vi "UNITEST MAIN v2.0.vi"() -> ()   [LabVIEW 2025]
uses:
  Traction Loop/Traction Receipe Enum.ctl
  controls/LAB-IQ UI Data.ctl
  <vilib>/Platform/TimedLoop/XDataNode/timing_clust.ctl
  <vilib>/Platform/TimedLoop/XDataNode/nitl_modes.ctl
  <vilib>/Platform/TimedLoop/XDataNode/wakeup.ctl
  Traction Loop/Traction Write enum.ctl
  Traction Loop/Traction Read enum.ctl
  HEAVE vi's/Heave Write enum.ctl
  SWAY vi's/Sway Write enum.ctl
  Acquostics Loops/Write Main Enum.ctl
  SWAY vi's/Sway Right enum.ctl
  HEAVE vi's/Heave Right enum.ctl
  Acquostics Loops/Read Main Enum.ctl
  0f9b3d6c-7caf-4790-9f98-5fac89a3677b.vi
  48f5795f-33f4-4366-aaa7-704d1097ecc1.vi
  d081153b-36ca-4bc4-8478-749476f82ba4.vi
  1202965f-721d-4349-8d61-5de826f379ef.vi
  785ec975-e53d-4ed4-be48-2cc128d7a91f.vi
  02c5850b-52e8-4ed5-91f8-6f0ad62f4994.vi
  1223eb78-e4c4-4b69-bf80-185c82055158.vi
  e5651a45-6a49-4a3f-b503-ff1eaf449b4a.vi
  <vilib>/Utility/error.llb/Trim Whitespace One-Sided.vi
  support/Message Queue/Enqueue Message (Single).vi
  <vilib>/Utility/error.llb/Error Cluster From Error Code.vi
  <vilib>/Utility/file.llb/Read Delimited Spreadsheet (string).vi
  <vilib>/Utility/file.llb/Write Delimited Spreadsheet (string).vi
  <vilib>/ErrorRing/Error Ring.xnode
  <vilib>/platform/TimedLoop/XDataNode/XDataNode.xnode
  support/Message Queue/LAB-IQ Message Queue.lvlib
  support/User Event - Stop/LAB-IQ User Event - Stop.lvlib
  <vilib>/Platform/TimedLoop/XDataNode/XDNodeRunTimeDep.lvlib
panel:
  out "AE Ring-Down Counts":u32(graph)
  out "Signal Energy":sgl(graph)
  out "Amplitude db_AE":sgl(graph)
  out "Peak Amplitude":sgl(graph)
  out "SET entrainment Velocity":dbl
  out "Test Array Size":i32
  in  "SRR INDEX [ STRIBECK]":i32
  out "Stribeck Size":i32
  out "SET SRR":dbl
  out "Enum - READ":T1
  out "ELAPSED TIMER":dbl
  out "BALL SET RPM":dbl
  out "DISC SET RPM":dbl
  out "SET LOAD":dbl
  in  "TEMPERATURE READ":dbl=40.0
  out "SET TEMPERATURE":dbl
  out "Traction Size":i32
  out "DISC SPEED (rpm)":dbl=100.0 min=0.1 max=3000.0 step=0.1 format="%.1f"
  out "BALL SPEED (rpm)":dbl=100.0 min=0.1 max=3000.0 step=0.1 format="%.1f"
  in  "BALL WEAR TRACK":dbl=7.9
  in  "DISC WEARTRACK":dbl=24.0
  in  "SRR INDEX [ TRACTION]":i32
  in  "Start Index Type":i32
  in  "Enum - Menu":T1
  out "Ball (mm/sec)":dbl
  out "Disc (mm/sec)":dbl
  in  "Traction Receipe Update Details":bool
  in  "HomeTraction":bool
  in  "Demo Mode Display":enum32{"Page 1", "Page 2"}(tab)
  in  "Traction Message":string="Recommended motion directions \nfor traction module.\n\nBall:  Counterclockwise\nDisc: Clockwise"
  in  "Traction Step Update Details":bool
  in  "Main Tab sequence for selection":T2(tab)
  out "ExceedDiscSpeed  Cinstant Speed":string
  out "ExceedBallSpeed Constant":string
  in  "TEST SELECTION (MTM) 2":enum32{"Ball Speed", "Disc Speed"}(radio)
  in  "SPEED SELECTION : MTM 2":enum32{"Speed in Rpm", "Speed in m/sec"}(radio)=enum."Speed in m/sec"
  in  "MTM Test Selection 2":enum32{"Time", "Cycle"}(radio)
  in  "Enter the Speed (m/sec):":dbl=0.5 min=3e-06 max=2500.0 step=0.001 format="%.6f"
  in  "Enter the Speed (m/sec):":dbl=0.5 min=3e-06 max=3000.0 step=0.001 format="%.6f"
  in  "Enter the Speed (RPM):":dbl=100.0 min=0.1 max=3000.0 step=0.1 format="%.1f"
  out "Lower Spped":string
  out "Upper":string
  in  "Enter the Speed (RPM):":dbl=1.0 min=0.1 max=2500.0 step=0.1 format="%.1f"
  out "ExceedBallSpeed step":string
  out "ExceedDiscSpeed":string
  out "Disc Speed Indicator":bool
  out "ExceedBallSpeed":string
  out "BallSpeed Exceed Indication":bool
  in  "Apply":bool
  in  "SPEED SELECTION : MTM":enum32{"Speed in Rpm", "Speed in m/sec"}(radio)=enum."Speed in m/sec"
  in  "TEST SELECTION (MTM)":enum32{"Ball Speed", "Disc Speed"}(radio)
  in  "MTM Test Selection":enum32{"Time", "Cycle"}(radio)
  in  "File Path Tab":enum32{"Page 1", "Page 2"}(tab)
  in  "File Path String":string="File Path Location : C:-->LAB-IQ 150 --> User Defined\n                                       Protocol-->File.txt"
  in  "Save":bool
  in  "Import":bool
  in  "File Path :":path
  in  "Step Sequence Indication Tab":enum32{"Page 1", "Page 2"}(tab)
  in  "Step Sequence Indication":string="Minimum 2 Steps required to perform the Speed Sequence"
  in  "Calculate Step":bool
  in  "StepTable":string[][](table)
  in  "Ramp Tab":enum32{"Page 1"}(tab)
  out "e.v/ssr":enum32{"E.V", "SSR"}(tab)
  in  "Enter Fixed SRR":dbl=1.0 min=-1.0 max=1.0 step=0.001 format="%.3f"
  in  "Enter the Final E.Velocity (m/s)":dbl=1.0 min=0.001 max=10.0 step=0.001 format="%.3f"
  in  "Enter initial E.Velocity (m/s)":dbl=2.0 min=0.001 max=10.0 step=0.001 format="%.3f"
  in  "Enter Fixed E.Velocity":dbl=1.0 min=0.001 max=2.0 step=0.001 format="%.3f"
  in  "Enter Final SRR":dbl=1.0 min=-1.0 max=1.0 step=0.001 format="%.2f"
  in  "Enter initial SRR":dbl=1.0 min=-1.0 max=1.0 step=0.001 format="%.2f"
  in  "Ball WTD":dbl=17.32 min=17.32 max=17.32 step=0.001 format="%.2f"
  in  "E.Velocity":bool caption="SRR"
  in  "Enter the Final Velocity (m/s)":dbl=1.0 min=0.001 max=2.0 step=0.001 format="%.3f"
  in  "Enter initial Velocity (m/s)":dbl=2.0 min=0.001 max=2.0 step=0.001 format="%.3f"
  out "Ramp Up   Disc":bool caption="Ramp Down"
  out "Initial DiscSpeed (RPM)":dbl=100.0 min=0.1 max=3000.0 step=0.1 format="%.1f"
  out "Final Speed (RPM)":dbl=1.0 min=0.1 max=3000.0 step=0.1 format="%.1f"
  out "Final Speed (RPM)":dbl=1.0 min=0.1 max=3000.0 step=0.1 format="%.1f"
  out "Initial Speed (RPM)":dbl=100.0 min=0.1 max=3000.0 step=0.1 format="%.1f"
  in  "Enter the Final Velocity (m/s)":dbl=1.0 min=0.001 max=2.0 step=0.001 format="%.3f"
  in  "Enter initial Velocity (m/s)":dbl=2.0 min=0.001 max=2.0 step=0.001 format="%.3f"
  out "Ramp Up":bool caption="Ramp Down"
  in  "Disc Motion Direction:":u16(ring) items=["Clockwise", "Counter Clockwise"]
  in  "Ball Motion Direction :":u16(ring) items=["Clockwise", "Counter Clockwise"]
  in  "Motion Mode:":u16(ring) items=["Uniform Rotation", "Speed Step", "Speed Ramp", "Speed Recipe"]
  in  "Wear Track Diameter (mm) 3":dbl=16.0 caption="Wear Track Diameter (mm):" min=1.0 max=20.0 step=0.01 format="%.2f"
  in  "Set WTD 2":bool
  in  "SRR Sweep Range (%)":string caption="Speed (mm/s)"
  out "Traction Receipe":i32(listbox)=-1
  in  "Total Execution Time":dbl
  in  "Total Steps":dbl
  in  "Duration / Step (s)":dbl=6.0
  in  "STRIBECK Fixed SRR List (%)":string="5,10,20,40,60,80,100"
  in  "Duration / Step (s)":dbl=6.0
  in  "SRR Sweep Range (%)":string
  in  "Speed (mm/s)":dbl=1000.0
  in  "Temperature Stages (°C)":string="40,100,140"
  in  "Load (N)":string="25"
  in  "Lubricant Name":string
  in  "Profile File Name":string
  out "error out":errorcluster
  in  "DEPTH TRIP   ENABLE":bool
  in  "DEPTH TRIP VALUE":dbl
  in  "LOAD TRIP  ENABLE":bool
  in  "LOAD TRIP VALUE":dbl
  in  "CYCLIC COF TRIP  ENABLE":bool
  in  "CYCLIC FF TRIP  ENABLE":bool
  in  "FF TRIP  ENABLE":bool
  in  "COF TRIP  ENABLE":bool
  in  "CYCLIC CoF TRIP VALUE":dbl
  in  "CYCLIC FF TRIP VALUE":dbl
  in  "FF TRIP VALUE":dbl
  in  "COF TRIP VALUE":dbl
  in  "Dummy Run":bool
  in  "AutoTune":bool
  in  "reinit 3":bool=TRUE
  in  "output range delay":cluster{"output high":dbl, "output low":dbl}={"output high"=100.0, "output low"=-100.0} {"output low" format="%.2f"; "output high" format="%.2f"}
  in  "PID gains out delay":T3={"proportional gain (Kc)"=30.0, "integral time (Ti, min)"=0.00101, "derivative time (Td, min)"=0.0} {"derivative time (Td, min)" format="%.3f"; "integral time (Ti, min)" min=1e-05 max=100.0 step=0.0001 format="%.4f"; "proportional gain (Kc)" format="%.3f"}
  in  "PID gains out delay (microForce)":T3={"proportional gain (Kc)"=300.0, "integral time (Ti, min)"=0.00011, "derivative time (Td, min)"=0.0} {"derivative time (Td, min)" format="%.3f"; "integral time (Ti, min)" min=1e-05 max=100.0 step=1e-06 format="%.6f"; "proportional gain (Kc)" format="%.3f"}
  in  "Gain 2":dbl=0.016
  in  "Offset  3":dbl=1.5
  in  "Ramp MulFac":dbl=2.0
  out "actpid":dbl
  in  "pulses LoadDiffRamp(2..10)":dbl=9.0
  in  "PulseControlRamp(diff<=3N)":dbl=5.0 min=1.0 max=1000.0 step=1.0 format="%#.1f"
  in  "SetLoadDeadband(%) Load(0-10N)":dbl=0.1 min=0.0001 max=100.0 step=0.0001 format="%#.6f"
  in  "pulses LoadDiff(2..10)":dbl=10.0
  in  "pulses LoadDiff(11..50)":dbl=40.0
  in  "PulseControl(diff<=3N)":dbl=1.0 min=1.0 max=1000.0 step=1.0 format="%#.1f"
  out "SetLoadDeadband(%)  2":dbl=1.0 min=0.001 max=100.0 step=0.001 format="%#.6f"
  in  "pulsesSent":dbl=200.0
  out "pulses":dbl
  in  "pulses LoadDiff(21..1000)":dbl=40.0
  in  "Delay":dbl=1.5 min=0.001 max=5.0 step=0.001 format="%#.6f"
  in  "deadband":dbl=0.2
  in  "Checkbox 2":bool
  in  "Checkbox":bool=TRUE
  out "Scratch Start Recording":bool
  in  "SwaySpeed Set":bool
  in  "Update":bool
  in  "Analysis Home":bool
  in  "Installation/Replacement completed":bool
  in  "Loahead":bool
  in  "Heave and Surge COM Port:":refnum<visa-resource-name>="COM9"
  in  "Sway COM Port:":refnum<visa-resource-name>="COM10"
  out "Test Trip":bool
  out "Hymidity":bool
  in  "Humidity Disable trip":bool=TRUE
  in  "CoF Trip  2":dbl=540.0 min=100.0 max=540.0 step=1.0
  in  "File Path :  2":path
  out "Wear Track Diameter":dbl
  in  "Stribeck table":bool
  in  "seq":bool=TRUE
  out "Drive Error":string
  out "mm/s  Surge":dbl=7.0 caption="Jog" min=0.001 max=50.0 step=0.0001 format="%.2f"
  in  "Update Surge Speed":bool
  out "mm/s  Sway":dbl=7.0 caption="Jog" min=0.001 max=50.0 step=0.0001 format="%.2f"
  in  "Update Sway Speed":bool
  in  "Update Heave Speed":bool
  out "mm/s Heave":dbl=7.0 caption="Jog" min=0.001 max=30.0 step=0.0001 format="%.2f"
  in  "mm/sec":dbl=1.0 caption="Jog" min=0.001 max=50.0 step=0.001 format="%.2f"
  out "Scratch Start Test":bool
  in  "HomeScratch":bool
  in  "TEST SELECTION":enum32{"Time", "Cycle"}(radio)
  out "Spare 15":u8
  out "Spare 14":u8
  out "Spare 13":u8
  out "Spare 12":u8
  out "Spare 11":u8
  out "Spare 10":u8
  out "Spare 9":u8
  out "Spare 8":u8
  out "Start Test Temp":bool
  in  "AppLoadSeq scratch":bool
  in  "PID Delay (sec)":dbl=1.0 format="%#_6p"
  out "Spare 15":u8
  out "Spare 14":u8
  out "Spare 13":u8
  out "Spare 12":u8
  out "Spare 11":u8
  out "Spare 10":u8
  out "Spare 9":u8
  out "Spare 8":u8
  out "Load Cell Temp":bool
  in  "Stop Scratch":bool
  in  "Enter Fixed SRR 2":dbl min=0.0 max=0.0 format="%.3f"
  in  "E.Velocity 2":bool=TRUE caption="SRR"
  in  "Tab Control 3":T4(tab)
  in  "Tab Control 5":enum32{""}(tab)
  in  "Tab Control 14":T5(tab)=enum."Motor Load"
  in  "Ramp":bool
  in  "apply load":bool
  in  "Enter ByPass Load":dbl
  in  "Bypass Load":bool
  out "gFF Rot 7":cluster{dbl, dbl, dbl}(graph)
  in  "Current Load":dbl
  in  "Set Load":dbl
  out "Current Position":dbl
  in  "Kp":dbl=1.0
  in  "Ki":dbl
  in  "Kd":dbl
  in  "Deadband":dbl=0.1
  in  "pct_scale":dbl=100.0
  in  "Init Step":dbl=10.0
  in  "Max Step Linit":dbl=10.0
  in  "i_limit":dbl=10.0
  in  "Min_pos_limit":dbl
  in  "Max_pos_limit":dbl=50000000.0
  in  "Fine Tune Zone":dbl=10.0
  out "Pulse delta":dbl
  out "Vertical load (N)":dbl format="%#.3f"
  in  "filter_alpha":dbl=0.05
  in  "dynamic_spindle_noise_scalar":dbl=100.0
  in  "min_finetune_floor":dbl=10.0
  in  "min_deadband_floor":dbl=50000000.0
  in  "Tab Control 26":enum32{"Page 1", "Page 2"}(tab)
  in  "ClearAll":bool
  out "Mz(Nm)":dbl[](array[numeric])
  out "My(Nm)":dbl[](array[numeric])
  out "Mx(Nm)":dbl[](array[numeric])
  in  "Save Dwell":dbl=0.015 caption="Save Dwell (sec)" min=0.0 max=5.0 step=0.001 format="%.3f"
  out "Mx":dbl[](graph)
  out "My":dbl[](graph)
  out "Mz":dbl[](graph)
  out "Fy(N)":dbl[](graph)
  out "Fz(N)":dbl[](graph)
  in  "ZeroAll":bool
  in  "Acq Delay (ms)":dbl=10.0
  in  "Burst Delay (ms)":dbl=10.0
  out "model":string
  out "SN":i32
  out "FFx(N)":dbl[](array[numeric])
  in  "Sensor IP":string="192.168.1.100"
  in  "Port":i32=8080
  out "FFy(N)":dbl[](array[numeric])
  out "Load(N)":dbl[](array[numeric])
  out "Fx(N)":dbl[](graph)
  out "AE":bool
  in  "delete Handle":bool
  in  "Create Handle":bool=TRUE
  out "ft_data":dbl[](array[numeric])=[1.0, 1.0, 1.0, 1.0, 1.0, 1.0]
  out "ft_range":dbl[](array[numeric])=[1.0, 1.0, 1.0, 1.0, 1.0, 1.0]
  in  "stop 6":bool
  out "running_flag":bool
  out "ft_udp_handle":i32
  out "get-data-return":i32
  out "get-range-return":i32
  out "zero-return":i32
  out "filter-return":i32
  out "initial-return":i32
  out "deleteHandle-result":i32
  in  "Tab Control 19":enum32{"Platform COM", "Config ", "DevInfo"}(tab)=enum."Config "
  in  "Manual Write Acquostic":bool
  out "data out":string
  out "Last Config Rejected":u32
  out "rx command count":u32
  out "Current Filter Id":u32
  out "Isolated Gain":u32
  out "DAQ Status":u32
  out "Heave and Surge Read":string
  out "error out Write":errorcluster
  out "error out Read":errorcluster
  out "Sequence ID":u16
  in  "Mode Command":u8=2
  in  "Distance":sgl=10000.0
  in  "SPEED":sgl=10000.0
  out "Ack ID":u16
  out "State":u8
  out "Homed":u8
  out "HEAVE POSE":sgl format="%#.6f"
  out "SURGE POSE":sgl format="%#.6f"
  out "faultCode":u16
  out "fwMajor":u8
  out "fwMinor":u8
  out "Read Heave Temp":bool
  out "Node Id":u8
  out "Spare 1":u8
  out "Spare 2":u8
  out "Spare 3":u8
  out "Spare 4":u8
  out "Spare 5":u8
  out "Spare 6":u8
  out "Spare 7":u8
  in  "SPARE 1":u8
  in  "SPARE 2":u8
  in  "SPARE 3":u8
  in  "SPARE 4":u8
  out "Heave and Surge Write":string
  in  "Manual Write Heave & Surge":bool
  out "HEAVE ENABLE":bool
  in  "Reserved":sgl
  in  "SPARE 5":u8
  in  "SPARE 6":u8
  in  "SPARE 7":u8
  in  "SPARE 8":u8
  in  "SPARE 9":u8
  in  "SPARE 10":u8
  in  "SPARE 11":u8
  in  "SPARE 12":u8
  in  "SPARE 13":u8
  in  "SPARE 14":u8
  in  "SPARE 15":u8
  in  "SPARE 16":u8
  in  "SPARE 17":u8
  out "System UPTIME":sgl
  out "Missed Packets":sgl format="%#.6f"
  out "faultCode Heave":u16
  out "faultCode Surge Left":u16
  out "faultCode Surge Right":u16
  out "SWAY READ":string
  out "error out Write  SWAY":errorcluster
  out "error out Read SWAY":errorcluster
  out "Sequence ID":u16
  in  "Mode Command":u8=2
  in  "Distance":sgl=10000.0
  in  "SPEED":sgl=10000.0
  out "Ack ID":u16
  out "State":u8
  out "Homed":u8
  out "SWAY POSE":sgl format="%#.6f"
  out "Rotary POSE":sgl format="%#.6f"
  out "faultCode":u16
  out "fwMajor":u8
  out "fwMinor":u8
  out "Read SWAY Temp":bool
  out "Node Id":u8
  out "Spare 1":u8
  out "Spare 2":u8
  out "Spare 3":u8
  out "Spare 4":u8
  out "Spare 5":u8
  out "Spare 6":u8
  out "Spare 7":u8
  in  "SPARE1":u8
  in  "SPARE 2":u8
  in  "SPARE  3":u8
  in  "SPARE  4":u8
  out "SWAY WRITE":string
  in  "Manual Write SWAY":bool
  in  "SPARE  5":u8
  in  "Reserved":sgl
  in  "SPARE 6":u8
  in  "SPARE 7":u8
  in  "SPARE 8":u8
  in  "SPARE 9":u8
  in  "SPARE 10":u8
  in  "SPARE 11":u8
  in  "SPARE 12":u8
  in  "SPARE 13":u8
  in  "SPARE 14":u8
  in  "SPARE 15":u8
  in  "SPARE 16":u8
  in  "SPARE 17":u8
  out "System UPTIME":sgl
  out "Missed Packets":sgl format="%#.6f"
  out "faultCode Sway":u16
  out "faultCode Rotary":u16
  out "TRACTION READ":string
  out "error out Write  TRACTION":errorcluster
  out "error out Read TRACTION":errorcluster
  out "Sequence ID":u16
  in  "Mode Command":u8=2
  in  "Distance":sgl=10000.0
  in  "SPEED":sgl=10000.0
  out "Ack ID":u16
  out "State":u8
  out "Homed":u8
  out "TRACTION POSE 1":sgl format="%#.6f"
  out "TRACTION POSE 2":sgl format="%#.6f"
  out "faultCode":u16
  out "fwMajor":u8
  out "fwMinor":u8
  out "Read TRACTION Temp":bool
  out "Node Id":u8
  out "Spare 1":u8
  out "Spare 2":u8
  out "Spare 3":u8
  out "Spare 4":u8
  out "Spare 5":u8
  out "Spare 6":u8
  out "Spare 7":u8
  in  "SPARE 1":u8
  in  "SPARE 2":u8
  in  "SPARE  3":u8
  in  "SPARE  4":u8
  out "TRACTION WRITE":string
  in  "Manual Write TRACTION":bool
  in  "SPARE  5":u8
  in  "Reserved":sgl
  in  "SPARE 6":u8
  in  "SPARE 7":u8
  in  "SPARE 8":u8
  in  "SPARE 9":u8
  in  "SPARE 10":u8
  in  "SPARE 11":u8
  in  "SPARE 12":u8
  in  "SPARE 13":u8
  in  "SPARE 14":u8
  in  "SPARE 15":u8
  in  "SPARE 16":u8
  in  "SPARE 17":u8
  out "System UPTIME":sgl
  out "Missed Packets":sgl format="%#.6f"
  out "faultCode Traction 1":u16
  out "faultCode Traction 2":u16
  in  "Uplink Packet":T6
  out "Downlink Packet":T7
  in  "error in (no error)":errorcluster
  out "error out":errorcluster
  in  "JOG TRIP LOAD VALUE (N)":dbl
  in  "SAMPLES":dbl=100.0
  in  "Re-initilaize":bool
  in  "Filter ON/OFF":bool=TRUE
  in  "TracHomeSurgeOffsetCounts 10MM":dbl=505100.0
  in  "TracHomeSwayOffsetCounts 10MM":dbl=1432.0
  in  "Acoustic Emission:":dbl=1.0 min=0.0001 max=200.0 step=0.0001 format="%.4f"
  in  "Apply Filter (FF)":bool
  in  "Filter% 2":dbl=50.0 min=50.0 max=100.0 step=0.1 format="%.1f"
  in  "Apply Filter (Load)":bool=TRUE
  in  "Filter%":dbl=80.0 min=50.0 max=100.0 step=0.1 format="%.1f"
  in  "Sway distance (mm)":dbl=245.0
  in  "Surge distance (mm)":dbl=370.0
  in  "DataSavingLoopDelay(ms)":dbl=15.0
  in  "SAVE  2":bool
  in  "Enter Distance":bool caption="Enter Counts"
  in  "Sway Counts:":dbl=100.0 min=0.0 max=100000000.0 step=1.0 format="%.2f"
  in  "Distance (mm): 3":dbl=100.0 caption="Distance (mm):" min=0.0 max=1500.0 step=0.001 format="%.5f"
  in  "Surge Counts:":dbl=100.0 min=0.0 max=100000000.0 step=1.0 format="%.1f"
  in  "Distance (mm): 2":dbl=100.0 caption="Distance (mm):" min=0.0 max=1500.0 step=0.0001 format="%.3f"
  in  "Distance (mm):":dbl=100.0 min=0.0 max=1500.0 step=0.001 format="%.5f"
  in  "Heave Counts:":dbl=100.0 min=0.0 max=100000000.0 step=1.0
  in  "LRMHomeSurgeOffsetCounts":dbl=307197.0
  in  "LRMHomeSwayOffsetCounts":dbl=26880.0
  in  "TracHomeSurgeOffsetCounts 20MM":dbl=505100.0
  in  "TracHomeSwayOffsetCounts 20MM":dbl=1432.0
  in  "RotHomeSwayOffsetCounts":dbl=14656.0
  in  "RotHomeSurgeOffsetCounts":dbl=311465.0
  in  "Heave distance":dbl=340.0
  out "Zmm":dbl=1600.0
  out "Heave Pulses/mm":dbl=1600.0
  out "Surge Pulses/mm":dbl=1600.0
  out "Sway Pulses/mm":dbl=320.0
  in  "Heave Pitch":dbl=4.0
  in  "Surge Pitch":dbl=3.0
  in  "Sway Pitch":dbl=2.0
  in  "Heave PPR":dbl=6400.0
  in  "Surge PPR":dbl=6400.0
  in  "Sway PPR":dbl=6400.0
  in  "Heave Jog Speed":dbl=15.0
  in  "Surge Jog Speed":dbl=1.0 format="%.4f"
  in  "Heave PID Speed":dbl=15.0
  in  "Heave Loop Delay":dbl
  in  "Sway Jog Speed":dbl=1.0 format="%.4f"
  in  "Sway PID Speed":dbl=1.0 format="%.4f"
  in  "Sway Loop Delay":dbl
  in  "GUI":T8(tab)
  in  "Platform Settings":bool caption="Password"
  in  "Configure":bool caption="Password"
  in  "Home":bool caption="Password"
  in  "EXIT":bool
  in  "Analysis":bool caption="Password"
  in  "service 2":bool caption="Password"
  in  "MainPage":T9(tab)=enum."HOME"
  in  "Select Load Head":bool
  in  "Notes :":string
  in  "FILE":string
  in  "Sample ID :":string
  in  "Operator ID :":string
  in  "Operator Name :":string
  in  "Auto":bool caption="Power Status"
  in  "Disable Axis Jog Soft Limits m":bool
  out "Sway and Surge COM Status":bool=TRUE caption="Load COM Status"
  out "Heave COM Status":bool=TRUE caption="Load COM Status"
  in  "Enable Platform":bool
  in  "Surge Forward Main":bool
  in  "Surge Backward Main":bool
  in  "Sway Right Main":bool
  in  "Sway Left Main":bool
  in  "Heave Down Main":bool
  in  "Heave Up main":bool
  in  "mm":dbl=0.001 caption="Jog" min=0.001 max=100.0 step=0.01 format="%#.3f"
  in  "Surface Analysis":bool
  in  "Imaging":bool
  in  "Image Analysis":bool
  in  "Post Analysis":bool
  in  "SSP 0.75":bool
  in  "SSP 0.5":bool
  in  "SSP 0.3":bool
  in  "Warning":enum32{"Page 2"}(tab)
  in  "gui GIF":enum32{"Check", "Deca", "kilo", "Micro"}(tab)
  out "Communication is established":bool=TRUE caption="Load COM Status"
  in  "Reference Sample":u16(ring) items=["None", "Brass", "Aluminium", "Mild Steel"]
  out "Load Cell Communication Slide":u8(slide)=1 min=1 max=10 step=1 scale=0.0..10.0
  in  "com 3":bool
  out "com":bool
  out "DecaForce COM Status":bool caption="Load COM Status"
  in  "Loading Mode":u16(ring) items=["Constant", "Ramp", "Steps", "Indentation"]
  in  "Enter the CoF Trip":dbl=1.0
  in  "Enter the Friction Force Trip":dbl=520.0 min=500.0 max=500.0 step=1.0 format="%#.1f"
  in  "Enter the Normal load Trip":dbl=520.0 min=500.0 max=500.0 step=0.001 format="%.3f"
  in  "KiloForce":bool
  in  "DecaForce":bool
  in  "MicroForce":bool
  in  "LHBack":bool
  in  "LHNext":bool
  in  "Load Selection":T10(tab)
  in  "Enter the Load  (N)":dbl=2.0 caption="Enter the Load (N)" min=2.0 max=50.0 step=0.1 format="%#.4f"
  in  "Enter the Final Load (N)":dbl=1.0 min=0.0 max=500.0 step=1.0 format="%#.0f"
  in  "Enter the Loading Rate (N/min)":dbl=60.0 min=1.0 max=1200.0 step=0.1 format="%.2f"
  out "Warning 2":bool
  in  "Stribeck Table  For loading":string[][](table)
  in  "Clear 3":bool
  out "Message":string="Load Entered is out of range!!!"
  in  "Indentation":string[][](table)=[["Detection", "5", "2"], ["Unload", "0", "5"], ["Load", "10", "2"], ["Unload", "0", "5"], ["Detection", "5", "2"], ["Unload", "0", "5"]]
  in  "Multipoint":bool caption="Singlepoint"
  in  "AppLoad 4":bool
  in  "zNL":bool
  out "NL disp":dbl caption="Normal Load ( N )" min=-2000.0 max=2000.0 step=0.0001 format="%.1f"
  in  "Traction":bool
  in  "Surge Forward MM":bool
  in  "Surge Backward MM":bool
  in  "M3 Image":enum32{"Page 1", "Page 2"}(tab)
  in  "String 39":string="Jog heave to bring the upper sample closer to the lower sample within 1mm."
  in  "Sway Left MM":bool
  in  "Sway Right MM":bool
  in  "Disable Axis Jog Soft Limits":bool
  in  "mm":dbl=0.001 caption="Jog" min=0.001 max=5.0 step=0.0001 format="%#.3f"
  in  "Heave Down MM":bool
  in  "Heave Up MM":bool
  in  "Wear Track Diameter (mm)":dbl=30.0 caption="Wear Track Diameter (mm):" min=1.0 max=30.0 step=1.0 format="%.2f"
  in  "Set WTD":bool
  in  "HomeScratch":bool
  in  "HomeRot":bool
  in  "PlaceModule":bool
  in  "Motion Mode:":u16(ring) items=["Uniform Rotation", "Angular Oscillation", "Stribeck ", "Steps"]
  in  "LR Sway":bool
  in  "Rot Hor":bool
  in  "Rot Ver":bool
  in  "Scratch":bool
  in  "LR Cam":bool
  in  "MMBack":bool
  in  "MMNext":bool
  in  "Rotary Module Selection":T11(tab)
  in  "SPEED SELECTION :":enum32{"Speed in RPM", "Speed in m/sec"}(radio)=enum."Speed in m/sec"
  in  "Enter the Speed(mm/sec)":dbl=0.1 min=0.1 max=10.0 step=0.1 format="%.3f"
  in  "Enter the Speed (RPM)":dbl=45.0 min=1.0 max=3000.0 step=1.0
  in  "Enter the Frequency (Hz)":dbl=1.0 min=0.1 max=10.0 step=0.1 format="%.1f"
  in  "Enter the Angle (Deg)":dbl=45.0 min=5.0 max=300.0 step=1.0
  in  "Angular Oscillation Set":bool
  in  "Rotary Tab":enum32{"Page 1", "Page 2"}(tab)
  out "e.v/ssr 2":enum32{"E.V", "SSR"}(tab)
  in  "Enter the Final E.Velocity (m/s) 2":dbl=1.0 min=0.001 max=4.0 step=0.001 format="%.3f"
  in  "Enter initial E.Velocity (m/s) 2":dbl=2.0 min=0.001 max=4.0 step=0.001 format="%.3f"
  in  "Enter Fixed E.Velocity 2":dbl=1.0 min=0.001 max=2.0 step=0.001 format="%.3f"
  in  "Enter Final SRR 2":dbl=1.0 min=0.001 max=1.0 step=0.001 format="%.2f"
  in  "Enter initial SRR 2":dbl=1.0 min=0.001 max=1.0 step=0.001 format="%.2f"
  out "Final Speed (RPM) 3":dbl=1.0 min=0.1 max=3000.0 step=0.1 format="%.1f"
  out "Initial Speed (RPM) 2":dbl=100.0 min=0.1 max=3000.0 step=0.1 format="%.1f"
  in  "Enter the Final Velocity (m/s) 3":dbl=1.0 min=0.001 max=2.0 step=0.001 format="%.3f"
  in  "Enter initial Velocity (m/s)  3":dbl=2.0 min=0.001 max=2.0 step=0.001 format="%.3f"
  out "Ramp Up 2":bool caption="Ramp Down"
  in  "Import 2":bool
  in  "Save 2":bool
  in  "SPEED SELECTION : rotary":enum32{"Speed in Rpm", "Speed in m/sec"}(radio)=enum."Speed in m/sec"
  in  "calculate rotary":bool
  in  "String 45":string="File Path Location : C:-->LAB-IQ 150 --> User Defined\n                                       Protocol-->File.txt"
  in  "Step Speed":enum32{"Step Speed", "Step (load-Speed)"}(tab)
  in  "StepTable For Speed":string[][](table)
  in  "StepTable For Load-Speed":string[][](table)=[["", "", ""], ["", "", ""], ["", "", ""], ["", "", ""]]
  in  "StepTable For Speed 3":string[][](table)=[["", "", ""], ["", "", ""], ["", "", ""], ["", "", ""]]
  in  "Motion Direction:  3":u16(ring) items=["Clockwise", "Counter Clockwise"]
  in  "Enter Scratch length (mm):":dbl=1.0 min=1.0 max=50.0 step=0.0001 format="%.4f"
  in  "Enter Scratch Speed (mm/s):":dbl=1.0 min=0.003 max=10.0 step=0.0031 format="%.5f"
  in  "Scartch Offset":dbl=1.0 caption="Scratch Offset: (mm)" min=0.1 max=5.0 step=0.1 format="%.1f"
  in  "Motion type:":u16(ring) items=["Unidirection", "Bidirection"]
  in  "Scratch Mode":u16(ring) items=["Scratch", "Pre-Post Scan", "Multi Scratch"]
  in  "Rotary Speed Exced":string="Motor Speed Out of Range"
  in  "No of Scratch":dbl=1.0 min=1.0 max=50.0 step=0.0001
  out "Humidity  Status  3":bool caption="Communication Status"
  out "Low Temp  Status  2":bool=TRUE caption="Communication Status"
  out "TK4 status 2":bool=TRUE caption="Communication Status"
  in  "Acuostic M":string="Before selecting Acoustic make sure the sensor output pin is connected to A4."
  in  "Stage Temperature":dbl[](array[numeric])=[150.0, 230.0, 300.0, 350.0, 400.0, 450.0, 500.0]
  in  "Sample Temperature":dbl[](array[numeric])=[100.0, 150.0, 200.0, 250.0, 300.0, 350.0, 400.0]
  in  "Humidity (Amb)":bool
  in  "Clear List":bool
  out "Sensors Picked":string
  in  "Add to list":bool
  in  "Wear":bool
  in  "Vibration":bool
  in  "Humidity (Chamber)":bool
  in  "Temperature (Chamber)":bool
  in  "ECR":bool
  in  "Temperature (Amb)":bool
  in  "Microphone":bool
  in  "Acoustic Emission 3":bool
  in  "SNext":bool
  in  "APBack":bool
  in  "Enter the Temperature (°C):":dbl
  in  "Enter the Stage \nTemperature (°C):":dbl=20.0 min=20.0 max=150.0 step=1.0 format="%#.0f"
  in  "Enter the Humidity (%Rh):":dbl=30.0 min=30.0 max=85.0 step=1.0
  in  "Low Temp":bool
  in  "High Temp":bool
  in  "Humidity":bool
  in  "Gains":enum32{"20dB", "40dB", "60dB"}(radio)=enum."60dB"
  in  "Main Screen Tab":T12(tab)
  in  "Depth Reset Graph":bool
  out "Weart Deapth":bool
  in  "Depth Trip 2":bool=TRUE
  out "Depth Trip":dbl=600.0
  out "NL Display 4":dbl caption="Normal Load ( N )" min=-2000.0 max=2000.0 step=0.0001 format="%.1f"
  in  "Load Reset Graph":bool
  in  "Load Disable Trip":bool=TRUE
  out "Load pid":bool
  out "NL Trip 2":dbl=600.0
  in  "ClrLog":bool
  out "Trip Log":string
  in  "Start Test":bool
  out "Test status":bool caption="Test Status"
  out "AR Led":bool caption="AR"
  out "Data":bool=TRUE
  out "Health":bool=TRUE
  out "Sway COM Status":bool=TRUE caption="Load COM Status"
  out "Heave COM Status":bool=TRUE caption="Load COM Status"
  in  "BACK":bool
  out "Ambient \nTemperature":dbl min=0.0 max=5000.0 step=0.1 format="%.1f"
  out "Ambient\n Humidity":dbl min=0.0 max=5000.0 step=0.1 format="%.2f"
  out "NL disp 2":dbl caption="Normal Load ( N )" min=-2000.0 max=2000.0 step=0.0001 format="%.1f"
  out "Set Humidity":dbl caption="Set Humidity  (% Rh)" min=-2000.0 max=2000.0 step=1.0 format="%.1f"
  out "humidity disp":dbl caption="Humidity (% Rh)" min=-2000.0 max=2000.0 step=1.0 format="%.1f"
  in  "Humidity On":bool
  in  "zNL 2":bool
  out "NLt":bool
  in  "Load En":bool
  out "Freq (Hz)":dbl min=0.0 max=5000.0 step=0.1 format="%.4f"
  out "HumCOMStatus":bool caption="Communication Status"
  out "Load Communication":bool
  in  "Temp Tabs":enum32{"Low Temp", "High Temp"}(tab)=enum."High Temp"
  out "Controller  Status":bool
  out "ChamberTemp":dbl format="%#.1f"
  in  "SetTmp":dbl=-190.0 caption="Set Temperature (Deg C)" min=-190.0 max=100.0 step=1.0 format="%.1f"
  in  "Cooling":bool
  in  "Heater":bool
  out "TK4 status":bool caption="Controller  Status"
  out "ChamberTemp":dbl format="%#.1f"
  in  "SetTmp":dbl caption="Set Temperature (Deg C)" min=0.0 max=1000.0 step=1.0 format="%.1f"
  in  "Set Load (N)":dbl=100.0 min=0.01 max=1500.0 step=0.01 format="%.1f"
  in  "Time Tab":enum32{"cycles", "duration"}(tab)=enum."duration"
  out "Test Duration 4":dbl=600.0 caption="Test Duration\n(HH:MM:SS)" min=0.0083 max=180000.0 step=0.0001 format="%<%H:%M:%S>t"
  out "TEST CYCLE":dbl min=0.0 max=5000.0 step=0.01 format="%.2f"
  in  "TOTAL CYCLES":dbl min=0.0 max=5000.0 step=0.1 format="%.4f"
  out "Time ( HH:MM:SS ) 2":dbl min=0.0 max=144000.0 step=1.0 format="%<%H:%M:%S>t"
  in  "Test Duration":dbl=600.0 caption="Test Duration\n(HH:MM:SS)" min=0.0083 max=180000.0 step=0.0001 format="%<%H:%M:%S>t"
  in  "Main Speed Tab":enum32{"ROTARY", "TRACTION"}(tab)
  in  "SPEED TAB":enum32{"RPM", "m/sec"}(tab)
  out "Speed (RPM)":dbl min=0.0 max=5000.0 step=0.1 format="%.1f"
  out "Set Speed":dbl caption="Set Speed (RPM)" min=0.0 max=1500.0 step=0.1 format="%.1f"
  out "Speed (m/sec)":dbl min=0.0 max=5000.0 step=0.001 format="%.4f"
  out "Set Speed (m/sec)":dbl min=0.0 max=1500.0 step=0.001 format="%.4f"
  in  "MTM MOTOR DISPLAY":enum32{"MTM RPM", "MTM m/sec"}(tab)
  out "Disc Speed (RPM)":dbl min=0.0 max=1500.0 step=0.1 format="%.1f"
  out "Ball Speed (RPM)":dbl min=0.0 max=1500.0 step=0.1 format="%.1f"
  out "Disc Speed (m/sec)":dbl min=0.0 max=1500.0 step=0.1 format="%.1f"
  out "Ball Speed (m/sec)":dbl min=0.0 max=1500.0 step=0.1 format="%.1f"
  in  "Angle and Frequency":enum32{"angular", "lrm"}(tab)
  out "Angle (Deg)":dbl min=0.0 max=5000.0 step=0.01 format="%.2f"
  out "Stroke (mm)":dbl min=0.0 max=5000.0 step=0.01 format="%.2f"
  in  "STOP":bool
  out "Multi Scratch Pass":dbl min=0.0 max=5000.0 step=0.1
  in  "FF Tab":T13(tab)
  in  "COF Reset Graph":bool
  in  "COF Disable Trip":bool=TRUE
  out "COF TRIP":dbl=600.0
  out "Coefficient of Friction":dbl(graph)=0.13298760003255525
  in  "zFF":bool
  out "Friction Force (N)":dbl min=-2000.0 max=2000.0 step=0.0001 format="%.3f"
  in  "FF Reset Graph":bool
  in  "FF Disable Trip":bool=TRUE
  out "FF TRIP":dbl=600.0
  out "Friction Force (N) Graph":dbl(graph)=0.13298760003255525
  in  "CZ FF":bool
  out "Cyclic Friction Force (N)":dbl min=-2000.0 max=2000.0 step=0.0001 format="%.3f"
  out "Cyclic FF TRIP":dbl=600.0
  in  "Cyclic FF Disable Trip":bool=TRUE
  in  "Cyclic FF Reset Graph":bool
  out "Cyclic Friction Force (N) Graph":dbl(graph)=0.13298760003255525
  out "cyclic COF TRIP":dbl=600.0
  in  "cyclic COF Disable Trip":bool=TRUE
  in  "cyclic COF Reset Graph":bool
  out "Cyclic Coefficient of Friction":dbl(graph)=0.13298760003255525
  out "Main Chart 3":cluster{dbl, "NL disp":dbl, dbl}(graph)
  out "WearGp":dbl(graph)=0.13298760003255525
  out "Depth (µm)":dbl min=-200.0 max=200.0 step=0.1 format="%.1f"
  in  "Depthz":bool
  out "Weart":bool
  in  "Sub Graph":T14(tab)
  in  "Speed Tab":enum32{" Rotary Disc", "MTM Ball", "MTM Disc"}(tab)
  in  "Speed Reset Graph":bool
  out "speed mm/sec":dbl(graph)=0.13298760003255525
  out "MTM BALL SPEED":dbl(graph)=0.13298760003255525
  out "MTM DISC  SPEED":dbl(graph)=0.13298760003255525
  in  "Temperature Reset":bool
  out "Temperature (deg c)":dbl(graph)=0.13298760003255525
  out "ECR 2":dbl(graph)=0.13298760003255525
  in  "ECR RESET":bool
  out "Acoustic Emission (mV)":dbl min=0.0 max=5000.0 step=0.1
  in  "Aqucostic Reset Graph":bool
  out "gACQUOS":dbl(graph)=0.13298760003255525
  in  "Humidity Reset Graph":bool
  out "HumrGp":dbl(graph)=0.13298760003255525
  out "SD (mm)":dbl caption="Sliding Distance ( mm )" min=-200.0 max=200.0 step=0.1 format="%.4f"
  in  "Siliding distance Reset Graph":bool
  out "SDGp":dbl(graph)=0.13298760003255525
  in  "X-AXIS":u16(ring) items=["None", "Time ( Sec )", "Normal Load ( N )", "Frictional Force ( N )", "Coefficient of Friction", "Depth ( Microns )", "Speed ( RPM )", "Frequency ( Hz )", "Angle ( Degree )", "Cyclic Friction Force ( N )", "Cyclic Co efficient Friction ", "Stage temperature ( Degree celcius )", "Sample temperature ( Degree celcius )", "Stroke Length ( mm )", "Scratch Speed ( mm/sec )", "Amb Humidity ( % Rh ) ", "Amb Temperature (Deg C)", "Acoustic (mV)", "Mx (Nm)", "My (Nm)", "Mz (Nm)", "Humidity ( % Rh )", "Sliding Distance (mm)", "Wear Track Diameter (mm)", "Fx(N)", "Fy(N)", "MTM BallSpeed (RPM)", "MTM DiscSpeed (RPM)", "Entrainment Speed", "Slide Role", "Slip(%)", "Rotary Speed (m/sec)", "MTM Ball Speed (m/sec)", "MTM Disc Speed (m/sec)", "ECR (ohms)"]
  in  "Y-AXIS":u16(ring) items=["None", "Time ( Sec )", "Normal Load ( N )", "Frictional Force ( N )", "Coefficient of Friction", "Depth ( Microns )", "Speed ( RPM )", "Frequency ( Hz )", "Angle ( Degree )", "Cyclic Friction Force ( N )", "Cyclic Co efficient Friction ", "Stage temperature ( Degree celcius )", "Sample temperature ( Degree celcius )", "Stroke Length ( mm )", "Scratch Speed ( mm/sec )", "Amb Humidity ( % Rh ) ", "Amb Temperature (Deg C)", "Acoustic (mV)", "Mx (Nm)", "My (Nm)", "Mz (Nm)", "Humidity ( % Rh )", "Sliding Distance (mm)", "Wear Track Diameter (mm)", "Fx(N)", "Fy(N)", "MTM BallSpeed (RPM)", "MTM DiscSpeed (RPM)", "Entrainment Speed", "Slide Role", "Slip(%)", "Rotary Speed (m/sec)", "MTM Ball Speed (m/sec)", "MTM Disc Speed (m/sec)", "ECR (ohms)"]
  out "XY Graph":cluster{"Array 2":dbl[], "Array 2":dbl[]}[](graph) caption="XY Graph 20"
  out "VARIANCE":dbl=-0.0 format="%0.2f"
  out "SD":dbl=-0.0 format="%.3f"
  out "MEAN":dbl format="%.3f"
  out "VARIANCE":dbl=-0.0 format="%0.2f"
  out "SD":dbl=-0.0 format="%.3f"
  out "MEAN":dbl format="%.3f"
  out "VARIANCE":dbl=-0.0 format="%0.2f"
  out "SD":dbl=-0.0 format="%.3f"
  out "MEAN":dbl format="%.3f"
  out "VARIANCE":dbl=-0.0 format="%0.2f"
  out "SD":dbl=-0.0 format="%.3f"
  out "MEAN":dbl format="%.3f"
  in  "Analysis Home new":bool
  out "File 2 Discription":string="\r"
  out "File 1 Discription":string="\r"
  in  "OPEN 1":bool
  in  "OPEN 2":bool
  out "File Name 1":string
  out "File Name 2":string
  in  "Refresh 2":bool
  in  "OPEN 3":bool
  out "File Name 3":string
  out "File Name 4":string
  in  "OPEN 4":bool
  out "File 4 Discription":string="\r"
  out "File 3 Discription":string="\r"
  in  "File Format":u16(ring) items=["csv", "txt", "duf"]
  in  "Export":bool
  in  "Report":bool
  in  "Password":string
  in  "Home Service":bool
  in  "Advanced Setting":bool
  in  "About Tab":enum32{"Primary"}(tab)
  in  "ECR Port:":refnum<visa-resource-name>="COM10"
  in  "Ramp Port:":refnum<visa-resource-name>="COM10"
  in  "Temp Modbus:":refnum<visa-resource-name>="COM14"
  in  "Humidity Port:":refnum<visa-resource-name>="COM10"
  in  "Edit Gain Constants":bool
  in  "Save Gain Constants":bool
  in  "Service About":bool
  # "1. Test Identification & Global Setup"
  # "2. Step Configurations & Timing"
  # "Step 1 Configuration: TRACTION Step"
  # "SET JOG SPEED"
  # "%"
  # "NOTE: This operation needs to be done only when the machine is ON."
  # "Steps 2+ Configuration: STRIBECK Steps"
  # "ohms"
  # "Upper Drive (Ball)"
  # "Lower Drive (Disc)"
  # "Variable"
  # "load Aquisition off"
  # "load Aquisition On"
  # "Configuration"
  # "Limits for Heave Surge and Sway"
  # "Modules Offset Parameters"
  # "Counts-Distance Calculator"
  # "File Name :"
  # "Ensure the traction module is aligned\n horizontally with the stage before ENABLE."
  # "JOG MODE"
  # "Module Selection"
  # "Positioning Control"
  # "Connect the controller\ncable to M3"
  # "Environment"
  # "Sensors"
  # "Data Points"
  # "Data Points"
  # "Data Points"
  # "Data Points"
  # "Data Points"
  # "Data Points"
  # "Data Points"
  # "LAB-IQ 150 / UNITEST / WO2456 / UT150  v05 / AUGUST 2025"
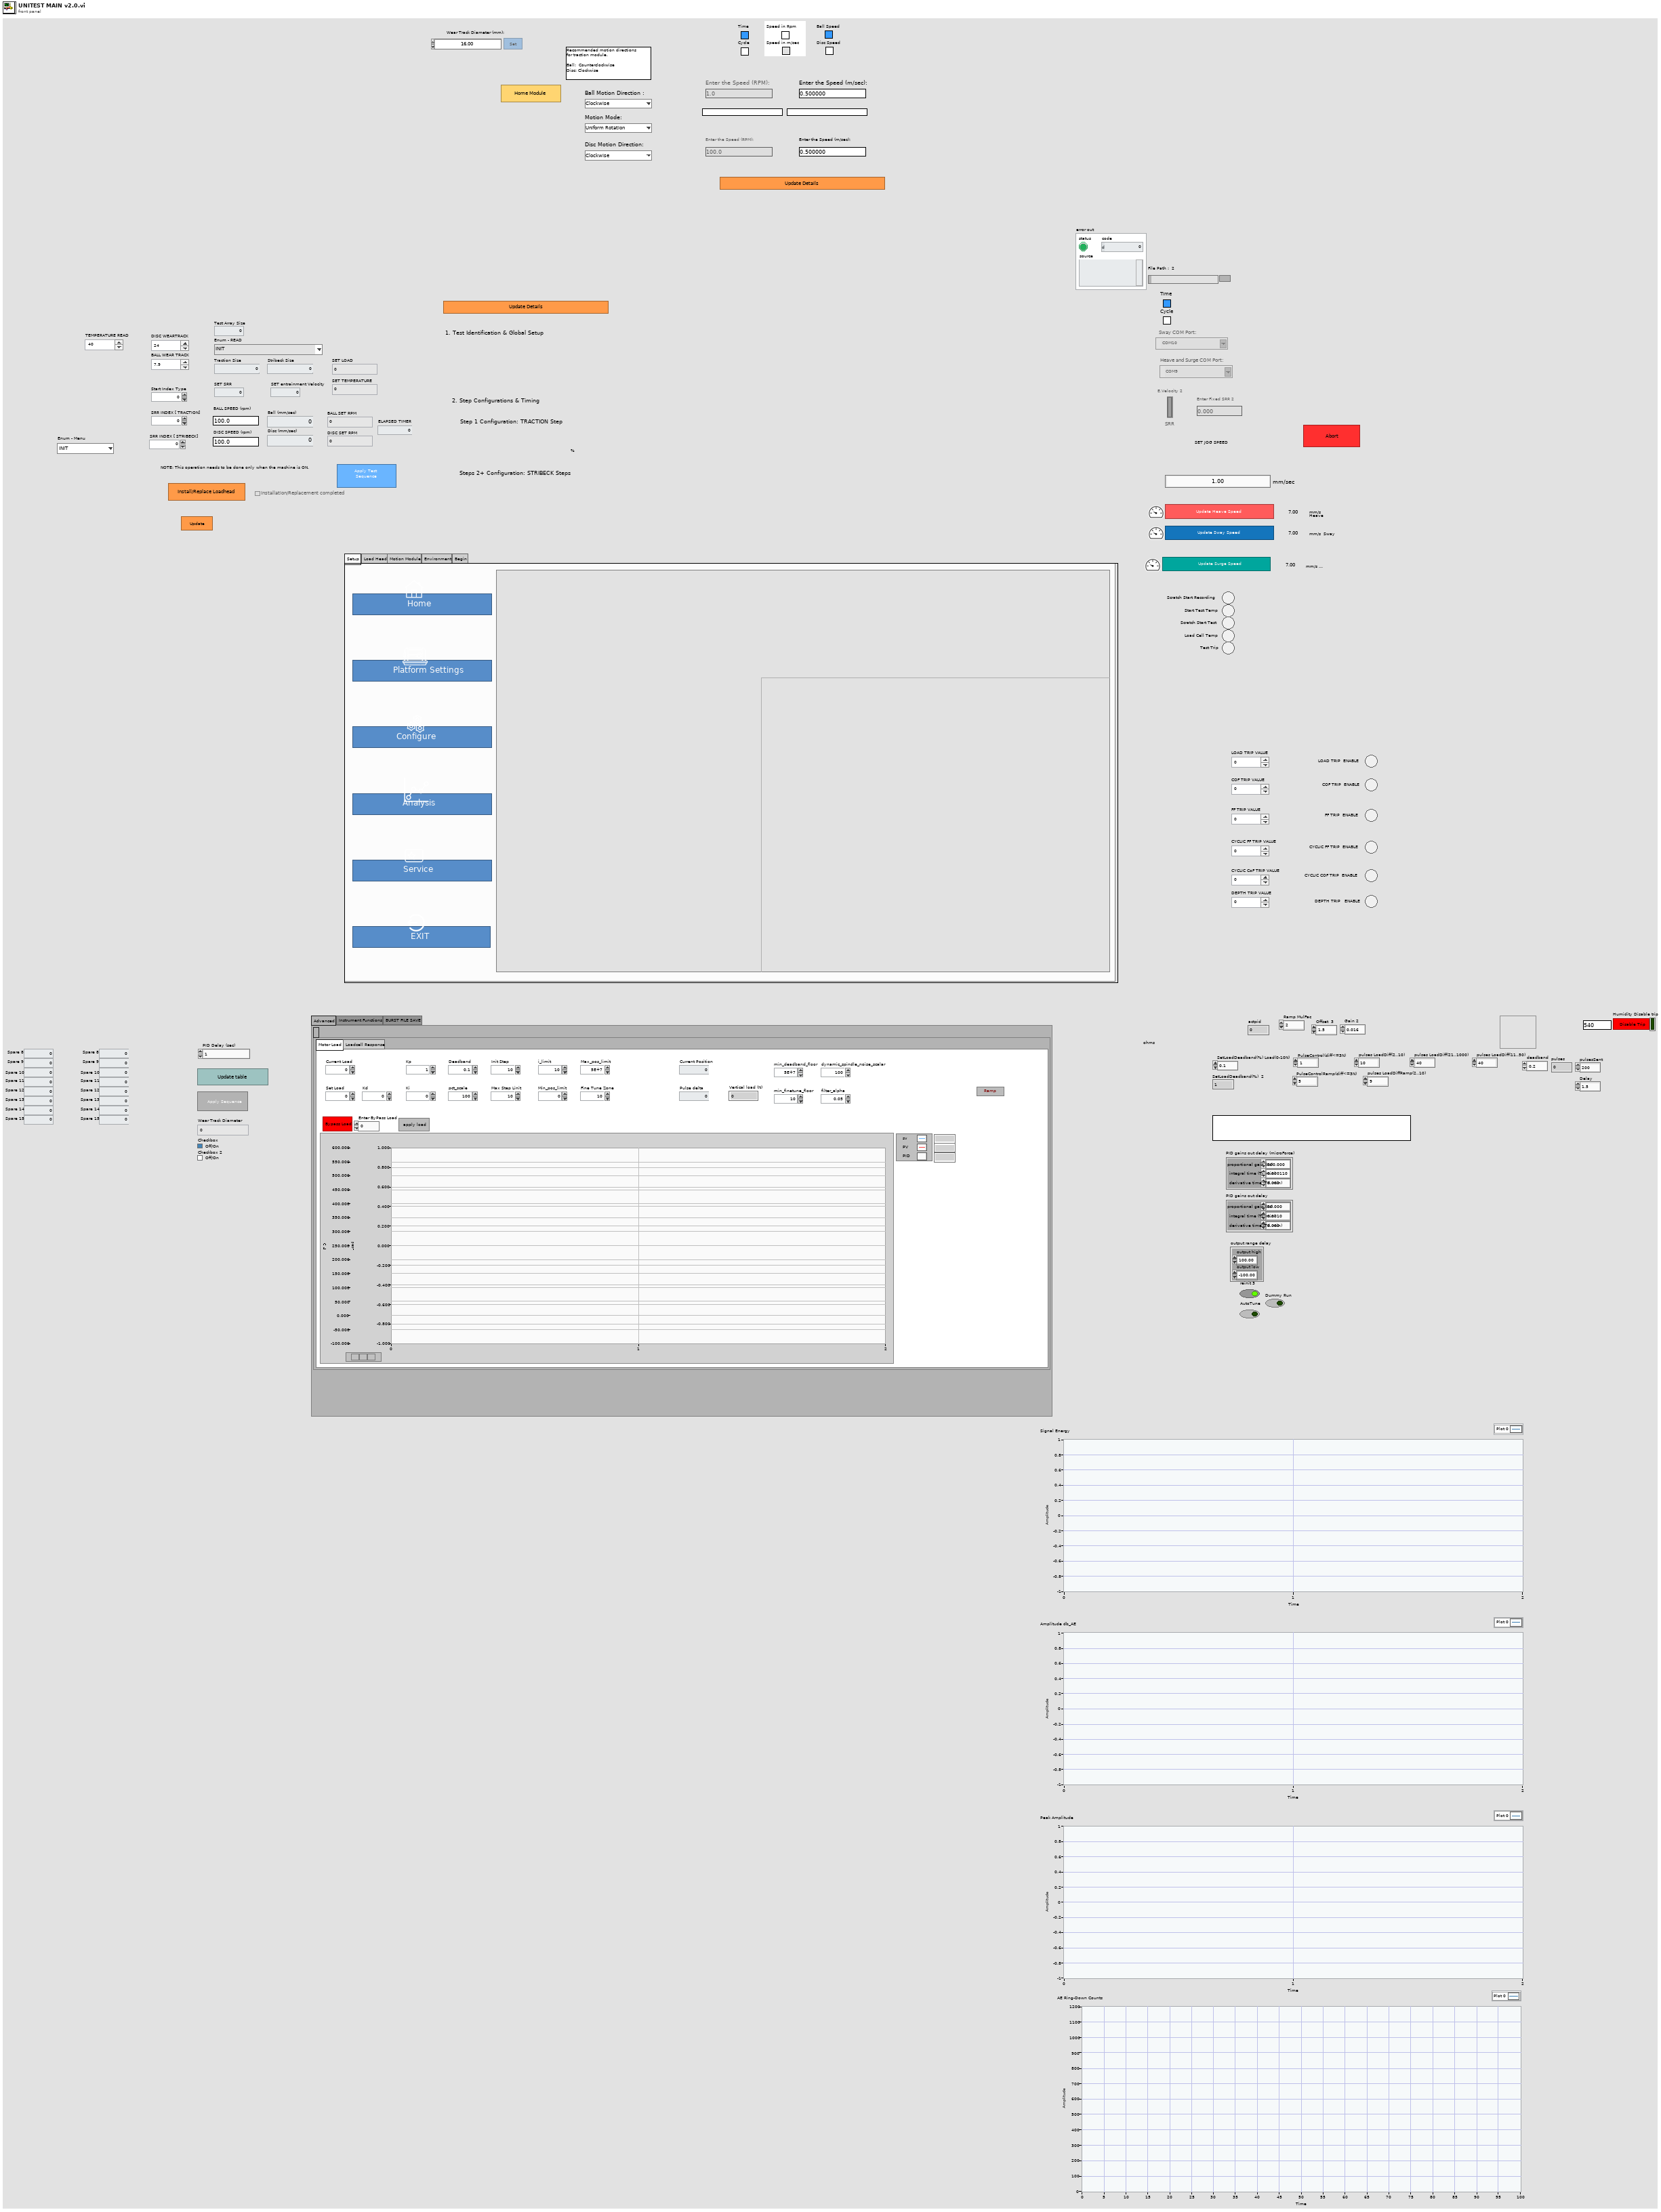
[diagram p1: front panel]
types:
  T1 = typedef "Traction Receipe Enum.ctl" = enum16{"INIT", "START", "TRACTION", "STRIBECK", "MAIN INDEX INCREMENT", "TEMPERATURE SET", "TEMPERATURE REACH", "CHURNING START", "CHURNING STOP", "LOAD", "LOAD REACHED", "SRR SET", "SRR WAIT", "SRR INCREMENT", "SPEED SET", "SPEED WAIT", "SPEED INCREMENT", "UNLOAD", "CLOSE"}
  T2 = enum32{"Uniform Rotary", "Speed Sequence", "SpeedRamp"}
  T3 = cluster{"proportional gain (Kc)":dbl, "integral time (Ti, min)":dbl, "derivative time (Td, min)":dbl}
  T4 = enum32{"Advanced", "Motor", "Depth_graph", "UIO Communicator", "Add to list parametrs", "Instrument Functions", "BURST FILE SAVE"}
  T5 = enum32{"LRM heating", "FBT_Heating", "Motor Load", "Loadcell Response", "Voice Load", "Step loading and speed ", "Depth"}
  T6 = cluster{"Sequence ID":u32, "Target Gain":u32, "Target Filter":u32, "Spare 1":u32, "Spare 2":u32, "Spare 3":u32, "Spare 4":u32, "Spare 5":u32}
  T7 = cluster{"Sequence ID":u32, "Timestamp":u32, "System Status":u32, "Peak Amplitude":sgl, "Amplitude dB_AE":sgl, "AE Ring-Down Counts":u32, "Signal Energy":sgl, "Spare 1":u32}
  T8 = enum32{"Setup", "Load Head", "Motion Module", "Environment", "Begin"}
  T9 = enum32{"Details", "PlatformSetting", "Analysis", "HOME"}
  T10 = enum32{"Constant", "Ramp", "Step", "Indentation"}
  T11 = enum32{"Uniform Rotation", "Angular Oscillation", "Speed Ramp", "Speed Step"}
  T12 = enum32{"  Acquire  ", "Compare Files Rot", "About", "Service"}
  T13 = enum32{"Coefficient of Friction ", "Friction Force (N)", "Cyclic Friction Force (N)", "Cyclic Coefficient of Friction "}
  T14 = enum32{"Speed", "Temperature", "ECR", "Acoustic Emission", "Humidity", "Sliding Distance"}
  T15 = typedef "LAB-IQ UI Data.ctl" = cluster{"Main Home Screen":cluster{"GUI":refnum<vi>, "Platform Settings":refnum<vi>, "Configure":refnum<vi>, "Home":refnum<vi>, "EXIT":refnum<vi>, "service 2":refnum<vi>, "MainPage":refnum<vi>, "Analysis":refnum<vi>}, "Platform Settings":cluster{"mm/s  Surge":refnum<vi>, "Update Surge Speed":refnum<vi>, "Drive Error":refnum<vi>, "Disable Axis Jog Soft Limits":refnum<vi>, "mm/s  Sway":refnum<vi>, "Sway and Surge COM Status":refnum<vi>, "Heave COM Status":refnum<vi>, "Enable Platform":refnum<vi>, "Surge Forward Main":refnum<vi>, "Sway Right Main":refnum<vi>, "Sway Left Main":refnum<vi>, "Heave Down Main":refnum<vi>, "Heave Up main":refnum<vi>, "Update Sway Speed":refnum<vi>, "Update Heave Speed":refnum<vi>, "mm/s Heave":refnum<vi>, "mm/sec":refnum<vi>, "mm":refnum<vi>, "Surge Backward Main":refnum<vi>}, "Analysis Screen":cluster{"Analysis Home":refnum<vi>, "Surface Analysis":refnum<vi>, "Imaging":refnum<vi>, "Image Analysis":refnum<vi>, "Post Analysis":refnum<vi>}, "Config Screen":cluster{"Select Load Head":refnum<vi>, "Notes :":refnum<vi>, "FILE":refnum<vi>, "Sample ID :":refnum<vi>, "Operator ID :":refnum<vi>, "Operator Name :":refnum<vi>, "Auto":refnum<vi>}, "Motion Module":cluster{"zNL":refnum<vi>, "NL disp":refnum<vi>, "Rotary Tab":refnum<vi>, "Motion Direction:  3":refnum<vi>, "E.Velocity 2":refnum<vi>, "e.v/ssr 2":refnum<vi>, "Enter Fixed E.Velocity 2":refnum<vi>, "Enter Final SRR 2":refnum<vi>, "Enter initial SRR 2":refnum<vi>, "Enter Fixed SRR 2":refnum<vi>, "Enter the Final E.Velocity (m/s) 2":refnum<vi>, "Enter initial E.Velocity (m/s) 2":refnum<vi>, "Final Speed (RPM) 3":refnum<vi>, "Initial Speed (RPM) 2":refnum<vi>, "Enter the Final Velocity (m/s) 3":refnum<vi>, "Enter initial Velocity (m/s)  3":refnum<vi>, "Ramp Up 2":refnum<vi>, "TEST SELECTION":refnum<vi>, "SPEED SELECTION : ":refnum<vi>, "Angular Oscillation Set":refnum<vi>, "Traction":refnum<vi>, "Step Speed":refnum<vi>, "StepTable For Load-Speed":refnum<vi>, "StepTable For Speed":refnum<vi>, "Surge Forward MM":refnum<vi>, "Surge Backward MM":refnum<vi>, "M3 Image":refnum<vi>, "String 39":refnum<vi>, "Sway Left MM":refnum<vi>, "Sway Right MM":refnum<vi>, "Disable Axis Jog Soft Limits":refnum<vi>, "mm":refnum<vi>, "Heave Down MM":refnum<vi>, "Heave Up MM":refnum<vi>, "Wear Track Diameter (mm)":refnum<vi>, "Set WTD":refnum<vi>, "HomeScratch":refnum<vi>, "HomeRot":refnum<vi>, "PlaceModule":refnum<vi>, "Enter the Angle (Deg)":refnum<vi>, "Enter the Frequency (Hz)":refnum<vi>, "Motion Mode:":refnum<vi>, "LR Sway":refnum<vi>, "Rot Hor":refnum<vi>, "Scratch":refnum<vi>, "LR Cam":refnum<vi>, "MMBack":refnum<vi>, "MMNext":refnum<vi>, "Rot Ver":refnum<vi>, "Rotary Module Selection":refnum<vi>, "calculate rotary":refnum<vi>, "SPEED SELECTION : rotary":refnum<vi>, "Import 2":refnum<vi>, "Save 2":refnum<vi>, "File Path :  2":refnum<vi>, "String 45":refnum<vi>, "StepTable For Speed 3":refnum<vi>, "Enter the Speed(mm/sec)":refnum<vi>, "Enter the Speed(RPM)":refnum<vi>, "Enter Scratch Speed (mm/s):":refnum<vi>, "SwaySpeed Set":refnum<vi>, "Scartch Offset":refnum<vi>, "Motion type:":refnum<vi>, "HomeScratch 2":refnum<vi>, "Enter Scratch length (mm):":refnum<vi>, "Wear Track Diameter":refnum<vi>, "Rotary Speed Exced":refnum<vi>, "Scratch Mode":refnum<vi>, "No of Scratch":refnum<vi>}, "Environmental control":cluster{"Humidity  Status  3":refnum<vi>, "Low Temp  Status  2":refnum<vi>, "TK4 status 2":refnum<vi>, "Stage Temperature":refnum<vi>, "Sample Temperature":refnum<vi>, "Humidity (Amb)":refnum<vi>, "Clear List":refnum<vi>, "Add to list":refnum<vi>, "Wear":refnum<vi>, "Vibration":refnum<vi>, "Humidity (Chamber)":refnum<vi>, "Temperature (Chamber)":refnum<vi>, "ECR ":refnum<vi>, "Temperature (Amb)":refnum<vi>, "Microphone":refnum<vi>, "Acoustic Emission 3":refnum<vi>, "SNext":refnum<vi>, "APBack":refnum<vi>, "Enter the Temperature (°C):":refnum<vi>, "Enter the Stage \nTemperature (°C):":refnum<vi>, "Enter the Humidity (%Rh):":refnum<vi>, "Low Temp":refnum<vi>, "High Temp":refnum<vi>, "Humidity":refnum<vi>, "Sensors Picked":refnum<vi>}, "About Screen":cluster{"Password":refnum<vi>, "Home Service":refnum<vi>, "Advanced Setting":refnum<vi>, "About Tab":refnum<vi>, "ECR Port:":refnum<vi>, "Ramp Port:":refnum<vi>, "Installation/Replacement completed":refnum<vi>, "Loahead":refnum<vi>, "Heave and Surge COM Port:":refnum<vi>, "Sway COM Port:":refnum<vi>, "Temp Modbus:":refnum<vi>, "Humidity Port:":refnum<vi>, "Edit Gain Constants":refnum<vi>, "Save Gain Constants":refnum<vi>}, "Main Screen":cluster{"Main Screen Tab":refnum<vi>, "Angle and Frequency":refnum<vi>, "Stroke (mm)":refnum<vi>, "Angle (Deg)":refnum<vi>, "Main Speed Tab":refnum<vi>, "MTM MOTOR DISPLAY":refnum<vi>, "Disc Speed (m/sec)":refnum<vi>, "Ball Speed (m/sec)":refnum<vi>, "Disc Speed (RPM)":refnum<vi>, "Ball Speed (RPM)":refnum<vi>, "SPEED TAB":refnum<vi>, "Speed (m/sec)":refnum<vi>, "Set Speed (m/sec)":refnum<vi>, "Speed (RPM)":refnum<vi>, "Set Speed":refnum<vi>, "Time Tab":refnum<vi>, "Time ( HH:MM:SS ) 2":refnum<vi>, "Test Duration":refnum<vi>, "Test Duration 4":refnum<vi>, "TEST CYCLE":refnum<vi>, "TOTAL CYCLES":refnum<vi>, "Set Load (N)":refnum<vi>, "Temp Tabs":refnum<vi>, "Heater":refnum<vi>, "TK4 status":refnum<vi>, "ChamberTemp":refnum<vi>, "SetTmp":refnum<vi>, "Controller  Status":refnum<vi>, "ChamberTemp 2":refnum<vi>, "SetTmp 2":refnum<vi>, "Controller  Status 2":refnum<vi>, "ChamberTemp 3":refnum<vi>, "SetTmp 3":refnum<vi>, "Cooling":refnum<vi>, "Load Communication":refnum<vi>, "Ambient \nTemperature":refnum<vi>, "HumCOMStatus":refnum<vi>, "Ambient\n Humidity":refnum<vi>, "Freq (Hz)":refnum<vi>, "Load En":refnum<vi>, "NLt":refnum<vi>, "zNL 2":refnum<vi>, "Humidity On":refnum<vi>, "humidity disp":refnum<vi>, "Set Humidity":refnum<vi>, "NL disp 2":refnum<vi>, "Humidity On 2":refnum<vi>, "humidity disp 2":refnum<vi>, "Set Humidity 2":refnum<vi>, "NL disp 3":refnum<vi>, "AppLoadSeq scratch":refnum<vi>, "Stop Scratch":refnum<vi>, "ClrLog":refnum<vi>, "Trip Log":refnum<vi>, "STOP":refnum<vi>, "Start Test":refnum<vi>, "Test status":refnum<vi>, "AR Led":refnum<vi>, "Data":refnum<vi>, "Health":refnum<vi>, "Sway COM Status":refnum<vi>, "Heave COM Status":refnum<vi>, "Grp Tab":refnum<vi>, "Sub Graph":refnum<vi>, "SD (mm)":refnum<vi>, "Siliding distance Reset Graph":refnum<vi>, "SDGp":refnum<vi>, "Humidity Reset Graph":refnum<vi>, "HumrGp":refnum<vi>, "Acoustic Emission (mV)":refnum<vi>, "Aqucostic Reset Graph":refnum<vi>, "gACQUOS":refnum<vi>, "ECR RESET":refnum<vi>, "ECR":refnum<vi>, "Temperature Reset":refnum<vi>, "Acoustic Emission (mV) 2":refnum<vi>, "Aqucostic Reset Graph 2":refnum<vi>, "gACQUOS 2":refnum<vi>, "ECR RESET 2":refnum<vi>, "ECR 2":refnum<vi>, "Temperature Reset 2":refnum<vi>, "Temperature (deg c)":refnum<vi>, "Speed Reset Graph":refnum<vi>, "Speed Tab":refnum<vi>, "MTM DISC  SPEED":refnum<vi>, "MTM BALL SPEED":refnum<vi>, "speed mm/sec":refnum<vi>, "Hymidity":refnum<vi>, "Humidity Disable trip":refnum<vi>, "CoF Trip  2":refnum<vi>, "Depth Trip":refnum<vi>, "Weart Deapth":refnum<vi>, "Depth Reset Graph":refnum<vi>, "Weart":refnum<vi>, "Depthz":refnum<vi>, "Depth (µm)":refnum<vi>, "WearGp":refnum<vi>, "NL Trip 2":refnum<vi>, "Load pid":refnum<vi>, "Load Disable Trip":refnum<vi>, "Load Reset Graph":refnum<vi>, "NL Display 4":refnum<vi>, "Main Chart 3":refnum<vi>, "BACK":refnum<vi>, "Depth Trip 2":refnum<vi>, "COF TRIP ":refnum<vi>, "Friction Force (N)":refnum<vi>, "FF Reset Graph":refnum<vi>, "FF Disable Trip":refnum<vi>, "FF TRIP":refnum<vi>, "COF Disable Trip":refnum<vi>, "COF Reset Graph":refnum<vi>, "Start Test Temp":refnum<vi>, "zFF":refnum<vi>, "Friction Force (N) Graph":refnum<vi>, "Coefficient of Friction":refnum<vi>, "Scratch Start Test":refnum<vi>, "FF Tab":refnum<vi>, "Cyclic Friction Force (N)":refnum<vi>, "CZ FF":refnum<vi>, "Cyclic Friction Force (N) Graph":refnum<vi>, "Cyclic Coefficient of Friction":refnum<vi>, "Cyclic FF TRIP":refnum<vi>, "Cyclic FF Disable Trip":refnum<vi>, "cyclic COF Disable Trip":refnum<vi>, "cyclic COF TRIP":refnum<vi>, "cyclic COF Reset Graph":refnum<vi>, "Cyclic FF Reset Graph":refnum<vi>, "Test Trip":refnum<vi>, "Multi Scratch Pass":refnum<vi>, "Scratch Start Recording":refnum<vi>}, "Loading":cluster{"Indentation":refnum<vi>, "Reference Sample":refnum<vi>, "Load Cell Communication Slide":refnum<vi>, "com 3":refnum<vi>, "com":refnum<vi>, "DecaForce COM Status":refnum<vi>, "Update":refnum<vi>, "Clear 3":refnum<vi>, "seq":refnum<vi>, "Stribeck table":refnum<vi>, "Stribeck Table  For loading":refnum<vi>, "Loading Mode":refnum<vi>, "Enter the Final Load (N)":refnum<vi>, "Enter the CoF Trip":refnum<vi>, "Enter the Friction Force Trip":refnum<vi>, "Enter the Normal load Trip":refnum<vi>, "Enter the Load  (N)":refnum<vi>, "KiloForce":refnum<vi>, "DecaForce ":refnum<vi>, "MicroForce":refnum<vi>, "LHBack":refnum<vi>, "LHNext":refnum<vi>, "Enter the Loading Rate (N/min)":refnum<vi>, "Message":refnum<vi>, "Warning 2":refnum<vi>, "SSP 0.75":refnum<vi>, "SSP 0.5":refnum<vi>, "SSP 0.3":refnum<vi>, "Warning":refnum<vi>, "gui GIF":refnum<vi>, "Communication is established":refnum<vi>, "AppLoad 4":refnum<vi>, "Multipoint":refnum<vi>, "Load Selection":refnum<vi>}, "PID":cluster{"Ramp MulFac":refnum<vi>, "pulses LoadDiffRamp(2..10)":refnum<vi>, "PulseControlRamp(diff<=3N)":refnum<vi>, "SetLoadDeadband(%) Load(0-10N)":refnum<vi>, "PID gains out delay (microForce)":refnum<vi>, "Ramp":refnum<vi>, "Gain 2":refnum<vi>, "pulses LoadDiff(2..10)":refnum<vi>, "pulses LoadDiff(11..50)":refnum<vi>, "PulseControl(diff<=3N)":refnum<vi>, "SetLoadDeadband(%)  2":refnum<vi>, "Dummy Run":refnum<vi>, "Vertical load (N)":refnum<vi>, "AutoTune":refnum<vi>, "Offset 3 ":refnum<vi>, "apply load":refnum<vi>, "Offset  3":refnum<vi>, "apply load 2":refnum<vi>, "Enter ByPass Load":refnum<vi>, "reinit 3":refnum<vi>, "output range delay":refnum<vi>, "PID gains out delay":refnum<vi>, "Bypass Load":refnum<vi>, "pulsesSent":refnum<vi>, "pulses ":refnum<vi>, "actpid":refnum<vi>, "gFF Rot":refnum<vi>, "pulses LoadDiff(21..1000)":refnum<vi>, "Delay":refnum<vi>, "deadband":refnum<vi>}, "Config Parameters":cluster{"Tab Control 3":refnum<vi>, "Tab Control 19":refnum<vi>, "SAMPLES":refnum<vi>, "Re-initilaize":refnum<vi>, "Filter ON/OFF":refnum<vi>, "TracHomeSurgeOffsetCounts 10MM":refnum<vi>, "TracHomeSwayOffsetCounts 10MM":refnum<vi>, "Acoustic Emission:":refnum<vi>, "Apply Filter (FF)":refnum<vi>, "Filter% 2":refnum<vi>, "Apply Filter (Load)":refnum<vi>, "Filter% ":refnum<vi>, "Sway distance (mm)":refnum<vi>, "Surge distance (mm)":refnum<vi>, "DataSavingLoopDelay(ms)":refnum<vi>, "SAVE 2":refnum<vi>, "Enter Distance":refnum<vi>, "Sway Counts:":refnum<vi>, "Distance (mm): 3":refnum<vi>, "Surge Counts:":refnum<vi>, "Distance (mm): 2":refnum<vi>, "Distance (mm):":refnum<vi>, "Heave Counts:":refnum<vi>, "LRMHomeSurgeOffsetCounts":refnum<vi>, "LRMHomeSwayOffsetCounts":refnum<vi>, "TracHomeSurgeOffsetCounts 20MM":refnum<vi>, "TracHomeSwayOffsetCounts 20MM":refnum<vi>, "RotHomeSwayOffsetCounts":refnum<vi>, "RotHomeSurgeOffsetCounts":refnum<vi>, "Heave distance":refnum<vi>, "Zmm":refnum<vi>, "Heave Pulses/mm":refnum<vi>, "Surge Pulses/mm":refnum<vi>, "Sway Pulses/mm":refnum<vi>, "Heave Pitch":refnum<vi>, "Surge Pitch":refnum<vi>, "Sway Pitch":refnum<vi>, "Heave PPR":refnum<vi>, "Surge PPR":refnum<vi>, "Sway PPR":refnum<vi>, "Tab Control 5":refnum<vi>, "Tab Control 14":refnum<vi>, "Tab Control 26":refnum<vi>, "AE":refnum<vi>, "Heave Loop Delay":refnum<vi>, "Heave PID Speed":refnum<vi>, "Surge Jog Speed":refnum<vi>, "Heave Jog Speed":refnum<vi>, "Sway Loop Delay":refnum<vi>, "Sway PID Speed":refnum<vi>, "Sway Jog Speed":refnum<vi>, "DEPTH TRIP VALUE":refnum<vi>, "LOAD TRIP VALUE":refnum<vi>, "DEPTH TRIP   ENABLE":refnum<vi>, "LOAD TRIP  ENABLE":refnum<vi>, "CYCLIC FF TRIP VALUE":refnum<vi>, "FF TRIP VALUE":refnum<vi>, "CYCLIC CoF TRIP VALUE":refnum<vi>, "COF TRIP VALUE":refnum<vi>, "CYCLIC COF TRIP  ENABLE":refnum<vi>, "CYCLIC FF TRIP  ENABLE":refnum<vi>, "FF TRIP  ENABLE":refnum<vi>, "COF TRIP  ENABLE":refnum<vi>, "JOG TRIP LOAD VALUE (N)":refnum<vi>}, "Loading Com Port":cluster{"ClearAll":refnum<vi>, "Mz(Nm)":refnum<vi>, "My(Nm)":refnum<vi>, "Mx(Nm)":refnum<vi>, "Save Dwell":refnum<vi>, "Mx ":refnum<vi>, "My ":refnum<vi>, "Mz":refnum<vi>, "Fx(N)":refnum<vi>, "Fy(N)":refnum<vi>, "Fz(N)":refnum<vi>, "ZeroAll":refnum<vi>, "Acq Delay (ms)":refnum<vi>, "Burst Delay (ms)":refnum<vi>, "model":refnum<vi>, "SN":refnum<vi>, "FFx(N)":refnum<vi>, "Sensor IP":refnum<vi>, "Port":refnum<vi>, "FFy(N)":refnum<vi>, "Load(N)":refnum<vi>, "delete Handle":refnum<vi>, "Create Handle":refnum<vi>, "ft_data":refnum<vi>, "ft_range":refnum<vi>, "ft_data 2":refnum<vi>, "stop 6":refnum<vi>, "running_flag":refnum<vi>, "ft_udp_handle":refnum<vi>, "get-data-return":refnum<vi>, "get-range-return":refnum<vi>, "zero-return":refnum<vi>, "filter-return":refnum<vi>, "initial-return":refnum<vi>, "deleteHandle-result":refnum<vi>, "Load Cell Temp":refnum<vi>}, "Heave AND Surge":cluster{"SURGE POSE":refnum<vi>, "error out Read":refnum<vi>, "HEAVE POSE":refnum<vi>, "State":refnum<vi>, "Homed":refnum<vi>, "Sequence ID":refnum<vi>, "error out Write":refnum<vi>, "faultCode":refnum<vi>, "Ack ID":refnum<vi>, "SPEED":refnum<vi>, "Distance":refnum<vi>, "Mode Command":refnum<vi>, "Heave and Surge Read":refnum<vi>, "Read Heave Temp":refnum<vi>, "Spare 15":refnum<vi>, "Spare 14":refnum<vi>, "Spare 13":refnum<vi>, "Spare 12":refnum<vi>, "Spare 11":refnum<vi>, "Spare 10":refnum<vi>, "Spare 9":refnum<vi>, "Spare 8":refnum<vi>, "Spare 7":refnum<vi>, "Spare 6":refnum<vi>, "Spare 5":refnum<vi>, "Spare 4":refnum<vi>, "Spare 2":refnum<vi>, "Spare 1":refnum<vi>, "Node Id":refnum<vi>, "Spare 3":refnum<vi>, "SPARE 4":refnum<vi>, "SPARE 3":refnum<vi>, "SPARE 2":refnum<vi>, "SPARE 1":refnum<vi>, "fwMajor":refnum<vi>, "fwMinor":refnum<vi>, "Manual Write":refnum<vi>, "Heave and Surge Write":refnum<vi>, "SPARE 5":refnum<vi>, "Reserved ":refnum<vi>, "SPARE 8":refnum<vi>, "SPARE 6":refnum<vi>, "SPARE 7":refnum<vi>, "SPARE 17":refnum<vi>, "SPARE 16":refnum<vi>, "SPARE 15":refnum<vi>, "SPARE 14":refnum<vi>, "SPARE 13":refnum<vi>, "SPARE 12":refnum<vi>, "SPARE 11":refnum<vi>, "SPARE 10":refnum<vi>, "SPARE 9":refnum<vi>, "System UPTIME":refnum<vi>, "Missed Packets":refnum<vi>, "faultCode Surge Right":refnum<vi>, "faultCode Surge Left":refnum<vi>, "faultCode Heave":refnum<vi>}, "New PID LOGIC":cluster{"Fine Tune Zone":refnum<vi>, "PID SDelay":refnum<vi>, "Max_pos_limit":refnum<vi>, "Min_pos_limit":refnum<vi>, "i_limit":refnum<vi>, "pct_scale":refnum<vi>, "Deadband":refnum<vi>, "Kd":refnum<vi>, "Ki":refnum<vi>, "Kp":refnum<vi>, "Current Position":refnum<vi>, "Set Load":refnum<vi>, "Current Load":refnum<vi>, "Pulse delta":refnum<vi>, "Init Step":refnum<vi>, "Max Step Linit":refnum<vi>, "min_deadband_floor":refnum<vi>, "dynamic_spindle_noise_scalar":refnum<vi>, "min_finetune_floor":refnum<vi>, "filter_alpha":refnum<vi>}, "SWAY ":cluster{"fwMajor":refnum<vi>, "Homed":refnum<vi>, "Rotary POSE":refnum<vi>, "State":refnum<vi>, "SWAY POSE":refnum<vi>, "Ack ID":refnum<vi>, "faultCode":refnum<vi>, "Node Id":refnum<vi>, "fwMinor":refnum<vi>, "Spare 6":refnum<vi>, "Spare 5":refnum<vi>, "Spare 4":refnum<vi>, "Spare 3":refnum<vi>, "Spare 2":refnum<vi>, "Spare 1":refnum<vi>, "Spare 7":refnum<vi>, "SPARE  5":refnum<vi>, "error out Write  SWAY ":refnum<vi>, "error out Read SWAY ":refnum<vi>, "Manual Write SWAY ":refnum<vi>, "SWAY WRITE":refnum<vi>, "SPARE  4":refnum<vi>, "SPARE  3":refnum<vi>, "SPARE 2":refnum<vi>, "SPARE 1":refnum<vi>, "Spare 15":refnum<vi>, "Spare 14":refnum<vi>, "Spare 13":refnum<vi>, "Spare 12":refnum<vi>, "Spare 11":refnum<vi>, "Spare 9":refnum<vi>, "Spare 8":refnum<vi>, "SPEED":refnum<vi>, "Distance":refnum<vi>, "Mode Command":refnum<vi>, "Sequence ID":refnum<vi>, "SWAY READ":refnum<vi>, "Spare 10":refnum<vi>, "Read SWAY Temp":refnum<vi>, "faultCode Sway ":refnum<vi>, "Missed Packets":refnum<vi>, "System UPTIME sway":refnum<vi>, "SPARE 6":refnum<vi>, "SPARE 7":refnum<vi>, "SPARE 9":refnum<vi>, "SPARE 11":refnum<vi>, "SPARE 10":refnum<vi>, "SPARE 8":refnum<vi>, "SPARE 13":refnum<vi>, "SPARE 12":refnum<vi>, "SPARE 17":refnum<vi>, "SPARE 16":refnum<vi>, "SPARE 15":refnum<vi>, "SPARE 14":refnum<vi>, "Reserved":refnum<vi>, "faultCode Rotary":refnum<vi>}, "Analysis Screen":cluster{"Analysis Home":refnum<vi>, "Refresh 2":refnum<vi>, "MEAN 4":refnum<vi>, "SD 4":refnum<vi>, "VARIANCE 4":refnum<vi>, "MEAN  3":refnum<vi>, "SD  3":refnum<vi>, "VARIANCE  3":refnum<vi>, "MEAN 2":refnum<vi>, "SD  2":refnum<vi>, "VARIANCE 2":refnum<vi>, "MEAN":refnum<vi>, "SD":refnum<vi>, "VARIANCE":refnum<vi>, "File 4 Discription":refnum<vi>, "OPEN 4":refnum<vi>, "File Name 4":refnum<vi>, "OPEN 3":refnum<vi>, "File 3 Discription":refnum<vi>, "File Name 3":refnum<vi>, "Y-AXIS":refnum<vi>, "X-AXIS":refnum<vi>, "XY Graph":refnum<vi>, "File Name 2":refnum<vi>, "File Name 1":refnum<vi>, "OPEN 2":refnum<vi>, "OPEN 1":refnum<vi>, "File 1 Discription ":refnum<vi>, "File 2 Discription":refnum<vi>, "Export":refnum<vi>, "File Format":refnum<vi>}, "Traction":cluster{"faultCode Traction 2":refnum<vi>, "faultCode Traction 1":refnum<vi>, "Missed Packets":refnum<vi>, "System UPTIME Traction":refnum<vi>, "SPARE 17":refnum<vi>, "SPARE 16":refnum<vi>, "SPARE 15":refnum<vi>, "SPARE 14":refnum<vi>, "SPARE 13":refnum<vi>, "SPARE 12":refnum<vi>, "SPARE 11":refnum<vi>, "SPARE 10":refnum<vi>, "SPARE 9":refnum<vi>, "SPARE 8":refnum<vi>, "SPARE 7":refnum<vi>, "SPARE 6":refnum<vi>, "Reserved":refnum<vi>, "SPARE  5":refnum<vi>, "Manual Write TRACTION":refnum<vi>, "TRACTION WRITE":refnum<vi>, "SPARE  4":refnum<vi>, "SPARE  3":refnum<vi>, "SPARE 2":refnum<vi>, "SPARE 1":refnum<vi>, "Spare 7":refnum<vi>, "Spare 6":refnum<vi>, "Spare 5":refnum<vi>, "Spare 4":refnum<vi>, "Spare 2":refnum<vi>, "Spare 1":refnum<vi>, "Node Id":refnum<vi>, "Read TRACTION Temp":refnum<vi>, "fwMinor":refnum<vi>, "fwMajor":refnum<vi>, "faultCode":refnum<vi>, "TRACTION POSE":refnum<vi>, "TRACTION POSE 2":refnum<vi>, "Homed":refnum<vi>, "State":refnum<vi>, "Ack ID":refnum<vi>, "SPEED":refnum<vi>, "Distance":refnum<vi>, "Mode Command":refnum<vi>, "Sequence ID":refnum<vi>, "error out Read TRACTION":refnum<vi>, "error out Write  TRACTION":refnum<vi>, "TRACTION READ":refnum<vi>, "Spare 3":refnum<vi>}, "Traction reciepe":cluster{"SRR Sweep Range (%) Stribeck":refnum<vi>, "Traction Receipe":refnum<vi>, "Total Execution Time":refnum<vi>, "Total Steps":refnum<vi>, "Duration / Step (s)  Stribeck":refnum<vi>, "STRIBECK Fixed SRR List (%)":refnum<vi>, "Duration / Step (s) Traction":refnum<vi>, "SRR Sweep Range (%) traction":refnum<vi>, "Rolling Speed (mm/s)":refnum<vi>, "Temperature Stages (°C)":refnum<vi>, "Ball Load (N)":refnum<vi>, "Lubricant Name":refnum<vi>, "Profile File Name":refnum<vi>, "SET entrainment Velocity":refnum<vi>, "Test Array Size":refnum<vi>, "SRR INDEX [ STRIBECK]":refnum<vi>, "Stribeck Size":refnum<vi>, "SET SRR":refnum<vi>, "ELAPSED TIMER ":refnum<vi>, "BALL SET RPM":refnum<vi>, "DISC SET RPM":refnum<vi>, "SET LOAD":refnum<vi>, "TEMPERATURE READ":refnum<vi>, "SET TEMPERATURE":refnum<vi>, "Traction Size":refnum<vi>, "DISC SPEED (rpm)":refnum<vi>, "BALL SPEED (rpm)":refnum<vi>, "BALL WEAR TRACK":refnum<vi>, "DISC WEARTRACK":refnum<vi>, "SRR INDEX [ TRACTION]":refnum<vi>, "Start Index Type":refnum<vi>, "Enum - Menu":refnum<vi>, "Ball (mm/sec)":refnum<vi>, "Disc (mm/sec)":refnum<vi>}, "Traction Control":cluster{"HomeTraction":refnum<vi>, "Demo Mode Display":refnum<vi>, "Traction Message":refnum<vi>, "Traction Step Update Details":refnum<vi>, "Main Tab sequence for selection":refnum<vi>, "Ramp Tab":refnum<vi>, "e.v/ssr":refnum<vi>, "Enter Fixed E.Velocity":refnum<vi>, "Enter Final SRR":refnum<vi>, "Enter initial SRR":refnum<vi>, "Enter Fixed SRR":refnum<vi>, "Enter the Final E.Velocity (m/s)":refnum<vi>, "Enter initial E.Velocity (m/s)":refnum<vi>, "Ball WTD":refnum<vi>, "E.Velocity":refnum<vi>, "Enter the Final Velocity (m/s)":refnum<vi>, "Enter initial Velocity (m/s)":refnum<vi>, "Ramp Up   Disc":refnum<vi>, "Initial DiscSpeed (RPM)":refnum<vi>, "Final Speed (RPM) Ball":refnum<vi>, "Final Speed (RPM)":refnum<vi>, "Initial Speed (RPM) Ball":refnum<vi>, "Enter the Final Velocity (m/s) Ball":refnum<vi>, "Enter initial Velocity (m/s) Ball":refnum<vi>, "Ramp Up":refnum<vi>, "ExceedBallSpeed step":refnum<vi>, "ExceedDiscSpeed":refnum<vi>, "BallSpeed Exceed Indication":refnum<vi>, "Apply":refnum<vi>, "SPEED SELECTION : MTM":refnum<vi>, "SPEED SELECTION : MTM 2":refnum<vi>, "TEST SELECTION (MTM)":refnum<vi>, "MTM Test Selection":refnum<vi>, "File Path Tab":refnum<vi>, "File Path String":refnum<vi>, "Save":refnum<vi>, "Save  2":refnum<vi>, "Import ":refnum<vi>, "File Path :":refnum<vi>, "Step Sequence Indication Tab":refnum<vi>, "Step Sequence Indication":refnum<vi>, "Calculate Step":refnum<vi>, "StepTable":refnum<vi>, "ExceedDiscSpeed  Cinstant Speed":refnum<vi>, "ExceedBallSpeed Constant":refnum<vi>, "TEST SELECTION (MTM) 2":refnum<vi>, "SPEED SELECTION : MTM 3":refnum<vi>, "MTM Test Selection 2":refnum<vi>, "Enter the Speed (m/sec): ":refnum<vi>, "Enter the Speed (m/sec):  2":refnum<vi>, "Enter the Speed (RPM):":refnum<vi>, "Lower Spped ":refnum<vi>, "Upper":refnum<vi>, "Enter the Speed (RPM):Ball":refnum<vi>, "Disc Motion Direction: ":refnum<vi>, "Ball Motion Direction :":refnum<vi>, "Motion Mode: ":refnum<vi>, "Wear Track Diameter (mm) ":refnum<vi>, "Disc Speed Indicator":refnum<vi>, "ExceedBallSpeed":refnum<vi>}, "Acquostic":cluster{"Last Config Rejected ":refnum<vi>, "rx command count":refnum<vi>, "Current Filter Id":refnum<vi>, "Isolated Gain":refnum<vi>, "DAQ Status":refnum<vi>, "error out":refnum<vi>, "error in (no error)":refnum<vi>, "Uplink Packet":refnum<vi>, "data out":refnum<vi>, "Downlink Packet":refnum<vi>, "Signal Energy":refnum<vi>, "Amplitude db_AE":refnum<vi>, "Peak Amplitude":refnum<vi>, "AE Ring-Down Counts":refnum<vi>, "Gains":refnum<vi>, "Manual Write Acquostic":refnum<vi>}}
  T16 = typedef "init queue out loop.ctl" = cluster{"UI Loop":refnum<queue>, "LOAD COM LOOP ":refnum<queue>, "SWAY MOTOR COM LOOP":refnum<queue>, "HEAVE MOTOR COM LOOP":refnum<queue>, "TEMPERATURE COM LOOP":refnum<queue>, "RAMP MOTOR COM LOOP":refnum<queue>, "ECR PORT":refnum<queue>, "HUMIDITY COM PORT":refnum<queue>, "PROGRAM LOOP":refnum<queue>, "MONITOR LOOP":refnum<queue>, "REPORT":refnum<queue>, "LOAD PID":refnum<queue>, "ACOUSTIC":refnum<queue>}
  T17 = typedef "XDNodeRunTimeDep.lvlib/timing_clust.ctl" = cluster{"Expected End [f-1]":u64, "Actual End [f-1]":u64, "Finished Late? [f-1]":bool, "Expected End [i-1]":u64, "Actual End [i-1]":u64, "Finished Late? [i-1]":bool, "Expected Start [i]":u64, "Actual Start [i]":u64, "Expected Start [f]":u64, "Actual Start [f]":u64, "Source Name":string, "Structure Name":string, "Period":i64, "Deadline":i64, "Offset":i64, "Start":i64, "Priority":i32, "Timeout":i32, "Mode":T18, "Wakeup Reason":T19, "Error":errorcluster, "Source Type":string, "Secondary Source Type":string, "Global End Time":u64, "Global Start Time":u64, "Frame Duration":u64, "Iteration Duration":u64, "Assigned CPU":i32, "I/O Scan Engine Mode":u32}
  T18 = typedef "XDNodeRunTimeDep.lvlib/nitl_modes.ctl" = enum32{"No Change", "Process missed periods, maintain original phase", "Discard missed periods, maintain original phase", "Process missed periods, ignore original phase", "Discard missed periods, ignore original phase"}
  T19 = typedef "XDNodeRunTimeDep.lvlib/wakeup.ctl" = enum32{"Normal", "Aborted", "Asynchronous wakeup", "Timing source error", "Timed loop error", "Timeout"}
  T20 = typedef "Read Main Enum.ctl" = enum16{"INIT", "READ", "RE-INIT", "CLOSE"}
  T21 = typedef "Write Main Enum.ctl" = enum16{"INIT", "WRITE", "RE-INIT", "CLOSE"}
  T22 = typedef "Heave Right enum.ctl" = enum16{"INIT", "READ", "CLOSE", "REINIT", ""}
  T23 = typedef "Heave Write enum.ctl" = enum16{"INIT", "WRITE", "CLOSE", "REINIT"}
  T24 = enum8{"Enabled", "Disabled", "Disabled and Grayed Out"}
  T25 = enum16{"INIT", "SETLOWPASSFILTER", "SETZERO", "GETSENSORINFO", "GETRANGE", "ZEROALL", "READDATA", "UNINITIAL", "DELETEHANDLE"}
  T26 = typedef "Sway Write enum.ctl" = enum16{"INIT", "WRITE", "CLOSE", "REINIT"}
  T27 = typedef "Traction Write enum.ctl" = enum16{"INIT", "WRITE", "CLOSE", "REINIT"}
  T28 = typedef "Sway Right enum.ctl" = enum16{"INIT", "READ", "CLOSE", "REINIT", ""}
  T29 = typedef "Traction Read enum.ctl" = enum16{"INIT", "READ", "CLOSE", "REINIT", ""}
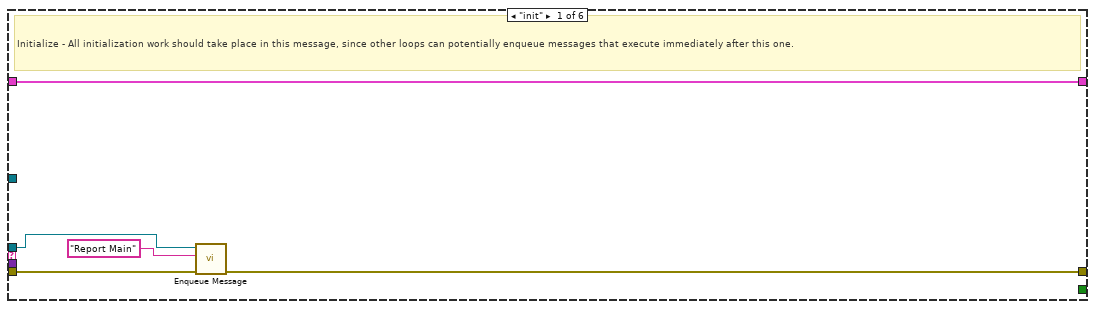
[diagram p2: hidden frame]
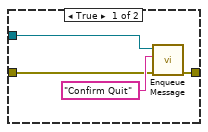
[diagram p3: hidden frame]
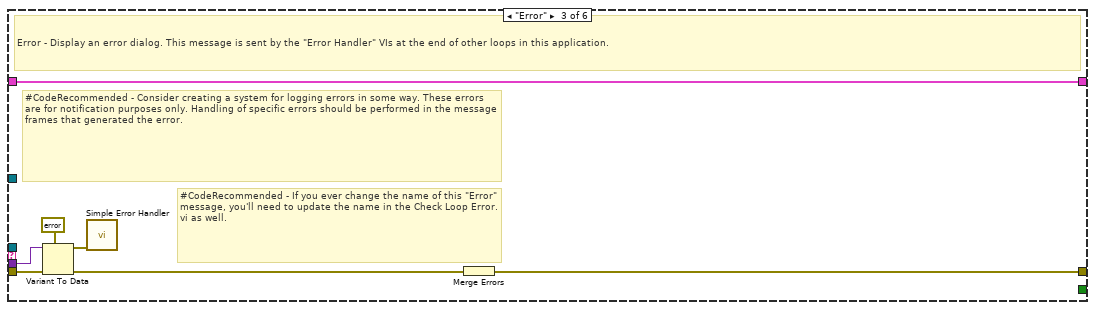
[diagram p4: hidden frame]
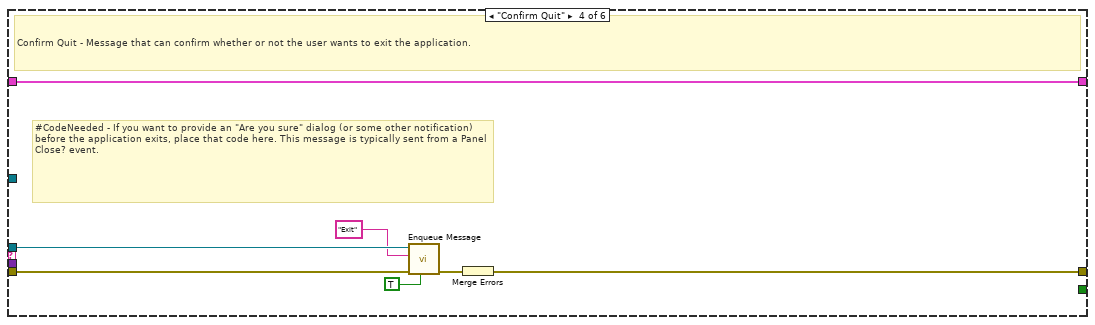
[diagram p5: hidden frame]
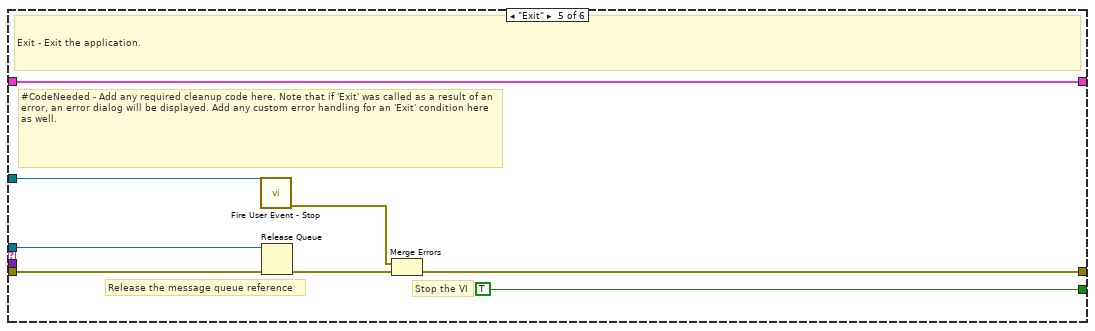
[diagram p6: hidden frame]
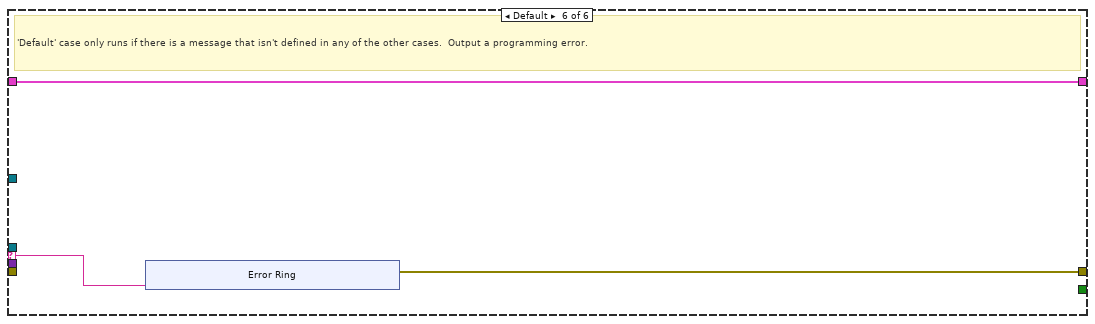
[diagram p7: hidden frame]
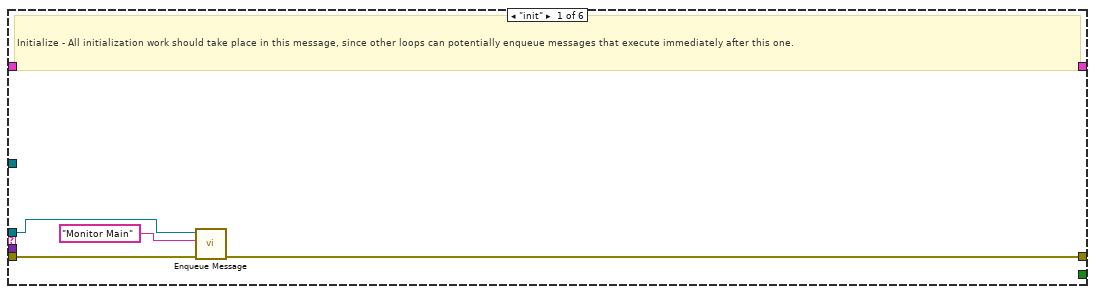
[diagram p8: hidden frame]
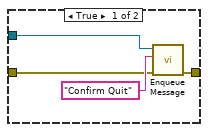
[diagram p9: hidden frame]
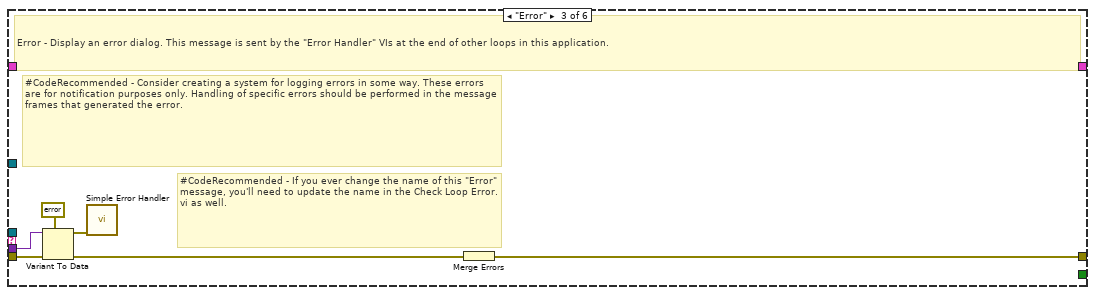
[diagram p10: hidden frame]
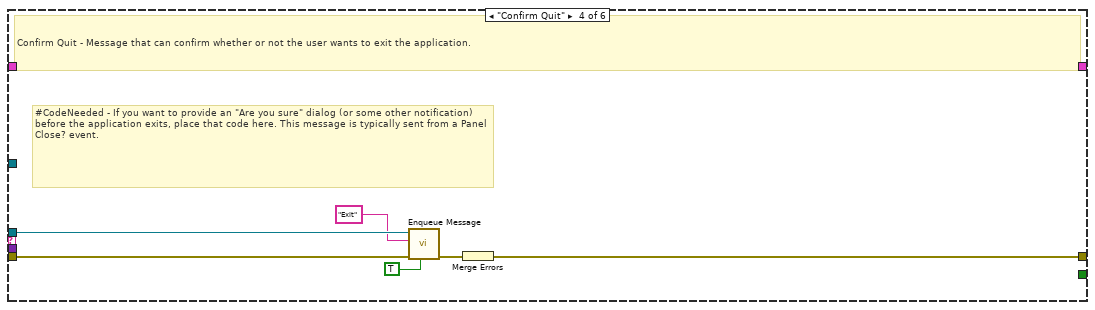
[diagram p11: hidden frame]
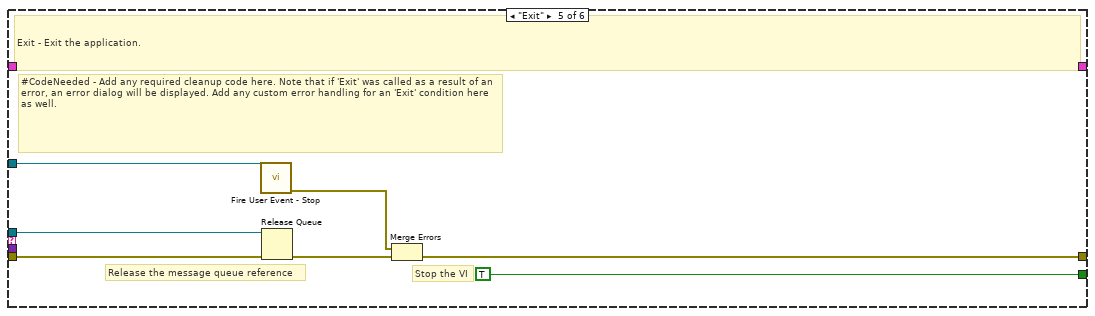
[diagram p12: hidden frame]
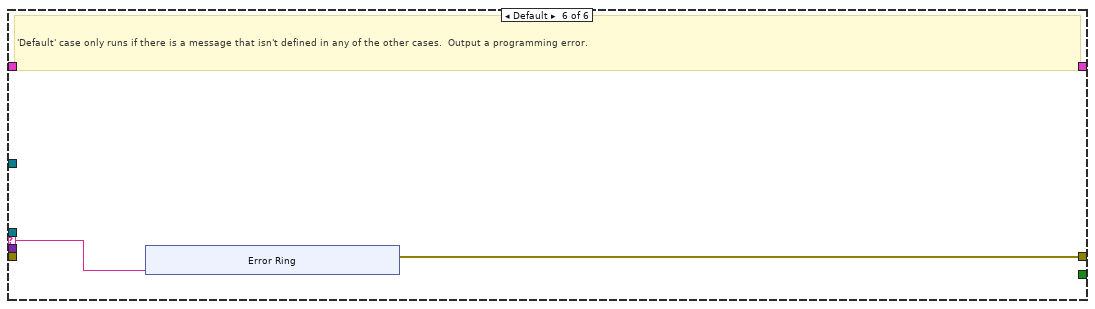
[diagram p13: hidden frame]
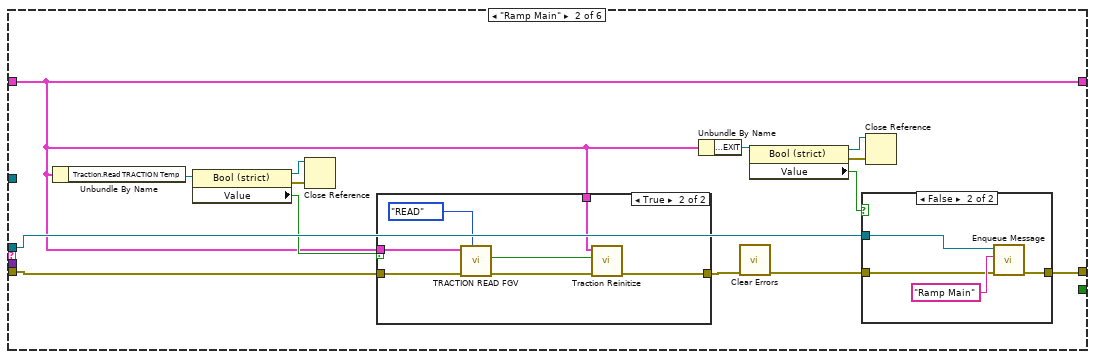
[diagram p14: hidden frame]
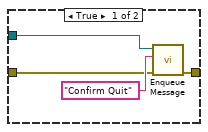
[diagram p16: hidden frame]
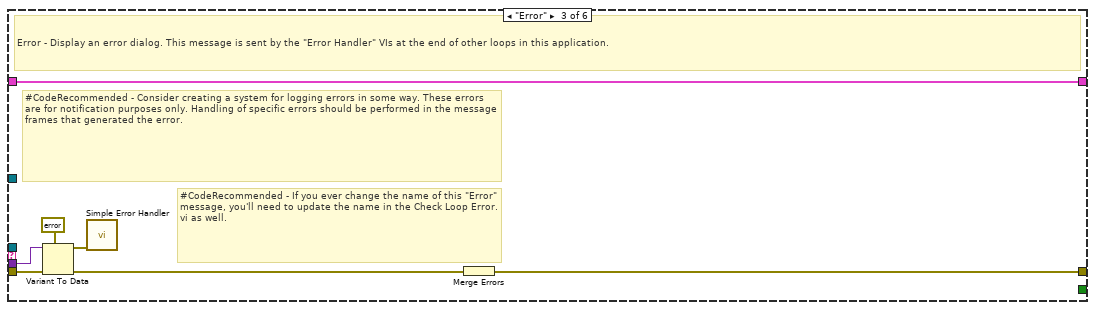
[diagram p17: hidden frame]
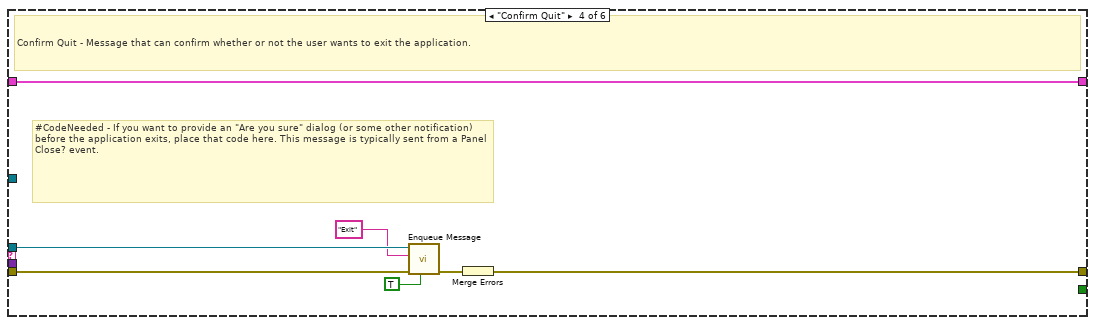
[diagram p18: hidden frame]
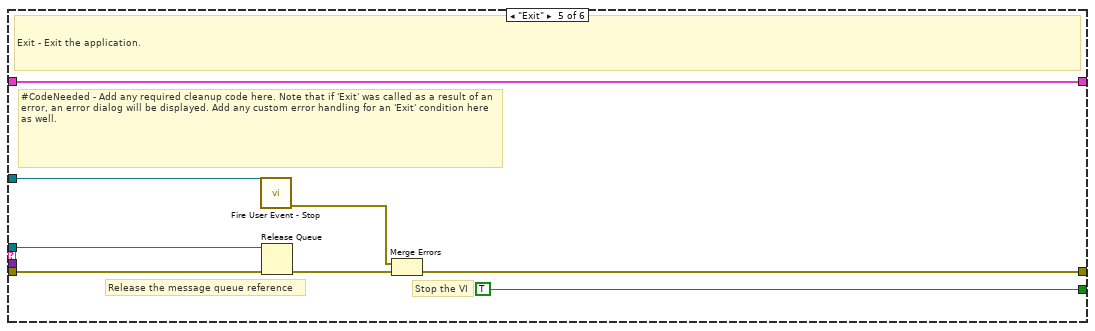
[diagram p19: hidden frame]
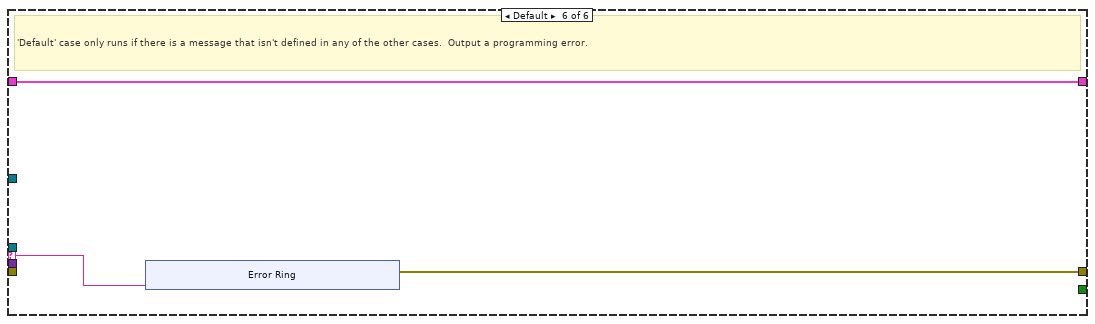
[diagram p20: hidden frame]
diagram:
  w24 = 0.0 ("prev_error_out")
  n1 = flat-sequence {
    tunnel: [w82] -> w69
    tunnel: T15 {"Main Home Screen"={"GUI"=refnum, "Platform Settings"=refnum, "Configure"=refnum, "Home"=refnum, "EXIT"=refnum, "service 2"=refnum, "MainPage"=refnum, "Analysis"=refnum}, "Platform Settings"={"mm/s  Surge"=refnum, "Update Surge Speed"=refnum, "Drive Error"=refnum, "Disable Axis Jog Soft Limits"=refnum, "mm/s  Sway"=refnum, "Sway and Surge COM Status"=refnum, "Heave COM Status"=refnum, "Enable Platform"=refnum, "Surge Forward Main"=refnum, "Sway Right Main"=refnum, "Sway Left Main"=refnum, "Heave Down Main"=refnum, "Heave Up main"=refnum, "Update Sway Speed"=refnum, "Update Heave Speed"=refnum, "mm/s Heave"=refnum, "mm/sec"=refnum, "mm"=refnum, "Surge Backward Main"=refnum}, "Analysis Screen"={"Analysis Home"=refnum, "Surface Analysis"=refnum, "Imaging"=refnum, "Image Analysis"=refnum, "Post Analysis"=refnum}, "Config Screen"={"Select Load Head"=refnum, "Notes :"=refnum, "FILE"=refnum, "Sample ID :"=refnum, "Operator ID :"=refnum, "Operator Name :"=refnum, "Auto"=refnum}, "Motion Module"={"zNL"=refnum, "NL disp"=refnum, "Rotary Tab"=refnum, "Motion Direction:  3"=refnum, "E.Velocity 2"=refnum, "e.v/ssr 2"=refnum, "Enter Fixed E.Velocity 2"=refnum, "Enter Final SRR 2"=refnum, "Enter initial SRR 2"=refnum, "Enter Fixed SRR 2"=refnum, "Enter the Final E.Velocity (m/s) 2"=refnum, "Enter initial E.Velocity (m/s) 2"=refnum, "Final Speed (RPM) 3"=refnum, "Initial Speed (RPM) 2"=refnum, "Enter the Final Velocity (m/s) 3"=refnum, "Enter initial Velocity (m/s)  3"=refnum, "Ramp Up 2"=refnum, "TEST SELECTION"=refnum, "SPEED SELECTION : "=refnum, "Angular Oscillation Set"=refnum, "Traction"=refnum, "Step Speed"=refnum, "StepTable For Load-Speed"=refnum, "StepTable For Speed"=refnum, "Surge Forward MM"=refnum, "Surge Backward MM"=refnum, "M3 Image"=refnum, "String 39"=refnum, "Sway Left MM"=refnum, "Sway Right MM"=refnum, "Disable Axis Jog Soft Limits"=refnum, "mm"=refnum, "Heave Down MM"=refnum, "Heave Up MM"=refnum, "Wear Track Diameter (mm)"=refnum, "Set WTD"=refnum, "HomeScratch"=refnum, "HomeRot"=refnum, "PlaceModule"=refnum, "Enter the Angle (Deg)"=refnum, "Enter the Frequency (Hz)"=refnum, "Motion Mode:"=refnum, "LR Sway"=refnum, "Rot Hor"=refnum, "Scratch"=refnum, "LR Cam"=refnum, "MMBack"=refnum, "MMNext"=refnum, "Rot Ver"=refnum, "Rotary Module Selection"=refnum, "calculate rotary"=refnum, "SPEED SELECTION : rotary"=refnum, "Import 2"=refnum, "Save 2"=refnum, "File Path :  2"=refnum, "String 45"=refnum, "StepTable For Speed 3"=refnum, "Enter the Speed(mm/sec)"=refnum, "Enter the Speed(RPM)"=refnum, "Enter Scratch Speed (mm/s):"=refnum, "SwaySpeed Set"=refnum, "Scartch Offset"=refnum, "Motion type:"=refnum, "HomeScratch 2"=refnum, "Enter Scratch length (mm):"=refnum, "Wear Track Diameter"=refnum, "Rotary Speed Exced"=refnum, "Scratch Mode"=refnum, "No of Scratch"=refnum}, "Environmental control"={"Humidity  Status  3"=refnum, "Low Temp  Status  2"=refnum, "TK4 status 2"=refnum, "Stage Temperature"=refnum, "Sample Temperature"=refnum, "Humidity (Amb)"=refnum, "Clear List"=refnum, "Add to list"=refnum, "Wear"=refnum, "Vibration"=refnum, "Humidity (Chamber)"=refnum, "Temperature (Chamber)"=refnum, "ECR "=refnum, "Temperature (Amb)"=refnum, "Microphone"=refnum, "Acoustic Emission 3"=refnum, "SNext"=refnum, "APBack"=refnum, "Enter the Temperature (°C):"=refnum, "Enter the Stage \nTemperature (°C):"=refnum, "Enter the Humidity (%Rh):"=refnum, "Low Temp"=refnum, "High Temp"=refnum, "Humidity"=refnum, "Sensors Picked"=refnum}, "About Screen"={"Password"=refnum, "Home Service"=refnum, "Advanced Setting"=refnum, "About Tab"=refnum, "ECR Port:"=refnum, "Ramp Port:"=refnum, "Installation/Replacement completed"=refnum, "Loahead"=refnum, "Heave and Surge COM Port:"=refnum, "Sway COM Port:"=refnum, "Temp Modbus:"=refnum, "Humidity Port:"=refnum, "Edit Gain Constants"=refnum, "Save Gain Constants"=refnum}, "Main Screen"={"Main Screen Tab"=refnum, "Angle and Frequency"=refnum, "Stroke (mm)"=refnum, "Angle (Deg)"=refnum, "Main Speed Tab"=refnum, "MTM MOTOR DISPLAY"=refnum, "Disc Speed (m/sec)"=refnum, "Ball Speed (m/sec)"=refnum, "Disc Speed (RPM)"=refnum, "Ball Speed (RPM)"=refnum, "SPEED TAB"=refnum, "Speed (m/sec)"=refnum, "Set Speed (m/sec)"=refnum, "Speed (RPM)"=refnum, "Set Speed"=refnum, "Time Tab"=refnum, "Time ( HH:MM:SS ) 2"=refnum, "Test Duration"=refnum, "Test Duration 4"=refnum, "TEST CYCLE"=refnum, "TOTAL CYCLES"=refnum, "Set Load (N)"=refnum, "Temp Tabs"=refnum, "Heater"=refnum, "TK4 status"=refnum, "ChamberTemp"=refnum, "SetTmp"=refnum, "Controller  Status"=refnum, "ChamberTemp 2"=refnum, "SetTmp 2"=refnum, "Controller  Status 2"=refnum, "ChamberTemp 3"=refnum, "SetTmp 3"=refnum, "Cooling"=refnum, "Load Communication"=refnum, "Ambient \nTemperature"=refnum, "HumCOMStatus"=refnum, "Ambient\n Humidity"=refnum, "Freq (Hz)"=refnum, "Load En"=refnum, "NLt"=refnum, "zNL 2"=refnum, "Humidity On"=refnum, "humidity disp"=refnum, "Set Humidity"=refnum, "NL disp 2"=refnum, "Humidity On 2"=refnum, "humidity disp 2"=refnum, "Set Humidity 2"=refnum, "NL disp 3"=refnum, "AppLoadSeq scratch"=refnum, "Stop Scratch"=refnum, "ClrLog"=refnum, "Trip Log"=refnum, "STOP"=refnum, "Start Test"=refnum, "Test status"=refnum, "AR Led"=refnum, "Data"=refnum, "Health"=refnum, "Sway COM Status"=refnum, "Heave COM Status"=refnum, "Grp Tab"=refnum, "Sub Graph"=refnum, "SD (mm)"=refnum, "Siliding distance Reset Graph"=refnum, "SDGp"=refnum, "Humidity Reset Graph"=refnum, "HumrGp"=refnum, "Acoustic Emission (mV)"=refnum, "Aqucostic Reset Graph"=refnum, "gACQUOS"=refnum, "ECR RESET"=refnum, "ECR"=refnum, "Temperature Reset"=refnum, "Acoustic Emission (mV) 2"=refnum, "Aqucostic Reset Graph 2"=refnum, "gACQUOS 2"=refnum, "ECR RESET 2"=refnum, "ECR 2"=refnum, "Temperature Reset 2"=refnum, "Temperature (deg c)"=refnum, "Speed Reset Graph"=refnum, "Speed Tab"=refnum, "MTM DISC  SPEED"=refnum, "MTM BALL SPEED"=refnum, "speed mm/sec"=refnum, "Hymidity"=refnum, "Humidity Disable trip"=refnum, "CoF Trip  2"=refnum, "Depth Trip"=refnum, "Weart Deapth"=refnum, "Depth Reset Graph"=refnum, "Weart"=refnum, "Depthz"=refnum, "Depth (µm)"=refnum, "WearGp"=refnum, "NL Trip 2"=refnum, "Load pid"=refnum, "Load Disable Trip"=refnum, "Load Reset Graph"=refnum, "NL Display 4"=refnum, "Main Chart 3"=refnum, "BACK"=refnum, "Depth Trip 2"=refnum, "COF TRIP "=refnum, "Friction Force (N)"=refnum, "FF Reset Graph"=refnum, "FF Disable Trip"=refnum, "FF TRIP"=refnum, "COF Disable Trip"=refnum, "COF Reset Graph"=refnum, "Start Test Temp"=refnum, "zFF"=refnum, "Friction Force (N) Graph"=refnum, "Coefficient of Friction"=refnum, "Scratch Start Test"=refnum, "FF Tab"=refnum, "Cyclic Friction Force (N)"=refnum, "CZ FF"=refnum, "Cyclic Friction Force (N) Graph"=refnum, "Cyclic Coefficient of Friction"=refnum, "Cyclic FF TRIP"=refnum, "Cyclic FF Disable Trip"=refnum, "cyclic COF Disable Trip"=refnum, "cyclic COF TRIP"=refnum, "cyclic COF Reset Graph"=refnum, "Cyclic FF Reset Graph"=refnum, "Test Trip"=refnum, "Multi Scratch Pass"=refnum, "Scratch Start Recording"=refnum}, "Loading"={"Indentation"=refnum, "Reference Sample"=refnum, "Load Cell Communication Slide"=refnum, "com 3"=refnum, "com"=refnum, "DecaForce COM Status"=refnum, "Update"=refnum, "Clear 3"=refnum, "seq"=refnum, "Stribeck table"=refnum, "Stribeck Table  For loading"=refnum, "Loading Mode"=refnum, "Enter the Final Load (N)"=refnum, "Enter the CoF Trip"=refnum, "Enter the Friction Force Trip"=refnum, "Enter the Normal load Trip"=refnum, "Enter the Load  (N)"=refnum, "KiloForce"=refnum, "DecaForce "=refnum, "MicroForce"=refnum, "LHBack"=refnum, "LHNext"=refnum, "Enter the Loading Rate (N/min)"=refnum, "Message"=refnum, "Warning 2"=refnum, "SSP 0.75"=refnum, "SSP 0.5"=refnum, "SSP 0.3"=refnum, "Warning"=refnum, "gui GIF"=refnum, "Communication is established"=refnum, "AppLoad 4"=refnum, "Multipoint"=refnum, "Load Selection"=refnum}, "PID"={"Ramp MulFac"=refnum, "pulses LoadDiffRamp(2..10)"=refnum, "PulseControlRamp(diff<=3N)"=refnum, "SetLoadDeadband(%) Load(0-10N)"=refnum, "PID gains out delay (microForce)"=refnum, "Ramp"=refnum, "Gain 2"=refnum, "pulses LoadDiff(2..10)"=refnum, "pulses LoadDiff(11..50)"=refnum, "PulseControl(diff<=3N)"=refnum, "SetLoadDeadband(%)  2"=refnum, "Dummy Run"=refnum, "Vertical load (N)"=refnum, "AutoTune"=refnum, "Offset 3 "=refnum, "apply load"=refnum, "Offset  3"=refnum, "apply load 2"=refnum, "Enter ByPass Load"=refnum, "reinit 3"=refnum, "output range delay"=refnum, "PID gains out delay"=refnum, "Bypass Load"=refnum, "pulsesSent"=refnum, "pulses "=refnum, "actpid"=refnum, "gFF Rot"=refnum, "pulses LoadDiff(21..1000)"=refnum, "Delay"=refnum, "deadband"=refnum}, "Config Parameters"={"Tab Control 3"=refnum, "Tab Control 19"=refnum, "SAMPLES"=refnum, "Re-initilaize"=refnum, "Filter ON/OFF"=refnum, "TracHomeSurgeOffsetCounts 10MM"=refnum, "TracHomeSwayOffsetCounts 10MM"=refnum, "Acoustic Emission:"=refnum, "Apply Filter (FF)"=refnum, "Filter% 2"=refnum, "Apply Filter (Load)"=refnum, "Filter% "=refnum, "Sway distance (mm)"=refnum, "Surge distance (mm)"=refnum, "DataSavingLoopDelay(ms)"=refnum, "SAVE 2"=refnum, "Enter Distance"=refnum, "Sway Counts:"=refnum, "Distance (mm): 3"=refnum, "Surge Counts:"=refnum, "Distance (mm): 2"=refnum, "Distance (mm):"=refnum, "Heave Counts:"=refnum, "LRMHomeSurgeOffsetCounts"=refnum, "LRMHomeSwayOffsetCounts"=refnum, "TracHomeSurgeOffsetCounts 20MM"=refnum, "TracHomeSwayOffsetCounts 20MM"=refnum, "RotHomeSwayOffsetCounts"=refnum, "RotHomeSurgeOffsetCounts"=refnum, "Heave distance"=refnum, "Zmm"=refnum, "Heave Pulses/mm"=refnum, "Surge Pulses/mm"=refnum, "Sway Pulses/mm"=refnum, "Heave Pitch"=refnum, "Surge Pitch"=refnum, "Sway Pitch"=refnum, "Heave PPR"=refnum, "Surge PPR"=refnum, "Sway PPR"=refnum, "Tab Control 5"=refnum, "Tab Control 14"=refnum, "Tab Control 26"=refnum, "AE"=refnum, "Heave Loop Delay"=refnum, "Heave PID Speed"=refnum, "Surge Jog Speed"=refnum, "Heave Jog Speed"=refnum, "Sway Loop Delay"=refnum, "Sway PID Speed"=refnum, "Sway Jog Speed"=refnum, "DEPTH TRIP VALUE"=refnum, "LOAD TRIP VALUE"=refnum, "DEPTH TRIP   ENABLE"=refnum, "LOAD TRIP  ENABLE"=refnum, "CYCLIC FF TRIP VALUE"=refnum, "FF TRIP VALUE"=refnum, "CYCLIC CoF TRIP VALUE"=refnum, "COF TRIP VALUE"=refnum, "CYCLIC COF TRIP  ENABLE"=refnum, "CYCLIC FF TRIP  ENABLE"=refnum, "FF TRIP  ENABLE"=refnum, "COF TRIP  ENABLE"=refnum, "JOG TRIP LOAD VALUE (N)"=refnum}, "Loading Com Port"={"ClearAll"=refnum, "Mz(Nm)"=refnum, "My(Nm)"=refnum, "Mx(Nm)"=refnum, "Save Dwell"=refnum, "Mx "=refnum, "My "=refnum, "Mz"=refnum, "Fx(N)"=refnum, "Fy(N)"=refnum, "Fz(N)"=refnum, "ZeroAll"=refnum, "Acq Delay (ms)"=refnum, "Burst Delay (ms)"=refnum, "model"=refnum, "SN"=refnum, "FFx(N)"=refnum, "Sensor IP"=refnum, "Port"=refnum, "FFy(N)"=refnum, "Load(N)"=refnum, "delete Handle"=refnum, "Create Handle"=refnum, "ft_data"=refnum, "ft_range"=refnum, "ft_data 2"=refnum, "stop 6"=refnum, "running_flag"=refnum, "ft_udp_handle"=refnum, "get-data-return"=refnum, "get-range-return"=refnum, "zero-return"=refnum, "filter-return"=refnum, "initial-return"=refnum, "deleteHandle-result"=refnum, "Load Cell Temp"=refnum}, "Heave AND Surge"={"SURGE POSE"=refnum, "error out Read"=refnum, "HEAVE POSE"=refnum, "State"=refnum, "Homed"=refnum, "Sequence ID"=refnum, "error out Write"=refnum, "faultCode"=refnum, "Ack ID"=refnum, "SPEED"=refnum, "Distance"=refnum, "Mode Command"=refnum, "Heave and Surge Read"=refnum, "Read Heave Temp"=refnum, "Spare 15"=refnum, "Spare 14"=refnum, "Spare 13"=refnum, "Spare 12"=refnum, "Spare 11"=refnum, "Spare 10"=refnum, "Spare 9"=refnum, "Spare 8"=refnum, "Spare 7"=refnum, "Spare 6"=refnum, "Spare 5"=refnum, "Spare 4"=refnum, "Spare 2"=refnum, "Spare 1"=refnum, "Node Id"=refnum, "Spare 3"=refnum, "SPARE 4"=refnum, "SPARE 3"=refnum, "SPARE 2"=refnum, "SPARE 1"=refnum, "fwMajor"=refnum, "fwMinor"=refnum, "Manual Write"=refnum, "Heave and Surge Write"=refnum, "SPARE 5"=refnum, "Reserved "=refnum, "SPARE 8"=refnum, "SPARE 6"=refnum, "SPARE 7"=refnum, "SPARE 17"=refnum, "SPARE 16"=refnum, "SPARE 15"=refnum, "SPARE 14"=refnum, "SPARE 13"=refnum, "SPARE 12"=refnum, "SPARE 11"=refnum, "SPARE 10"=refnum, "SPARE 9"=refnum, "System UPTIME"=refnum, "Missed Packets"=refnum, "faultCode Surge Right"=refnum, "faultCode Surge Left"=refnum, "faultCode Heave"=refnum}, "New PID LOGIC"={"Fine Tune Zone"=refnum, "PID SDelay"=refnum, "Max_pos_limit"=refnum, "Min_pos_limit"=refnum, "i_limit"=refnum, "pct_scale"=refnum, "Deadband"=refnum, "Kd"=refnum, "Ki"=refnum, "Kp"=refnum, "Current Position"=refnum, "Set Load"=refnum, "Current Load"=refnum, "Pulse delta"=refnum, "Init Step"=refnum, "Max Step Linit"=refnum, "min_deadband_floor"=refnum, "dynamic_spindle_noise_scalar"=refnum, "min_finetune_floor"=refnum, "filter_alpha"=refnum}, "SWAY "={"fwMajor"=refnum, "Homed"=refnum, "Rotary POSE"=refnum, "State"=refnum, "SWAY POSE"=refnum, "Ack ID"=refnum, "faultCode"=refnum, "Node Id"=refnum, "fwMinor"=refnum, "Spare 6"=refnum, "Spare 5"=refnum, "Spare 4"=refnum, "Spare 3"=refnum, "Spare 2"=refnum, "Spare 1"=refnum, "Spare 7"=refnum, "SPARE  5"=refnum, "error out Write  SWAY "=refnum, "error out Read SWAY "=refnum, "Manual Write SWAY "=refnum, "SWAY WRITE"=refnum, "SPARE  4"=refnum, "SPARE  3"=refnum, "SPARE 2"=refnum, "SPARE 1"=refnum, "Spare 15"=refnum, "Spare 14"=refnum, "Spare 13"=refnum, "Spare 12"=refnum, "Spare 11"=refnum, "Spare 9"=refnum, "Spare 8"=refnum, "SPEED"=refnum, "Distance"=refnum, "Mode Command"=refnum, "Sequence ID"=refnum, "SWAY READ"=refnum, "Spare 10"=refnum, "Read SWAY Temp"=refnum, "faultCode Sway "=refnum, "Missed Packets"=refnum, "System UPTIME sway"=refnum, "SPARE 6"=refnum, "SPARE 7"=refnum, "SPARE 9"=refnum, "SPARE 11"=refnum, "SPARE 10"=refnum, "SPARE 8"=refnum, "SPARE 13"=refnum, "SPARE 12"=refnum, "SPARE 17"=refnum, "SPARE 16"=refnum, "SPARE 15"=refnum, "SPARE 14"=refnum, "Reserved"=refnum, "faultCode Rotary"=refnum}, "Analysis Screen"={"Analysis Home"=refnum, "Refresh 2"=refnum, "MEAN 4"=refnum, "SD 4"=refnum, "VARIANCE 4"=refnum, "MEAN  3"=refnum, "SD  3"=refnum, "VARIANCE  3"=refnum, "MEAN 2"=refnum, "SD  2"=refnum, "VARIANCE 2"=refnum, "MEAN"=refnum, "SD"=refnum, "VARIANCE"=refnum, "File 4 Discription"=refnum, "OPEN 4"=refnum, "File Name 4"=refnum, "OPEN 3"=refnum, "File 3 Discription"=refnum, "File Name 3"=refnum, "Y-AXIS"=refnum, "X-AXIS"=refnum, "XY Graph"=refnum, "File Name 2"=refnum, "File Name 1"=refnum, "OPEN 2"=refnum, "OPEN 1"=refnum, "File 1 Discription "=refnum, "File 2 Discription"=refnum, "Export"=refnum, "File Format"=refnum}, "Traction"={"faultCode Traction 2"=refnum, "faultCode Traction 1"=refnum, "Missed Packets"=refnum, "System UPTIME Traction"=refnum, "SPARE 17"=refnum, "SPARE 16"=refnum, "SPARE 15"=refnum, "SPARE 14"=refnum, "SPARE 13"=refnum, "SPARE 12"=refnum, "SPARE 11"=refnum, "SPARE 10"=refnum, "SPARE 9"=refnum, "SPARE 8"=refnum, "SPARE 7"=refnum, "SPARE 6"=refnum, "Reserved"=refnum, "SPARE  5"=refnum, "Manual Write TRACTION"=refnum, "TRACTION WRITE"=refnum, "SPARE  4"=refnum, "SPARE  3"=refnum, "SPARE 2"=refnum, "SPARE 1"=refnum, "Spare 7"=refnum, "Spare 6"=refnum, "Spare 5"=refnum, "Spare 4"=refnum, "Spare 2"=refnum, "Spare 1"=refnum, "Node Id"=refnum, "Read TRACTION Temp"=refnum, "fwMinor"=refnum, "fwMajor"=refnum, "faultCode"=refnum, "TRACTION POSE"=refnum, "TRACTION POSE 2"=refnum, "Homed"=refnum, "State"=refnum, "Ack ID"=refnum, "SPEED"=refnum, "Distance"=refnum, "Mode Command"=refnum, "Sequence ID"=refnum, "error out Read TRACTION"=refnum, "error out Write  TRACTION"=refnum, "TRACTION READ"=refnum, "Spare 3"=refnum}, "Traction reciepe"={"SRR Sweep Range (%) Stribeck"=refnum, "Traction Receipe"=refnum, "Total Execution Time"=refnum, "Total Steps"=refnum, "Duration / Step (s)  Stribeck"=refnum, "STRIBECK Fixed SRR List (%)"=refnum, "Duration / Step (s) Traction"=refnum, "SRR Sweep Range (%) traction"=refnum, "Rolling Speed (mm/s)"=refnum, "Temperature Stages (°C)"=refnum, "Ball Load (N)"=refnum, "Lubricant Name"=refnum, "Profile File Name"=refnum, "SET entrainment Velocity"=refnum, "Test Array Size"=refnum, "SRR INDEX [ STRIBECK]"=refnum, "Stribeck Size"=refnum, "SET SRR"=refnum, "ELAPSED TIMER "=refnum, "BALL SET RPM"=refnum, "DISC SET RPM"=refnum, "SET LOAD"=refnum, "TEMPERATURE READ"=refnum, "SET TEMPERATURE"=refnum, "Traction Size"=refnum, "DISC SPEED (rpm)"=refnum, "BALL SPEED (rpm)"=refnum, "BALL WEAR TRACK"=refnum, "DISC WEARTRACK"=refnum, "SRR INDEX [ TRACTION]"=refnum, "Start Index Type"=refnum, "Enum - Menu"=refnum, "Ball (mm/sec)"=refnum, "Disc (mm/sec)"=refnum}, "Traction Control"={"HomeTraction"=refnum, "Demo Mode Display"=refnum, "Traction Message"=refnum, "Traction Step Update Details"=refnum, "Main Tab sequence for selection"=refnum, "Ramp Tab"=refnum, "e.v/ssr"=refnum, "Enter Fixed E.Velocity"=refnum, "Enter Final SRR"=refnum, "Enter initial SRR"=refnum, "Enter Fixed SRR"=refnum, "Enter the Final E.Velocity (m/s)"=refnum, "Enter initial E.Velocity (m/s)"=refnum, "Ball WTD"=refnum, "E.Velocity"=refnum, "Enter the Final Velocity (m/s)"=refnum, "Enter initial Velocity (m/s)"=refnum, "Ramp Up   Disc"=refnum, "Initial DiscSpeed (RPM)"=refnum, "Final Speed (RPM) Ball"=refnum, "Final Speed (RPM)"=refnum, "Initial Speed (RPM) Ball"=refnum, "Enter the Final Velocity (m/s) Ball"=refnum, "Enter initial Velocity (m/s) Ball"=refnum, "Ramp Up"=refnum, "ExceedBallSpeed step"=refnum, "ExceedDiscSpeed"=refnum, "BallSpeed Exceed Indication"=refnum, "Apply"=refnum, "SPEED SELECTION : MTM"=refnum, "SPEED SELECTION : MTM 2"=refnum, "TEST SELECTION (MTM)"=refnum, "MTM Test Selection"=refnum, "File Path Tab"=refnum, "File Path String"=refnum, "Save"=refnum, "Save  2"=refnum, "Import "=refnum, "File Path :"=refnum, "Step Sequence Indication Tab"=refnum, "Step Sequence Indication"=refnum, "Calculate Step"=refnum, "StepTable"=refnum, "ExceedDiscSpeed  Cinstant Speed"=refnum, "ExceedBallSpeed Constant"=refnum, "TEST SELECTION (MTM) 2"=refnum, "SPEED SELECTION : MTM 3"=refnum, "MTM Test Selection 2"=refnum, "Enter the Speed (m/sec): "=refnum, "Enter the Speed (m/sec):  2"=refnum, "Enter the Speed (RPM):"=refnum, "Lower Spped "=refnum, "Upper"=refnum, "Enter the Speed (RPM):Ball"=refnum, "Disc Motion Direction: "=refnum, "Ball Motion Direction :"=refnum, "Motion Mode: "=refnum, "Wear Track Diameter (mm) "=refnum, "Disc Speed Indicator"=refnum, "ExceedBallSpeed"=refnum}, "Acquostic"={"Last Config Rejected "=refnum, "rx command count"=refnum, "Current Filter Id"=refnum, "Isolated Gain"=refnum, "DAQ Status"=refnum, "error out"=refnum, "error in (no error)"=refnum, "Uplink Packet"=refnum, "data out"=refnum, "Downlink Packet"=refnum, "Signal Energy"=refnum, "Amplitude db_AE"=refnum, "Peak Amplitude"=refnum, "AE Ring-Down Counts"=refnum, "Gains"=refnum, "Manual Write Acquostic"=refnum}} ("Data Cluster") -> [w81]
    tunnel: w69 -> [w111]
    tunnel: [w91] -> w68
    tunnel: w68 -> [w118]
    tunnel: [w112] -> w67
    tunnel: w67 -> [w127]
    tunnel: [w126] -> w66
    tunnel: w66 -> [w163]
    tunnel: [w162] -> w64
    tunnel: w64 -> [w234]
    tunnel: [w233] -> w63
    tunnel: w63 -> [w261]
    tunnel: [w260] -> w62
    tunnel: w62 -> [w277]
    tunnel: [w276] -> w61
    tunnel: w61 -> [w396]
    tunnel: [w395] -> w39
    tunnel: w39 -> [w426]
    tunnel: [w425] -> w38
    tunnel: w38 -> [w492]
    tunnel: [w491] -> w37
    tunnel: w37 -> [w529]
    tunnel: [w528] -> w36
    tunnel: w36 -> [w588]
    tunnel: [w587] -> w34
    tunnel: w34 -> [w610]
    tunnel: [w609] -> w33
    tunnel: w33 -> [w668]
    tunnel: [w667] -> w31
    tunnel: w31 -> [w701]
    tunnel: [w700] -> w22
    tunnel: w22 -> [w751]
    tunnel: [w750] -> w21
    tunnel: w21 -> [w787]
    tunnel: [w786] -> w18
    tunnel: w18 -> [w847]
    tunnel: [w846] -> w11
    tunnel: [w864] -> w9
    tunnel: w11 -> [w865]
    frame #0 {
      n2 = control-ref of="GUI"() -> (w90:refnum<vi>)
      n3 = control-ref of="MainPage"() -> (w84:refnum<vi>)
      n4 = control-ref of="Platform Settings"() -> (w89:refnum<vi>)
      n5 = control-ref of="Configure"() -> (w88:refnum<vi>)
      n6 = control-ref of="Home"() -> (w87:refnum<vi>)
      n7 = control-ref of="EXIT"() -> (w86:refnum<vi>)
      n8 = control-ref of="service 2"() -> (w85:refnum<vi>)
      n9 = control-ref of="Analysis"() -> (w83:refnum<vi>)
      n10 = Bundle By Name(cluster=w81, "Main Home Screen.GUI"=w90, "Main Home Screen.Platform Settings"=w89, "Main Home Screen.Configure"=w88, "Main Home Screen.Home"=w87, "Main Home Screen.EXIT"=w86, "Main Home Screen.service 2"=w85, "Main Home Screen.MainPage"=w84, "Main Home Screen.Analysis"=w83) -> (w82:T15)
    }
    frame #1 {
      n11 = control-ref of="Sway Right Main"() -> (w101:refnum<vi>)
      n12 = control-ref of="Sway Left Main"() -> (w100:refnum<vi>)
      n13 = control-ref of="Heave Down Main"() -> (w99:refnum<vi>)
      n14 = control-ref of="Heave Up main"() -> (w98:refnum<vi>)
      n15 = control-ref of="Update Sway Speed"() -> (w97:refnum<vi>)
      n16 = control-ref of="Update Heave Speed"() -> (w96:refnum<vi>)
      n17 = control-ref of="Surge Backward Main"() -> (w92:refnum<vi>)
      n18 = control-ref of="Update Surge Speed"() -> (w109:refnum<vi>)
      n19 = control-ref of="Disable Axis Jog Soft Limits m"() -> (w107:refnum<vi>)
      n20 = control-ref of="Sway and Surge COM Status"() -> (w105:refnum<vi>)
      n21 = control-ref of="Heave COM Status"() -> (w104:refnum<vi>)
      n22 = control-ref of="Enable Platform"() -> (w103:refnum<vi>)
      n23 = control-ref of="Surge Forward Main"() -> (w102:refnum<vi>)
      n24 = control-ref of="mm/s Heave"() -> (w95:refnum<vi>)
      n25 = control-ref of="mm/sec"() -> (w94:refnum<vi>)
      n26 = control-ref of="mm"() -> (w93:refnum<vi>)
      n27 = control-ref of="mm/s  Surge"() -> (w110:refnum<vi>)
      n28 = control-ref of="mm/s  Sway"() -> (w106:refnum<vi>)
      n29 = control-ref of="Drive Error"() -> (w108:refnum<vi>)
      n30 = Bundle By Name(cluster=w111, "Platform Settings.mm/s  Surge"=w110, "Platform Settings.Update Surge Speed"=w109, "Platform Settings.Drive Error"=w108, "Platform Settings.Disable Axis Jog Soft Limits"=w107, "Platform Settings.mm/s  Sway"=w106, "Platform Settings.Sway and Surge COM Status"=w105, "Platform Settings.Heave COM Status"=w104, "Platform Settings.Enable Platform"=w103, "Platform Settings.Surge Forward Main"=w102, "Platform Settings.Sway Right Main"=w101, "Platform Settings.Sway Left Main"=w100, "Platform Settings.Heave Down Main"=w99, "Platform Settings.Heave Up main"=w98, "Platform Settings.Update Sway Speed"=w97, "Platform Settings.Update Heave Speed"=w96, "Platform Settings.mm/s Heave"=w95, "Platform Settings.mm/sec"=w94, "Platform Settings.mm"=w93, "Platform Settings.Surge Backward Main"=w92) -> (w91:T15)
    }
    frame #2 {
      n31 = control-ref of="Analysis Home"() -> (w117:refnum<vi>)
      n32 = control-ref of="Surface Analysis"() -> (w116:refnum<vi>)
      n33 = control-ref of="Imaging"() -> (w115:refnum<vi>)
      n34 = control-ref of="Image Analysis"() -> (w114:refnum<vi>)
      n35 = control-ref of="Post Analysis"() -> (w113:refnum<vi>)
      n36 = Bundle By Name(cluster=w118, "Analysis Screen.Analysis Home"=w117, "Analysis Screen.Surface Analysis"=w116, "Analysis Screen.Imaging"=w115, "Analysis Screen.Image Analysis"=w114, "Analysis Screen.Post Analysis"=w113) -> (w112:T15)
    }
    frame #3 {
      n37 = control-ref of="Select Load Head"() -> (w125:refnum<vi>)
      n38 = control-ref of="Auto"() -> (w119:refnum<vi>)
      n39 = control-ref of="Notes :"() -> (w124:refnum<vi>)
      n40 = control-ref of="FILE"() -> (w123:refnum<vi>)
      n41 = control-ref of="Sample ID :"() -> (w122:refnum<vi>)
      n42 = control-ref of="Operator ID :"() -> (w121:refnum<vi>)
      n43 = control-ref of="Operator Name :"() -> (w120:refnum<vi>)
      n44 = Bundle By Name(cluster=w127, "Config Screen.Select Load Head"=w125, "Config Screen.Notes :"=w124, "Config Screen.FILE"=w123, "Config Screen.Sample ID :"=w122, "Config Screen.Operator ID :"=w121, "Config Screen.Operator Name :"=w120, "Config Screen.Auto"=w119) -> (w126:T15)
    }
    frame #4 {
      n45 = control-ref of="Warning"() -> (w155:refnum<vi>)
      n46 = control-ref of="gui GIF"() -> (w154:refnum<vi>)
      n47 = control-ref of="Load Selection"() -> (w128:refnum<vi>)
      n48 = control-ref of="Warning 2"() -> (w159:refnum<vi>)
      n49 = control-ref of="SSP 0.75"() -> (w158:refnum<vi>)
      n50 = control-ref of="SSP 0.5"() -> (w157:refnum<vi>)
      n51 = control-ref of="SSP 0.3"() -> (w156:refnum<vi>)
      n52 = control-ref of="Communication is established"() -> (w153:refnum<vi>)
      n53 = control-ref of="AppLoad 4"() -> (w152:refnum<vi>)
      n54 = control-ref of="Multipoint"() -> (w151:refnum<vi>)
      n55 = control-ref of="com 3"() -> (w147:refnum<vi>)
      n56 = control-ref of="com"() -> (w146:refnum<vi>)
      n57 = control-ref of="DecaForce COM Status"() -> (w145:refnum<vi>)
      n58 = control-ref of="Update"() -> (w144:refnum<vi>)
      n59 = control-ref of="Clear 3"() -> (w143:refnum<vi>)
      n60 = control-ref of="seq"() -> (w142:refnum<vi>)
      n61 = control-ref of="Stribeck table"() -> (w141:refnum<vi>)
      n62 = control-ref of="KiloForce"() -> (w133:refnum<vi>)
      n63 = control-ref of="DecaForce"() -> (w132:refnum<vi>)
      n64 = control-ref of="MicroForce"() -> (w131:refnum<vi>)
      n65 = control-ref of="LHBack"() -> (w130:refnum<vi>)
      n66 = control-ref of="LHNext"() -> (w129:refnum<vi>)
      n67 = control-ref of="Enter the Loading Rate (N/min)"() -> (w161:refnum<vi>)
      n68 = control-ref of="Enter the Final Load (N)"() -> (w138:refnum<vi>)
      n69 = control-ref of="Enter the CoF Trip"() -> (w137:refnum<vi>)
      n70 = control-ref of="Enter the Friction Force Trip"() -> (w136:refnum<vi>)
      n71 = control-ref of="Enter the Normal load Trip"() -> (w135:refnum<vi>)
      n72 = control-ref of="Enter the Load  (N)"() -> (w134:refnum<vi>)
      n73 = control-ref of="Message"() -> (w160:refnum<vi>)
      n74 = control-ref of="Indentation"() -> (w150:refnum<vi>)
      n75 = control-ref of="Stribeck Table  For loading"() -> (w140:refnum<vi>)
      n76 = control-ref of="Reference Sample"() -> (w149:refnum<vi>)
      n77 = control-ref of="Load Cell Communication Slide"() -> (w148:refnum<vi>)
      n78 = control-ref of="Loading Mode"() -> (w139:refnum<vi>)
      n79 = Bundle By Name(cluster=w163, "Loading.Enter the Loading Rate (N/min)"=w161, "Loading.Message"=w160, "Loading.Warning 2"=w159, "Loading.SSP 0.75"=w158, "Loading.SSP 0.5"=w157, "Loading.SSP 0.3"=w156, "Loading.Warning"=w155, "Loading.gui GIF"=w154, "Loading.Communication is established"=w153, "Loading.AppLoad 4"=w152, "Loading.Multipoint"=w151, "Loading.Indentation"=w150, "Loading.Reference Sample"=w149, "Loading.Load Cell Communication Slide"=w148, "Loading.com 3"=w147, "Loading.com"=w146, "Loading.DecaForce COM Status"=w145, "Loading.Update"=w144, "Loading.Clear 3"=w143, "Loading.seq"=w142, "Loading.Stribeck table"=w141, "Loading.Stribeck Table  For loading"=w140, "Loading.Loading Mode"=w139, "Loading.Enter the Final Load (N)"=w138, "Loading.Enter the CoF Trip"=w137, "Loading.Enter the Friction Force Trip"=w136, "Loading.Enter the Normal load Trip"=w135, "Loading.Enter the Load  (N)"=w134, "Loading.KiloForce"=w133, "Loading.DecaForce"=w132, "Loading.MicroForce"=w131, "Loading.LHBack"=w130, "Loading.LHNext"=w129, "Loading.Load Selection"=w128) -> (w162:T15)
    }
    frame #5 {
      n80 = control-ref of="TEST SELECTION"() -> (w215:refnum<vi>)
      n81 = control-ref of="SPEED SELECTION :"() -> (w214:refnum<vi>)
      n82 = control-ref of="SPEED SELECTION : rotary"() -> (w181:refnum<vi>)
      n83 = control-ref of="Rotary Tab"() -> (w230:refnum<vi>)
      n84 = control-ref of="e.v/ssr 2"() -> (w227:refnum<vi>)
      n85 = control-ref of="Step Speed"() -> (w211:refnum<vi>)
      n86 = control-ref of="M3 Image"() -> (w206:refnum<vi>)
      n87 = control-ref of="Rotary Module Selection"() -> (w183:refnum<vi>)
      n88 = control-ref of="zNL"() -> (w232:refnum<vi>)
      n89 = control-ref of="E.Velocity 2"() -> (w228:refnum<vi>)
      n90 = control-ref of="Ramp Up 2"() -> (w216:refnum<vi>)
      n91 = control-ref of="Angular Oscillation Set"() -> (w213:refnum<vi>)
      n92 = control-ref of="Traction"() -> (w212:refnum<vi>)
      n93 = control-ref of="Surge Forward MM"() -> (w208:refnum<vi>)
      n94 = control-ref of="Surge Backward MM"() -> (w207:refnum<vi>)
      n95 = control-ref of="Sway Left MM"() -> (w204:refnum<vi>)
      n96 = control-ref of="Sway Right MM"() -> (w203:refnum<vi>)
      n97 = control-ref of="Disable Axis Jog Soft Limits"() -> (w202:refnum<vi>)
      n98 = control-ref of="Heave Down MM"() -> (w200:refnum<vi>)
      n99 = control-ref of="Heave Up MM"() -> (w199:refnum<vi>)
      n100 = control-ref of="Set WTD"() -> (w197:refnum<vi>)
      n101 = control-ref of="HomeScratch"() -> (w196:refnum<vi>)
      n102 = control-ref of="HomeRot"() -> (w195:refnum<vi>)
      n103 = control-ref of="PlaceModule"() -> (w194:refnum<vi>)
      n104 = control-ref of="LR Sway"() -> (w190:refnum<vi>)
      n105 = control-ref of="Rot Hor"() -> (w189:refnum<vi>)
      n106 = control-ref of="Scratch"() -> (w188:refnum<vi>)
      n107 = control-ref of="LR Cam"() -> (w187:refnum<vi>)
      n108 = control-ref of="MMBack"() -> (w186:refnum<vi>)
      n109 = control-ref of="MMNext"() -> (w185:refnum<vi>)
      n110 = control-ref of="Rot Ver"() -> (w184:refnum<vi>)
      n111 = control-ref of="calculate rotary"() -> (w182:refnum<vi>)
      n112 = control-ref of="Import 2"() -> (w180:refnum<vi>)
      n113 = control-ref of="Save 2"() -> (w179:refnum<vi>)
      n114 = control-ref of="SwaySpeed Set"() -> (w172:refnum<vi>)
      n115 = control-ref of="HomeScratch"() -> (w168:refnum<vi>)
      n116 = control-ref of="NL disp"() -> (w231:refnum<vi>)
      n117 = control-ref of="Enter Fixed E.Velocity 2"() -> (w226:refnum<vi>)
      n118 = control-ref of="Enter Final SRR 2"() -> (w225:refnum<vi>)
      n119 = control-ref of="Enter initial SRR 2"() -> (w224:refnum<vi>)
      n120 = control-ref of="Enter Fixed SRR 2"() -> (w223:refnum<vi>)
      n121 = control-ref of="Enter the Final E.Velocity (m/s) 2"() -> (w222:refnum<vi>)
      n122 = control-ref of="Enter initial E.Velocity (m/s) 2"() -> (w221:refnum<vi>)
      n123 = control-ref of="Final Speed (RPM) 3"() -> (w220:refnum<vi>)
      n124 = control-ref of="Initial Speed (RPM) 2"() -> (w219:refnum<vi>)
      n125 = control-ref of="Enter the Final Velocity (m/s) 3"() -> (w218:refnum<vi>)
      n126 = control-ref of="Enter initial Velocity (m/s)  3"() -> (w217:refnum<vi>)
      n127 = control-ref of="mm"() -> (w201:refnum<vi>)
      n128 = control-ref of="Wear Track Diameter (mm)"() -> (w198:refnum<vi>)
      n129 = control-ref of="Enter the Angle (Deg)"() -> (w193:refnum<vi>)
      n130 = control-ref of="Enter the Frequency (Hz)"() -> (w192:refnum<vi>)
      n131 = control-ref of="Enter the Speed(mm/sec)"() -> (w175:refnum<vi>)
      n132 = control-ref of="Enter the Speed (RPM)"() -> (w174:refnum<vi>)
      n133 = control-ref of="Enter Scratch Speed (mm/s):"() -> (w173:refnum<vi>)
      n134 = control-ref of="Scartch Offset"() -> (w171:refnum<vi>)
      n135 = control-ref of="Enter Scratch length (mm):"() -> (w167:refnum<vi>)
      n136 = control-ref of="Wear Track Diameter"() -> (w166:refnum<vi>)
      n137 = control-ref of="No of Scratch"() -> (w164:refnum<vi>)
      n138 = control-ref of="String 39"() -> (w205:refnum<vi>)
      n139 = control-ref of="String 45"() -> (w177:refnum<vi>)
      n140 = control-ref of="Rotary Speed Exced"() -> (w165:refnum<vi>)
      n141 = control-ref of="StepTable For Load-Speed"() -> (w210:refnum<vi>)
      n142 = control-ref of="StepTable For Speed"() -> (w209:refnum<vi>)
      n143 = control-ref of="StepTable For Speed 3"() -> (w176:refnum<vi>)
      n144 = control-ref of="Motion Direction:  3"() -> (w229:refnum<vi>)
      n145 = control-ref of="Motion Mode:"() -> (w191:refnum<vi>)
      n146 = control-ref of="Scratch Mode"() -> (w170:refnum<vi>)
      n147 = control-ref of="Motion type:"() -> (w169:refnum<vi>)
      n148 = control-ref of="File Path :  2"() -> (w178:refnum<vi>)
      n149 = Bundle By Name(cluster=w234, "Motion Module.zNL"=w232, "Motion Module.NL disp"=w231, "Motion Module.Rotary Tab"=w230, "Motion Module.Motion Direction:  3"=w229, "Motion Module.E.Velocity 2"=w228, "Motion Module.e.v/ssr 2"=w227, "Motion Module.Enter Fixed E.Velocity 2"=w226, "Motion Module.Enter Final SRR 2"=w225, "Motion Module.Enter initial SRR 2"=w224, "Motion Module.Enter Fixed SRR 2"=w223, "Motion Module.Enter the Final E.Velocity (m/s) 2"=w222, "Motion Module.Enter initial E.Velocity (m/s) 2"=w221, "Motion Module.Final Speed (RPM) 3"=w220, "Motion Module.Initial Speed (RPM) 2"=w219, "Motion Module.Enter the Final Velocity (m/s) 3"=w218, "Motion Module.Enter initial Velocity (m/s)  3"=w217, "Motion Module.Ramp Up 2"=w216, "Motion Module.TEST SELECTION"=w215, "Motion Module.SPEED SELECTION :"=w214, "Motion Module.Angular Oscillation Set"=w213, "Motion Module.Traction"=w212, "Motion Module.Step Speed"=w211, "Motion Module.StepTable For Load-Speed"=w210, "Motion Module.StepTable For Speed"=w209, "Motion Module.Surge Forward MM"=w208, "Motion Module.Surge Backward MM"=w207, "Motion Module.M3 Image"=w206, "Motion Module.String 39"=w205, "Motion Module.Sway Left MM"=w204, "Motion Module.Sway Right MM"=w203, "Motion Module.Disable Axis Jog Soft Limits"=w202, "Motion Module.mm"=w201, "Motion Module.Heave Down MM"=w200, "Motion Module.Heave Up MM"=w199, "Motion Module.Wear Track Diameter (mm)"=w198, "Motion Module.Set WTD"=w197, "Motion Module.HomeScratch"=w196, "Motion Module.HomeRot"=w195, "Motion Module.PlaceModule"=w194, "Motion Module.Enter the Angle (Deg)"=w193, "Motion Module.Enter the Frequency (Hz)"=w192, "Motion Module.Motion Mode:"=w191, "Motion Module.LR Sway"=w190, "Motion Module.Rot Hor"=w189, "Motion Module.Scratch"=w188, "Motion Module.LR Cam"=w187, "Motion Module.MMBack"=w186, "Motion Module.MMNext"=w185, "Motion Module.Rot Ver"=w184, "Motion Module.Rotary Module Selection"=w183, "Motion Module.calculate rotary"=w182, "Motion Module.SPEED SELECTION : rotary"=w181, "Motion Module.Import 2"=w180, "Motion Module.Save 2"=w179, "Motion Module.File Path :  2"=w178, "Motion Module.String 45"=w177, "Motion Module.StepTable For Speed 3"=w176, "Motion Module.Enter the Speed(mm/sec)"=w175, "Motion Module.Enter the Speed(RPM)"=w174, "Motion Module.Enter Scratch Speed (mm/s):"=w173, "Motion Module.SwaySpeed Set"=w172, "Motion Module.Scartch Offset"=w171, "Motion Module.Scratch Mode"=w170, "Motion Module.Motion type:"=w169, "Motion Module.HomeScratch 2"=w168, "Motion Module.Enter Scratch length (mm):"=w167, "Motion Module.Wear Track Diameter"=w166, "Motion Module.Rotary Speed Exced"=w165, "Motion Module.No of Scratch"=w164) -> (w233:T15)
    }
    frame #6 {
      n150 = control-ref of="Add to list"() -> (w252:refnum<vi>)
      n151 = control-ref of="Wear"() -> (w251:refnum<vi>)
      n152 = control-ref of="Vibration"() -> (w250:refnum<vi>)
      n153 = control-ref of="Humidity (Chamber)"() -> (w249:refnum<vi>)
      n154 = control-ref of="Temperature (Chamber)"() -> (w248:refnum<vi>)
      n155 = control-ref of="ECR"() -> (w247:refnum<vi>)
      n156 = control-ref of="Temperature (Amb)"() -> (w246:refnum<vi>)
      n157 = control-ref of="Microphone"() -> (w245:refnum<vi>)
      n158 = control-ref of="Acoustic Emission 3"() -> (w244:refnum<vi>)
      n159 = control-ref of="SNext"() -> (w243:refnum<vi>)
      n160 = control-ref of="APBack"() -> (w242:refnum<vi>)
      n161 = control-ref of="Low Temp"() -> (w238:refnum<vi>)
      n162 = control-ref of="High Temp"() -> (w237:refnum<vi>)
      n163 = control-ref of="Humidity"() -> (w236:refnum<vi>)
      n164 = control-ref of="Humidity  Status  3"() -> (w259:refnum<vi>)
      n165 = control-ref of="Low Temp  Status  2"() -> (w258:refnum<vi>)
      n166 = control-ref of="TK4 status 2"() -> (w257:refnum<vi>)
      n167 = control-ref of="Humidity (Amb)"() -> (w254:refnum<vi>)
      n168 = control-ref of="Clear List"() -> (w253:refnum<vi>)
      n169 = control-ref of="Enter the Temperature (°C):"() -> (w241:refnum<vi>)
      n170 = control-ref of="Enter the Stage \nTemperature (°C):"() -> (w240:refnum<vi>)
      n171 = control-ref of="Enter the Humidity (%Rh):"() -> (w239:refnum<vi>)
      n172 = control-ref of="Sensors Picked"() -> (w235:refnum<vi>)
      n173 = control-ref of="Stage Temperature"() -> (w256:refnum<vi>)
      n174 = control-ref of="Sample Temperature"() -> (w255:refnum<vi>)
      n175 = Bundle By Name(cluster=w261, "Environmental control.Humidity  Status  3"=w259, "Environmental control.Low Temp  Status  2"=w258, "Environmental control.TK4 status 2"=w257, "Environmental control.Stage Temperature"=w256, "Environmental control.Sample Temperature"=w255, "Environmental control.Humidity (Amb)"=w254, "Environmental control.Clear List"=w253, "Environmental control.Add to list"=w252, "Environmental control.Wear"=w251, "Environmental control.Vibration"=w250, "Environmental control.Humidity (Chamber)"=w249, "Environmental control.Temperature (Chamber)"=w248, "Environmental control.ECR"=w247, "Environmental control.Temperature (Amb)"=w246, "Environmental control.Microphone"=w245, "Environmental control.Acoustic Emission 3"=w244, "Environmental control.SNext"=w243, "Environmental control.APBack"=w242, "Environmental control.Enter the Temperature (°C):"=w241, "Environmental control.Enter the Stage \nTemperature (°C):"=w240, "Environmental control.Enter the Humidity (%Rh):"=w239, "Environmental control.Low Temp"=w238, "Environmental control.High Temp"=w237, "Environmental control.Humidity"=w236, "Environmental control.Sensors Picked"=w235) -> (w260:T15)
    }
    frame #7 {
      n176 = control-ref of="ECR Port:"() -> (w271:refnum<vi>)
      n177 = control-ref of="Ramp Port:"() -> (w270:refnum<vi>)
      n178 = control-ref of="Heave and Surge COM Port:"() -> (w267:refnum<vi>)
      n179 = control-ref of="Sway COM Port:"() -> (w266:refnum<vi>)
      n180 = control-ref of="Temp Modbus:"() -> (w265:refnum<vi>)
      n181 = control-ref of="Humidity Port:"() -> (w264:refnum<vi>)
      n182 = control-ref of="About Tab"() -> (w272:refnum<vi>)
      n183 = control-ref of="Home Service"() -> (w274:refnum<vi>)
      n184 = control-ref of="Advanced Setting"() -> (w273:refnum<vi>)
      n185 = control-ref of="Installation/Replacement completed"() -> (w269:refnum<vi>)
      n186 = control-ref of="Loahead"() -> (w268:refnum<vi>)
      n187 = control-ref of="Edit Gain Constants"() -> (w263:refnum<vi>)
      n188 = control-ref of="Save Gain Constants"() -> (w262:refnum<vi>)
      n189 = control-ref of="Password"() -> (w275:refnum<vi>)
      n190 = Bundle By Name(cluster=w277, "About Screen.Password"=w275, "About Screen.Home Service"=w274, "About Screen.Advanced Setting"=w273, "About Screen.About Tab"=w272, "About Screen.ECR Port:"=w271, "About Screen.Ramp Port:"=w270, "About Screen.Installation/Replacement completed"=w269, "About Screen.Loahead"=w268, "About Screen.Heave and Surge COM Port:"=w267, "About Screen.Sway COM Port:"=w266, "About Screen.Temp Modbus:"=w265, "About Screen.Humidity Port:"=w264, "About Screen.Edit Gain Constants"=w263, "About Screen.Save Gain Constants"=w262) -> (w276:T15)
    }
    frame #8 {
      n191 = control-ref of="Cyclic Friction Force (N) Graph"() -> (w288:refnum<vi>)
      n192 = control-ref of="Cyclic Coefficient of Friction"() -> (w287:refnum<vi>)
      n193 = control-ref of="SDGp"() -> (w336:refnum<vi>)
      n194 = control-ref of="HumrGp"() -> (w334:refnum<vi>)
      n195 = control-ref of="gACQUOS"() -> (w331:refnum<vi>)
      n196 = control-ref of="ECR 2"() -> (w329:refnum<vi>)
      n197 = control-ref of="Temperature (deg c)"() -> (w327:refnum<vi>)
      n198 = control-ref of="MTM DISC  SPEED"() -> (w324:refnum<vi>)
      n199 = control-ref of="MTM BALL SPEED"() -> (w323:refnum<vi>)
      n200 = control-ref of="speed mm/sec"() -> (w322:refnum<vi>)
      n201 = control-ref of="WearGp"() -> (w312:refnum<vi>)
      n202 = control-ref of="Main Chart 3"() -> (w306:refnum<vi>)
      n203 = control-ref of="Friction Force (N) Graph"() -> (w294:refnum<vi>)
      n204 = control-ref of="Coefficient of Friction"() -> (w293:refnum<vi>)
      n205 = control-ref of="Main Screen Tab"() -> (w394:refnum<vi>)
      n206 = control-ref of="Angle and Frequency"() -> (w393:refnum<vi>)
      n207 = control-ref of="Main Speed Tab"() -> (w390:refnum<vi>)
      n208 = control-ref of="MTM MOTOR DISPLAY"() -> (w389:refnum<vi>)
      n209 = control-ref of="SPEED TAB"() -> (w384:refnum<vi>)
      n210 = control-ref of="Time Tab"() -> (w379:refnum<vi>)
      n211 = control-ref of="Temp Tabs"() -> (w372:refnum<vi>)
      n212 = control-ref of="Sub Graph"() -> (w339:refnum<vi>)
      n213 = control-ref of="Speed Tab"() -> (w325:refnum<vi>)
      n214 = control-ref of="FF Tab"() -> (w291:refnum<vi>)
      n215 = control-ref of="CZ FF"() -> (w289:refnum<vi>)
      n216 = control-ref of="Cyclic FF Disable Trip"() -> (w285:refnum<vi>)
      n217 = control-ref of="cyclic COF Disable Trip"() -> (w284:refnum<vi>)
      n218 = control-ref of="cyclic COF Reset Graph"() -> (w282:refnum<vi>)
      n219 = control-ref of="Cyclic FF Reset Graph"() -> (w281:refnum<vi>)
      n220 = control-ref of="Test Trip"() -> (w280:refnum<vi>)
      n221 = control-ref of="Scratch Start Test"() -> (w292:refnum<vi>)
      n222 = control-ref of="Scratch Start Recording"() -> (w278:refnum<vi>)
      n223 = control-ref of="Heater"() -> (w371:refnum<vi>)
      n224 = control-ref of="TK4 status"() -> (w370:refnum<vi>)
      n225 = control-ref of="Controller  Status"() -> (w367:refnum<vi>)
      n226 = control-ref of="Cooling"() -> (w364:refnum<vi>)
      n227 = control-ref of="Load Communication"() -> (w363:refnum<vi>)
      n228 = control-ref of="HumCOMStatus"() -> (w361:refnum<vi>)
      n229 = control-ref of="Load En"() -> (w358:refnum<vi>)
      n230 = control-ref of="NLt"() -> (w357:refnum<vi>)
      n231 = control-ref of="zNL 2"() -> (w356:refnum<vi>)
      n232 = control-ref of="Humidity On"() -> (w355:refnum<vi>)
      n233 = control-ref of="AppLoadSeq scratch"() -> (w351:refnum<vi>)
      n234 = control-ref of="Stop Scratch"() -> (w350:refnum<vi>)
      n235 = control-ref of="ClrLog"() -> (w349:refnum<vi>)
      n236 = control-ref of="STOP"() -> (w347:refnum<vi>)
      n237 = control-ref of="Start Test"() -> (w346:refnum<vi>)
      n238 = control-ref of="Test status"() -> (w345:refnum<vi>)
      n239 = control-ref of="AR Led"() -> (w344:refnum<vi>)
      n240 = control-ref of="Data"() -> (w343:refnum<vi>)
      n241 = control-ref of="Health"() -> (w342:refnum<vi>)
      n242 = control-ref of="Sway COM Status"() -> (w341:refnum<vi>)
      n243 = control-ref of="Heave COM Status"() -> (w340:refnum<vi>)
      n244 = control-ref of="Siliding distance Reset Graph"() -> (w337:refnum<vi>)
      n245 = control-ref of="Humidity Reset Graph"() -> (w335:refnum<vi>)
      n246 = control-ref of="Aqucostic Reset Graph"() -> (w332:refnum<vi>)
      n247 = control-ref of="ECR RESET"() -> (w330:refnum<vi>)
      n248 = control-ref of="Temperature Reset"() -> (w328:refnum<vi>)
      n249 = control-ref of="Speed Reset Graph"() -> (w326:refnum<vi>)
      n250 = control-ref of="Hymidity"() -> (w321:refnum<vi>)
      n251 = control-ref of="Humidity Disable trip"() -> (w320:refnum<vi>)
      n252 = control-ref of="Weart Deapth"() -> (w317:refnum<vi>)
      n253 = control-ref of="Depth Reset Graph"() -> (w316:refnum<vi>)
      n254 = control-ref of="Weart"() -> (w315:refnum<vi>)
      n255 = control-ref of="Depthz"() -> (w314:refnum<vi>)
      n256 = control-ref of="Load pid"() -> (w310:refnum<vi>)
      n257 = control-ref of="Load Disable Trip"() -> (w309:refnum<vi>)
      n258 = control-ref of="Load Reset Graph"() -> (w308:refnum<vi>)
      n259 = control-ref of="BACK"() -> (w305:refnum<vi>)
      n260 = control-ref of="zFF"() -> (w295:refnum<vi>)
      n261 = control-ref of="FF Reset Graph"() -> (w301:refnum<vi>)
      n262 = control-ref of="FF Disable Trip"() -> (w300:refnum<vi>)
      n263 = control-ref of="COF Disable Trip"() -> (w298:refnum<vi>)
      n264 = control-ref of="COF Reset Graph"() -> (w297:refnum<vi>)
      n265 = control-ref of="Start Test Temp"() -> (w296:refnum<vi>)
      n266 = control-ref of="Depth Trip 2"() -> (w304:refnum<vi>)
      n267 = control-ref of="Multi Scratch Pass"() -> (w279:refnum<vi>)
      n268 = control-ref of="Cyclic Friction Force (N)"() -> (w290:refnum<vi>)
      n269 = control-ref of="Cyclic FF TRIP"() -> (w286:refnum<vi>)
      n270 = control-ref of="cyclic COF TRIP"() -> (w283:refnum<vi>)
      n271 = control-ref of="Stroke (mm)"() -> (w392:refnum<vi>)
      n272 = control-ref of="Angle (Deg)"() -> (w391:refnum<vi>)
      n273 = control-ref of="Disc Speed (m/sec)"() -> (w388:refnum<vi>)
      n274 = control-ref of="Ball Speed (m/sec)"() -> (w387:refnum<vi>)
      n275 = control-ref of="Disc Speed (RPM)"() -> (w386:refnum<vi>)
      n276 = control-ref of="Ball Speed (RPM)"() -> (w385:refnum<vi>)
      n277 = control-ref of="Speed (m/sec)"() -> (w383:refnum<vi>)
      n278 = control-ref of="Set Speed (m/sec)"() -> (w382:refnum<vi>)
      n279 = control-ref of="Speed (RPM)"() -> (w381:refnum<vi>)
      n280 = control-ref of="Set Speed"() -> (w380:refnum<vi>)
      n281 = control-ref of="Time ( HH:MM:SS ) 2"() -> (w378:refnum<vi>)
      n282 = control-ref of="Test Duration"() -> (w377:refnum<vi>)
      n283 = control-ref of="Test Duration 4"() -> (w376:refnum<vi>)
      n284 = control-ref of="TEST CYCLE"() -> (w375:refnum<vi>)
      n285 = control-ref of="TOTAL CYCLES"() -> (w374:refnum<vi>)
      n286 = control-ref of="Set Load (N)"() -> (w373:refnum<vi>)
      n287 = control-ref of="ChamberTemp"() -> (w369:refnum<vi>)
      n288 = control-ref of="SetTmp"() -> (w368:refnum<vi>)
      n289 = control-ref of="ChamberTemp"() -> (w366:refnum<vi>)
      n290 = control-ref of="SetTmp"() -> (w365:refnum<vi>)
      n291 = control-ref of="Ambient \nTemperature"() -> (w362:refnum<vi>)
      n292 = control-ref of="Ambient\n Humidity"() -> (w360:refnum<vi>)
      n293 = control-ref of="Freq (Hz)"() -> (w359:refnum<vi>)
      n294 = control-ref of="humidity disp"() -> (w354:refnum<vi>)
      n295 = control-ref of="Set Humidity"() -> (w353:refnum<vi>)
      n296 = control-ref of="NL disp 2"() -> (w352:refnum<vi>)
      n297 = control-ref of="SD (mm)"() -> (w338:refnum<vi>)
      n298 = control-ref of="Acoustic Emission (mV)"() -> (w333:refnum<vi>)
      n299 = control-ref of="CoF Trip  2"() -> (w319:refnum<vi>)
      n300 = control-ref of="Depth Trip"() -> (w318:refnum<vi>)
      n301 = control-ref of="Depth (µm)"() -> (w313:refnum<vi>)
      n302 = control-ref of="NL Trip 2"() -> (w311:refnum<vi>)
      n303 = control-ref of="NL Display 4"() -> (w307:refnum<vi>)
      n304 = control-ref of="COF TRIP"() -> (w303:refnum<vi>)
      n305 = control-ref of="Friction Force (N)"() -> (w302:refnum<vi>)
      n306 = control-ref of="FF TRIP"() -> (w299:refnum<vi>)
      n307 = control-ref of="Trip Log"() -> (w348:refnum<vi>)
      n308 = Bundle By Name(cluster=w396, "Main Screen.Test Trip"=w280, "Main Screen.Main Screen Tab"=w394, "Main Screen.Angle and Frequency"=w393, "Main Screen.Stroke (mm)"=w392, "Main Screen.Angle (Deg)"=w391, "Main Screen.Main Speed Tab"=w390, "Main Screen.MTM MOTOR DISPLAY"=w389, "Main Screen.Disc Speed (m/sec)"=w388, "Main Screen.Ball Speed (m/sec)"=w387, "Main Screen.Disc Speed (RPM)"=w386, "Main Screen.Ball Speed (RPM)"=w385, "Main Screen.SPEED TAB"=w384, "Main Screen.Speed (m/sec)"=w383, "Main Screen.Set Speed (m/sec)"=w382, "Main Screen.Speed (RPM)"=w381, "Main Screen.Set Speed"=w380, "Main Screen.Time Tab"=w379, "Main Screen.Time ( HH:MM:SS ) 2"=w378, "Main Screen.Test Duration"=w377, "Main Screen.Test Duration 4"=w376, "Main Screen.TEST CYCLE"=w375, "Main Screen.TOTAL CYCLES"=w374, "Main Screen.Set Load (N)"=w373, "Main Screen.Temp Tabs"=w372, "Main Screen.Heater"=w371, "Main Screen.TK4 status"=w370, "Main Screen.ChamberTemp"=w369, "Main Screen.SetTmp"=w368, "Main Screen.Controller  Status"=w367, "Main Screen.ChamberTemp 2"=w366, "Main Screen.SetTmp 2"=w365, "Main Screen.Cooling"=w364, "Main Screen.Load Communication"=w363, "Main Screen.Ambient \nTemperature"=w362, "Main Screen.HumCOMStatus"=w361, "Main Screen.Ambient\n Humidity"=w360, "Main Screen.Freq (Hz)"=w359, "Main Screen.Load En"=w358, "Main Screen.NLt"=w357, "Main Screen.zNL 2"=w356, "Main Screen.Humidity On"=w355, "Main Screen.humidity disp"=w354, "Main Screen.Set Humidity"=w353, "Main Screen.NL disp 2"=w352, "Main Screen.AppLoadSeq scratch"=w351, "Main Screen.Stop Scratch"=w350, "Main Screen.ClrLog"=w349, "Main Screen.Trip Log"=w348, "Main Screen.STOP"=w347, "Main Screen.Start Test"=w346, "Main Screen.Test status"=w345, "Main Screen.AR Led"=w344, "Main Screen.Data"=w343, "Main Screen.Health"=w342, "Main Screen.Sway COM Status"=w341, "Main Screen.Heave COM Status"=w340, "Main Screen.Sub Graph"=w339, "Main Screen.SD (mm)"=w338, "Main Screen.Siliding distance Reset Graph"=w337, "Main Screen.SDGp"=w336, "Main Screen.Humidity Reset Graph"=w335, "Main Screen.HumrGp"=w334, "Main Screen.Acoustic Emission (mV)"=w333, "Main Screen.Aqucostic Reset Graph"=w332, "Main Screen.gACQUOS"=w331, "Main Screen.ECR RESET"=w330, "Main Screen.ECR"=w329, "Main Screen.Temperature Reset"=w328, "Main Screen.Temperature (deg c)"=w327, "Main Screen.Speed Reset Graph"=w326, "Main Screen.Speed Tab"=w325, "Main Screen.MTM DISC  SPEED"=w324, "Main Screen.MTM BALL SPEED"=w323, "Main Screen.speed mm/sec"=w322, "Main Screen.Hymidity"=w321, "Main Screen.Humidity Disable trip"=w320, "Main Screen.CoF Trip  2"=w319, "Main Screen.Depth Trip"=w318, "Main Screen.Weart Deapth"=w317, "Main Screen.Depth Reset Graph"=w316, "Main Screen.Weart"=w315, "Main Screen.Depthz"=w314, "Main Screen.Depth (µm)"=w313, "Main Screen.WearGp"=w312, "Main Screen.NL Trip 2"=w311, "Main Screen.Load pid"=w310, "Main Screen.Load Disable Trip"=w309, "Main Screen.Load Reset Graph"=w308, "Main Screen.NL Display 4"=w307, "Main Screen.Main Chart 3"=w306, "Main Screen.BACK"=w305, "Main Screen.Depth Trip 2"=w304, "Main Screen.COF TRIP"=w303, "Main Screen.Friction Force (N)"=w302, "Main Screen.FF Reset Graph"=w301, "Main Screen.FF Disable Trip"=w300, "Main Screen.FF TRIP"=w299, "Main Screen.COF Disable Trip"=w298, "Main Screen.COF Reset Graph"=w297, "Main Screen.FF Tab"=w291, "Main Screen.Start Test Temp"=w296, "Main Screen.zFF"=w295, "Main Screen.Friction Force (N) Graph"=w294, "Main Screen.Coefficient of Friction"=w293, "Main Screen.Scratch Start Test"=w292, "Main Screen.Cyclic Friction Force (N)"=w290, "Main Screen.CZ FF"=w289, "Main Screen.Cyclic Friction Force (N) Graph"=w288, "Main Screen.Cyclic Coefficient of Friction"=w287, "Main Screen.Cyclic FF TRIP"=w286, "Main Screen.Cyclic FF Disable Trip"=w285, "Main Screen.cyclic COF Disable Trip"=w284, "Main Screen.cyclic COF TRIP"=w283, "Main Screen.cyclic COF Reset Graph"=w282, "Main Screen.Cyclic FF Reset Graph"=w281, "Main Screen.Multi Scratch Pass"=w279, "Main Screen.Scratch Start Recording"=w278) -> (w395:T15)
    }
    frame #9 {
      n309 = control-ref of="gFF Rot 7"() -> (w400:refnum<vi>)
      n310 = control-ref of="Ramp"() -> (w419:refnum<vi>)
      n311 = control-ref of="Dummy Run"() -> (w413:refnum<vi>)
      n312 = control-ref of="AutoTune"() -> (w411:refnum<vi>)
      n313 = control-ref of="apply load"() -> (w409:refnum<vi>)
      n314 = control-ref of="reinit 3"() -> (w407:refnum<vi>)
      n315 = control-ref of="Bypass Load"() -> (w404:refnum<vi>)
      n316 = control-ref of="PID gains out delay (microForce)"() -> (w420:refnum<vi>)
      n317 = control-ref of="output range delay"() -> (w406:refnum<vi>)
      n318 = control-ref of="PID gains out delay"() -> (w405:refnum<vi>)
      n319 = control-ref of="Ramp MulFac"() -> (w424:refnum<vi>)
      n320 = control-ref of="pulses LoadDiffRamp(2..10)"() -> (w423:refnum<vi>)
      n321 = control-ref of="PulseControlRamp(diff<=3N)"() -> (w422:refnum<vi>)
      n322 = control-ref of="SetLoadDeadband(%) Load(0-10N)"() -> (w421:refnum<vi>)
      n323 = control-ref of="Gain 2"() -> (w418:refnum<vi>)
      n324 = control-ref of="pulses LoadDiff(2..10)"() -> (w417:refnum<vi>)
      n325 = control-ref of="pulses LoadDiff(11..50)"() -> (w416:refnum<vi>)
      n326 = control-ref of="PulseControl(diff<=3N)"() -> (w415:refnum<vi>)
      n327 = control-ref of="SetLoadDeadband(%)  2"() -> (w414:refnum<vi>)
      n328 = control-ref of="Vertical load (N)"() -> (w412:refnum<vi>)
      n329 = control-ref of="Offset  3"() -> (w410:refnum<vi>)
      n330 = control-ref of="Enter ByPass Load"() -> (w408:refnum<vi>)
      n331 = control-ref of="pulsesSent"() -> (w403:refnum<vi>)
      n332 = control-ref of="pulses"() -> (w402:refnum<vi>)
      n333 = control-ref of="actpid"() -> (w401:refnum<vi>)
      n334 = control-ref of="pulses LoadDiff(21..1000)"() -> (w399:refnum<vi>)
      n335 = control-ref of="Delay"() -> (w398:refnum<vi>)
      n336 = control-ref of="deadband"() -> (w397:refnum<vi>)
      n337 = Bundle By Name(cluster=w426, "PID.Ramp MulFac"=w424, "PID.pulses LoadDiffRamp(2..10)"=w423, "PID.PulseControlRamp(diff<=3N)"=w422, "PID.SetLoadDeadband(%) Load(0-10N)"=w421, "PID.PID gains out delay (microForce)"=w420, "PID.Ramp"=w419, "PID.Gain 2"=w418, "PID.pulses LoadDiff(2..10)"=w417, "PID.pulses LoadDiff(11..50)"=w416, "PID.PulseControl(diff<=3N)"=w415, "PID.SetLoadDeadband(%)  2"=w414, "PID.Dummy Run"=w413, "PID.Vertical load (N)"=w412, "PID.AutoTune"=w411, "PID.Offset 3"=w410, "PID.apply load"=w409, "PID.Enter ByPass Load"=w408, "PID.reinit 3"=w407, "PID.output range delay"=w406, "PID.PID gains out delay"=w405, "PID.Bypass Load"=w404, "PID.pulsesSent"=w403, "PID.pulses"=w402, "PID.actpid"=w401, "PID.gFF Rot"=w400, "PID.pulses LoadDiff(21..1000)"=w399, "PID.Delay"=w398, "PID.deadband"=w397) -> (w425:T15)
    }
    frame #10 {
      n338 = control-ref of="Tab Control 3"() -> (w490:refnum<vi>)
      n339 = control-ref of="Tab Control 19"() -> (w489:refnum<vi>)
      n340 = control-ref of="Tab Control 5"() -> (w450:refnum<vi>)
      n341 = control-ref of="Tab Control 14"() -> (w449:refnum<vi>)
      n342 = control-ref of="Tab Control 26"() -> (w448:refnum<vi>)
      n343 = control-ref of="DEPTH TRIP   ENABLE"() -> (w437:refnum<vi>)
      n344 = control-ref of="LOAD TRIP  ENABLE"() -> (w436:refnum<vi>)
      n345 = control-ref of="CYCLIC COF TRIP  ENABLE"() -> (w431:refnum<vi>)
      n346 = control-ref of="CYCLIC FF TRIP  ENABLE"() -> (w430:refnum<vi>)
      n347 = control-ref of="FF TRIP  ENABLE"() -> (w429:refnum<vi>)
      n348 = control-ref of="COF TRIP  ENABLE"() -> (w428:refnum<vi>)
      n349 = control-ref of="Re-initilaize"() -> (w487:refnum<vi>)
      n350 = control-ref of="Filter ON/OFF"() -> (w486:refnum<vi>)
      n351 = control-ref of="Apply Filter (FF)"() -> (w482:refnum<vi>)
      n352 = control-ref of="Apply Filter (Load)"() -> (w480:refnum<vi>)
      n353 = control-ref of="SAVE  2"() -> (w475:refnum<vi>)
      n354 = control-ref of="Enter Distance"() -> (w474:refnum<vi>)
      n355 = control-ref of="AE"() -> (w447:refnum<vi>)
      n356 = control-ref of="Heave Loop Delay"() -> (w446:refnum<vi>)
      n357 = control-ref of="Heave PID Speed"() -> (w445:refnum<vi>)
      n358 = control-ref of="Surge Jog Speed"() -> (w444:refnum<vi>)
      n359 = control-ref of="Heave Jog Speed"() -> (w443:refnum<vi>)
      n360 = control-ref of="Sway Loop Delay"() -> (w442:refnum<vi>)
      n361 = control-ref of="Sway PID Speed"() -> (w441:refnum<vi>)
      n362 = control-ref of="Sway Jog Speed"() -> (w440:refnum<vi>)
      n363 = control-ref of="DEPTH TRIP VALUE"() -> (w439:refnum<vi>)
      n364 = control-ref of="LOAD TRIP VALUE"() -> (w438:refnum<vi>)
      n365 = control-ref of="CYCLIC FF TRIP VALUE"() -> (w435:refnum<vi>)
      n366 = control-ref of="FF TRIP VALUE"() -> (w434:refnum<vi>)
      n367 = control-ref of="CYCLIC CoF TRIP VALUE"() -> (w433:refnum<vi>)
      n368 = control-ref of="COF TRIP VALUE"() -> (w432:refnum<vi>)
      n369 = control-ref of="JOG TRIP LOAD VALUE (N)"() -> (w427:refnum<vi>)
      n370 = control-ref of="SAMPLES"() -> (w488:refnum<vi>)
      n371 = control-ref of="TracHomeSurgeOffsetCounts 10MM"() -> (w485:refnum<vi>)
      n372 = control-ref of="TracHomeSwayOffsetCounts 10MM"() -> (w484:refnum<vi>)
      n373 = control-ref of="Acoustic Emission:"() -> (w483:refnum<vi>)
      n374 = control-ref of="Filter% 2"() -> (w481:refnum<vi>)
      n375 = control-ref of="Filter%"() -> (w479:refnum<vi>)
      n376 = control-ref of="Sway distance (mm)"() -> (w478:refnum<vi>)
      n377 = control-ref of="Surge distance (mm)"() -> (w477:refnum<vi>)
      n378 = control-ref of="DataSavingLoopDelay(ms)"() -> (w476:refnum<vi>)
      n379 = control-ref of="Sway Counts:"() -> (w473:refnum<vi>)
      n380 = control-ref of="Distance (mm): 3"() -> (w472:refnum<vi>)
      n381 = control-ref of="Surge Counts:"() -> (w471:refnum<vi>)
      n382 = control-ref of="Distance (mm): 2"() -> (w470:refnum<vi>)
      n383 = control-ref of="Distance (mm):"() -> (w469:refnum<vi>)
      n384 = control-ref of="Heave Counts:"() -> (w468:refnum<vi>)
      n385 = control-ref of="LRMHomeSurgeOffsetCounts"() -> (w467:refnum<vi>)
      n386 = control-ref of="LRMHomeSwayOffsetCounts"() -> (w466:refnum<vi>)
      n387 = control-ref of="TracHomeSurgeOffsetCounts 20MM"() -> (w465:refnum<vi>)
      n388 = control-ref of="TracHomeSwayOffsetCounts 20MM"() -> (w464:refnum<vi>)
      n389 = control-ref of="RotHomeSwayOffsetCounts"() -> (w463:refnum<vi>)
      n390 = control-ref of="RotHomeSurgeOffsetCounts"() -> (w462:refnum<vi>)
      n391 = control-ref of="Heave distance"() -> (w461:refnum<vi>)
      n392 = control-ref of="Zmm"() -> (w460:refnum<vi>)
      n393 = control-ref of="Heave Pulses/mm"() -> (w459:refnum<vi>)
      n394 = control-ref of="Surge Pulses/mm"() -> (w458:refnum<vi>)
      n395 = control-ref of="Sway Pulses/mm"() -> (w457:refnum<vi>)
      n396 = control-ref of="Heave Pitch"() -> (w456:refnum<vi>)
      n397 = control-ref of="Surge Pitch"() -> (w455:refnum<vi>)
      n398 = control-ref of="Sway Pitch"() -> (w454:refnum<vi>)
      n399 = control-ref of="Heave PPR"() -> (w453:refnum<vi>)
      n400 = control-ref of="Surge PPR"() -> (w452:refnum<vi>)
      n401 = control-ref of="Sway PPR"() -> (w451:refnum<vi>)
      n402 = Bundle By Name(cluster=w492, "Config Parameters.Tab Control 3"=w490, "Config Parameters.Tab Control 19"=w489, "Config Parameters.SAMPLES"=w488, "Config Parameters.Re-initilaize"=w487, "Config Parameters.Filter ON/OFF"=w486, "Config Parameters.TracHomeSurgeOffsetCounts 10MM"=w485, "Config Parameters.TracHomeSwayOffsetCounts 10MM"=w484, "Config Parameters.Acoustic Emission:"=w483, "Config Parameters.Apply Filter (FF)"=w482, "Config Parameters.Filter% 2"=w481, "Config Parameters.Apply Filter (Load)"=w480, "Config Parameters.Filter%"=w479, "Config Parameters.Sway distance (mm)"=w478, "Config Parameters.Surge distance (mm)"=w477, "Config Parameters.DataSavingLoopDelay(ms)"=w476, "Config Parameters.SAVE 2"=w475, "Config Parameters.Enter Distance"=w474, "Config Parameters.Sway Counts:"=w473, "Config Parameters.Distance (mm): 3"=w472, "Config Parameters.Surge Counts:"=w471, "Config Parameters.Distance (mm): 2"=w470, "Config Parameters.Distance (mm):"=w469, "Config Parameters.Heave Counts:"=w468, "Config Parameters.LRMHomeSurgeOffsetCounts"=w467, "Config Parameters.LRMHomeSwayOffsetCounts"=w466, "Config Parameters.TracHomeSurgeOffsetCounts 20MM"=w465, "Config Parameters.TracHomeSwayOffsetCounts 20MM"=w464, "Config Parameters.RotHomeSwayOffsetCounts"=w463, "Config Parameters.RotHomeSurgeOffsetCounts"=w462, "Config Parameters.Heave distance"=w461, "Config Parameters.Zmm"=w460, "Config Parameters.Heave Pulses/mm"=w459, "Config Parameters.Surge Pulses/mm"=w458, "Config Parameters.Sway Pulses/mm"=w457, "Config Parameters.Heave Pitch"=w456, "Config Parameters.Surge Pitch"=w455, "Config Parameters.Sway Pitch"=w454, "Config Parameters.Heave PPR"=w453, "Config Parameters.Surge PPR"=w452, "Config Parameters.Sway PPR"=w451, "Config Parameters.Tab Control 5"=w450, "Config Parameters.Tab Control 14"=w449, "Config Parameters.Tab Control 26"=w448, "Config Parameters.AE"=w447, "Config Parameters.Heave Loop Delay"=w446, "Config Parameters.Heave PID Speed"=w445, "Config Parameters.Surge Jog Speed"=w444, "Config Parameters.Heave Jog Speed"=w443, "Config Parameters.Sway Loop Delay"=w442, "Config Parameters.Sway PID Speed"=w441, "Config Parameters.Sway Jog Speed"=w440, "Config Parameters.DEPTH TRIP VALUE"=w439, "Config Parameters.LOAD TRIP VALUE"=w438, "Config Parameters.DEPTH TRIP   ENABLE"=w437, "Config Parameters.LOAD TRIP  ENABLE"=w436, "Config Parameters.CYCLIC FF TRIP VALUE"=w435, "Config Parameters.FF TRIP VALUE"=w434, "Config Parameters.CYCLIC CoF TRIP VALUE"=w433, "Config Parameters.COF TRIP VALUE"=w432, "Config Parameters.CYCLIC COF TRIP  ENABLE"=w431, "Config Parameters.CYCLIC FF TRIP  ENABLE"=w430, "Config Parameters.FF TRIP  ENABLE"=w429, "Config Parameters.COF TRIP  ENABLE"=w428, "Config Parameters.JOG TRIP LOAD VALUE (N)"=w427) -> (w491:T15)
    }
    frame #11 {
      n403 = control-ref of="Mx"() -> (w522:refnum<vi>)
      n404 = control-ref of="My"() -> (w521:refnum<vi>)
      n405 = control-ref of="Mz"() -> (w520:refnum<vi>)
      n406 = control-ref of="Fx(N)"() -> (w519:refnum<vi>)
      n407 = control-ref of="Fy(N)"() -> (w518:refnum<vi>)
      n408 = control-ref of="Fz(N)"() -> (w517:refnum<vi>)
      n409 = control-ref of="Load Cell Temp"() -> (w493:refnum<vi>)
      n410 = control-ref of="ClearAll"() -> (w527:refnum<vi>)
      n411 = control-ref of="ZeroAll"() -> (w516:refnum<vi>)
      n412 = control-ref of="delete Handle"() -> (w506:refnum<vi>)
      n413 = control-ref of="Create Handle"() -> (w505:refnum<vi>)
      n414 = control-ref of="stop 6"() -> (w502:refnum<vi>)
      n415 = control-ref of="running_flag"() -> (w501:refnum<vi>)
      n416 = control-ref of="Save Dwell"() -> (w523:refnum<vi>)
      n417 = control-ref of="Acq Delay (ms)"() -> (w515:refnum<vi>)
      n418 = control-ref of="Burst Delay (ms)"() -> (w514:refnum<vi>)
      n419 = control-ref of="SN"() -> (w512:refnum<vi>)
      n420 = control-ref of="Port"() -> (w509:refnum<vi>)
      n421 = control-ref of="ft_udp_handle"() -> (w500:refnum<vi>)
      n422 = control-ref of="get-data-return"() -> (w499:refnum<vi>)
      n423 = control-ref of="get-range-return"() -> (w498:refnum<vi>)
      n424 = control-ref of="zero-return"() -> (w497:refnum<vi>)
      n425 = control-ref of="filter-return"() -> (w496:refnum<vi>)
      n426 = control-ref of="initial-return"() -> (w495:refnum<vi>)
      n427 = control-ref of="deleteHandle-result"() -> (w494:refnum<vi>)
      n428 = control-ref of="model"() -> (w513:refnum<vi>)
      n429 = control-ref of="Sensor IP"() -> (w510:refnum<vi>)
      n430 = control-ref of="Mz(Nm)"() -> (w526:refnum<vi>)
      n431 = control-ref of="My(Nm)"() -> (w525:refnum<vi>)
      n432 = control-ref of="Mx(Nm)"() -> (w524:refnum<vi>)
      n433 = control-ref of="FFx(N)"() -> (w511:refnum<vi>)
      n434 = control-ref of="FFy(N)"() -> (w508:refnum<vi>)
      n435 = control-ref of="Load(N)"() -> (w507:refnum<vi>)
      n436 = control-ref of="ft_data"() -> (w504:refnum<vi>)
      n437 = control-ref of="ft_range"() -> (w503:refnum<vi>)
      n438 = Bundle By Name(cluster=w529, "Loading Com Port.ClearAll"=w527, "Loading Com Port.Mz(Nm)"=w526, "Loading Com Port.My(Nm)"=w525, "Loading Com Port.Mx(Nm)"=w524, "Loading Com Port.Save Dwell"=w523, "Loading Com Port.Mx"=w522, "Loading Com Port.My"=w521, "Loading Com Port.Mz"=w520, "Loading Com Port.Fx(N)"=w519, "Loading Com Port.Fy(N)"=w518, "Loading Com Port.Fz(N)"=w517, "Loading Com Port.ZeroAll"=w516, "Loading Com Port.Acq Delay (ms)"=w515, "Loading Com Port.Burst Delay (ms)"=w514, "Loading Com Port.model"=w513, "Loading Com Port.SN"=w512, "Loading Com Port.FFx(N)"=w511, "Loading Com Port.Sensor IP"=w510, "Loading Com Port.Port"=w509, "Loading Com Port.FFy(N)"=w508, "Loading Com Port.Load(N)"=w507, "Loading Com Port.delete Handle"=w506, "Loading Com Port.Create Handle"=w505, "Loading Com Port.ft_data"=w504, "Loading Com Port.ft_range"=w503, "Loading Com Port.stop 6"=w502, "Loading Com Port.running_flag"=w501, "Loading Com Port.ft_udp_handle"=w500, "Loading Com Port.get-data-return"=w499, "Loading Com Port.get-range-return"=w498, "Loading Com Port.zero-return"=w497, "Loading Com Port.filter-return"=w496, "Loading Com Port.initial-return"=w495, "Loading Com Port.deleteHandle-result"=w494, "Loading Com Port.Load Cell Temp"=w493) -> (w528:T15)
    }
    frame #12 {
      n439 = control-ref of="Read Heave Temp"() -> (w573:refnum<vi>)
      n440 = control-ref of="Manual Write Heave & Surge"() -> (w550:refnum<vi>)
      n441 = control-ref of="error out Read"() -> (w585:refnum<vi>)
      n442 = control-ref of="error out Write"() -> (w580:refnum<vi>)
      n443 = control-ref of="SURGE POSE"() -> (w586:refnum<vi>)
      n444 = control-ref of="HEAVE POSE"() -> (w584:refnum<vi>)
      n445 = control-ref of="State"() -> (w583:refnum<vi>)
      n446 = control-ref of="Homed"() -> (w582:refnum<vi>)
      n447 = control-ref of="Sequence ID"() -> (w581:refnum<vi>)
      n448 = control-ref of="faultCode"() -> (w579:refnum<vi>)
      n449 = control-ref of="Ack ID"() -> (w578:refnum<vi>)
      n450 = control-ref of="SPEED"() -> (w577:refnum<vi>)
      n451 = control-ref of="Distance"() -> (w576:refnum<vi>)
      n452 = control-ref of="Mode Command"() -> (w575:refnum<vi>)
      n453 = control-ref of="SPARE 2"() -> (w572:refnum<vi>)
      n454 = control-ref of="SPARE 1"() -> (w571:refnum<vi>)
      n455 = control-ref of="Spare 15"() -> (w570:refnum<vi>)
      n456 = control-ref of="Spare 14"() -> (w569:refnum<vi>)
      n457 = control-ref of="Spare 13"() -> (w568:refnum<vi>)
      n458 = control-ref of="Spare 12"() -> (w567:refnum<vi>)
      n459 = control-ref of="Spare 11"() -> (w566:refnum<vi>)
      n460 = control-ref of="Spare 10"() -> (w565:refnum<vi>)
      n461 = control-ref of="Spare 9"() -> (w564:refnum<vi>)
      n462 = control-ref of="Spare 8"() -> (w563:refnum<vi>)
      n463 = control-ref of="Spare 7"() -> (w562:refnum<vi>)
      n464 = control-ref of="Spare 6"() -> (w561:refnum<vi>)
      n465 = control-ref of="Spare 5"() -> (w560:refnum<vi>)
      n466 = control-ref of="Spare 4"() -> (w559:refnum<vi>)
      n467 = control-ref of="Spare 3"() -> (w558:refnum<vi>)
      n468 = control-ref of="Spare 2"() -> (w557:refnum<vi>)
      n469 = control-ref of="Spare 1"() -> (w556:refnum<vi>)
      n470 = control-ref of="Node Id"() -> (w555:refnum<vi>)
      n471 = control-ref of="SPARE 3"() -> (w554:refnum<vi>)
      n472 = control-ref of="SPARE 4"() -> (w553:refnum<vi>)
      n473 = control-ref of="fwMajor"() -> (w552:refnum<vi>)
      n474 = control-ref of="fwMinor"() -> (w551:refnum<vi>)
      n475 = control-ref of="SPARE 5"() -> (w548:refnum<vi>)
      n476 = control-ref of="Reserved"() -> (w547:refnum<vi>)
      n477 = control-ref of="SPARE 8"() -> (w546:refnum<vi>)
      n478 = control-ref of="SPARE 6"() -> (w545:refnum<vi>)
      n479 = control-ref of="SPARE 7"() -> (w544:refnum<vi>)
      n480 = control-ref of="SPARE 17"() -> (w543:refnum<vi>)
      n481 = control-ref of="SPARE 16"() -> (w542:refnum<vi>)
      n482 = control-ref of="SPARE 15"() -> (w541:refnum<vi>)
      n483 = control-ref of="SPARE 14"() -> (w540:refnum<vi>)
      n484 = control-ref of="SPARE 13"() -> (w539:refnum<vi>)
      n485 = control-ref of="SPARE 12"() -> (w538:refnum<vi>)
      n486 = control-ref of="SPARE 11"() -> (w537:refnum<vi>)
      n487 = control-ref of="SPARE 10"() -> (w536:refnum<vi>)
      n488 = control-ref of="SPARE 9"() -> (w535:refnum<vi>)
      n489 = control-ref of="System UPTIME"() -> (w534:refnum<vi>)
      n490 = control-ref of="Missed Packets"() -> (w533:refnum<vi>)
      n491 = control-ref of="faultCode Surge Right"() -> (w532:refnum<vi>)
      n492 = control-ref of="faultCode Surge Left"() -> (w531:refnum<vi>)
      n493 = control-ref of="faultCode Heave"() -> (w530:refnum<vi>)
      n494 = control-ref of="Heave and Surge Read"() -> (w574:refnum<vi>)
      n495 = control-ref of="Heave and Surge Write"() -> (w549:refnum<vi>)
      n496 = Bundle By Name(cluster=w588, "Heave AND Surge.SURGE POSE"=w586, "Heave AND Surge.error out Read"=w585, "Heave AND Surge.HEAVE POSE"=w584, "Heave AND Surge.State"=w583, "Heave AND Surge.Homed"=w582, "Heave AND Surge.Sequence ID"=w581, "Heave AND Surge.error out Write"=w580, "Heave AND Surge.faultCode"=w579, "Heave AND Surge.Ack ID"=w578, "Heave AND Surge.SPEED"=w577, "Heave AND Surge.Distance"=w576, "Heave AND Surge.Mode Command"=w575, "Heave AND Surge.Heave and Surge Read"=w574, "Heave AND Surge.Read Heave Temp"=w573, "Heave AND Surge.SPARE 2"=w572, "Heave AND Surge.SPARE 1"=w571, "Heave AND Surge.Spare 15"=w570, "Heave AND Surge.Spare 14"=w569, "Heave AND Surge.Spare 13"=w568, "Heave AND Surge.Spare 12"=w567, "Heave AND Surge.Spare 11"=w566, "Heave AND Surge.Spare 10"=w565, "Heave AND Surge.Spare 9"=w564, "Heave AND Surge.Spare 8"=w563, "Heave AND Surge.Spare 7"=w562, "Heave AND Surge.Spare 6"=w561, "Heave AND Surge.Spare 5"=w560, "Heave AND Surge.Spare 4"=w559, "Heave AND Surge.Spare 3"=w558, "Heave AND Surge.Spare 2"=w557, "Heave AND Surge.Spare 1"=w556, "Heave AND Surge.Node Id"=w555, "Heave AND Surge.SPARE 3"=w554, "Heave AND Surge.SPARE 4"=w553, "Heave AND Surge.fwMajor"=w552, "Heave AND Surge.fwMinor"=w551, "Heave AND Surge.Manual Write"=w550, "Heave AND Surge.Heave and Surge Write"=w549, "Heave AND Surge.SPARE 5"=w548, "Heave AND Surge.Reserved"=w547, "Heave AND Surge.SPARE 8"=w546, "Heave AND Surge.SPARE 6"=w545, "Heave AND Surge.SPARE 7"=w544, "Heave AND Surge.SPARE 17"=w543, "Heave AND Surge.SPARE 16"=w542, "Heave AND Surge.SPARE 15"=w541, "Heave AND Surge.SPARE 14"=w540, "Heave AND Surge.SPARE 13"=w539, "Heave AND Surge.SPARE 12"=w538, "Heave AND Surge.SPARE 11"=w537, "Heave AND Surge.SPARE 10"=w536, "Heave AND Surge.SPARE 9"=w535, "Heave AND Surge.System UPTIME"=w534, "Heave AND Surge.Missed Packets"=w533, "Heave AND Surge.faultCode Surge Right"=w532, "Heave AND Surge.faultCode Surge Left"=w531, "Heave AND Surge.faultCode Heave"=w530) -> (w587:T15)
    }
    frame #13 {
      n497 = control-ref of="Fine Tune Zone"() -> (w608:refnum<vi>)
      n498 = control-ref of="PID Delay (sec)"() -> (w607:refnum<vi>)
      n499 = control-ref of="Max_pos_limit"() -> (w606:refnum<vi>)
      n500 = control-ref of="Min_pos_limit"() -> (w605:refnum<vi>)
      n501 = control-ref of="i_limit"() -> (w604:refnum<vi>)
      n502 = control-ref of="pct_scale"() -> (w595:refnum<vi>)
      n503 = control-ref of="Deadband"() -> (w603:refnum<vi>)
      n504 = control-ref of="Kd"() -> (w602:refnum<vi>)
      n505 = control-ref of="Ki"() -> (w601:refnum<vi>)
      n506 = control-ref of="Kp"() -> (w600:refnum<vi>)
      n507 = control-ref of="Current Position"() -> (w599:refnum<vi>)
      n508 = control-ref of="Set Load"() -> (w598:refnum<vi>)
      n509 = control-ref of="Current Load"() -> (w597:refnum<vi>)
      n510 = control-ref of="Pulse delta"() -> (w596:refnum<vi>)
      n511 = control-ref of="Init Step"() -> (w594:refnum<vi>)
      n512 = control-ref of="Max Step Linit"() -> (w593:refnum<vi>)
      n513 = control-ref of="min_deadband_floor"() -> (w592:refnum<vi>)
      n514 = control-ref of="dynamic_spindle_noise_scalar"() -> (w591:refnum<vi>)
      n515 = control-ref of="min_finetune_floor"() -> (w590:refnum<vi>)
      n516 = control-ref of="filter_alpha"() -> (w589:refnum<vi>)
      n517 = Bundle By Name(cluster=w610, "New PID LOGIC.Fine Tune Zone"=w608, "New PID LOGIC.PID SDelay"=w607, "New PID LOGIC.Max_pos_limit"=w606, "New PID LOGIC.Min_pos_limit"=w605, "New PID LOGIC.i_limit"=w604, "New PID LOGIC.pct_scale"=w595, "New PID LOGIC.Deadband"=w603, "New PID LOGIC.Kd"=w602, "New PID LOGIC.Ki"=w601, "New PID LOGIC.Kp"=w600, "New PID LOGIC.Current Position"=w599, "New PID LOGIC.Set Load"=w598, "New PID LOGIC.Current Load"=w597, "New PID LOGIC.Pulse delta"=w596, "New PID LOGIC.Init Step"=w594, "New PID LOGIC.Max Step Linit"=w593, "New PID LOGIC.min_deadband_floor"=w592, "New PID LOGIC.dynamic_spindle_noise_scalar"=w591, "New PID LOGIC.min_finetune_floor"=w590, "New PID LOGIC.filter_alpha"=w589) -> (w609:T15)
    }
    frame #14 {
      n518 = control-ref of="Manual Write SWAY"() -> (w647:refnum<vi>)
      n519 = control-ref of="Read SWAY Temp"() -> (w628:refnum<vi>)
      n520 = control-ref of="error out Write  SWAY"() -> (w649:refnum<vi>)
      n521 = control-ref of="error out Read SWAY"() -> (w648:refnum<vi>)
      n522 = control-ref of="faultCode Rotary"() -> (w611:refnum<vi>)
      n523 = control-ref of="fwMajor"() -> (w666:refnum<vi>)
      n524 = control-ref of="Homed"() -> (w665:refnum<vi>)
      n525 = control-ref of="Rotary POSE"() -> (w664:refnum<vi>)
      n526 = control-ref of="State"() -> (w663:refnum<vi>)
      n527 = control-ref of="SWAY POSE"() -> (w662:refnum<vi>)
      n528 = control-ref of="Ack ID"() -> (w661:refnum<vi>)
      n529 = control-ref of="faultCode"() -> (w660:refnum<vi>)
      n530 = control-ref of="Node Id"() -> (w659:refnum<vi>)
      n531 = control-ref of="fwMinor"() -> (w658:refnum<vi>)
      n532 = control-ref of="Spare 6"() -> (w657:refnum<vi>)
      n533 = control-ref of="Spare 5"() -> (w656:refnum<vi>)
      n534 = control-ref of="Spare 4"() -> (w655:refnum<vi>)
      n535 = control-ref of="Spare 3"() -> (w654:refnum<vi>)
      n536 = control-ref of="Spare 2"() -> (w653:refnum<vi>)
      n537 = control-ref of="Spare 1"() -> (w652:refnum<vi>)
      n538 = control-ref of="Spare 7"() -> (w651:refnum<vi>)
      n539 = control-ref of="SPARE  5"() -> (w650:refnum<vi>)
      n540 = control-ref of="SPARE  4"() -> (w645:refnum<vi>)
      n541 = control-ref of="SPARE  3"() -> (w644:refnum<vi>)
      n542 = control-ref of="SPARE 2"() -> (w643:refnum<vi>)
      n543 = control-ref of="SPARE1"() -> (w642:refnum<vi>)
      n544 = control-ref of="Spare 15"() -> (w641:refnum<vi>)
      n545 = control-ref of="Spare 14"() -> (w640:refnum<vi>)
      n546 = control-ref of="Spare 13"() -> (w639:refnum<vi>)
      n547 = control-ref of="Spare 12"() -> (w638:refnum<vi>)
      n548 = control-ref of="Spare 11"() -> (w637:refnum<vi>)
      n549 = control-ref of="Spare 9"() -> (w636:refnum<vi>)
      n550 = control-ref of="Spare 8"() -> (w635:refnum<vi>)
      n551 = control-ref of="SPEED"() -> (w634:refnum<vi>)
      n552 = control-ref of="Distance"() -> (w633:refnum<vi>)
      n553 = control-ref of="Mode Command"() -> (w632:refnum<vi>)
      n554 = control-ref of="Sequence ID"() -> (w631:refnum<vi>)
      n555 = control-ref of="Spare 10"() -> (w629:refnum<vi>)
      n556 = control-ref of="faultCode Sway"() -> (w627:refnum<vi>)
      n557 = control-ref of="Missed Packets"() -> (w626:refnum<vi>)
      n558 = control-ref of="System UPTIME"() -> (w625:refnum<vi>)
      n559 = control-ref of="SPARE 6"() -> (w624:refnum<vi>)
      n560 = control-ref of="SPARE 7"() -> (w623:refnum<vi>)
      n561 = control-ref of="SPARE 9"() -> (w622:refnum<vi>)
      n562 = control-ref of="SPARE 11"() -> (w621:refnum<vi>)
      n563 = control-ref of="SPARE 10"() -> (w620:refnum<vi>)
      n564 = control-ref of="SPARE 8"() -> (w619:refnum<vi>)
      n565 = control-ref of="SPARE 13"() -> (w618:refnum<vi>)
      n566 = control-ref of="SPARE 12"() -> (w617:refnum<vi>)
      n567 = control-ref of="SPARE 17"() -> (w616:refnum<vi>)
      n568 = control-ref of="SPARE 16"() -> (w615:refnum<vi>)
      n569 = control-ref of="SPARE 15"() -> (w614:refnum<vi>)
      n570 = control-ref of="SPARE 14"() -> (w613:refnum<vi>)
      n571 = control-ref of="Reserved"() -> (w612:refnum<vi>)
      n572 = control-ref of="SWAY WRITE"() -> (w646:refnum<vi>)
      n573 = control-ref of="SWAY READ"() -> (w630:refnum<vi>)
      n574 = Bundle By Name(cluster=w668, "SWAY.fwMajor"=w666, "SWAY.Homed"=w665, "SWAY.Rotary POSE"=w664, "SWAY.State"=w663, "SWAY.SWAY POSE"=w662, "SWAY.Ack ID"=w661, "SWAY.faultCode"=w660, "SWAY.Node Id"=w659, "SWAY.fwMinor"=w658, "SWAY.Spare 6"=w657, "SWAY.Spare 5"=w656, "SWAY.Spare 4"=w655, "SWAY.Spare 3"=w654, "SWAY.Spare 2"=w653, "SWAY.Spare 1"=w652, "SWAY.Spare 7"=w651, "SWAY.SPARE  5"=w650, "SWAY.error out Write  SWAY"=w649, "SWAY.error out Read SWAY"=w648, "SWAY.Manual Write SWAY"=w647, "SWAY.SWAY WRITE"=w646, "SWAY.SPARE  4"=w645, "SWAY.SPARE  3"=w644, "SWAY.SPARE 2"=w643, "SWAY.SPARE 1"=w642, "SWAY.Spare 15"=w641, "SWAY.Spare 14"=w640, "SWAY.Spare 13"=w639, "SWAY.Spare 12"=w638, "SWAY.Spare 11"=w637, "SWAY.Spare 9"=w636, "SWAY.Spare 8"=w635, "SWAY.SPEED"=w634, "SWAY.Distance"=w633, "SWAY.Mode Command"=w632, "SWAY.Sequence ID"=w631, "SWAY.SWAY READ"=w630, "SWAY.Spare 10"=w629, "SWAY.Read SWAY Temp"=w628, "SWAY.faultCode Sway"=w627, "SWAY.Missed Packets"=w626, "SWAY.System UPTIME sway"=w625, "SWAY.SPARE 6"=w624, "SWAY.SPARE 7"=w623, "SWAY.SPARE 9"=w622, "SWAY.SPARE 11"=w621, "SWAY.SPARE 10"=w620, "SWAY.SPARE 8"=w619, "SWAY.SPARE 13"=w618, "SWAY.SPARE 12"=w617, "SWAY.SPARE 17"=w616, "SWAY.SPARE 16"=w615, "SWAY.SPARE 15"=w614, "SWAY.SPARE 14"=w613, "SWAY.Reserved"=w612, "SWAY.faultCode Rotary"=w611) -> (w667:T15)
    }
    frame #15 {
      n575 = control-ref of="Analysis Home new"() -> (w699:refnum<vi>)
      n576 = control-ref of="Refresh 2"() -> (w698:refnum<vi>)
      n577 = control-ref of="OPEN 4"() -> (w684:refnum<vi>)
      n578 = control-ref of="OPEN 3"() -> (w682:refnum<vi>)
      n579 = control-ref of="XY Graph"() -> (w677:refnum<vi>)
      n580 = control-ref of="OPEN 2"() -> (w674:refnum<vi>)
      n581 = control-ref of="OPEN 1"() -> (w673:refnum<vi>)
      n582 = control-ref of="Export"() -> (w670:refnum<vi>)
      n583 = control-ref of="MEAN"() -> (w697:refnum<vi>)
      n584 = control-ref of="SD"() -> (w696:refnum<vi>)
      n585 = control-ref of="VARIANCE"() -> (w695:refnum<vi>)
      n586 = control-ref of="MEAN"() -> (w694:refnum<vi>)
      n587 = control-ref of="SD"() -> (w693:refnum<vi>)
      n588 = control-ref of="VARIANCE"() -> (w692:refnum<vi>)
      n589 = control-ref of="MEAN"() -> (w691:refnum<vi>)
      n590 = control-ref of="SD"() -> (w690:refnum<vi>)
      n591 = control-ref of="VARIANCE"() -> (w689:refnum<vi>)
      n592 = control-ref of="MEAN"() -> (w688:refnum<vi>)
      n593 = control-ref of="SD"() -> (w687:refnum<vi>)
      n594 = control-ref of="VARIANCE"() -> (w686:refnum<vi>)
      n595 = control-ref of="File 4 Discription"() -> (w685:refnum<vi>)
      n596 = control-ref of="File Name 4"() -> (w683:refnum<vi>)
      n597 = control-ref of="File 3 Discription"() -> (w681:refnum<vi>)
      n598 = control-ref of="File Name 3"() -> (w680:refnum<vi>)
      n599 = control-ref of="File Name 2"() -> (w676:refnum<vi>)
      n600 = control-ref of="File Name 1"() -> (w675:refnum<vi>)
      n601 = control-ref of="File 1 Discription"() -> (w672:refnum<vi>)
      n602 = control-ref of="File 2 Discription"() -> (w671:refnum<vi>)
      n603 = control-ref of="Y-AXIS"() -> (w679:refnum<vi>)
      n604 = control-ref of="X-AXIS"() -> (w678:refnum<vi>)
      n605 = control-ref of="File Format"() -> (w669:refnum<vi>)
      n606 = Bundle By Name(cluster=w701, "Analysis Screen.Analysis Home"=w699, "Analysis Screen.Refresh 2"=w698, "Analysis Screen.MEAN 4"=w697, "Analysis Screen.SD 4"=w696, "Analysis Screen.VARIANCE 4"=w695, "Analysis Screen.MEAN  3"=w694, "Analysis Screen.SD  3"=w693, "Analysis Screen.VARIANCE  3"=w692, "Analysis Screen.MEAN 2"=w691, "Analysis Screen.SD  2"=w690, "Analysis Screen.VARIANCE 2"=w689, "Analysis Screen.MEAN"=w688, "Analysis Screen.SD"=w687, "Analysis Screen.VARIANCE"=w686, "Analysis Screen.File 4 Discription"=w685, "Analysis Screen.OPEN 4"=w684, "Analysis Screen.File Name 4"=w683, "Analysis Screen.OPEN 3"=w682, "Analysis Screen.File 3 Discription"=w681, "Analysis Screen.File Name 3"=w680, "Analysis Screen.Y-AXIS"=w679, "Analysis Screen.X-AXIS"=w678, "Analysis Screen.XY Graph"=w677, "Analysis Screen.File Name 2"=w676, "Analysis Screen.File Name 1"=w675, "Analysis Screen.OPEN 2"=w674, "Analysis Screen.OPEN 1"=w673, "Analysis Screen.File 1 Discription"=w672, "Analysis Screen.File 2 Discription"=w671, "Analysis Screen.Export"=w670, "Analysis Screen.File Format"=w669) -> (w700:T15)
    }
    frame #16 {
      n607 = control-ref of="Manual Write TRACTION"() -> (w731:refnum<vi>)
      n608 = control-ref of="Read TRACTION Temp"() -> (w718:refnum<vi>)
      n609 = control-ref of="error out Read TRACTION"() -> (w705:refnum<vi>)
      n610 = control-ref of="error out Write  TRACTION"() -> (w704:refnum<vi>)
      n611 = control-ref of="Spare 3"() -> (w702:refnum<vi>)
      n612 = control-ref of="faultCode Traction 2"() -> (w749:refnum<vi>)
      n613 = control-ref of="faultCode Traction 1"() -> (w748:refnum<vi>)
      n614 = control-ref of="Missed Packets"() -> (w747:refnum<vi>)
      n615 = control-ref of="System UPTIME"() -> (w746:refnum<vi>)
      n616 = control-ref of="SPARE 17"() -> (w745:refnum<vi>)
      n617 = control-ref of="SPARE 16"() -> (w744:refnum<vi>)
      n618 = control-ref of="SPARE 15"() -> (w743:refnum<vi>)
      n619 = control-ref of="SPARE 14"() -> (w742:refnum<vi>)
      n620 = control-ref of="SPARE 13"() -> (w741:refnum<vi>)
      n621 = control-ref of="SPARE 12"() -> (w740:refnum<vi>)
      n622 = control-ref of="SPARE 11"() -> (w739:refnum<vi>)
      n623 = control-ref of="SPARE 10"() -> (w738:refnum<vi>)
      n624 = control-ref of="SPARE 9"() -> (w737:refnum<vi>)
      n625 = control-ref of="SPARE 8"() -> (w736:refnum<vi>)
      n626 = control-ref of="SPARE 7"() -> (w735:refnum<vi>)
      n627 = control-ref of="SPARE 6"() -> (w734:refnum<vi>)
      n628 = control-ref of="Reserved"() -> (w733:refnum<vi>)
      n629 = control-ref of="SPARE  5"() -> (w732:refnum<vi>)
      n630 = control-ref of="SPARE  4"() -> (w729:refnum<vi>)
      n631 = control-ref of="SPARE  3"() -> (w728:refnum<vi>)
      n632 = control-ref of="SPARE 2"() -> (w727:refnum<vi>)
      n633 = control-ref of="SPARE 1"() -> (w726:refnum<vi>)
      n634 = control-ref of="Spare 7"() -> (w725:refnum<vi>)
      n635 = control-ref of="Spare 6"() -> (w724:refnum<vi>)
      n636 = control-ref of="Spare 5"() -> (w723:refnum<vi>)
      n637 = control-ref of="Spare 4"() -> (w722:refnum<vi>)
      n638 = control-ref of="Spare 2"() -> (w721:refnum<vi>)
      n639 = control-ref of="Spare 1"() -> (w720:refnum<vi>)
      n640 = control-ref of="Node Id"() -> (w719:refnum<vi>)
      n641 = control-ref of="fwMinor"() -> (w717:refnum<vi>)
      n642 = control-ref of="fwMajor"() -> (w716:refnum<vi>)
      n643 = control-ref of="faultCode"() -> (w715:refnum<vi>)
      n644 = control-ref of="TRACTION POSE 2"() -> (w714:refnum<vi>)
      n645 = control-ref of="TRACTION POSE 1"() -> (w713:refnum<vi>)
      n646 = control-ref of="Homed"() -> (w712:refnum<vi>)
      n647 = control-ref of="State"() -> (w711:refnum<vi>)
      n648 = control-ref of="Ack ID"() -> (w710:refnum<vi>)
      n649 = control-ref of="SPEED"() -> (w709:refnum<vi>)
      n650 = control-ref of="Distance"() -> (w708:refnum<vi>)
      n651 = control-ref of="Mode Command"() -> (w707:refnum<vi>)
      n652 = control-ref of="Sequence ID"() -> (w706:refnum<vi>)
      n653 = control-ref of="TRACTION WRITE"() -> (w730:refnum<vi>)
      n654 = control-ref of="TRACTION READ"() -> (w703:refnum<vi>)
      n655 = Bundle By Name(cluster=w751, "Traction.faultCode Traction 2"=w749, "Traction.faultCode Traction 1"=w748, "Traction.Missed Packets"=w747, "Traction.System UPTIME Traction"=w746, "Traction.SPARE 17"=w745, "Traction.SPARE 16"=w744, "Traction.SPARE 15"=w743, "Traction.SPARE 14"=w742, "Traction.SPARE 13"=w741, "Traction.SPARE 12"=w740, "Traction.SPARE 11"=w739, "Traction.SPARE 10"=w738, "Traction.SPARE 9"=w737, "Traction.SPARE 8"=w736, "Traction.SPARE 7"=w735, "Traction.SPARE 6"=w734, "Traction.Reserved"=w733, "Traction.SPARE  5"=w732, "Traction.Manual Write TRACTION"=w731, "Traction.TRACTION WRITE"=w730, "Traction.SPARE  4"=w729, "Traction.SPARE  3"=w728, "Traction.SPARE 2"=w727, "Traction.SPARE 1"=w726, "Traction.Spare 7"=w725, "Traction.Spare 6"=w724, "Traction.Spare 5"=w723, "Traction.Spare 4"=w722, "Traction.Spare 2"=w721, "Traction.Spare 1"=w720, "Traction.Node Id"=w719, "Traction.Read TRACTION Temp"=w718, "Traction.fwMinor"=w717, "Traction.fwMajor"=w716, "Traction.faultCode"=w715, "Traction.TRACTION POSE"=w714, "Traction.TRACTION POSE 2"=w713, "Traction.Homed"=w712, "Traction.State"=w711, "Traction.Ack ID"=w710, "Traction.SPEED"=w709, "Traction.Distance"=w708, "Traction.Mode Command"=w707, "Traction.Sequence ID"=w706, "Traction.error out Read TRACTION"=w705, "Traction.error out Write  TRACTION"=w704, "Traction.TRACTION READ"=w703, "Traction.Spare 3"=w702) -> (w750:T15)
    }
    frame #17 {
      n656 = control-ref of="Traction Receipe"() -> (w773:refnum<vi>)
      n657 = control-ref of="Total Execution Time"() -> (w784:refnum<vi>)
      n658 = control-ref of="Total Steps"() -> (w783:refnum<vi>)
      n659 = control-ref of="Duration / Step (s)"() -> (w782:refnum<vi>)
      n660 = control-ref of="Duration / Step (s)"() -> (w780:refnum<vi>)
      n661 = control-ref of="Speed (mm/s)"() -> (w778:refnum<vi>)
      n662 = control-ref of="SET entrainment Velocity"() -> (w772:refnum<vi>)
      n663 = control-ref of="Test Array Size"() -> (w771:refnum<vi>)
      n664 = control-ref of="SRR INDEX [ STRIBECK]"() -> (w770:refnum<vi>)
      n665 = control-ref of="Stribeck Size"() -> (w769:refnum<vi>)
      n666 = control-ref of="SET SRR"() -> (w768:refnum<vi>)
      n667 = control-ref of="ELAPSED TIMER"() -> (w767:refnum<vi>)
      n668 = control-ref of="BALL SET RPM"() -> (w766:refnum<vi>)
      n669 = control-ref of="DISC SET RPM"() -> (w765:refnum<vi>)
      n670 = control-ref of="SET LOAD"() -> (w764:refnum<vi>)
      n671 = control-ref of="TEMPERATURE READ"() -> (w763:refnum<vi>)
      n672 = control-ref of="SET TEMPERATURE"() -> (w762:refnum<vi>)
      n673 = control-ref of="Traction Size"() -> (w761:refnum<vi>)
      n674 = control-ref of="DISC SPEED (rpm)"() -> (w760:refnum<vi>)
      n675 = control-ref of="BALL SPEED (rpm)"() -> (w759:refnum<vi>)
      n676 = control-ref of="BALL WEAR TRACK"() -> (w758:refnum<vi>)
      n677 = control-ref of="DISC WEARTRACK"() -> (w757:refnum<vi>)
      n678 = control-ref of="SRR INDEX [ TRACTION]"() -> (w756:refnum<vi>)
      n679 = control-ref of="Start Index Type"() -> (w755:refnum<vi>)
      n680 = control-ref of="Ball (mm/sec)"() -> (w753:refnum<vi>)
      n681 = control-ref of="Disc (mm/sec)"() -> (w752:refnum<vi>)
      n682 = control-ref of="SRR Sweep Range (%)"() -> (w785:refnum<vi>)
      n683 = control-ref of="STRIBECK Fixed SRR List (%)"() -> (w781:refnum<vi>)
      n684 = control-ref of="SRR Sweep Range (%)"() -> (w779:refnum<vi>)
      n685 = control-ref of="Temperature Stages (°C)"() -> (w777:refnum<vi>)
      n686 = control-ref of="Load (N)"() -> (w776:refnum<vi>)
      n687 = control-ref of="Lubricant Name"() -> (w775:refnum<vi>)
      n688 = control-ref of="Profile File Name"() -> (w774:refnum<vi>)
      n689 = control-ref of="Enum - Menu"() -> (w754:refnum<vi>)
      n690 = Bundle By Name(cluster=w787, "Traction reciepe.SRR Sweep Range (%) Stribeck"=w785, "Traction reciepe.Traction Receipe"=w773, "Traction reciepe.Total Execution Time"=w784, "Traction reciepe.Total Steps"=w783, "Traction reciepe.Duration / Step (s)  Stribeck"=w782, "Traction reciepe.STRIBECK Fixed SRR List (%)"=w781, "Traction reciepe.Duration / Step (s) Traction"=w780, "Traction reciepe.SRR Sweep Range (%) traction"=w779, "Traction reciepe.Rolling Speed (mm/s)"=w778, "Traction reciepe.Temperature Stages (°C)"=w777, "Traction reciepe.Ball Load (N)"=w776, "Traction reciepe.Lubricant Name"=w775, "Traction reciepe.Profile File Name"=w774, "Traction reciepe.SET entrainment Velocity"=w772, "Traction reciepe.Test Array Size"=w771, "Traction reciepe.SRR INDEX [ STRIBECK]"=w770, "Traction reciepe.Stribeck Size"=w769, "Traction reciepe.SET SRR"=w768, "Traction reciepe.ELAPSED TIMER"=w767, "Traction reciepe.BALL SET RPM"=w766, "Traction reciepe.DISC SET RPM"=w765, "Traction reciepe.SET LOAD"=w764, "Traction reciepe.TEMPERATURE READ"=w763, "Traction reciepe.SET TEMPERATURE"=w762, "Traction reciepe.Traction Size"=w761, "Traction reciepe.DISC SPEED (rpm)"=w760, "Traction reciepe.BALL SPEED (rpm)"=w759, "Traction reciepe.BALL WEAR TRACK"=w758, "Traction reciepe.DISC WEARTRACK"=w757, "Traction reciepe.SRR INDEX [ TRACTION]"=w756, "Traction reciepe.Start Index Type"=w755, "Traction reciepe.Enum - Menu"=w754, "Traction reciepe.Ball (mm/sec)"=w753, "Traction reciepe.Disc (mm/sec)"=w752) -> (w786:T15)
    }
    frame #18 {
      n691 = control-ref of="SPEED SELECTION : MTM"() -> (w816:refnum<vi>)
      n692 = control-ref of="TEST SELECTION (MTM)"() -> (w815:refnum<vi>)
      n693 = control-ref of="MTM Test Selection"() -> (w814:refnum<vi>)
      n694 = control-ref of="TEST SELECTION (MTM) 2"() -> (w802:refnum<vi>)
      n695 = control-ref of="SPEED SELECTION : MTM 2"() -> (w801:refnum<vi>)
      n696 = control-ref of="MTM Test Selection 2"() -> (w800:refnum<vi>)
      n697 = control-ref of="Demo Mode Display"() -> (w844:refnum<vi>)
      n698 = control-ref of="Main Tab sequence for selection"() -> (w841:refnum<vi>)
      n699 = control-ref of="Ramp Tab"() -> (w840:refnum<vi>)
      n700 = control-ref of="e.v/ssr"() -> (w839:refnum<vi>)
      n701 = control-ref of="File Path Tab"() -> (w813:refnum<vi>)
      n702 = control-ref of="Step Sequence Indication Tab"() -> (w808:refnum<vi>)
      n703 = control-ref of="Disc Speed Indicator"() -> (w789:refnum<vi>)
      n704 = control-ref of="HomeTraction"() -> (w845:refnum<vi>)
      n705 = control-ref of="Traction Step Update Details"() -> (w842:refnum<vi>)
      n706 = control-ref of="E.Velocity"() -> (w831:refnum<vi>)
      n707 = control-ref of="Ramp Up   Disc"() -> (w828:refnum<vi>)
      n708 = control-ref of="Ramp Up"() -> (w821:refnum<vi>)
      n709 = control-ref of="BallSpeed Exceed Indication"() -> (w818:refnum<vi>)
      n710 = control-ref of="Apply"() -> (w817:refnum<vi>)
      n711 = control-ref of="Save"() -> (w811:refnum<vi>)
      n712 = control-ref of="Import"() -> (w810:refnum<vi>)
      n713 = control-ref of="Calculate Step"() -> (w806:refnum<vi>)
      n714 = control-ref of="Enter Fixed E.Velocity"() -> (w838:refnum<vi>)
      n715 = control-ref of="Enter Final SRR"() -> (w837:refnum<vi>)
      n716 = control-ref of="Enter initial SRR"() -> (w836:refnum<vi>)
      n717 = control-ref of="Enter Fixed SRR"() -> (w835:refnum<vi>)
      n718 = control-ref of="Enter the Final E.Velocity (m/s)"() -> (w834:refnum<vi>)
      n719 = control-ref of="Enter initial E.Velocity (m/s)"() -> (w833:refnum<vi>)
      n720 = control-ref of="Ball WTD"() -> (w832:refnum<vi>)
      n721 = control-ref of="Enter the Final Velocity (m/s)"() -> (w830:refnum<vi>)
      n722 = control-ref of="Enter initial Velocity (m/s)"() -> (w829:refnum<vi>)
      n723 = control-ref of="Initial DiscSpeed (RPM)"() -> (w827:refnum<vi>)
      n724 = control-ref of="Final Speed (RPM)"() -> (w826:refnum<vi>)
      n725 = control-ref of="Final Speed (RPM) Ball"() -> (w825:refnum<vi>)
      n726 = control-ref of="Initial Speed (RPM) Ball"() -> (w824:refnum<vi>)
      n727 = control-ref of="Enter the Final Velocity (m/s) Ball"() -> (w823:refnum<vi>)
      n728 = control-ref of="Enter initial Velocity (m/s) Ball"() -> (w822:refnum<vi>)
      n729 = control-ref of="Enter the Speed (m/sec):"() -> (w799:refnum<vi>)
      n730 = control-ref of="Enter the Speed (m/sec):"() -> (w798:refnum<vi>)
      n731 = control-ref of="Enter the Speed (RPM):"() -> (w797:refnum<vi>)
      n732 = control-ref of="Enter the Speed (RPM):Ball"() -> (w794:refnum<vi>)
      n733 = control-ref of="Wear Track Diameter (mm)"() -> (w790:refnum<vi>)
      n734 = control-ref of="ExceedBallSpeed"() -> (w788:refnum<vi>)
      n735 = control-ref of="Traction Message"() -> (w843:refnum<vi>)
      n736 = control-ref of="ExceedBallSpeed step"() -> (w820:refnum<vi>)
      n737 = control-ref of="ExceedDiscSpeed"() -> (w819:refnum<vi>)
      n738 = control-ref of="File Path String"() -> (w812:refnum<vi>)
      n739 = control-ref of="Step Sequence Indication"() -> (w807:refnum<vi>)
      n740 = control-ref of="ExceedDiscSpeed  Cinstant Speed"() -> (w804:refnum<vi>)
      n741 = control-ref of="ExceedBallSpeed Constant"() -> (w803:refnum<vi>)
      n742 = control-ref of="Lower Spped"() -> (w796:refnum<vi>)
      n743 = control-ref of="Upper"() -> (w795:refnum<vi>)
      n744 = control-ref of="StepTable"() -> (w805:refnum<vi>)
      n745 = control-ref of="Disc Motion Direction:"() -> (w793:refnum<vi>)
      n746 = control-ref of="Ball Motion Direction :"() -> (w792:refnum<vi>)
      n747 = control-ref of="Motion Mode:"() -> (w791:refnum<vi>)
      n748 = control-ref of="File Path :"() -> (w809:refnum<vi>)
      n749 = Bundle By Name(cluster=w847, "Traction Control.HomeTraction"=w845, "Traction Control.Demo Mode Display"=w844, "Traction Control.Traction Message"=w843, "Traction Control.Traction Step Update Details"=w842, "Traction Control.Main Tab sequence for selection"=w841, "Traction Control.Ramp Tab"=w840, "Traction Control.e.v/ssr"=w839, "Traction Control.Enter Fixed E.Velocity"=w838, "Traction Control.Enter Final SRR"=w837, "Traction Control.Enter initial SRR"=w836, "Traction Control.Enter Fixed SRR"=w835, "Traction Control.Enter the Final E.Velocity (m/s)"=w834, "Traction Control.Enter initial E.Velocity (m/s)"=w833, "Traction Control.Ball WTD"=w832, "Traction Control.E.Velocity"=w831, "Traction Control.Enter the Final Velocity (m/s)"=w830, "Traction Control.Enter initial Velocity (m/s)"=w829, "Traction Control.Ramp Up   Disc"=w828, "Traction Control.Initial DiscSpeed (RPM)"=w827, "Traction Control.Final Speed (RPM) Ball"=w826, "Traction Control.Final Speed (RPM)"=w825, "Traction Control.Initial Speed (RPM) Ball"=w824, "Traction Control.Enter the Final Velocity (m/s) Ball"=w823, "Traction Control.Enter initial Velocity (m/s) Ball"=w822, "Traction Control.Ramp Up"=w821, "Traction Control.ExceedBallSpeed step"=w820, "Traction Control.ExceedDiscSpeed"=w819, "Traction Control.BallSpeed Exceed Indication"=w818, "Traction Control.Apply"=w817, "Traction Control.SPEED SELECTION : MTM"=w816, "Traction Control.TEST SELECTION (MTM)"=w815, "Traction Control.MTM Test Selection"=w814, "Traction Control.File Path Tab"=w813, "Traction Control.File Path String"=w812, "Traction Control.Save"=w811, "Traction Control.Import"=w810, "Traction Control.File Path :"=w809, "Traction Control.Step Sequence Indication Tab"=w808, "Traction Control.Step Sequence Indication"=w807, "Traction Control.Calculate Step"=w806, "Traction Control.StepTable"=w805, "Traction Control.ExceedDiscSpeed  Cinstant Speed"=w804, "Traction Control.ExceedBallSpeed Constant"=w803, "Traction Control.TEST SELECTION (MTM) 2"=w802, "Traction Control.SPEED SELECTION : MTM 3"=w801, "Traction Control.MTM Test Selection 2"=w800, "Traction Control.Enter the Speed (m/sec):"=w799, "Traction Control.Enter the Speed (m/sec):  2"=w798, "Traction Control.Enter the Speed (RPM):"=w797, "Traction Control.Lower Spped"=w796, "Traction Control.Upper"=w795, "Traction Control.Enter the Speed (RPM):Ball"=w794, "Traction Control.Disc Motion Direction:"=w793, "Traction Control.Ball Motion Direction :"=w792, "Traction Control.Motion Mode:"=w791, "Traction Control.Wear Track Diameter (mm)"=w790, "Traction Control.Disc Speed Indicator"=w789, "Traction Control.ExceedBallSpeed"=w788) -> (w846:T15)
    }
    frame #19 {
      n750 = control-ref of="Gains"() -> (w849:refnum<vi>)
      n751 = control-ref of="Signal Energy"() -> (w853:refnum<vi>)
      n752 = control-ref of="Amplitude db_AE"() -> (w852:refnum<vi>)
      n753 = control-ref of="Peak Amplitude"() -> (w851:refnum<vi>)
      n754 = control-ref of="AE Ring-Down Counts"() -> (w850:refnum<vi>)
      n755 = control-ref of="Manual Write Acquostic"() -> (w848:refnum<vi>)
      n756 = control-ref of="error out"() -> (w858:refnum<vi>)
      n757 = control-ref of="error in (no error)"() -> (w857:refnum<vi>)
      n758 = control-ref of="Downlink Packet"() -> (w856:refnum<vi>)
      n759 = control-ref of="Uplink Packet"() -> (w855:refnum<vi>)
      n760 = control-ref of="Last Config Rejected"() -> (w863:refnum<vi>)
      n761 = control-ref of="rx command count"() -> (w862:refnum<vi>)
      n762 = control-ref of="Current Filter Id"() -> (w861:refnum<vi>)
      n763 = control-ref of="Isolated Gain"() -> (w860:refnum<vi>)
      n764 = control-ref of="DAQ Status"() -> (w859:refnum<vi>)
      n765 = control-ref of="data out"() -> (w854:refnum<vi>)
      n766 = Bundle By Name(cluster=w865, "Acquostic.Last Config Rejected"=w863, "Acquostic.rx command count"=w862, "Acquostic.Current Filter Id"=w861, "Acquostic.Isolated Gain"=w860, "Acquostic.DAQ Status"=w859, "Acquostic.error out"=w858, "Acquostic.error in (no error)"=w857, "Acquostic.Downlink Packet"=w856, "Acquostic.Uplink Packet"=w855, "Acquostic.data out"=w854, "Acquostic.Signal Energy"=w853, "Acquostic.Amplitude db_AE"=w852, "Acquostic.Peak Amplitude"=w851, "Acquostic.AE Ring-Down Counts"=w850, "Acquostic.Gains"=w849, "Acquostic.Manual Write Acquostic"=w848) -> (w864:T15)
    }
  }
  n767 = call <userlib>:"Fit VI window to Largest Dec.vi"() -> ("error out"=w57:errorcluster, "dup VI Ref"=w54:refnum<vi>)  [unwired: 6 in]
  n768 = invoke on="Invoke Node" class="VI" method="FP.Run-Time Position.Maximized"(reference=w54, error in=w57) -> (error out=w56:errorcluster)  [unwired: 2 in, 3 out]
  n769 = call <vilib>:"Clear Errors.vi"("error in (no error)"=w56) -> ("error out"=w55:errorcluster)  [unwired: 5 in, 1 out]
  n770 = control-ref of="This VI"() -> (w60:refnum<vi>)
  n771 = invoke on="Invoke Node" class="VI" method="Default Vals.Reinit All"(reference=w60, error in=w55) -> (reference out=w58:refnum<vi>, error out=w59:errorcluster)  [unwired: 1 in, 1 out]
  n772 = Close Reference(reference=w58, error in (no error)=w59) -> (error out=w53:errorcluster)
  n773 = call "Create User Event - Stop.vi"("error in (no error)"=w53) -> ("error out"=w6:errorcluster, "User Event - Stop"=w10:refnum<user-event>)  [unwired: 9 in]
  n774 = call "main screen queue out Unitest.vi"("error in (no error)"=w6) -> ("error out"=w80:errorcluster, "output Queue"=w8:T16)  [unwired: 9 in]
  n775 = Unbundle By Name(w8) -> ("RAMP MOTOR COM LOOP"=w46:refnum<queue>)
  n776 = Unbundle By Name(w8) -> ("TEMPERATURE COM LOOP"=w48:refnum<queue>)
  n777 = Unbundle By Name(w8) -> ("ECR PORT"=w45:refnum<queue>)
  n778 = Unbundle By Name(w8) -> ("SWAY MOTOR COM LOOP"=w50:refnum<queue>)
  n779 = Unbundle By Name(w8) -> ("UI Loop"=w78:refnum<queue>)
  n780 = Unbundle By Name(w8) -> ("LOAD COM LOOP"=w51:refnum<queue>)
  n781 = Unbundle By Name(w8) -> ("HEAVE MOTOR COM LOOP"=w35:refnum<queue>)
  n782 = Unbundle By Name(w8) -> ("HUMIDITY COM PORT"=w44:refnum<queue>)
  n783 = Unbundle By Name(w8) -> ("PROGRAM LOOP"=w43:refnum<queue>)
  n784 = Unbundle By Name(w8) -> ("MONITOR LOOP"=w42:refnum<queue>)
  n785 = Unbundle By Name(w8) -> ("LOAD PID"=w41:refnum<queue>)
  n786 = Unbundle By Name(w8) -> ("REPORT"=w40:refnum<queue>)
  n787 = register-events(w10) -> (reference out=w72:refnum<event-registration>, error out=w70:errorcluster)  [unwired: 2 in]
  n788 = Unbundle By Name(w8) -> ("ACOUSTIC"=w7:refnum<queue>)
  n789 = Merge Errors(w70, w80) -> (w71:errorcluster)
  n790 = node-c288() -> (w26:T17)  [unwired: 4 in]
  n791 = node-c288() -> (w4:T17)  [unwired: 4 in]
  n792 = node-c288() -> (w20:T17)  [unwired: 4 in]
  n793 = node-c288() -> (w28:T17)  [unwired: 4 in]
  n794 = node-c288() -> (w30:T17)  [unwired: 4 in]
  n795 = node-c288() -> (w2:T17)  [unwired: 4 in]
  n796 = disable-structure "Diagram Disable Structure" shown="Disabled" {
    disable-tunnel: w44 -> [w870 _]
    disable-tunnel: w9 -> [w869 _]
    disable-tunnel: w10 -> [w868 _]
    disable-tunnel: w6 -> [w867 _]
    disable-tunnel: [w866 _] -> w16
    frame Disabled {
      n797 = while {
        shift-right: [w881] -> _
        shift-left: w869 -> [w882]
        tunnel: [w875] -> w866
        tunnel: w870 -> [w873]
        tunnel: w867 -> [w872]
        tunnel: w868 -> [w871]
        stop <- w880 stop-if-true
        # "Humidity  Handling Loop"
        n798 = call "Dequeue Message.vi"("error in (no error)"=w872, "Message Queue"=w873) -> ("error out"=w879:errorcluster, "Message Data"=w877:variant, "Message"=w878:string, "dup Message Queue"=w876:refnum<queue>)  [unwired: 6 in]
        n799 = case "Message Cases" shown="\"Humidity Main\"" w878 {
          selector: w878 -> [_ _ _ _ _ w926]
          tunnel: w876 -> [w883 w894 _ w913 w925 _]
          tunnel: w879 -> [w886 w891 w910 w917 w919 _]
          tunnel: [w887 w895 w904 w915 w921 w927] -> w874
          tunnel: w882 -> [w885 w893 w909 w916 w924 w928]
          tunnel: [w885 w893 w909 w916 w924 w928] -> w881
          tunnel: [_ _ _ _ TRUE _] -> w880
          tunnel: w877 -> [_ _ w908 _ _ _]
          tunnel: w871 -> [_ _ _ _ w918 _]
          frame "init" {
            # "Initialize - All initialization work should take place in this message, since other loops can potentially enqueue messages that execute immediately after this one."
            n800 = call-poly "Enqueue Message.vi"("error in (no error)"=w886, "Message"="Humidity Main", "Message Queue"=w883) -> ("error out"=w887:errorcluster)  [unwired: 7 in, 1 out]
          }
          frame "Humidity Main" {
            n801 = Unbundle By Name(w893) -> ("Main Home Screen.EXIT"=w892:refnum<vi>)
            n802 = property on="Property Node" class="Bool (strict)"(reference=w892) -> (reference out=w889:refnum<vi>, error out=w890:errorcluster, "Value"=w888:bool)  [unwired: 1 in]
            n803 = case shown="False" w888 {
              tunnel: [w898 w902] -> w895
              tunnel: w894 -> [w897 w901]
              tunnel: w891 -> [w896 w900]
              frame True {
                n804 = call-poly "Enqueue Message.vi"("error in (no error)"=w896, "Message"="Confirm Quit", "Message Queue"=w897) -> ("error out"=w898:errorcluster)  [unwired: 7 in, 1 out]
              }
              frame False {
                n805 = call-poly "Enqueue Message.vi"("error in (no error)"=w900, "Message"="Humidity Main", "Message Queue"=w901) -> ("error out"=w902:errorcluster)  [unwired: 7 in, 1 out]
              }
            }
            n806 = Close Reference(reference=w889, error in (no error)=w890) -> ()  [unwired: 1 out]
          }
          frame "Error" {
            # "#CodeRecommended - If you ever change the name of this \"Error\" message, you'll need to update the name in the Check Loop Error.vi as well."
            # "#CodeRecommended - Consider creating a system for logging errors in some way. These errors are for notification purposes only. Handling of specific errors should be performed in the message frames that generated the error."
            # "Error - Display an error dialog. This message is sent by the \"Error Handler\" VIs at the end of other loops in this application."
            n807 = Variant To Data(error in=w910, type=errorcluster {"status"=FALSE, "code"=0, "source"=""} ("error constant"), Variant=w908) -> (data=w906:errorcluster, error out=w905:errorcluster)
            n808 = call <vilib>:"Simple Error Handler.vi"("error in (no error)"=w906) -> ()  [unwired: 4 in, 5 out]
            n809 = Merge Errors(w905) -> (w904:errorcluster)
          }
          frame "Confirm Quit" {
            # "#CodeNeeded - If you want to provide an \"Are you sure\" dialog (or some other notification) before the application exits, place that code here. This message is typically sent from a Panel Close? event."
            # "Confirm Quit - Message that can confirm whether or not the user wants to exit the application."
            n810 = call-poly "Enqueue Message.vi"("Priority Message? (F)"=TRUE, "error in (no error)"=w917, "Message"="Exit", "Message Queue"=w913) -> ("error out"=w914:errorcluster)  [unwired: 6 in, 1 out]
            n811 = Merge Errors(w914) -> (w915:errorcluster)
          }
          frame "Exit" {
            # "Stop the VI"
            # "Release the message queue reference"
            # "#CodeNeeded - Add any required cleanup code here. Note that if 'Exit' was called as a result of an error, an error dialog will be displayed. Add any custom error handling for an 'Exit' condition here as well."
            # "Exit - Exit the application."
            n812 = call "Fire User Event - Stop.vi"("User Event - Stop"=w918) -> ("error out"=w920:errorcluster)  [unwired: 10 in]
            n813 = Release Queue(queue=w925, error in (no error)=w919) -> (error out=w922:errorcluster)  [unwired: 1 in, 2 out]
            n814 = Merge Errors(w920, w922) -> (w921:errorcluster)
          }
          frame Default {
            # "'Default' case only runs if there is a message that isn't defined in any of the other cases.  Output a programming error."
            n815 = xnode ("Error Ring")("parameter 0"=w926) -> ("error out"=w927:errorcluster)
          }
        }
        n816 = call "LAB-IQ Error Handler - Message Handling Loop.vi"("error in (no error)"=w874, "Message Queue"=w876) -> ("dup error in"=w875:errorcluster)  [unwired: 8 in, 1 out]
      }
    }
    frame Enabled {
    }
  }
  n817 = disable-structure "Diagram Disable Structure" shown="Disabled" {
    disable-tunnel: w45 -> [w940 _]
    disable-tunnel: w9 -> [w939 _]
    disable-tunnel: w10 -> [w938 _]
    disable-tunnel: w6 -> [w937 w1006]
    disable-tunnel: [w936 w1006] -> w17
    frame Disabled {
      n818 = while {
        shift-right: [w951] -> _
        shift-left: w939 -> [w952]
        tunnel: [w945] -> w936
        tunnel: w940 -> [w943]
        tunnel: w937 -> [w942]
        tunnel: w938 -> [w941]
        stop <- w950 stop-if-true
        # "ECR  Handling Loop"
        n819 = call "Dequeue Message.vi"("error in (no error)"=w942, "Message Queue"=w943) -> ("error out"=w949:errorcluster, "Message Data"=w947:variant, "Message"=w948:string, "dup Message Queue"=w946:refnum<queue>)  [unwired: 6 in]
        n820 = case "Message Cases" shown="\"ECR Main\"" w948 {
          selector: w948 -> [_ _ _ _ _ w996]
          tunnel: w946 -> [w953 w964 _ w983 w995 _]
          tunnel: w949 -> [w956 w961 w980 w987 w989 _]
          tunnel: [w957 w965 w974 w985 w991 w997] -> w944
          tunnel: w952 -> [w955 w963 w979 w986 w994 w998]
          tunnel: [w955 w963 w979 w986 w994 w998] -> w951
          tunnel: [_ _ _ _ TRUE _] -> w950
          tunnel: w947 -> [_ _ w978 _ _ _]
          tunnel: w941 -> [_ _ _ _ w988 _]
          frame "init" {
            # "Initialize - All initialization work should take place in this message, since other loops can potentially enqueue messages that execute immediately after this one."
            n821 = call-poly "Enqueue Message.vi"("error in (no error)"=w956, "Message"="ECR Main", "Message Queue"=w953) -> ("error out"=w957:errorcluster)  [unwired: 7 in, 1 out]
          }
          frame "ECR Main" {
            n822 = Unbundle By Name(w963) -> ("Main Home Screen.EXIT"=w962:refnum<vi>)
            n823 = property on="Property Node" class="Bool (strict)"(reference=w962) -> (reference out=w959:refnum<vi>, error out=w960:errorcluster, "Value"=w958:bool)  [unwired: 1 in]
            n824 = case shown="False" w958 {
              tunnel: [w968 w972] -> w965
              tunnel: w964 -> [w967 w971]
              tunnel: w961 -> [w966 w970]
              frame True {
                n825 = call-poly "Enqueue Message.vi"("error in (no error)"=w966, "Message"="Confirm Quit", "Message Queue"=w967) -> ("error out"=w968:errorcluster)  [unwired: 7 in, 1 out]
              }
              frame False {
                n826 = call-poly "Enqueue Message.vi"("error in (no error)"=w970, "Message"="ECR Main", "Message Queue"=w971) -> ("error out"=w972:errorcluster)  [unwired: 7 in, 1 out]
              }
            }
            n827 = Close Reference(reference=w959, error in (no error)=w960) -> ()  [unwired: 1 out]
          }
          frame "Error" {
            # "#CodeRecommended - If you ever change the name of this \"Error\" message, you'll need to update the name in the Check Loop Error.vi as well."
            # "#CodeRecommended - Consider creating a system for logging errors in some way. These errors are for notification purposes only. Handling of specific errors should be performed in the message frames that generated the error."
            # "Error - Display an error dialog. This message is sent by the \"Error Handler\" VIs at the end of other loops in this application."
            n828 = Variant To Data(error in=w980, type=errorcluster {"status"=FALSE, "code"=0, "source"=""} ("error constant"), Variant=w978) -> (data=w976:errorcluster, error out=w975:errorcluster)
            n829 = call <vilib>:"Simple Error Handler.vi"("error in (no error)"=w976) -> ()  [unwired: 4 in, 5 out]
            n830 = Merge Errors(w975) -> (w974:errorcluster)
          }
          frame "Confirm Quit" {
            # "#CodeNeeded - If you want to provide an \"Are you sure\" dialog (or some other notification) before the application exits, place that code here. This message is typically sent from a Panel Close? event."
            # "Confirm Quit - Message that can confirm whether or not the user wants to exit the application."
            n831 = call-poly "Enqueue Message.vi"("Priority Message? (F)"=TRUE, "error in (no error)"=w987, "Message"="Exit", "Message Queue"=w983) -> ("error out"=w984:errorcluster)  [unwired: 6 in, 1 out]
            n832 = Merge Errors(w984) -> (w985:errorcluster)
          }
          frame "Exit" {
            # "Stop the VI"
            # "Release the message queue reference"
            # "#CodeNeeded - Add any required cleanup code here. Note that if 'Exit' was called as a result of an error, an error dialog will be displayed. Add any custom error handling for an 'Exit' condition here as well."
            # "Exit - Exit the application."
            n833 = call "Fire User Event - Stop.vi"("User Event - Stop"=w988) -> ("error out"=w990:errorcluster)  [unwired: 10 in]
            n834 = Release Queue(queue=w995, error in (no error)=w989) -> (error out=w992:errorcluster)  [unwired: 1 in, 2 out]
            n835 = Merge Errors(w990, w992) -> (w991:errorcluster)
          }
          frame Default {
            # "'Default' case only runs if there is a message that isn't defined in any of the other cases.  Output a programming error."
            n836 = xnode ("Error Ring")("parameter 0"=w996) -> ("error out"=w997:errorcluster)
          }
        }
        n837 = call "LAB-IQ Error Handler - Message Handling Loop.vi"("error in (no error)"=w944, "Message Queue"=w946) -> ("dup error in"=w945:errorcluster)  [unwired: 8 in, 1 out]
      }
    }
    frame Enabled {
    }
  }
  n838 = while "Timed Loop" {
    shift-right: [w1008] -> _
    shift-left: w9 -> [w1027]
    tunnel: [w1021] -> w13
    tunnel: w40 -> [w1019]
    tunnel: w6 -> [w1018]
    tunnel: w10 -> [w1017]
    stop <- w1026 stop-if-true
    # "Report  Handling Loop"
    n839 = call "Dequeue Message.vi"("error in (no error)"=w1018, "Message Queue"=w1019) -> ("error out"=w1025:errorcluster, "Message Data"=w1023:variant, "Message"=w1024:string, "dup Message Queue"=w1022:refnum<queue>)  [unwired: 6 in]
    n840 = case "Message Cases" shown="\"Report Main\"" w1024 {
      selector: w1024 -> [_ _ _ _ _ w1072]
      tunnel: w1022 -> [w1028 w1040 _ w1059 w1071 _]
      tunnel: w1025 -> [w1031 w1038 w1056 w1063 w1065 _]
      tunnel: [w1032 w1041 w1050 w1061 w1067 w1073] -> w1020
      tunnel: w1027 -> [w1030 w1033 w1055 w1062 w1070 w1074]
      tunnel: [w1030 w1033 w1055 w1062 w1070 w1074] -> w1008
      tunnel: [_ _ _ _ TRUE _] -> w1026
      tunnel: w1023 -> [_ _ w1054 _ _ _]
      tunnel: w1017 -> [_ _ _ _ w1064 _]
      frame "init" {
        # "Initialize - All initialization work should take place in this message, since other loops can potentially enqueue messages that execute immediately after this one."
        n841 = call-poly "Enqueue Message.vi"("error in (no error)"=w1031, "Message"="Report Main", "Message Queue"=w1028) -> ("error out"=w1032:errorcluster)  [unwired: 7 in, 1 out]
      }
      frame "Report Main" {
        n842 = call "Main Data Log.vi"("error in (no error)"=w1038, "main ref"=w1033) -> ("error out"=w1034:errorcluster)  [unwired: 9 in]
        n843 = Unbundle By Name(w1033) -> ("Main Home Screen.EXIT"=w1039:refnum<vi>)
        n844 = property on="Property Node" class="Bool (strict)"(reference=w1039) -> (reference out=w1036:refnum<vi>, error out=w1037:errorcluster, "Value"=w1035:bool)  [unwired: 1 in]
        n845 = case shown="False" w1035 {
          tunnel: [w1044 w1048] -> w1041
          tunnel: w1040 -> [w1043 w1047]
          tunnel: w1034 -> [w1042 w1046]
          frame True {
            n846 = call-poly "Enqueue Message.vi"("error in (no error)"=w1042, "Message"="Confirm Quit", "Message Queue"=w1043) -> ("error out"=w1044:errorcluster)  [unwired: 7 in, 1 out]
          }
          frame False {
            n847 = call-poly "Enqueue Message.vi"("error in (no error)"=w1046, "Message"="Report Main", "Message Queue"=w1047) -> ("error out"=w1048:errorcluster)  [unwired: 7 in, 1 out]
          }
        }
        n848 = Close Reference(reference=w1036, error in (no error)=w1037) -> ()  [unwired: 1 out]
      }
      frame "Error" {
        # "#CodeRecommended - If you ever change the name of this \"Error\" message, you'll need to update the name in the Check Loop Error.vi as well."
        # "#CodeRecommended - Consider creating a system for logging errors in some way. These errors are for notification purposes only. Handling of specific errors should be performed in the message frames that generated the error."
        # "Error - Display an error dialog. This message is sent by the \"Error Handler\" VIs at the end of other loops in this application."
        n849 = Variant To Data(error in=w1056, type=errorcluster {"status"=FALSE, "code"=0, "source"=""} ("error constant"), Variant=w1054) -> (data=w1052:errorcluster, error out=w1051:errorcluster)
        n850 = call <vilib>:"Simple Error Handler.vi"("error in (no error)"=w1052) -> ()  [unwired: 4 in, 5 out]
        n851 = Merge Errors(w1051) -> (w1050:errorcluster)
      }
      frame "Confirm Quit" {
        # "#CodeNeeded - If you want to provide an \"Are you sure\" dialog (or some other notification) before the application exits, place that code here. This message is typically sent from a Panel Close? event."
        # "Confirm Quit - Message that can confirm whether or not the user wants to exit the application."
        n852 = call-poly "Enqueue Message.vi"("Priority Message? (F)"=TRUE, "error in (no error)"=w1063, "Message"="Exit", "Message Queue"=w1059) -> ("error out"=w1060:errorcluster)  [unwired: 6 in, 1 out]
        n853 = Merge Errors(w1060) -> (w1061:errorcluster)
      }
      frame "Exit" {
        # "Stop the VI"
        # "Release the message queue reference"
        # "#CodeNeeded - Add any required cleanup code here. Note that if 'Exit' was called as a result of an error, an error dialog will be displayed. Add any custom error handling for an 'Exit' condition here as well."
        # "Exit - Exit the application."
        n854 = call "Fire User Event - Stop.vi"("User Event - Stop"=w1064) -> ("error out"=w1066:errorcluster)  [unwired: 10 in]
        n855 = Release Queue(queue=w1071, error in (no error)=w1065) -> (error out=w1068:errorcluster)  [unwired: 1 in, 2 out]
        n856 = Merge Errors(w1066, w1068) -> (w1067:errorcluster)
      }
      frame Default {
        # "'Default' case only runs if there is a message that isn't defined in any of the other cases.  Output a programming error."
        n857 = xnode ("Error Ring")("parameter 0"=w1072) -> ("error out"=w1073:errorcluster)
      }
    }
    n858 = Unbundle By Name(w1008) -> ("Environmental control.Acoustic Emission 3"=w1016:refnum<vi>)
    n859 = call "LAB-IQ Error Handler - Message Handling Loop.vi"("error in (no error)"=w1020, "Message Queue"=w1022) -> ("dup error in"=w1021:errorcluster)  [unwired: 8 in, 1 out]
    n860 = property on="Property Node" class="Bool (strict)"(reference=w1016) -> (reference out=w1014:refnum<vi>, error out=w1015:errorcluster, "Value"=w1013:bool)  [unwired: 1 in]
    n861 = Close Reference(reference=w1014, error in (no error)=w1015) -> ()  [unwired: 1 out]
    n862 = Equal?(x=w1013, y=TRUE) -> (x = y?=w1011:bool)
    n863 = Select(t=i64 30 ("Period"), s=w1011, f=i64 100) -> (s? t:f=w1007:i64)
    n864 = Wait (ms)(milliseconds to wait=w1007) -> ()  [unwired: 1 out]
  }
  n865 = timed-loop "Timed Loop" {
    shift-right: [w1100] -> _
    shift-left: w9 -> [w1101]
    tunnel: [w1094] -> w12
    tunnel: w41 -> [w1092]
    tunnel: w6 -> [w1091]
    tunnel: w10 -> [w1090]
    timing: w26 -> [_]
    timing-out: [_] -> w25
    shift-right: [w1088] -> _
    shift-left: w24 -> [w1089]
    shift-right: [w1086] -> _
    shift-left: w24 -> [w1087]
    shift-right: [w1084] -> _
    shift-left: w24 -> [w1085]
    shift-right: [w1083] -> _
    shift-left: w24 -> [w1082]
    stop <- w1099 stop-if-true
    # "Load Pid  Handling Loop"
    n866 = node-c288() -> ()  [unwired: 1 in, 1 out]
    n867 = call "Dequeue Message.vi"("error in (no error)"=w1091, "Message Queue"=w1092) -> ("error out"=w1098:errorcluster, "Message Data"=w1096:variant, "Message"=w1097:string, "dup Message Queue"=w1095:refnum<queue>)  [unwired: 6 in]
    n868 = case "Message Cases" shown="\"Load Pid Main\"" w1097 {
      selector: w1097 -> [_ _ _ _ _ w1209]
      tunnel: w1095 -> [w1108 w1137 _ w1188 w1204 _]
      tunnel: w1098 -> [w1111 w1135 w1181 w1192 w1198 _]
      tunnel: [w1112 w1138 w1175 w1190 w1200 w1210] -> w1093
      tunnel: w1101 -> [w1110 w1124 w1180 w1191 w1203 w1211]
      tunnel: [w1110 w1124 w1180 w1191 w1203 w1211] -> w1100
      tunnel: [_ _ _ _ TRUE _] -> w1099
      tunnel: w1096 -> [_ _ w1179 _ _ _]
      tunnel: w1090 -> [_ _ _ _ w1197 _]
      tunnel: w1089 -> [w1106 w1120 w1174 w1185 w1196 w1207]
      tunnel: [w1106 w1119 w1174 w1185 w1196 w1207] -> w1088
      tunnel: w1087 -> [w1107 w1118 w1173 w1184 w1195 w1208]
      tunnel: [w1107 w1117 w1173 w1184 w1195 w1208] -> w1086
      tunnel: w1085 -> [w1105 w1116 w1172 w1183 w1194 w1206]
      tunnel: [w1105 w1115 w1172 w1183 w1194 w1206] -> w1084
      tunnel: w1082 -> [_ w1114 _ _ _ _]
      tunnel: [w1104 w1113 w1171 w1182 w1193 w1205] -> w1083
      tunnel: w1082 -> [w1104 _ w1171 w1182 w1193 w1205]
      frame "init" {
        # "Initialize - All initialization work should take place in this message, since other loops can potentially enqueue messages that execute immediately after this one."
        n869 = call-poly "Enqueue Message.vi"("error in (no error)"=w1111, "Message"="Load Pid Main", "Message Queue"=w1108) -> ("error out"=w1112:errorcluster)  [unwired: 7 in, 1 out]
      }
      frame "Load Pid Main" {
        n870 = Unbundle By Name(w1124) -> ("Main Screen.Load En"=w1130:refnum<vi>)
        n871 = Unbundle By Name(w1124) -> ("PID.apply load"=w1125:refnum<vi>)
        n872 = property on="Property Node" class="Bool (strict)"(reference=w1130) -> (reference out=w1128:refnum<vi>, error out=w1129:errorcluster, "Value"=w1123:bool)  [unwired: 1 in]
        n873 = property on="Property Node" class="Bool (strict)"(reference=w1125) -> (reference out=w1127:refnum<vi>, error out=w1126:errorcluster, "Value"=w1122:bool)  [unwired: 1 in]
        n874 = Close Reference(reference=w1128, error in (no error)=w1129) -> ()  [unwired: 1 out]
        n875 = Close Reference(reference=w1127, error in (no error)=w1126) -> ()  [unwired: 1 out]
        n876 = Or(x=w1123, y=w1122) -> (x .or. y?=w1121:bool)
        n877 = case shown="True" w1121 {
          tunnel: w1135 -> [w1145 w1158]
          tunnel: [w1145 w1157] -> w1131
          tunnel: w1124 -> [_ w1156]
          tunnel: w1120 -> [w1144 w1155]
          tunnel: [w1144 w1154] -> w1119
          tunnel: w1118 -> [w1143 w1153]
          tunnel: [w1143 w1152] -> w1117
          tunnel: w1116 -> [w1140 w1149]
          tunnel: [w1140 w1148] -> w1115
          tunnel: w1114 -> [w1139 w1147]
          tunnel: [w1139 w1146] -> w1113
          frame False {
            n878 = local write "Checkbox 2"(TRUE ("Checkbox 2")) -> ()
            n879 = local write "Checkbox"(TRUE ("Checkbox")) -> ()
          }
          frame True {
            n880 = case shown="True" "Checkbox 2" {
              selector: "Checkbox 2" -> [_ w1161]
              tunnel: [FALSE ("Checkbox") "Checkbox"] -> w1151
              frame False {
              }
              frame True {
                n881 = Not(x=w1161) -> (.not. x?=w1160:bool)
                n882 = local write "Checkbox 2"(w1160) -> ()
              }
            }
            n883 = call "NEW LOAD CELL PID.vi"("filtered_load_in"=w1149, "filtered_deriv_in"=w1147, "integral_out"=w1153, "error in (no error)"=w1158, "prev_error_out"=w1155, "Checkbox"=w1151, "main ref"=w1156) -> ("error out"=w1157:errorcluster, "prev_error_out"=w1154:dbl, "integral_out"=w1152:dbl, "filtered_load_out"=w1148:dbl, "filtered_deriv_out"=w1146:dbl)
          }
        }
        n884 = Unbundle By Name(w1124) -> ("Main Home Screen.EXIT"=w1136:refnum<vi>)
        n885 = property on="Property Node" class="Bool (strict)"(reference=w1136) -> (reference out=w1133:refnum<vi>, error out=w1134:errorcluster, "Value"=w1132:bool)  [unwired: 1 in]
        n886 = case shown="False" w1132 {
          tunnel: [w1165 w1169] -> w1138
          tunnel: w1137 -> [w1164 w1168]
          tunnel: w1131 -> [w1163 w1167]
          frame True {
            n887 = call-poly "Enqueue Message.vi"("error in (no error)"=w1163, "Message"="Confirm Quit", "Message Queue"=w1164) -> ("error out"=w1165:errorcluster)  [unwired: 7 in, 1 out]
          }
          frame False {
            n888 = call-poly "Enqueue Message.vi"("error in (no error)"=w1167, "Message"="Load Pid Main", "Message Queue"=w1168) -> ("error out"=w1169:errorcluster)  [unwired: 7 in, 1 out]
          }
        }
        n889 = Close Reference(reference=w1133, error in (no error)=w1134) -> ()  [unwired: 1 out]
      }
      frame "Error" {
        # "#CodeRecommended - If you ever change the name of this \"Error\" message, you'll need to update the name in the Check Loop Error.vi as well."
        # "#CodeRecommended - Consider creating a system for logging errors in some way. These errors are for notification purposes only. Handling of specific errors should be performed in the message frames that generated the error."
        # "Error - Display an error dialog. This message is sent by the \"Error Handler\" VIs at the end of other loops in this application."
        n890 = Variant To Data(error in=w1181, type=errorcluster {"status"=FALSE, "code"=0, "source"=""} ("error constant"), Variant=w1179) -> (data=w1177:errorcluster, error out=w1176:errorcluster)
        n891 = call <vilib>:"Simple Error Handler.vi"("error in (no error)"=w1177) -> ()  [unwired: 4 in, 5 out]
        n892 = Merge Errors(w1176) -> (w1175:errorcluster)
      }
      frame "Confirm Quit" {
        # "#CodeNeeded - If you want to provide an \"Are you sure\" dialog (or some other notification) before the application exits, place that code here. This message is typically sent from a Panel Close? event."
        # "Confirm Quit - Message that can confirm whether or not the user wants to exit the application."
        n893 = call-poly "Enqueue Message.vi"("Priority Message? (F)"=TRUE, "error in (no error)"=w1192, "Message"="Exit", "Message Queue"=w1188) -> ("error out"=w1189:errorcluster)  [unwired: 6 in, 1 out]
        n894 = Merge Errors(w1189) -> (w1190:errorcluster)
      }
      frame "Exit" {
        # "Stop the VI"
        # "Release the message queue reference"
        # "#CodeNeeded - Add any required cleanup code here. Note that if 'Exit' was called as a result of an error, an error dialog will be displayed. Add any custom error handling for an 'Exit' condition here as well."
        # "Exit - Exit the application."
        n895 = call "Fire User Event - Stop.vi"("User Event - Stop"=w1197) -> ("error out"=w1199:errorcluster)  [unwired: 10 in]
        n896 = Release Queue(queue=w1204, error in (no error)=w1198) -> (error out=w1201:errorcluster)  [unwired: 1 in, 2 out]
        n897 = Merge Errors(w1199, w1201) -> (w1200:errorcluster)
      }
      frame Default {
        # "'Default' case only runs if there is a message that isn't defined in any of the other cases.  Output a programming error."
        n898 = xnode ("Error Ring")("parameter 0"=w1209) -> ("error out"=w1210:errorcluster)
      }
    }
    n899 = call "LAB-IQ Error Handler - Message Handling Loop.vi"("error in (no error)"=w1093, "Message Queue"=w1095) -> ("dup error in"=w1094:errorcluster)  [unwired: 8 in, 1 out]
    n900 = node-c288() -> ()  [unwired: 1 in, 1 out]
  }
  n901 = timed-loop {
    shift-right: [w1229] -> _
    shift-left: w9 -> [w1230]
    tunnel: [w1223] -> w5
    tunnel: w7 -> [w1221]
    tunnel: w6 -> [w1220]
    tunnel: w10 -> [w1219]
    timing: w4 -> [_]
    timing-out: [_] -> w3
    stop <- w1228 stop-if-true
    # "Acqoustic  Handling Loop"
    n902 = node-c288() -> ()  [unwired: 1 in, 1 out]
    n903 = call "Dequeue Message.vi"("error in (no error)"=w1220, "Message Queue"=w1221) -> ("error out"=w1227:errorcluster, "Message Data"=w1225:variant, "Message"=w1226:string, "dup Message Queue"=w1224:refnum<queue>)  [unwired: 6 in]
    n904 = case "Message Cases" shown="\"Acoustic Main\"" w1226 {
      selector: w1226 -> [_ _ _ _ _ w1322]
      tunnel: w1224 -> [w1243 w1258 _ w1309 w1321 _]
      tunnel: w1227 -> [w1237 w1249 w1306 w1313 w1315 _]
      tunnel: [w1245 w1259 w1300 w1311 w1317 w1323] -> w1222
      tunnel: w1230 -> [w1234 w1248 w1305 w1312 w1320 w1324]
      tunnel: [w1234 w1248 w1305 w1312 w1320 w1324] -> w1229
      tunnel: [_ _ _ _ TRUE _] -> w1228
      tunnel: w1225 -> [_ _ w1304 _ _ _]
      tunnel: w1219 -> [_ _ _ _ w1314 _]
      frame "init" {
        (unwired) dbl[] [] ("0UTPUT")
        # "Initialize - All initialization work should take place in this message, since other loops can potentially enqueue messages that execute immediately after this one."
        n905 = call "Acq Write Loop.vi"("Enum - Menu"=Write_Main_Enum."INIT", "error in (no error)"=w1237, "main ref"=w1234) -> ("error out"=w1242:errorcluster)  [unwired: 8 in]
        n906 = call <vilib>:"Clear Errors.vi"("error in (no error)"=w1242) -> ("error out"=w1241:errorcluster)  [unwired: 5 in, 1 out]
        n907 = call "Stall Data Flow.vim"("value in"=w1241, "milliseconds to wait"=u32 1000) -> ("value out"=w1240:errorcluster)  [unwired: 1 out]
        n908 = call "Acq Read Loop.vi"("Enum - Menu"=Read_Main_Enum."INIT", "error in (no error)"=w1240, "main ref"=w1234) -> ("error out"=w1238:errorcluster)  [unwired: 7 in, 1 out]
        n909 = call <vilib>:"Clear Errors.vi"("error in (no error)"=w1238) -> ("error out"=w1236:errorcluster)  [unwired: 5 in, 1 out]
        n910 = call-poly "Enqueue Message.vi"("error in (no error)"=w1236, "Message"="Acoustic Main", "Message Queue"=w1243) -> ("error out"=w1245:errorcluster)  [unwired: 7 in, 1 out]
      }
      frame "Acoustic Main" {
        n911 = Unbundle By Name(w1248) -> ("Environmental control.Acoustic Emission 3"=w1253:refnum<vi>)
        n912 = property on="Property Node" class="Bool (strict)"(reference=w1253) -> (reference out=w1251:refnum<vi>, error out=w1252:errorcluster, "Value"=w1250:bool)  [unwired: 1 in]
        n913 = Close Reference(reference=w1251, error in (no error)=w1252) -> ()  [unwired: 1 out]
        n914 = case shown="True" w1250 {
          tunnel: w1249 -> [w1260 w1287]
          tunnel: w1248 -> [_ w1264]
          tunnel: [w1260 w1279] -> w1247
          frame False {
          }
          frame True {
            n915 = call "Acq Read Loop.vi"("Enum - Menu"=Read_Main_Enum."READ", "error in (no error)"=w1287, "main ref"=w1264) -> ("error out"=w1285:errorcluster, "ERROR TEMP"=w1284:bool)  [unwired: 7 in]
            n916 = Unbundle By Name(w1264) -> ("Acquostic.Downlink Packet"=w1283:refnum<vi>)
            n917 = case shown="False" w1284 {
              tunnel: w1285 -> [w1288 w1291]
              tunnel: [w1288 w1290] -> w1280
              tunnel: w1264 -> [_ w1289]
              frame False {
              }
              frame True {
                n918 = call "Acoustic Reinitize.vi"("error in (no error)"=w1291, "Data Cluster"=w1289) -> ("error out"=w1290:errorcluster)  [unwired: 9 in]
              }
            }
            n919 = property on="Property Node" class="Clust (strict)"(reference=w1283, error in=w1280) -> (reference out=w1281:refnum<vi>, error out=w1282:errorcluster, "Value"=w1263:T7)
            n920 = Close Reference(reference=w1281, error in (no error)=w1282) -> (error out=w1279:errorcluster)
            n921 = Unbundle By Name(w1263) -> ("AE Ring-Down Counts"=w1261:u32)
            n922 = Unbundle By Name(w1263) -> ("Amplitude dB_AE"=w1262:sgl)
            n923 = Unbundle By Name(w1263) -> ("Peak Amplitude"=w1268:sgl)
            n924 = Unbundle By Name(w1263) -> ("Signal Energy"=w1275:sgl)
            n925 = Unbundle By Name(w1264) -> ("Acquostic.Signal Energy"=w1278:refnum<vi>)
            n926 = Unbundle By Name(w1264) -> ("Acquostic.Amplitude db_AE"=w1272:refnum<vi>)
            n927 = Unbundle By Name(w1264) -> ("Acquostic.Peak Amplitude"=w1271:refnum<vi>)
            n928 = Unbundle By Name(w1264) -> ("Acquostic.AE Ring-Down Counts"=w1265:refnum<vi>)
            n929 = property on="Property Node" class="WFChart (strict)"(reference=w1278, "Value"=w1275) -> (reference out=w1276:refnum<vi>, error out=w1277:errorcluster)  [unwired: 1 in]
            n930 = property on="Property Node" class="WFChart (strict)"(reference=w1272, "Value"=w1262) -> (reference out=w1274:refnum<vi>, error out=w1273:errorcluster)  [unwired: 1 in]
            n931 = property on="Property Node" class="WFChart (strict)"(reference=w1271, "Value"=w1268) -> (reference out=w1269:refnum<vi>, error out=w1270:errorcluster)  [unwired: 1 in]
            n932 = property on="Property Node" class="WFChart (strict)"(reference=w1265, "Value"=w1261) -> (reference out=w1267:refnum<vi>, error out=w1266:errorcluster)  [unwired: 1 in]
            n933 = Close Reference(reference=w1276, error in (no error)=w1277) -> ()  [unwired: 1 out]
            n934 = Close Reference(reference=w1274, error in (no error)=w1273) -> ()  [unwired: 1 out]
            n935 = Close Reference(reference=w1269, error in (no error)=w1270) -> ()  [unwired: 1 out]
            n936 = Close Reference(reference=w1267, error in (no error)=w1266) -> ()  [unwired: 1 out]
          }
        }
        n937 = Unbundle By Name(w1248) -> ("Main Home Screen.EXIT"=w1257:refnum<vi>)
        n938 = property on="Property Node" class="Bool (strict)"(reference=w1257) -> (reference out=w1255:refnum<vi>, error out=w1256:errorcluster, "Value"=w1254:bool)  [unwired: 1 in]
        n939 = call <vilib>:"Clear Errors.vi"("error in (no error)"=w1247) -> ("error out"=w1246:errorcluster)  [unwired: 5 in, 1 out]
        n940 = Close Reference(reference=w1255, error in (no error)=w1256) -> ()  [unwired: 1 out]
        n941 = case shown="False" w1254 {
          tunnel: [w1294 w1298] -> w1259
          tunnel: w1258 -> [w1293 w1297]
          tunnel: w1246 -> [w1292 w1296]
          frame True {
            n942 = call-poly "Enqueue Message.vi"("error in (no error)"=w1292, "Message"="Confirm Quit", "Message Queue"=w1293) -> ("error out"=w1294:errorcluster)  [unwired: 7 in, 1 out]
          }
          frame False {
            n943 = call-poly "Enqueue Message.vi"("error in (no error)"=w1296, "Message"="Acoustic Main", "Message Queue"=w1297) -> ("error out"=w1298:errorcluster)  [unwired: 7 in, 1 out]
          }
        }
      }
      frame "Error" {
        (unwired) dbl[] [] ("0UTPUT")
        # "#CodeRecommended - If you ever change the name of this \"Error\" message, you'll need to update the name in the Check Loop Error.vi as well."
        # "#CodeRecommended - Consider creating a system for logging errors in some way. These errors are for notification purposes only. Handling of specific errors should be performed in the message frames that generated the error."
        # "Error - Display an error dialog. This message is sent by the \"Error Handler\" VIs at the end of other loops in this application."
        n944 = Variant To Data(error in=w1306, type=errorcluster {"status"=FALSE, "code"=0, "source"=""} ("error constant"), Variant=w1304) -> (data=w1302:errorcluster, error out=w1301:errorcluster)
        n945 = call <vilib>:"Simple Error Handler.vi"("error in (no error)"=w1302) -> ()  [unwired: 4 in, 5 out]
        n946 = Merge Errors(w1301) -> (w1300:errorcluster)
      }
      frame "Confirm Quit" {
        (unwired) dbl[] [] ("0UTPUT")
        # "#CodeNeeded - If you want to provide an \"Are you sure\" dialog (or some other notification) before the application exits, place that code here. This message is typically sent from a Panel Close? event."
        # "Confirm Quit - Message that can confirm whether or not the user wants to exit the application."
        n947 = call-poly "Enqueue Message.vi"("Priority Message? (F)"=TRUE, "error in (no error)"=w1313, "Message"="Exit", "Message Queue"=w1309) -> ("error out"=w1310:errorcluster)  [unwired: 6 in, 1 out]
        n948 = Merge Errors(w1310) -> (w1311:errorcluster)
      }
      frame "Exit" {
        (unwired) dbl[] [] ("0UTPUT")
        # "Stop the VI"
        # "Release the message queue reference"
        # "#CodeNeeded - Add any required cleanup code here. Note that if 'Exit' was called as a result of an error, an error dialog will be displayed. Add any custom error handling for an 'Exit' condition here as well."
        # "Exit - Exit the application."
        n949 = call "Fire User Event - Stop.vi"("User Event - Stop"=w1314) -> ("error out"=w1316:errorcluster)  [unwired: 10 in]
        n950 = Release Queue(queue=w1321, error in (no error)=w1315) -> (error out=w1318:errorcluster)  [unwired: 1 in, 2 out]
        n951 = Merge Errors(w1316, w1318) -> (w1317:errorcluster)
      }
      frame Default {
        # "'Default' case only runs if there is a message that isn't defined in any of the other cases.  Output a programming error."
        n952 = xnode ("Error Ring")("parameter 0"=w1322) -> ("error out"=w1323:errorcluster)
      }
    }
    n953 = call "LAB-IQ Error Handler - Message Handling Loop.vi"("error in (no error)"=w1222, "Message Queue"=w1224) -> ("dup error in"=w1223:errorcluster)  [unwired: 8 in, 1 out]
    n954 = node-c288() -> ()  [unwired: 1 in, 1 out]
  }
  n955 = disable-structure "Diagram Disable Structure" shown="Disabled" {
    disable-tunnel: w48 -> [w1336 _]
    disable-tunnel: w9 -> [w1335 _]
    disable-tunnel: w10 -> [w1334 _]
    disable-tunnel: w6 -> [w1333 w1402]
    disable-tunnel: [w1332 w1402] -> w32
    frame Disabled {
      n956 = while {
        shift-right: [w1347] -> _
        shift-left: w1335 -> [w1348]
        tunnel: [w1341] -> w1332
        tunnel: w1336 -> [w1339]
        tunnel: w1333 -> [w1338]
        tunnel: w1334 -> [w1337]
        stop <- w1346 stop-if-true
        # "Temperature  Handling Loop"
        n957 = call "Dequeue Message.vi"("error in (no error)"=w1338, "Message Queue"=w1339) -> ("error out"=w1345:errorcluster, "Message Data"=w1343:variant, "Message"=w1344:string, "dup Message Queue"=w1342:refnum<queue>)  [unwired: 6 in]
        n958 = case "Message Cases" shown="\"Temperature Main\"" w1344 {
          selector: w1344 -> [_ _ _ _ _ w1392]
          tunnel: w1342 -> [w1349 w1360 _ w1379 w1391 _]
          tunnel: w1345 -> [w1352 w1357 w1376 w1383 w1385 _]
          tunnel: [w1353 w1361 w1370 w1381 w1387 w1393] -> w1340
          tunnel: w1348 -> [w1351 w1359 w1375 w1382 w1390 w1394]
          tunnel: [w1351 w1359 w1375 w1382 w1390 w1394] -> w1347
          tunnel: [_ _ _ _ TRUE _] -> w1346
          tunnel: w1343 -> [_ _ w1374 _ _ _]
          tunnel: w1337 -> [_ _ _ _ w1384 _]
          frame "init" {
            # "Initialize - All initialization work should take place in this message, since other loops can potentially enqueue messages that execute immediately after this one."
            n959 = call-poly "Enqueue Message.vi"("error in (no error)"=w1352, "Message"="Temperature Main", "Message Queue"=w1349) -> ("error out"=w1353:errorcluster)  [unwired: 7 in, 1 out]
          }
          frame "Temperature Main" {
            n960 = Unbundle By Name(w1359) -> ("Main Home Screen.EXIT"=w1358:refnum<vi>)
            n961 = property on="Property Node" class="Bool (strict)"(reference=w1358) -> (reference out=w1355:refnum<vi>, error out=w1356:errorcluster, "Value"=w1354:bool)  [unwired: 1 in]
            n962 = case shown="False" w1354 {
              tunnel: [w1364 w1368] -> w1361
              tunnel: w1360 -> [w1363 w1367]
              tunnel: w1357 -> [w1362 w1366]
              frame True {
                n963 = call-poly "Enqueue Message.vi"("error in (no error)"=w1362, "Message"="Confirm Quit", "Message Queue"=w1363) -> ("error out"=w1364:errorcluster)  [unwired: 7 in, 1 out]
              }
              frame False {
                n964 = call-poly "Enqueue Message.vi"("error in (no error)"=w1366, "Message"="Temperature Main", "Message Queue"=w1367) -> ("error out"=w1368:errorcluster)  [unwired: 7 in, 1 out]
              }
            }
            n965 = Close Reference(reference=w1355, error in (no error)=w1356) -> ()  [unwired: 1 out]
          }
          frame "Error" {
            # "#CodeRecommended - If you ever change the name of this \"Error\" message, you'll need to update the name in the Check Loop Error.vi as well."
            # "#CodeRecommended - Consider creating a system for logging errors in some way. These errors are for notification purposes only. Handling of specific errors should be performed in the message frames that generated the error."
            # "Error - Display an error dialog. This message is sent by the \"Error Handler\" VIs at the end of other loops in this application."
            n966 = Variant To Data(error in=w1376, type=errorcluster {"status"=FALSE, "code"=0, "source"=""} ("error constant"), Variant=w1374) -> (data=w1372:errorcluster, error out=w1371:errorcluster)
            n967 = call <vilib>:"Simple Error Handler.vi"("error in (no error)"=w1372) -> ()  [unwired: 4 in, 5 out]
            n968 = Merge Errors(w1371) -> (w1370:errorcluster)
          }
          frame "Confirm Quit" {
            # "#CodeNeeded - If you want to provide an \"Are you sure\" dialog (or some other notification) before the application exits, place that code here. This message is typically sent from a Panel Close? event."
            # "Confirm Quit - Message that can confirm whether or not the user wants to exit the application."
            n969 = call-poly "Enqueue Message.vi"("Priority Message? (F)"=TRUE, "error in (no error)"=w1383, "Message"="Exit", "Message Queue"=w1379) -> ("error out"=w1380:errorcluster)  [unwired: 6 in, 1 out]
            n970 = Merge Errors(w1380) -> (w1381:errorcluster)
          }
          frame "Exit" {
            # "Stop the VI"
            # "Release the message queue reference"
            # "#CodeNeeded - Add any required cleanup code here. Note that if 'Exit' was called as a result of an error, an error dialog will be displayed. Add any custom error handling for an 'Exit' condition here as well."
            # "Exit - Exit the application."
            n971 = call "Fire User Event - Stop.vi"("User Event - Stop"=w1384) -> ("error out"=w1386:errorcluster)  [unwired: 10 in]
            n972 = Release Queue(queue=w1391, error in (no error)=w1385) -> (error out=w1388:errorcluster)  [unwired: 1 in, 2 out]
            n973 = Merge Errors(w1386, w1388) -> (w1387:errorcluster)
          }
          frame Default {
            # "'Default' case only runs if there is a message that isn't defined in any of the other cases.  Output a programming error."
            n974 = xnode ("Error Ring")("parameter 0"=w1392) -> ("error out"=w1393:errorcluster)
          }
        }
        n975 = call "LAB-IQ Error Handler - Message Handling Loop.vi"("error in (no error)"=w1340, "Message Queue"=w1342) -> ("dup error in"=w1341:errorcluster)  [unwired: 8 in, 1 out]
      }
    }
    frame Enabled {
    }
  }
  n976 = while {
    tunnel: w78 -> [w1410]
    shift-right: [w1408] -> w75
    shift-left: w72 -> [w1409]
    tunnel: [w1404] -> w73
    stop <- w1406 stop-if-true
    # "Event Handling Loop"
    n977 = event shown="[75] \"Acoustic Emission 3\": Value Change" {
      selector: w1409 -> [_ _ _ _ _ _ _ _ _ _ _ _ _ _ _ _ _ _ _ _ _ _ _ _ _ _ _ _ _ _ _ _ _ _ _ _ _ _ _ _ _ _ _ _ _ _ _ _ _ _ _ _ _ _ _ _ _ _ _ _ _ _ _ _ _ _ _ _ _ _ _ _ _ _ _ _ _ _ _]
      dyn-events: [_ _ _ _ _ _ _ _ _ _ _ _ _ _ _ _ _ _ _ _ _ _ _ _ _ _ _ _ _ _ _ _ _ _ _ _ _ _ _ _ _ _ _ _ _ _ _ _ _ _ _ _ _ _ _ _ _ _ _ _ _ _ _ _ _ _ _ _ _ _ _ _ _ _ _ _ _ _ _] -> w1408
      timeout: 100 -> [_ _ _ _ _ _ _ _ _ _ _ _ _ _ _ _ _ _ _ _ _ _ _ _ _ _ _ _ _ _ _ _ _ _ _ _ _ _ _ _ _ _ _ _ _ _ _ _ _ _ _ _ _ _ _ _ _ _ _ _ _ _ _ _ _ _ _ _ _ _ _ _ _ _ _ _ _ _ _]
      tunnel: [_ _ _ _ _ _ _ _ _ _ _ _ _ _ _ _ _ _ _ _ _ _ _ _ _ _ _ _ _ _ _ _ _ _ _ _ _ _ _ _ _ _ _ _ _ _ _ _ _ _ _ _ _ _ _ _ _ _ _ _ _ _ _ _ _ _ _ _ _ _ _ _ _ _ _ _ _ _ TRUE ("Discard?")] -> w1406
      tunnel: w1410 -> [w1415 w1421 w1424 w1429 w1434 w1439 w1444 w1449 w1454 w1459 w1464 w1469 w1474 w1479 w1484 w1489 w1494 w1499 w1504 w1509 w1514 w1519 w1524 w1529 w1534 w1539 w1544 w1549 w1554 w1559 w1564 w1569 w1574 w1579 w1584 w1589 w1594 w1599 w1604 w1609 w1614 w1619 w1624 w1629 w1634 w1639 w1644 w1649 w1654 w1659 w1664 w1669 w1674 w1679 w1684 w1689 w1694 w1699 w1704 w1709 w1714 w1719 w1724 w1729 w1734 w1739 w1744 w1749 w1754 w1759 w1764 w1769 w1774 w1779 w1784 w1789 w1792 w1797 w1799]
      tunnel: [w1414 w1420 w1422 w1427 w1432 w1437 w1442 w1447 w1452 w1457 w1462 w1467 w1472 w1477 w1482 w1487 w1492 w1497 w1502 w1507 w1512 w1517 w1522 w1527 w1532 w1537 w1542 w1547 w1552 w1557 w1562 w1567 w1572 w1577 w1582 w1587 w1592 w1597 w1602 w1607 w1612 w1617 w1622 w1627 w1632 w1637 w1642 w1647 w1652 w1657 w1662 w1667 w1672 w1677 w1682 w1687 w1692 w1697 w1702 w1707 w1712 w1717 w1722 w1727 w1732 w1737 w1742 w1747 w1752 w1757 w1762 w1767 w1772 w1777 w1782 w1787 _ w1796 _] -> w1407
      tunnel: [w1413 w1419 w1423 w1428 w1433 w1438 w1443 w1448 w1453 w1458 w1463 w1468 w1473 w1478 w1483 w1488 w1493 w1498 w1503 w1508 w1513 w1518 w1523 w1528 w1533 w1538 w1543 w1548 w1553 w1558 w1563 w1568 w1573 w1578 w1583 w1588 w1593 w1598 w1603 w1608 w1613 w1618 w1623 w1628 w1633 w1638 w1643 w1648 w1653 w1658 w1663 w1668 w1673 w1678 w1683 w1688 w1693 w1698 w1703 w1708 w1713 w1718 w1723 w1728 w1733 w1738 w1743 w1748 w1753 w1758 w1763 w1768 w1773 w1778 w1783 w1788 w1792 w1795 w1799] -> w1405
      event Panel Close? {
        n978 = event-data() -> ()  [unwired: 1 in, 1 out]
        n979 = call-poly "Enqueue Message.vi"("Priority Message? (F)"=TRUE, "Message"="Confirm Quit", "Message Queue"=w1415) -> ("error out"=w1414:errorcluster, "dup Message Queue"=w1413:refnum<queue>)  [unwired: 7 in]
        n980 = event-data ("Event Filter Node")("Discard?"=TRUE) -> ()  [unwired: 1 in, 1 out]
      }
      event Timeout {
        n981 = event-data() -> ()  [unwired: 1 in, 1 out]
        n982 = call-poly "Enqueue Message.vi"("Priority Message? (F)"=TRUE, "Message"="Timeout", "Message Queue"=w1421) -> ("error out"=w1420:errorcluster, "dup Message Queue"=w1419:refnum<queue>)  [unwired: 7 in]
      }
      event "SAVE  2": Value Change {
        n983 = event-data() -> ()  [unwired: 1 in, 1 out]
        n984 = call-poly "Enqueue Message.vi"("Priority Message? (F)"=TRUE, "Message"="Service Save", "Message Queue"=w1424) -> ("error out"=w1422:errorcluster, "dup Message Queue"=w1423:refnum<queue>)  [unwired: 7 in]
      }
      event "Home": Value Change {
        n985 = event-data() -> ()  [unwired: 1 in, 1 out]
        n986 = call-poly "Enqueue Message.vi"("Priority Message? (F)"=TRUE, "Message"="HOME", "Message Queue"=w1429) -> ("error out"=w1427:errorcluster, "dup Message Queue"=w1428:refnum<queue>)  [unwired: 7 in]
      }
      event "Platform Settings": Value Change {
        n987 = event-data() -> ()  [unwired: 1 in, 1 out]
        n988 = call-poly "Enqueue Message.vi"("Priority Message? (F)"=TRUE, "Message"="Platform Setting", "Message Queue"=w1434) -> ("error out"=w1432:errorcluster, "dup Message Queue"=w1433:refnum<queue>)  [unwired: 7 in]
      }
      event "Configure": Value Change {
        n989 = event-data() -> ()  [unwired: 1 in, 1 out]
        n990 = call-poly "Enqueue Message.vi"("Priority Message? (F)"=TRUE, "Message"="Configure", "Message Queue"=w1439) -> ("error out"=w1437:errorcluster, "dup Message Queue"=w1438:refnum<queue>)  [unwired: 7 in]
      }
      event "Analysis": Value Change {
        n991 = event-data() -> ()  [unwired: 1 in, 1 out]
        n992 = call-poly "Enqueue Message.vi"("Priority Message? (F)"=TRUE, "Message"="Analysis", "Message Queue"=w1444) -> ("error out"=w1442:errorcluster, "dup Message Queue"=w1443:refnum<queue>)  [unwired: 7 in]
      }
      event "service 2": Value Change {
        n993 = event-data() -> ()  [unwired: 1 in, 1 out]
        n994 = call-poly "Enqueue Message.vi"("Priority Message? (F)"=TRUE, "Message"="service 2", "Message Queue"=w1449) -> ("error out"=w1447:errorcluster, "dup Message Queue"=w1448:refnum<queue>)  [unwired: 7 in]
      }
      event "Auto": Value Change {
        n995 = event-data() -> ()  [unwired: 1 in, 1 out]
        n996 = call-poly "Enqueue Message.vi"("Priority Message? (F)"=TRUE, "Message"="Auto", "Message Queue"=w1454) -> ("error out"=w1452:errorcluster, "dup Message Queue"=w1453:refnum<queue>)  [unwired: 7 in]
      }
      event "Select Load Head": Value Change {
        n997 = event-data() -> ()  [unwired: 1 in, 1 out]
        n998 = call-poly "Enqueue Message.vi"("Priority Message? (F)"=TRUE, "Message"="Select Load Head", "Message Queue"=w1459) -> ("error out"=w1457:errorcluster, "dup Message Queue"=w1458:refnum<queue>)  [unwired: 7 in]
      }
      event "com 3": Value Change {
        n999 = event-data() -> ()  [unwired: 1 in, 1 out]
        n1000 = call-poly "Enqueue Message.vi"("Priority Message? (F)"=TRUE, "Message"="com 3", "Message Queue"=w1464) -> ("error out"=w1462:errorcluster, "dup Message Queue"=w1463:refnum<queue>)  [unwired: 7 in]
      }
      event "Loading Mode": Value Change {
        n1001 = event-data() -> ()  [unwired: 1 in, 1 out]
        n1002 = call-poly "Enqueue Message.vi"("Priority Message? (F)"=TRUE, "Message"="Loading Mode", "Message Queue"=w1469) -> ("error out"=w1467:errorcluster, "dup Message Queue"=w1468:refnum<queue>)  [unwired: 7 in]
      }
      event "SSP 0.3": Value Change {
        n1003 = event-data() -> ()  [unwired: 1 in, 1 out]
        n1004 = call-poly "Enqueue Message.vi"("Priority Message? (F)"=TRUE, "Message"="SSP 0.3", "Message Queue"=w1474) -> ("error out"=w1472:errorcluster, "dup Message Queue"=w1473:refnum<queue>)  [unwired: 7 in]
      }
      event "SSP 0.5": Value Change {
        n1005 = event-data() -> ()  [unwired: 1 in, 1 out]
        n1006 = call-poly "Enqueue Message.vi"("Priority Message? (F)"=TRUE, "Message"="SSP 0.5", "Message Queue"=w1479) -> ("error out"=w1477:errorcluster, "dup Message Queue"=w1478:refnum<queue>)  [unwired: 7 in]
      }
      event "SSP 0.75": Value Change {
        n1007 = event-data() -> ()  [unwired: 1 in, 1 out]
        n1008 = call-poly "Enqueue Message.vi"("Priority Message? (F)"=TRUE, "Message"="SSP 0.75", "Message Queue"=w1484) -> ("error out"=w1482:errorcluster, "dup Message Queue"=w1483:refnum<queue>)  [unwired: 7 in]
      }
      event "LHBack": Value Change {
        n1009 = event-data() -> ()  [unwired: 1 in, 1 out]
        n1010 = call-poly "Enqueue Message.vi"("Priority Message? (F)"=TRUE, "Message"="LHBack", "Message Queue"=w1489) -> ("error out"=w1487:errorcluster, "dup Message Queue"=w1488:refnum<queue>)  [unwired: 7 in]
      }
      event "LHNext": Value Change {
        n1011 = event-data() -> ()  [unwired: 1 in, 1 out]
        n1012 = call-poly "Enqueue Message.vi"("Priority Message? (F)"=TRUE, "Message"="LHNext", "Message Queue"=w1494) -> ("error out"=w1492:errorcluster, "dup Message Queue"=w1493:refnum<queue>)  [unwired: 7 in]
      }
      event "Rot Ver": Value Change {
        n1013 = event-data() -> ()  [unwired: 1 in, 1 out]
        n1014 = call-poly "Enqueue Message.vi"("Priority Message? (F)"=TRUE, "Message"="Rot Ver", "Message Queue"=w1499) -> ("error out"=w1497:errorcluster, "dup Message Queue"=w1498:refnum<queue>)  [unwired: 7 in]
      }
      event "Traction": Value Change {
        n1015 = event-data() -> ()  [unwired: 1 in, 1 out]
        n1016 = call-poly "Enqueue Message.vi"("Priority Message? (F)"=TRUE, "Message"="Traction", "Message Queue"=w1504) -> ("error out"=w1502:errorcluster, "dup Message Queue"=w1503:refnum<queue>)  [unwired: 7 in]
      }
      event "Scratch": Value Change {
        n1017 = event-data() -> ()  [unwired: 1 in, 1 out]
        n1018 = call-poly "Enqueue Message.vi"("Priority Message? (F)"=TRUE, "Message"="Scratch", "Message Queue"=w1509) -> ("error out"=w1507:errorcluster, "dup Message Queue"=w1508:refnum<queue>)  [unwired: 7 in]
      }
      event "Motion Mode:": Value Change {
        n1019 = event-data() -> ()  [unwired: 1 in, 1 out]
        n1020 = call-poly "Enqueue Message.vi"("Priority Message? (F)"=TRUE, "Message"="Motion Mode:", "Message Queue"=w1514) -> ("error out"=w1512:errorcluster, "dup Message Queue"=w1513:refnum<queue>)  [unwired: 7 in]
      }
      event "MMBack": Value Change {
        n1021 = event-data() -> ()  [unwired: 1 in, 1 out]
        n1022 = call-poly "Enqueue Message.vi"("Priority Message? (F)"=TRUE, "Message"="MMBack", "Message Queue"=w1519) -> ("error out"=w1517:errorcluster, "dup Message Queue"=w1518:refnum<queue>)  [unwired: 7 in]
      }
      event "MMNext": Value Change {
        n1023 = event-data() -> ()  [unwired: 1 in, 1 out]
        n1024 = call-poly "Enqueue Message.vi"("Priority Message? (F)"=TRUE, "Message"="MMNext", "Message Queue"=w1524) -> ("error out"=w1522:errorcluster, "dup Message Queue"=w1523:refnum<queue>)  [unwired: 7 in]
      }
      event "APBack": Value Change {
        n1025 = event-data() -> ()  [unwired: 1 in, 1 out]
        n1026 = call-poly "Enqueue Message.vi"("Priority Message? (F)"=TRUE, "Message"="APBack", "Message Queue"=w1529) -> ("error out"=w1527:errorcluster, "dup Message Queue"=w1528:refnum<queue>)  [unwired: 7 in]
      }
      event "SNext": Value Change {
        n1027 = event-data() -> ()  [unwired: 1 in, 1 out]
        n1028 = call-poly "Enqueue Message.vi"("Priority Message? (F)"=TRUE, "Message"="SNext", "Message Queue"=w1534) -> ("error out"=w1532:errorcluster, "dup Message Queue"=w1533:refnum<queue>)  [unwired: 7 in]
      }
      event "ZeroAll": Value Change {
        n1029 = event-data() -> ()  [unwired: 1 in, 1 out]
        n1030 = call-poly "Enqueue Message.vi"("Priority Message? (F)"=TRUE, "Message"="ZeroAll", "Message Queue"=w1539) -> ("error out"=w1537:errorcluster, "dup Message Queue"=w1538:refnum<queue>)  [unwired: 7 in]
      }
      event "Enable Platform": Value Change {
        n1031 = event-data() -> ()  [unwired: 1 in, 1 out]
        n1032 = call-poly "Enqueue Message.vi"("Priority Message? (F)"=TRUE, "Message"="Enable Platform", "Message Queue"=w1544) -> ("error out"=w1542:errorcluster, "dup Message Queue"=w1543:refnum<queue>)  [unwired: 7 in]
      }
      event "Heave Up main": Value Change {
        n1033 = event-data() -> ()  [unwired: 1 in, 1 out]
        n1034 = call-poly "Enqueue Message.vi"("Priority Message? (F)"=TRUE, "Message"="Heave Up main", "Message Queue"=w1549) -> ("error out"=w1547:errorcluster, "dup Message Queue"=w1548:refnum<queue>)  [unwired: 7 in]
      }
      event "Heave Up MM": Value Change {
        n1035 = event-data() -> ()  [unwired: 1 in, 1 out]
        n1036 = call-poly "Enqueue Message.vi"("Priority Message? (F)"=TRUE, "Message"="Heave Up MM", "Message Queue"=w1554) -> ("error out"=w1552:errorcluster, "dup Message Queue"=w1553:refnum<queue>)  [unwired: 7 in]
      }
      event "Heave Down Main": Value Change {
        n1037 = event-data() -> ()  [unwired: 1 in, 1 out]
        n1038 = call-poly "Enqueue Message.vi"("Priority Message? (F)"=TRUE, "Message"="Heave Down Main", "Message Queue"=w1559) -> ("error out"=w1557:errorcluster, "dup Message Queue"=w1558:refnum<queue>)  [unwired: 7 in]
      }
      event "Heave Down MM": Value Change {
        n1039 = event-data() -> ()  [unwired: 1 in, 1 out]
        n1040 = call-poly "Enqueue Message.vi"("Priority Message? (F)"=TRUE, "Message"="Heave Down MM", "Message Queue"=w1564) -> ("error out"=w1562:errorcluster, "dup Message Queue"=w1563:refnum<queue>)  [unwired: 7 in]
      }
      event "Manual Write Heave & Surge": Value Change {
        n1041 = event-data() -> ()  [unwired: 1 in, 1 out]
        n1042 = call-poly "Enqueue Message.vi"("Priority Message? (F)"=TRUE, "Message"="Manual Write Heave & Surge", "Message Queue"=w1569) -> ("error out"=w1567:errorcluster, "dup Message Queue"=w1568:refnum<queue>)  [unwired: 7 in]
      }
      event "Manual Write SWAY": Value Change {
        n1043 = event-data() -> ()  [unwired: 1 in, 1 out]
        n1044 = call-poly "Enqueue Message.vi"("Priority Message? (F)"=TRUE, "Message"="Manual Write SWAY", "Message Queue"=w1574) -> ("error out"=w1572:errorcluster, "dup Message Queue"=w1573:refnum<queue>)  [unwired: 7 in]
      }
      event "Surge Backward Main": Value Change {
        n1045 = event-data() -> ()  [unwired: 1 in, 1 out]
        n1046 = call-poly "Enqueue Message.vi"("Priority Message? (F)"=TRUE, "Message"="Surge Backward Main", "Message Queue"=w1579) -> ("error out"=w1577:errorcluster, "dup Message Queue"=w1578:refnum<queue>)  [unwired: 7 in]
      }
      event "Surge Backward MM": Value Change {
        n1047 = event-data() -> ()  [unwired: 1 in, 1 out]
        n1048 = call-poly "Enqueue Message.vi"("Priority Message? (F)"=TRUE, "Message"="Surge Backward MM", "Message Queue"=w1584) -> ("error out"=w1582:errorcluster, "dup Message Queue"=w1583:refnum<queue>)  [unwired: 7 in]
      }
      event "Surge Forward Main": Value Change {
        n1049 = event-data() -> ()  [unwired: 1 in, 1 out]
        n1050 = call-poly "Enqueue Message.vi"("Priority Message? (F)"=TRUE, "Message"="Surge Forward Main", "Message Queue"=w1589) -> ("error out"=w1587:errorcluster, "dup Message Queue"=w1588:refnum<queue>)  [unwired: 7 in]
      }
      event "Surge Forward MM": Value Change {
        n1051 = event-data() -> ()  [unwired: 1 in, 1 out]
        n1052 = call-poly "Enqueue Message.vi"("Priority Message? (F)"=TRUE, "Message"="Surge Forward MM", "Message Queue"=w1594) -> ("error out"=w1592:errorcluster, "dup Message Queue"=w1593:refnum<queue>)  [unwired: 7 in]
      }
      event "Sway Left Main": Value Change {
        n1053 = event-data() -> ()  [unwired: 1 in, 1 out]
        n1054 = call-poly "Enqueue Message.vi"("Priority Message? (F)"=TRUE, "Message"="Sway Left Main", "Message Queue"=w1599) -> ("error out"=w1597:errorcluster, "dup Message Queue"=w1598:refnum<queue>)  [unwired: 7 in]
      }
      event "Sway Left MM": Value Change {
        n1055 = event-data() -> ()  [unwired: 1 in, 1 out]
        n1056 = call-poly "Enqueue Message.vi"("Priority Message? (F)"=TRUE, "Message"="Sway Left MM", "Message Queue"=w1604) -> ("error out"=w1602:errorcluster, "dup Message Queue"=w1603:refnum<queue>)  [unwired: 7 in]
      }
      event "Sway Right MM": Value Change {
        n1057 = event-data() -> ()  [unwired: 1 in, 1 out]
        n1058 = call-poly "Enqueue Message.vi"("Priority Message? (F)"=TRUE, "Message"="Sway Right MM", "Message Queue"=w1609) -> ("error out"=w1607:errorcluster, "dup Message Queue"=w1608:refnum<queue>)  [unwired: 7 in]
      }
      event "Sway Right Main": Value Change {
        n1059 = event-data() -> ()  [unwired: 1 in, 1 out]
        n1060 = call-poly "Enqueue Message.vi"("Priority Message? (F)"=TRUE, "Message"="Sway Right Main", "Message Queue"=w1614) -> ("error out"=w1612:errorcluster, "dup Message Queue"=w1613:refnum<queue>)  [unwired: 7 in]
      }
      event "Load En": Value Change {
        n1061 = event-data() -> ()  [unwired: 1 in, 1 out]
        n1062 = call-poly "Enqueue Message.vi"("Priority Message? (F)"=TRUE, "Message"="Load En", "Message Queue"=w1619) -> ("error out"=w1617:errorcluster, "dup Message Queue"=w1618:refnum<queue>)  [unwired: 7 in]
      }
      event "apply load": Value Change {
        n1063 = event-data() -> ()  [unwired: 1 in, 1 out]
        n1064 = call-poly "Enqueue Message.vi"("Priority Message? (F)"=TRUE, "Message"="apply load", "Message Queue"=w1624) -> ("error out"=w1622:errorcluster, "dup Message Queue"=w1623:refnum<queue>)  [unwired: 7 in]
      }
      event "BACK": Value Change {
        n1065 = event-data() -> ()  [unwired: 1 in, 1 out]
        n1066 = call-poly "Enqueue Message.vi"("Priority Message? (F)"=TRUE, "Message"="BACK", "Message Queue"=w1629) -> ("error out"=w1627:errorcluster, "dup Message Queue"=w1628:refnum<queue>)  [unwired: 7 in]
      }
      event "Start Test": Value Change {
        n1067 = event-data() -> ()  [unwired: 1 in, 1 out]
        n1068 = call-poly "Enqueue Message.vi"("Priority Message? (F)"=TRUE, "Message"="Start Test", "Message Queue"=w1634) -> ("error out"=w1632:errorcluster, "dup Message Queue"=w1633:refnum<queue>)  [unwired: 7 in]
      }
      event "STOP": Value Change {
        n1069 = event-data() -> ()  [unwired: 1 in, 1 out]
        n1070 = call-poly "Enqueue Message.vi"("Priority Message? (F)"=TRUE, "Message"="STOP", "Message Queue"=w1639) -> ("error out"=w1637:errorcluster, "dup Message Queue"=w1638:refnum<queue>)  [unwired: 7 in]
      }
      event "PlaceModule": Value Change {
        n1071 = event-data() -> ()  [unwired: 1 in, 1 out]
        n1072 = call-poly "Enqueue Message.vi"("Priority Message? (F)"=TRUE, "Message"="PlaceModule", "Message Queue"=w1644) -> ("error out"=w1642:errorcluster, "dup Message Queue"=w1643:refnum<queue>)  [unwired: 7 in]
      }
      event "HomeRot", "HomeScratch", "HomeScratch": Value Change {
        n1073 = event-data() -> ()  [unwired: 1 in, 1 out]
        n1074 = call-poly "Enqueue Message.vi"("Priority Message? (F)"=TRUE, "Message"="Stage Homing", "Message Queue"=w1649) -> ("error out"=w1647:errorcluster, "dup Message Queue"=w1648:refnum<queue>)  [unwired: 7 in]
      }
      event "Clear 3": Value Change {
        n1075 = event-data() -> ()  [unwired: 1 in, 1 out]
        n1076 = call-poly "Enqueue Message.vi"("Priority Message? (F)"=TRUE, "Message"="Clear 3", "Message Queue"=w1654) -> ("error out"=w1652:errorcluster, "dup Message Queue"=w1653:refnum<queue>)  [unwired: 7 in]
      }
      event "Set WTD": Value Change {
        n1077 = event-data() -> ()  [unwired: 1 in, 1 out]
        n1078 = call-poly "Enqueue Message.vi"("Priority Message? (F)"=TRUE, "Message"="Set WTD", "Message Queue"=w1659) -> ("error out"=w1657:errorcluster, "dup Message Queue"=w1658:refnum<queue>)  [unwired: 7 in]
      }
      event "Import 2": Value Change {
        n1079 = event-data() -> ()  [unwired: 1 in, 1 out]
        n1080 = call-poly "Enqueue Message.vi"("Priority Message? (F)"=TRUE, "Message"="Import 2", "Message Queue"=w1664) -> ("error out"=w1662:errorcluster, "dup Message Queue"=w1663:refnum<queue>)  [unwired: 7 in]
      }
      event "Save 2": Value Change {
        n1081 = event-data() -> ()  [unwired: 1 in, 1 out]
        n1082 = call-poly "Enqueue Message.vi"("Priority Message? (F)"=TRUE, "Message"="Save 2", "Message Queue"=w1669) -> ("error out"=w1667:errorcluster, "dup Message Queue"=w1668:refnum<queue>)  [unwired: 7 in]
      }
      event "calculate rotary": Value Change {
        n1083 = event-data() -> ()  [unwired: 1 in, 1 out]
        n1084 = call-poly "Enqueue Message.vi"("Priority Message? (F)"=TRUE, "Message"="Calculate Rotary", "Message Queue"=w1674) -> ("error out"=w1672:errorcluster, "dup Message Queue"=w1673:refnum<queue>)  [unwired: 7 in]
      }
      event "Clear List": Value Change {
        n1085 = event-data() -> ()  [unwired: 1 in, 1 out]
        n1086 = call-poly "Enqueue Message.vi"("Priority Message? (F)"=TRUE, "Message"="Clear List", "Message Queue"=w1679) -> ("error out"=w1677:errorcluster, "dup Message Queue"=w1678:refnum<queue>)  [unwired: 7 in]
      }
      event "Add to list": Value Change {
        n1087 = event-data() -> ()  [unwired: 1 in, 1 out]
        n1088 = call-poly "Enqueue Message.vi"("Priority Message? (F)"=TRUE, "Message"="Add to list", "Message Queue"=w1684) -> ("error out"=w1682:errorcluster, "dup Message Queue"=w1683:refnum<queue>)  [unwired: 7 in]
      }
      event "ClrLog": Value Change {
        n1089 = event-data() -> ()  [unwired: 1 in, 1 out]
        n1090 = call-poly "Enqueue Message.vi"("Priority Message? (F)"=TRUE, "Message"="ClrLog", "Message Queue"=w1689) -> ("error out"=w1687:errorcluster, "dup Message Queue"=w1688:refnum<queue>)  [unwired: 7 in]
      }
      event "Disable Axis Jog Soft Limits m": Value Change {
        n1091 = event-data() -> ()  [unwired: 1 in, 1 out]
        n1092 = call-poly "Enqueue Message.vi"("Priority Message? (F)"=TRUE, "Message"="Disable Axis Jog Soft Limits", "Message Queue"=w1694) -> ("error out"=w1692:errorcluster, "dup Message Queue"=w1693:refnum<queue>)  [unwired: 7 in]
      }
      event "Home Service": Value Change {
        n1093 = event-data() -> ()  [unwired: 1 in, 1 out]
        n1094 = call-poly "Enqueue Message.vi"("Priority Message? (F)"=TRUE, "Message"="Home Service", "Message Queue"=w1699) -> ("error out"=w1697:errorcluster, "dup Message Queue"=w1698:refnum<queue>)  [unwired: 7 in]
      }
      event "Edit Gain Constants": Value Change {
        n1095 = event-data() -> ()  [unwired: 1 in, 1 out]
        n1096 = call-poly "Enqueue Message.vi"("Priority Message? (F)"=TRUE, "Message"="Edit Gain Constants", "Message Queue"=w1704) -> ("error out"=w1702:errorcluster, "dup Message Queue"=w1703:refnum<queue>)  [unwired: 7 in]
      }
      event "Advanced Setting": Value Change {
        n1097 = event-data() -> ()  [unwired: 1 in, 1 out]
        n1098 = call-poly "Enqueue Message.vi"("Priority Message? (F)"=TRUE, "Message"="Advanced Setting", "Message Queue"=w1709) -> ("error out"=w1707:errorcluster, "dup Message Queue"=w1708:refnum<queue>)  [unwired: 7 in]
      }
      event "Password": Value Change {
        n1099 = event-data() -> ()  [unwired: 1 in, 1 out]
        n1100 = call-poly "Enqueue Message.vi"("Priority Message? (F)"=TRUE, "Message"="Password", "Message Queue"=w1714) -> ("error out"=w1712:errorcluster, "dup Message Queue"=w1713:refnum<queue>)  [unwired: 7 in]
      }
      event "Service About": Value Change {
        n1101 = event-data() -> ()  [unwired: 1 in, 1 out]
        n1102 = call-poly "Enqueue Message.vi"("Priority Message? (F)"=TRUE, "Message"="Service About", "Message Queue"=w1719) -> ("error out"=w1717:errorcluster, "dup Message Queue"=w1718:refnum<queue>)  [unwired: 7 in]
      }
      event "OPEN 1": Value Change {
        n1103 = event-data() -> ()  [unwired: 1 in, 1 out]
        n1104 = call-poly "Enqueue Message.vi"("Priority Message? (F)"=TRUE, "Message"="OPEN 1", "Message Queue"=w1724) -> ("error out"=w1722:errorcluster, "dup Message Queue"=w1723:refnum<queue>)  [unwired: 7 in]
      }
      event "OPEN 2": Value Change {
        n1105 = event-data() -> ()  [unwired: 1 in, 1 out]
        n1106 = call-poly "Enqueue Message.vi"("Priority Message? (F)"=TRUE, "Message"="OPEN 2", "Message Queue"=w1729) -> ("error out"=w1727:errorcluster, "dup Message Queue"=w1728:refnum<queue>)  [unwired: 7 in]
      }
      event "OPEN 3": Value Change {
        n1107 = event-data() -> ()  [unwired: 1 in, 1 out]
        n1108 = call-poly "Enqueue Message.vi"("Priority Message? (F)"=TRUE, "Message"="OPEN 3", "Message Queue"=w1734) -> ("error out"=w1732:errorcluster, "dup Message Queue"=w1733:refnum<queue>)  [unwired: 7 in]
      }
      event "OPEN 4": Value Change {
        n1109 = event-data() -> ()  [unwired: 1 in, 1 out]
        n1110 = call-poly "Enqueue Message.vi"("Priority Message? (F)"=TRUE, "Message"="OPEN 4", "Message Queue"=w1739) -> ("error out"=w1737:errorcluster, "dup Message Queue"=w1738:refnum<queue>)  [unwired: 7 in]
      }
      event "Refresh 2": Value Change {
        n1111 = event-data() -> ()  [unwired: 1 in, 1 out]
        n1112 = call-poly "Enqueue Message.vi"("Priority Message? (F)"=TRUE, "Message"="Refresh 2", "Message Queue"=w1744) -> ("error out"=w1742:errorcluster, "dup Message Queue"=w1743:refnum<queue>)  [unwired: 7 in]
      }
      event "Analysis Home new": Value Change {
        n1113 = event-data() -> ()  [unwired: 1 in, 1 out]
        n1114 = call-poly "Enqueue Message.vi"("Priority Message? (F)"=TRUE, "Message"="Analysis Home", "Message Queue"=w1749) -> ("error out"=w1747:errorcluster, "dup Message Queue"=w1748:refnum<queue>)  [unwired: 7 in]
      }
      event "Post Analysis": Value Change {
        n1115 = event-data() -> ()  [unwired: 1 in, 1 out]
        n1116 = call-poly "Enqueue Message.vi"("Priority Message? (F)"=TRUE, "Message"="Post Analysis", "Message Queue"=w1754) -> ("error out"=w1752:errorcluster, "dup Message Queue"=w1753:refnum<queue>)  [unwired: 7 in]
      }
      event "Scratch Mode": Value Change {
        n1117 = event-data() -> ()  [unwired: 1 in, 1 out]
        n1118 = call-poly "Enqueue Message.vi"("Priority Message? (F)"=TRUE, "Message"="Scratch Mode", "Message Queue"=w1759) -> ("error out"=w1757:errorcluster, "dup Message Queue"=w1758:refnum<queue>)  [unwired: 7 in]
      }
      event "Export": Value Change {
        n1119 = event-data() -> ()  [unwired: 1 in, 1 out]
        n1120 = call-poly "Enqueue Message.vi"("Priority Message? (F)"=TRUE, "Message"="Export", "Message Queue"=w1764) -> ("error out"=w1762:errorcluster, "dup Message Queue"=w1763:refnum<queue>)  [unwired: 7 in]
      }
      event "Traction Receipe Update Details": Value Change {
        n1121 = event-data() -> ()  [unwired: 1 in, 1 out]
        n1122 = call-poly "Enqueue Message.vi"("Priority Message? (F)"=TRUE, "Message"="Traction Receipe Update Details", "Message Queue"=w1769) -> ("error out"=w1767:errorcluster, "dup Message Queue"=w1768:refnum<queue>)  [unwired: 7 in]
      }
      event "Manual Write TRACTION": Value Change {
        n1123 = event-data() -> ()  [unwired: 1 in, 1 out]
        n1124 = call-poly "Enqueue Message.vi"("Priority Message? (F)"=TRUE, "Message"="Manual Write TRACTION", "Message Queue"=w1774) -> ("error out"=w1772:errorcluster, "dup Message Queue"=w1773:refnum<queue>)  [unwired: 7 in]
      }
      event "Manual Write Acquostic": Value Change {
        n1125 = event-data() -> ()  [unwired: 1 in, 1 out]
        n1126 = call-poly "Enqueue Message.vi"("Priority Message? (F)"=TRUE, "Message"="Manual Write ACQUOSTIC", "Message Queue"=w1779) -> ("error out"=w1777:errorcluster, "dup Message Queue"=w1778:refnum<queue>)  [unwired: 7 in]
      }
      event "Report": Value Change {
        n1127 = event-data() -> ()  [unwired: 1 in, 1 out]
        n1128 = call-poly "Enqueue Message.vi"("Priority Message? (F)"=TRUE, "Message"="Report", "Message Queue"=w1784) -> ("error out"=w1782:errorcluster, "dup Message Queue"=w1783:refnum<queue>)  [unwired: 7 in]
      }
      event "Acoustic Emission 3": Value Change {
        n1129 = event-data() -> ()  [unwired: 1 in, 1 out]
        n1130 = call-poly "Enqueue Message.vi"("Priority Message? (F)"=TRUE, "Message"="Acoustic Emission 3", "Message Queue"=w1789) -> ("error out"=w1787:errorcluster, "dup Message Queue"=w1788:refnum<queue>)  [unwired: 7 in]
      }
      event Application Instance Close {
        # "#CodeRecommended - When a project closes, all VIs within that project are aborted and leave memory. However, any code placed in this event frame is guaranteed to run to completion, so add any cleanup code that absolutely must happen here."
        n1131 = event-data() -> ()  [unwired: 1 in, 1 out]
      }
      event "EXIT": Value Change {
        n1132 = event-data() -> ()  [unwired: 1 in, 1 out]
        n1133 = call-poly "Enqueue Message.vi"("Priority Message? (F)"=TRUE, "Message"="Exit", "Message Queue"=w1797) -> ("error out"=w1796:errorcluster, "dup Message Queue"=w1795:refnum<queue>)  [unwired: 7 in]
      }
      event User Event {
        # "The Message Handling Loop processed an \"Exit\" message, which fired this event to stop the Event Handling Loop."
        n1134 = event-data() -> ()  [unwired: 1 in, 1 out]
      }
    }
    n1135 = call "LAB-IQ Error Handler - Event Handling Loop.vi"("error in (no error)"=w1407, "Message Queue"=w1405) -> ("dup error in"=w1404:errorcluster)  [unwired: 8 in, 1 out]
  }
  n1136 = timed-loop "Timed Loop" {
    shift-right: [w1810] -> _
    shift-left: w9 -> [w1811]
    tunnel: [w1804] -> w47
    tunnel: w35 -> [w1802]
    tunnel: w6 -> [w1801]
    tunnel: w10 -> [w1800]
    timing: w20 -> [_]
    timing-out: [_] -> w19
    stop <- w1809 stop-if-true
    # "Heave Motor  Handling Loop"
    n1137 = node-c288() -> ()  [unwired: 1 in, 1 out]
    n1138 = call "Dequeue Message.vi"("error in (no error)"=w1801, "Message Queue"=w1802) -> ("error out"=w1808:errorcluster, "Message Data"=w1806:variant, "Message"=w1807:string, "dup Message Queue"=w1805:refnum<queue>)  [unwired: 6 in]
    n1139 = case "Message Cases" shown="\"init\"" w1807 {
      selector: w1807 -> [_ _ _ _ _ w1906]
      tunnel: w1805 -> [w1826 w1842 _ w1894 w1905 _]
      tunnel: w1808 -> [w1823 w1840 w1886 w1897 w1899 _]
      tunnel: [w1824 w1843 w1880 w1887 w1901 w1907] -> w1803
      tunnel: w1811 -> [w1815 w1828 w1885 w1890 w1904 w1908]
      tunnel: [w1815 w1828 w1885 w1890 w1904 w1908] -> w1810
      tunnel: [_ _ _ _ TRUE _] -> w1809
      tunnel: w1806 -> [_ _ w1884 _ _ _]
      tunnel: w1800 -> [_ _ _ _ w1898 _]
      frame "init" {
        # "Initialize - All initialization work should take place in this message, since other loops can potentially enqueue messages that execute immediately after this one."
        n1140 = call "HEAVE WRITE FGV.vi"("Enum - Menu"=Heave_Write_enum."INIT", "error in (no error)"=w1823, "main ref"=w1815) -> ("error out"=w1822:errorcluster)  [unwired: 8 in]
        n1141 = call <vilib>:"Clear Errors.vi"("error in (no error)"=w1822) -> ("error out"=w1817:errorcluster)  [unwired: 5 in, 1 out]
        n1142 = call "Stall Data Flow.vim"("value in"=w1817, "milliseconds to wait"=u32 1000) -> ("value out"=w1820:errorcluster)  [unwired: 1 out]
        n1143 = call "Heave Init.vi"("error in (no error)"=w1820, "main ref"=w1815) -> ("error out"=w1818:errorcluster)  [unwired: 9 in]
        n1144 = call "HEAVE READ FGV.vi"("Enum - Menu"=Heave_Right_enum."INIT", "error in (no error)"=w1818, "main ref"=w1815) -> ("error out"=w1816:errorcluster)  [unwired: 6 in, 2 out]
        n1145 = call <vilib>:"Clear Errors.vi"("error in (no error)"=w1816) -> ("error out"=w1825:errorcluster)  [unwired: 5 in, 1 out]
        n1146 = call-poly "Enqueue Message.vi"("error in (no error)"=w1825, "Message"="Heave Main", "Message Queue"=w1826) -> ("error out"=w1824:errorcluster)  [unwired: 7 in, 1 out]
      }
      frame "Heave Main" {
        n1147 = Unbundle By Name(w1828) -> ("Heave AND Surge.Read Heave Temp"=w1836:refnum<vi>)
        n1148 = property on="Property Node" class="Bool (strict)"(reference=w1836) -> (reference out=w1834:refnum<vi>, error out=w1835:errorcluster, "Value"=w1833:bool)  [unwired: 1 in]
        n1149 = Close Reference(reference=w1834, error in (no error)=w1835) -> ()  [unwired: 1 out]
        n1150 = case shown="True" w1833 {
          tunnel: w1840 -> [w1866 w1871]
          tunnel: [w1866 w1870] -> w1831
          tunnel: w1828 -> [_ w1869]
          tunnel: [FALSE ("x < y?") w1868] -> w1829
          frame False {
          }
          frame True {
            n1151 = call "HEAVE READ FGV.vi"("Enum - Menu"=Heave_Right_enum."READ", "error in (no error)"=w1871, "main ref"=w1869) -> ("error out"=w1870:errorcluster, "x < y?"=w1868:bool)  [unwired: 6 in, 1 out]
          }
        }
        n1152 = case shown="True" w1829 {
          tunnel: w1828 -> [w1846 w1853]
          frame False {
            w1844 = TRUE ("PAUSE")
            w1845 = FALSE ("Value")
            n1153 = Unbundle By Name(w1846) -> ("Platform Settings.Heave COM Status"=w1852:refnum<vi>)
            n1154 = Unbundle By Name(w1846) -> ("Main Screen.Heave COM Status"=w1847:refnum<vi>)
            n1155 = property on="Property Node" class="Bool (strict)"(reference=w1852, "Value"=w1845) -> (reference out=w1850:refnum<vi>, error out=w1851:errorcluster)  [unwired: 1 in]
            n1156 = property on="Property Node" class="Bool (strict)"(reference=w1847, "Value"=w1845) -> (reference out=w1849:refnum<vi>, error out=w1848:errorcluster)  [unwired: 1 in]
            n1157 = Close Reference(reference=w1850, error in (no error)=w1851) -> ()  [unwired: 1 out]
            n1158 = Close Reference(reference=w1849, error in (no error)=w1848) -> ()  [unwired: 1 out]
            n1159 = call "ELAPSED TIMER VI FOR Sway Loop Connection.vi"("RESET"=w1844, "PAUSE"=w1844) -> ()  [unwired: 7 in, 3 out]
          }
          frame True {
            w1856 = FALSE ("PAUSE")
            n1160 = call "ELAPSED TIMER VI FOR Sway Loop Connection.vi"("TARGET"=2.0, "RESET"=w1856, "PAUSE"=w1856) -> ("ELAPSED INDICATION"=w1854:bool)  [unwired: 6 in, 2 out]
            n1161 = case shown="True" w1854 {
              tunnel: w1853 -> [_ w1857]
              frame False {
              }
              frame True {
                w1858 = TRUE ("Value")
                n1162 = Unbundle By Name(w1857) -> ("Main Screen.Heave COM Status"=w1859:refnum<vi>)
                n1163 = Unbundle By Name(w1857) -> ("Platform Settings.Heave COM Status"=w1864:refnum<vi>)
                n1164 = property on="Property Node" class="Bool (strict)"(reference=w1859, "Value"=w1858) -> (reference out=w1861:refnum<vi>, error out=w1860:errorcluster)  [unwired: 1 in]
                n1165 = property on="Property Node" class="Bool (strict)"(reference=w1864, "Value"=w1858) -> (reference out=w1862:refnum<vi>, error out=w1863:errorcluster)  [unwired: 1 in]
                n1166 = Close Reference(reference=w1861, error in (no error)=w1860) -> ()  [unwired: 1 out]
                n1167 = Close Reference(reference=w1862, error in (no error)=w1863) -> ()  [unwired: 1 out]
              }
            }
          }
        }
        n1168 = call "Heave Reinitial.vi"("error in (no error)"=w1831, "Data Cluster"=w1828) -> ("error out"=w1830:errorcluster)  [unwired: 9 in]
        n1169 = Unbundle By Name(w1828) -> ("Main Home Screen.EXIT"=w1841:refnum<vi>)
        n1170 = property on="Property Node" class="Bool (strict)"(reference=w1841) -> (reference out=w1838:refnum<vi>, error out=w1839:errorcluster, "Value"=w1837:bool)  [unwired: 1 in]
        n1171 = call <vilib>:"Clear Errors.vi"("error in (no error)"=w1830) -> ("error out"=w1832:errorcluster)  [unwired: 5 in, 1 out]
        n1172 = Close Reference(reference=w1838, error in (no error)=w1839) -> ()  [unwired: 1 out]
        n1173 = case shown="False" w1837 {
          tunnel: [w1874 w1878] -> w1843
          tunnel: w1842 -> [w1873 w1877]
          tunnel: w1832 -> [w1872 w1876]
          frame True {
            n1174 = call-poly "Enqueue Message.vi"("error in (no error)"=w1872, "Message"="Confirm Quit", "Message Queue"=w1873) -> ("error out"=w1874:errorcluster)  [unwired: 7 in, 1 out]
          }
          frame False {
            n1175 = call-poly "Enqueue Message.vi"("error in (no error)"=w1876, "Message"="Heave Main", "Message Queue"=w1877) -> ("error out"=w1878:errorcluster)  [unwired: 7 in, 1 out]
          }
        }
      }
      frame "Error" {
        # "#CodeRecommended - If you ever change the name of this \"Error\" message, you'll need to update the name in the Check Loop Error.vi as well."
        # "#CodeRecommended - Consider creating a system for logging errors in some way. These errors are for notification purposes only. Handling of specific errors should be performed in the message frames that generated the error."
        # "Error - Display an error dialog. This message is sent by the \"Error Handler\" VIs at the end of other loops in this application."
        n1176 = Variant To Data(error in=w1886, type=errorcluster {"status"=FALSE, "code"=0, "source"=""} ("error constant"), Variant=w1884) -> (data=w1882:errorcluster, error out=w1881:errorcluster)
        n1177 = call <vilib>:"Simple Error Handler.vi"("error in (no error)"=w1882) -> ()  [unwired: 4 in, 5 out]
        n1178 = Merge Errors(w1881) -> (w1880:errorcluster)
      }
      frame "Confirm Quit" {
        # "#CodeNeeded - If you want to provide an \"Are you sure\" dialog (or some other notification) before the application exits, place that code here. This message is typically sent from a Panel Close? event."
        # "Confirm Quit - Message that can confirm whether or not the user wants to exit the application."
        n1179 = call-poly "Enqueue Message.vi"("Priority Message? (F)"=TRUE, "error in (no error)"=w1897, "Message"="Exit", "Message Queue"=w1894) -> ("error out"=w1895:errorcluster)  [unwired: 6 in, 1 out]
        n1180 = Merge Errors(w1895) -> (w1896:errorcluster)
        n1181 = call <vilib>:"Clear Errors.vi"("error in (no error)"=w1896) -> ("error out"=w1888:errorcluster)  [unwired: 5 in, 1 out]
        n1182 = call "HEAVE WRITE FGV.vi"("Enum - Menu"=Heave_Write_enum."CLOSE", "error in (no error)"=w1888, "main ref"=w1890) -> ("error out"=w1891:errorcluster)  [unwired: 8 in]
        n1183 = call <vilib>:"Clear Errors.vi"("error in (no error)"=w1891) -> ("error out"=w1887:errorcluster)  [unwired: 5 in, 1 out]
      }
      frame "Exit" {
        # "Stop the VI"
        # "Release the message queue reference"
        # "#CodeNeeded - Add any required cleanup code here. Note that if 'Exit' was called as a result of an error, an error dialog will be displayed. Add any custom error handling for an 'Exit' condition here as well."
        # "Exit - Exit the application."
        n1184 = call "Fire User Event - Stop.vi"("User Event - Stop"=w1898) -> ("error out"=w1900:errorcluster)  [unwired: 10 in]
        n1185 = Release Queue(queue=w1905, error in (no error)=w1899) -> (error out=w1902:errorcluster)  [unwired: 1 in, 2 out]
        n1186 = Merge Errors(w1900, w1902) -> (w1901:errorcluster)
      }
      frame Default {
        # "'Default' case only runs if there is a message that isn't defined in any of the other cases.  Output a programming error."
        n1187 = xnode ("Error Ring")("parameter 0"=w1906) -> ("error out"=w1907:errorcluster)
      }
    }
    n1188 = call "LAB-IQ Error Handler - Message Handling Loop.vi"("error in (no error)"=w1803, "Message Queue"=w1805) -> ("dup error in"=w1804:errorcluster)  [unwired: 8 in, 1 out]
    n1189 = node-c288() -> ()  [unwired: 1 in, 1 out]
  }
  n1190 = while {
    tunnel: w78 -> [w1919]
    shift-right: [w1926] -> _
    shift-left: w9 -> [w1927]
    tunnel: w10 -> [w1924]
    tunnel: w71 -> [w1923]
    tunnel: [w1917] -> w79
    stop <- w1925 stop-if-true
    # "Message Handling Loop"
    n1191 = call "Dequeue Message.vi"("error in (no error)"=w1923, "Message Queue"=w1919) -> ("error out"=w1922:errorcluster, "Message Data"=w1920:variant, "Message"=w1921:string, "dup Message Queue"=w1918:refnum<queue>)  [unwired: 6 in]
    n1192 = case "Message Cases" shown="\"Acoustic Emission 3\"" w1921 {
      selector: w1921 -> [_ _ _ _ _ _ _ _ _ _ _ _ _ _ _ _ _ _ _ _ _ _ _ _ _ _ _ _ _ _ _ _ _ _ _ _ _ _ _ _ _ _ _ _ _ _ _ _ _ _ _ _ _ _ _ _ _ _ _ _ _ _ _ _ _ _ _ _ _ _ _ _ _ _ _ _ _ _ _ _ w3320]
      tunnel: w1918 -> [_ w1972 _ _ _ _ _ _ _ _ _ _ _ _ _ _ _ _ _ _ _ _ _ _ _ _ _ _ _ _ _ _ _ _ _ _ _ _ _ _ _ _ _ _ _ _ _ _ _ _ _ _ _ _ _ _ _ _ _ _ _ _ _ _ _ _ _ _ _ _ _ _ _ _ _ _ _ _ w3308 w3319 _]
      tunnel: w1922 -> [w1930 w1974 w1978 w1987 w2008 w2025 w2042 w2059 w2080 w2093 w2098 w2102 w2109 w2114 w2179 w2205 w2231 w2266 w2282 w2334 w2338 w2341 w2344 w2351 w2427 w2439 w2456 w2486 w2504 w2515 w2526 w2537 w2548 w2559 w2570 w2581 w2593 w2604 w2615 w2626 w2635 w2646 w2656 w2667 w2674 w2704 w2745 w2751 w2783 w2791 w2794 w2802 w2814 w2823 w2843 w2857 w2867 w2877 w2879 w2894 w2907 w2924 w2941 w2977 w2985 w3044 w3068 w3078 w3119 w3162 w3205 w3241 w3248 w3267 w3273 w3281 w3297 w3304 w3311 w3312 _]
      tunnel: [w1929 w1941 w1983 w1988 w2003 w2020 w2037 w2054 w2075 w2085 w2096 w2100 w2107 w2118 w2175 w2201 w2227 w2267 w2283 w2298 w2337 w2340 w2343 w2350 w2421 w2438 w2457 w2473 w2506 w2517 w2528 w2539 w2550 w2561 w2572 w2583 w2594 w2605 w2616 w2627 w2637 w2647 w2657 w2668 w2673 w2703 w2724 w2756 w2764 w2790 w2793 w2801 w2808 w2818 w2836 w2856 w2867 w2877 w2885 w2893 w2906 w2923 w2940 w2976 w2984 w3044 w3068 w3075 w3116 w3159 w3202 w3242 w3248 w3261 w3271 w3280 w3295 w3298 w3310 w3315 w3321] -> w1916
      tunnel: w1927 -> [w1928 w1932 w1979 w1986 w1994 w2011 w2028 w2045 w2063 w2083 w2095 w2099 w2105 w2113 w2177 w2203 w2229 w2254 w2269 w2285 w2336 w2339 w2342 w2345 w2420 w2437 w2450 w2466 w2502 w2513 w2524 w2535 w2546 w2557 w2568 w2579 w2591 w2602 w2613 w2624 w2634 w2645 w2655 w2666 w2672 w2702 w2723 w2749 w2762 w2789 w2792 w2796 w2807 w2816 w2838 w2855 w2859 w2869 w2878 w2892 w2896 w2909 w2927 w2943 w2979 w3036 w3059 w3071 w3112 w3155 w3198 w3240 w3243 w3260 w3270 w3275 w3294 w3303 w3305 w3318 w3322]
      tunnel: [w1928 w1932 w1979 w1986 w1994 w2011 w2028 w2045 w2063 w2083 w2095 w2099 w2105 w2113 w2177 w2203 w2229 w2254 w2269 w2285 w2336 w2339 w2342 w2345 w2420 w2437 w2450 w2466 w2502 w2513 w2524 w2535 w2546 w2557 w2568 w2579 w2591 w2602 w2613 w2624 w2634 w2645 w2655 w2666 w2672 w2702 w2723 w2749 w2762 w2789 w2792 w2796 w2807 w2816 w2838 w2855 w2859 w2869 w2878 w2892 w2896 w2909 w2927 w2943 w2979 w3036 w3059 w3071 w3112 w3155 w3198 w3240 w3243 w3260 w3270 w3275 w3294 w3303 w3305 w3318 w3322] -> w1926
      tunnel: [_ _ _ _ _ _ _ _ _ _ _ _ _ _ _ _ _ _ _ _ _ _ _ _ _ _ _ _ _ _ _ _ _ _ _ _ _ _ _ _ _ _ _ _ _ _ _ _ _ _ _ _ _ _ _ _ _ _ _ _ _ _ _ _ _ _ _ _ _ _ _ _ _ _ _ _ _ _ _ TRUE _] -> w1925
      tunnel: w1920 -> [_ _ _ _ _ _ _ _ _ _ _ _ _ _ _ _ _ _ _ _ _ _ _ _ _ _ _ _ _ _ _ _ _ _ _ _ _ _ _ _ _ _ _ _ _ _ _ _ _ _ _ _ _ _ _ _ _ _ _ _ _ _ _ _ _ _ _ _ _ _ _ _ _ _ _ _ _ w3302 _ _ _]
      tunnel: w1924 -> [_ _ _ _ _ _ _ _ _ _ _ _ _ _ _ _ _ _ _ _ _ _ _ _ _ _ _ _ _ _ _ _ _ _ _ _ _ _ _ _ _ _ _ _ _ _ _ _ _ _ _ _ _ _ _ _ _ _ _ _ _ _ _ _ _ _ _ _ _ _ _ _ _ _ _ _ _ _ _ w3314 _]
      frame "Timeout" {
        n1193 = call "Time Out Loop.vi"("error in (no error)"=w1930, "Data Cluster"=w1928) -> ("error out"=w1929:errorcluster)  [unwired: 9 in]
      }
      frame "init" {
        # "Initialize - All initialization work should take place in this message, since other loops can potentially enqueue messages that execute immediately after this one."
        n1194 = call-poly "Enqueue Message.vi"("error in (no error)"=w1974, "Message"="Init Other Loop", "Message Queue"=w1972) -> ("error out"=w1975:errorcluster)  [unwired: 7 in, 1 out]
        n1195 = Unbundle By Name(w1932) -> ("Loading.SSP 0.3"=w1960:refnum<vi>)
        n1196 = Unbundle By Name(w1932) -> ("Loading.SSP 0.5"=w1957:refnum<vi>)
        n1197 = Unbundle By Name(w1932) -> ("Loading.SSP 0.75"=w1952:refnum<vi>)
        n1198 = Unbundle By Name(w1932) -> ("Loading.Communication is established"=w1947:refnum<vi>)
        n1199 = Unbundle By Name(w1932) -> ("Loading Com Port.Load Cell Temp"=w1966:refnum<vi>)
        n1200 = Unbundle By Name(w1932) -> ("Motion Module.Set WTD"=w1940:refnum<vi>)
        n1201 = call "Read Config Unitest.vi"("error in (no error)"=w1975, "main ref"=w1932) -> ("error out"=w1970:errorcluster)  [unwired: 9 in]
        n1202 = Unbundle By Name(w1932) -> ("Motion Module.Wear Track Diameter"=w1934:refnum<vi>)
        n1203 = Unbundle By Name(w1932) -> ("PID.Ramp"=w1944:refnum<vi>)
        n1204 = call "Encrypt file path creation.vi"("error in (no error)"=w1970) -> ("error out"=w1969:errorcluster, "File Path"=w1968:path)  [unwired: 9 in]
        n1205 = property on="Property Node" class="Bool (strict)"(reference=w1966, "Value"=FALSE) -> (reference out=w1964:refnum<vi>, error out=w1965:errorcluster)  [unwired: 1 in]
        n1206 = property on="Property Node" class="Bool (strict)"(reference=w1957, "Visible"=FALSE) -> (reference out=w1955:refnum<vi>, error out=w1956:errorcluster)  [unwired: 1 in]
        n1207 = property on="Property Node" class="Bool (strict)"(reference=w1960, "Visible"=FALSE) -> (reference out=w1962:refnum<vi>, error out=w1961:errorcluster)  [unwired: 1 in]
        n1208 = property on="Property Node" class="Bool (strict)"(reference=w1952, "Visible"=FALSE) -> (reference out=w1954:refnum<vi>, error out=w1953:errorcluster)  [unwired: 1 in]
        n1209 = property on="Property Node" class="Bool (strict)"(reference=w1944, "Value"=FALSE) -> (reference out=w1946:refnum<vi>, error out=w1945:errorcluster)  [unwired: 1 in]
        n1210 = property on="Property Node" class="DigNum (strict)"(reference=w1934, "Value"=0.0) -> (reference out=w1933:refnum<vi>, error out=w1935:errorcluster)  [unwired: 1 in]
        n1211 = property on="Property Node" class="Bool (strict)"(reference=w1940, "Visible"=FALSE, "DisabledEnum"=T24."Disabled and Grayed Out" ("Disabled")) -> (reference out=w1937:refnum<vi>, error out=w1939:errorcluster)  [unwired: 1 in]
        n1212 = property on="Property Node" class="Bool (strict)"(reference=w1947, "Visible"=FALSE ("Value")) -> (reference out=w1949:refnum<vi>, error out=w1948:errorcluster)  [unwired: 1 in]
        n1213 = call "DATA ENCRYPT STRING FILE WRITE.vi"("file path (dialog if empty)"=w1968, "error in (no error)"=w1969, "User Action"="System Booted", "main ref"=w1932) -> ("error out"=w1971:errorcluster)  [unwired: 5 in, 1 out]
        n1214 = Close Reference(reference=w1955, error in (no error)=w1956) -> ()  [unwired: 1 out]
        n1215 = Close Reference(reference=w1962, error in (no error)=w1961) -> ()  [unwired: 1 out]
        n1216 = Close Reference(reference=w1954, error in (no error)=w1953) -> ()  [unwired: 1 out]
        n1217 = Close Reference(reference=w1946, error in (no error)=w1945) -> ()  [unwired: 1 out]
        n1218 = Close Reference(reference=w1964, error in (no error)=w1965) -> ()  [unwired: 1 out]
        n1219 = Close Reference(reference=w1933, error in (no error)=w1935) -> ()  [unwired: 1 out]
        n1220 = Close Reference(reference=w1937, error in (no error)=w1939) -> ()  [unwired: 1 out]
        n1221 = Close Reference(reference=w1949, error in (no error)=w1948) -> ()  [unwired: 1 out]
        n1222 = call "Reinitial Parameter After Test.vi"("error in (no error)"=w1971, "main ref"=w1932) -> ("error out"=w1941:errorcluster)  [unwired: 9 in]
        n1223 = local write "HEAVE ENABLE"(FALSE ("HEAVE ENABLE")) -> ()
      }
      frame "Init Other Loop" {
        n1224 = Unbundle By Name(w1979) -> ("Loading.com 3"=w1982:refnum<vi>)
        n1225 = property on="Property Node" class="Bool (strict)"(reference=w1982, error in=w1978, "Value"=TRUE) -> (reference out=w1980:refnum<vi>, error out=w1981:errorcluster)
        n1226 = Close Reference(reference=w1980, error in (no error)=w1981) -> (error out=w1977:errorcluster)
        n1227 = call "SET LOAD PARAMETERS.vi"("error in (no error)"=w1977, "main ref"=w1979) -> ("error out"=w1983:errorcluster)  [unwired: 9 in]
      }
      frame "Service Save" {
        n1228 = call "Write Config Unitest.vi"("error in (no error)"=w1987, "main ref"=w1986) -> ("error out"=w1992:errorcluster)  [unwired: 9 in]
        n1229 = call "Stall Data Flow.vim"("value in"=w1992, "milliseconds to wait"=u32 2000) -> ("value out"=w1991:errorcluster)  [unwired: 1 out]
        n1230 = call "Read Config Unitest.vi"("error in (no error)"=w1991, "main ref"=w1986) -> ("error out"=w1989:errorcluster)  [unwired: 9 in]
        n1231 = local write "SAVE  2"(FALSE ("SAVE  2")) -> ()
        n1232 = call "DATA ENCRYPT STRING FILE WRITE.vi"("error in (no error)"=w1989, "User Action"="Service Parameter Saved", "main ref"=w1986) -> ("error out"=w1988:errorcluster)  [unwired: 6 in, 1 out]
      }
      frame "HOME" {
        n1233 = call "DATA ENCRYPT STRING FILE WRITE.vi"("error in (no error)"=w2008, "User Action"="User Pressed Home", "main ref"=w1994) -> ("error out"=w2004:errorcluster)  [unwired: 6 in, 1 out]
        n1234 = Unbundle By Name(w1994) -> ("Main Home Screen.MainPage"=w1999:refnum<vi>)
        n1235 = Unbundle By Name(w1994) -> ("Main Home Screen.Home"=w2007:refnum<vi>)
        n1236 = Unbundle By Name(w1994) -> ("Main Home Screen.GUI"=w1997:refnum<vi>)
        n1237 = property on="Property Node" class="Bool (strict)"(reference=w2007, error in=w2004, "Value"=FALSE) -> (reference out=w2005:refnum<vi>, error out=w2006:errorcluster)
        n1238 = property on="Property Node" class="TabCtl (strict)"(reference=w1999, "Value"=T9."HOME") -> (reference out=w2001:refnum<vi>, error out=w2000:errorcluster)  [unwired: 1 in]
        n1239 = property on="Property Node" class="TabCtl (strict)"(reference=w1997, "Value"=T8."Setup") -> (reference out=w1995:refnum<vi>, error out=w1996:errorcluster)  [unwired: 1 in]
        n1240 = Close Reference(reference=w2005, error in (no error)=w2006) -> (error out=w2003:errorcluster)
        n1241 = Close Reference(reference=w2001, error in (no error)=w2000) -> ()  [unwired: 1 out]
        n1242 = Close Reference(reference=w1995, error in (no error)=w1996) -> ()  [unwired: 1 out]
      }
      frame "Platform Setting" {
        n1243 = call "DATA ENCRYPT STRING FILE WRITE.vi"("error in (no error)"=w2025, "User Action"="User Pressed Platform Setting", "main ref"=w2011) -> ("error out"=w2021:errorcluster)  [unwired: 6 in, 1 out]
        n1244 = Unbundle By Name(w2011) -> ("Main Home Screen.Platform Settings"=w2024:refnum<vi>)
        n1245 = Unbundle By Name(w2011) -> ("Main Home Screen.MainPage"=w2016:refnum<vi>)
        n1246 = Unbundle By Name(w2011) -> ("Main Home Screen.GUI"=w2014:refnum<vi>)
        n1247 = property on="Property Node" class="TabCtl (strict)"(reference=w2016, "Value"=T9."PlatformSetting") -> (reference out=w2018:refnum<vi>, error out=w2017:errorcluster)  [unwired: 1 in]
        n1248 = property on="Property Node" class="TabCtl (strict)"(reference=w2014, "Value"=T8."Setup") -> (reference out=w2012:refnum<vi>, error out=w2013:errorcluster)  [unwired: 1 in]
        n1249 = property on="Property Node" class="Bool (strict)"(reference=w2024, error in=w2021, "Value"=FALSE) -> (reference out=w2022:refnum<vi>, error out=w2023:errorcluster)
        n1250 = Close Reference(reference=w2018, error in (no error)=w2017) -> ()  [unwired: 1 out]
        n1251 = Close Reference(reference=w2012, error in (no error)=w2013) -> ()  [unwired: 1 out]
        n1252 = Close Reference(reference=w2022, error in (no error)=w2023) -> (error out=w2020:errorcluster)
      }
      frame "Configure" {
        n1253 = call "DATA ENCRYPT STRING FILE WRITE.vi"("error in (no error)"=w2042, "User Action"="User Pressed Configure", "main ref"=w2028) -> ("error out"=w2038:errorcluster)  [unwired: 6 in, 1 out]
        n1254 = Unbundle By Name(w2028) -> ("Main Home Screen.Configure"=w2041:refnum<vi>)
        n1255 = Unbundle By Name(w2028) -> ("Main Home Screen.MainPage"=w2033:refnum<vi>)
        n1256 = Unbundle By Name(w2028) -> ("Main Home Screen.GUI"=w2031:refnum<vi>)
        n1257 = property on="Property Node" class="Bool (strict)"(reference=w2041, error in=w2038, "Value"=FALSE) -> (reference out=w2039:refnum<vi>, error out=w2040:errorcluster)
        n1258 = property on="Property Node" class="TabCtl (strict)"(reference=w2033, "Value"=T9."Details") -> (reference out=w2035:refnum<vi>, error out=w2034:errorcluster)  [unwired: 1 in]
        n1259 = property on="Property Node" class="TabCtl (strict)"(reference=w2031, "Value"=T8."Setup") -> (reference out=w2029:refnum<vi>, error out=w2030:errorcluster)  [unwired: 1 in]
        n1260 = Close Reference(reference=w2039, error in (no error)=w2040) -> (error out=w2037:errorcluster)
        n1261 = Close Reference(reference=w2035, error in (no error)=w2034) -> ()  [unwired: 1 out]
        n1262 = Close Reference(reference=w2029, error in (no error)=w2030) -> ()  [unwired: 1 out]
      }
      frame "Analysis" {
        n1263 = call "DATA ENCRYPT STRING FILE WRITE.vi"("error in (no error)"=w2059, "User Action"="User Pressed Analysis", "main ref"=w2045) -> ("error out"=w2055:errorcluster)  [unwired: 6 in, 1 out]
        n1264 = Unbundle By Name(w2045) -> ("Main Home Screen.MainPage"=w2050:refnum<vi>)
        n1265 = Unbundle By Name(w2045) -> ("Main Home Screen.Analysis"=w2058:refnum<vi>)
        n1266 = Unbundle By Name(w2045) -> ("Main Home Screen.GUI"=w2048:refnum<vi>)
        n1267 = property on="Property Node" class="Bool (strict)"(reference=w2058, error in=w2055, "Value"=FALSE) -> (reference out=w2056:refnum<vi>, error out=w2057:errorcluster)
        n1268 = property on="Property Node" class="TabCtl (strict)"(reference=w2050, "Value"=T9."Analysis") -> (reference out=w2052:refnum<vi>, error out=w2051:errorcluster)  [unwired: 1 in]
        n1269 = property on="Property Node" class="TabCtl (strict)"(reference=w2048, "Value"=T8."Setup") -> (reference out=w2046:refnum<vi>, error out=w2047:errorcluster)  [unwired: 1 in]
        n1270 = Close Reference(reference=w2056, error in (no error)=w2057) -> (error out=w2054:errorcluster)
        n1271 = Close Reference(reference=w2052, error in (no error)=w2051) -> ()  [unwired: 1 out]
        n1272 = Close Reference(reference=w2046, error in (no error)=w2047) -> ()  [unwired: 1 out]
      }
      frame "service 2" {
        n1273 = call "DATA ENCRYPT STRING FILE WRITE.vi"("error in (no error)"=w2080, "User Action"="User Pressed service", "main ref"=w2063) -> ("error out"=w2076:errorcluster)  [unwired: 6 in, 1 out]
        n1274 = Unbundle By Name(w2063) -> ("Main Screen.Main Screen Tab"=w2064:refnum<vi>)
        n1275 = Unbundle By Name(w2063) -> ("Main Home Screen.MainPage"=w2071:refnum<vi>)
        n1276 = Unbundle By Name(w2063) -> ("Main Home Screen.Analysis"=w2079:refnum<vi>)
        n1277 = Unbundle By Name(w2063) -> ("Main Home Screen.GUI"=w2069:refnum<vi>)
        n1278 = property on="Property Node" class="Bool (strict)"(reference=w2079, error in=w2076, "Value"=FALSE) -> (reference out=w2077:refnum<vi>, error out=w2078:errorcluster)
        n1279 = property on="Property Node" class="TabCtl (strict)"(reference=w2071, "Value"=T9."HOME") -> (reference out=w2073:refnum<vi>, error out=w2072:errorcluster)  [unwired: 1 in]
        n1280 = property on="Property Node" class="TabCtl (strict)"(reference=w2069, "Value"=T8."Begin") -> (reference out=w2067:refnum<vi>, error out=w2068:errorcluster)  [unwired: 1 in]
        n1281 = property on="Property Node" class="TabCtl (strict)"(reference=w2064, "Value"=T12."About") -> (reference out=w2061:refnum<vi>, error out=w2065:errorcluster)  [unwired: 1 in]
        n1282 = Close Reference(reference=w2077, error in (no error)=w2078) -> (error out=w2075:errorcluster)
        n1283 = Close Reference(reference=w2073, error in (no error)=w2072) -> ()  [unwired: 1 out]
        n1284 = Close Reference(reference=w2067, error in (no error)=w2068) -> ()  [unwired: 1 out]
        n1285 = Close Reference(reference=w2061, error in (no error)=w2065) -> ()  [unwired: 1 out]
      }
      frame "Auto" {
        n1286 = call "DATA ENCRYPT STRING FILE WRITE.vi"("error in (no error)"=w2093, "User Action"="User Pressed Auto File Name", "main ref"=w2083) -> ("error out"=w2090:errorcluster)  [unwired: 6 in, 1 out]
        n1287 = Get Date/Time In Seconds() -> (seconds since 1Jan1904=w2091:timestamp)
        n1288 = Format Into String(format string="%<%I_%M_%S_%p_%d_%B_%Y>T", error in=w2090, w2091) -> (resulting string=w2084:string, error out=w2086:errorcluster)  [unwired: 1 in]
        n1289 = local write "Auto"(FALSE ("Auto")) -> ()
        n1290 = Unbundle By Name(w2083) -> ("Config Screen.FILE"=w2089:refnum<vi>)
        n1291 = property on="Property Node" class="Str"(reference=w2089, error in=w2086, "Value"=w2084) -> (reference out=w2087:refnum<vi>, error out=w2088:errorcluster)
        n1292 = Close Reference(reference=w2087, error in (no error)=w2088) -> (error out=w2085:errorcluster)
      }
      frame "Select Load Head" {
        n1293 = call "Reinitial Parameter.vi"("error in (no error)"=w2098, "Data Cluster"=w2095) -> ("error out"=w2097:errorcluster)  [unwired: 9 in]
        n1294 = call "FILE NAME RECHECK.vi"("error in (no error)"=w2097, "main ref"=w2095) -> ("error out"=w2096:errorcluster)  [unwired: 9 in]
      }
      frame "com 3" {
        n1295 = call "DATA ENCRYPT STRING FILE WRITE.vi"("error in (no error)"=w2102, "User Action"="User Pressed Check Load Communication", "main ref"=w2099) -> ("error out"=w2101:errorcluster)  [unwired: 6 in, 1 out]
        n1296 = call "SET LOAD PARAMETERS.vi"("error in (no error)"=w2101, "main ref"=w2099) -> ("error out"=w2100:errorcluster)  [unwired: 9 in]
      }
      frame "ZeroAll" {
        n1297 = call "DATA ENCRYPT STRING FILE WRITE.vi"("error in (no error)"=w2109, "User Action"="User Pressed Zero All", "main ref"=w2105) -> ("error out"=w2108:errorcluster)  [unwired: 6 in, 1 out]
        n1298 = local write "ZeroAll"(FALSE ("ZeroAll")) -> ()
        n1299 = call "LOAD CELL FGV MAIN.vi"("Enum"=T25."ZEROALL", "error in (no error)"=w2108, "main ref"=w2105) -> ("error IO"=w2107:errorcluster)  [unwired: 8 in]
      }
      frame "Loading Mode" {
        n1300 = Unbundle By Name(w2113) -> ("Loading.Loading Mode"=w2115:refnum<vi>)
        n1301 = property on="Property Node" class="Ring (strict)"(reference=w2115, error in=w2114) -> (reference out=w2117:refnum<vi>, error out=w2116:errorcluster, "Value"=w2111:u16)
        n1302 = Close Reference(reference=w2117, error in (no error)=w2116) -> (error out=w2112:errorcluster)
        n1303 = case shown="1" w2111 {
          tunnel: [w2132 w2149 w2161 w2173] -> w2118
          tunnel: w2113 -> [w2119 w2135 w2153 w2165]
          tunnel: w2112 -> [w2133 w2148 w2160 w2172]
          frame 0, Default {
            n1304 = Unbundle By Name(w2119) -> ("Loading.Enter the Loading Rate (N/min)"=w2126:refnum<vi>)
            n1305 = Unbundle By Name(w2119) -> ("Loading.Load Selection"=w2129:refnum<vi>)
            n1306 = Unbundle By Name(w2119) -> ("Loading.Enter the Final Load (N)"=w2121:refnum<vi>)
            n1307 = property on="Property Node" class="TabCtl (strict)"(reference=w2129, "Value"=T10."Constant") -> (reference out=w2131:refnum<vi>, error out=w2130:errorcluster)  [unwired: 1 in]
            n1308 = property on="Property Node" class="DigNum (strict)"(reference=w2126, "DisabledEnum"=T24."Disabled and Grayed Out" ("Disabled")) -> (reference out=w2125:refnum<vi>, error out=w2127:errorcluster)  [unwired: 1 in]
            n1309 = property on="Property Node" class="DigNum (strict)"(reference=w2121, "DisabledEnum"=T24."Disabled and Grayed Out" ("Disabled")) -> (reference out=w2122:refnum<vi>, error out=w2120:errorcluster)  [unwired: 1 in]
            n1310 = call "DATA ENCRYPT STRING FILE WRITE.vi"("error in (no error)"=w2133, "User Action"="User selected Constant Mode", "main ref"=w2119) -> ("error out"=w2132:errorcluster)  [unwired: 6 in, 1 out]
            n1311 = Close Reference(reference=w2131, error in (no error)=w2130) -> ()  [unwired: 1 out]
            n1312 = Close Reference(reference=w2125, error in (no error)=w2127) -> ()  [unwired: 1 out]
            n1313 = Close Reference(reference=w2122, error in (no error)=w2120) -> ()  [unwired: 1 out]
          }
          frame 1 {
            n1314 = Unbundle By Name(w2135) -> ("Loading.Enter the Loading Rate (N/min)"=w2146:refnum<vi>)
            n1315 = Unbundle By Name(w2135) -> ("Loading.Enter the Final Load (N)"=w2141:refnum<vi>)
            n1316 = Unbundle By Name(w2135) -> ("Loading.Load Selection"=w2137:refnum<vi>)
            n1317 = property on="Property Node" class="TabCtl (strict)"(reference=w2137, "Value"=T10."Constant") -> (reference out=w2139:refnum<vi>, error out=w2138:errorcluster)  [unwired: 1 in]
            n1318 = property on="Property Node" class="DigNum (strict)"(reference=w2146, "DisabledEnum"=T24."Enabled" ("Disabled")) -> (reference out=w2145:refnum<vi>, error out=w2147:errorcluster)  [unwired: 1 in]
            n1319 = property on="Property Node" class="DigNum (strict)"(reference=w2141, "DisabledEnum"=T24."Enabled" ("Disabled")) -> (reference out=w2142:refnum<vi>, error out=w2140:errorcluster)  [unwired: 1 in]
            n1320 = call "DATA ENCRYPT STRING FILE WRITE.vi"("error in (no error)"=w2148, "User Action"="User selected Ramp Mode", "main ref"=w2135) -> ("error out"=w2149:errorcluster)  [unwired: 6 in, 1 out]
            n1321 = Close Reference(reference=w2139, error in (no error)=w2138) -> ()  [unwired: 1 out]
            n1322 = Close Reference(reference=w2145, error in (no error)=w2147) -> ()  [unwired: 1 out]
            n1323 = Close Reference(reference=w2142, error in (no error)=w2140) -> ()  [unwired: 1 out]
          }
          frame 2 {
            n1324 = Unbundle By Name(w2153) -> ("Loading.Load Selection"=w2157:refnum<vi>)
            n1325 = Unbundle By Name(w2153) -> ("Loading.Warning 2"=w2155:refnum<vi>)
            n1326 = property on="Property Node" class="TabCtl (strict)"(reference=w2157, "Value"=T10."Step") -> (reference out=w2159:refnum<vi>, error out=w2158:errorcluster)  [unwired: 1 in]
            n1327 = property on="Property Node" class="Bool (strict)"(reference=w2155, "Visible"=FALSE) -> (reference out=w2151:refnum<vi>, error out=w2154:errorcluster)  [unwired: 1 in]
            n1328 = call "DATA ENCRYPT STRING FILE WRITE.vi"("error in (no error)"=w2160, "User Action"="User selected Step Mode", "main ref"=w2153) -> ("error out"=w2161:errorcluster)  [unwired: 6 in, 1 out]
            n1329 = Close Reference(reference=w2159, error in (no error)=w2158) -> ()  [unwired: 1 out]
            n1330 = Close Reference(reference=w2151, error in (no error)=w2154) -> ()  [unwired: 1 out]
          }
          frame 3 {
            n1331 = Unbundle By Name(w2165) -> ("Loading.Load Selection"=w2169:refnum<vi>)
            n1332 = Unbundle By Name(w2165) -> ("Loading.Warning 2"=w2167:refnum<vi>)
            n1333 = property on="Property Node" class="TabCtl (strict)"(reference=w2169, "Value"=T10."Indentation") -> (reference out=w2171:refnum<vi>, error out=w2170:errorcluster)  [unwired: 1 in]
            n1334 = property on="Property Node" class="Bool (strict)"(reference=w2167, "Visible"=FALSE) -> (reference out=w2163:refnum<vi>, error out=w2166:errorcluster)  [unwired: 1 in]
            n1335 = call "DATA ENCRYPT STRING FILE WRITE.vi"("error in (no error)"=w2172, "User Action"="User selected Indentation Mode", "main ref"=w2165) -> ("error out"=w2173:errorcluster)  [unwired: 6 in, 1 out]
            n1336 = Close Reference(reference=w2171, error in (no error)=w2170) -> ()  [unwired: 1 out]
            n1337 = Close Reference(reference=w2163, error in (no error)=w2166) -> ()  [unwired: 1 out]
          }
        }
      }
      frame "SSP 0.3" {
        n1338 = Unbundle By Name(w2177) -> ("Loading.SSP 0.3"=w2180:refnum<vi>)
        n1339 = property on="Property Node" class="Bool (strict)"(reference=w2180, error in=w2179) -> (reference out=w2182:refnum<vi>, error out=w2181:errorcluster, "Value"=w2178:bool)
        n1340 = Close Reference(reference=w2182, error in (no error)=w2181) -> (error out=w2176:errorcluster)
        n1341 = case shown="True" w2178 {
          tunnel: w2177 -> [_ w2184]
          tunnel: w2176 -> [w2183 w2192]
          tunnel: [w2183 w2191] -> w2175
          frame False {
          }
          frame True {
            w2194 = FALSE ("Value")
            n1342 = Unbundle By Name(w2184) -> ("Loading.Enter the Load  (N)"=w2190:refnum<vi>)
            n1343 = Unbundle By Name(w2184) -> ("Loading.SSP 0.75"=w2195:refnum<vi>)
            n1344 = Unbundle By Name(w2184) -> ("Loading.SSP 0.5"=w2200:refnum<vi>)
            n1345 = property on="Property Node" class="Bool (strict)"(reference=w2195, "Value"=w2194) -> (reference out=w2197:refnum<vi>, error out=w2196:errorcluster)  [unwired: 1 in]
            n1346 = property on="Property Node" class="Bool (strict)"(reference=w2200, "Value"=w2194) -> (reference out=w2198:refnum<vi>, error out=w2199:errorcluster)  [unwired: 1 in]
            n1347 = property on="Property Node" class="DigNum (strict)"(reference=w2190, "Minimum"=2.0 ("Data Entry Limits:Minimum"), "Maximum"=50.0 ("Data Entry Limits:Maximum"), "Increment"=0.1 ("Data Entry Limits:Increment")) -> (reference out=w2188:refnum<vi>, error out=w2189:errorcluster)  [unwired: 1 in]
            n1348 = call "DATA ENCRYPT STRING FILE WRITE.vi"("error in (no error)"=w2192, "User Action"="User selected 0.3 SSP", "main ref"=w2184) -> ("error out"=w2191:errorcluster)  [unwired: 6 in, 1 out]
            n1349 = Close Reference(reference=w2197, error in (no error)=w2196) -> ()  [unwired: 1 out]
            n1350 = Close Reference(reference=w2198, error in (no error)=w2199) -> ()  [unwired: 1 out]
            n1351 = Close Reference(reference=w2188, error in (no error)=w2189) -> ()  [unwired: 1 out]
          }
        }
      }
      frame "SSP 0.5" {
        n1352 = Unbundle By Name(w2203) -> ("Loading.SSP 0.5"=w2206:refnum<vi>)
        n1353 = property on="Property Node" class="Bool (strict)"(reference=w2206, error in=w2205) -> (reference out=w2208:refnum<vi>, error out=w2207:errorcluster, "Value"=w2204:bool)
        n1354 = Close Reference(reference=w2208, error in (no error)=w2207) -> (error out=w2202:errorcluster)
        n1355 = case shown="True" w2204 {
          tunnel: w2203 -> [_ w2210]
          tunnel: w2202 -> [w2209 w2218]
          tunnel: [w2209 w2217] -> w2201
          frame False {
          }
          frame True {
            w2220 = FALSE ("Value")
            n1356 = Unbundle By Name(w2210) -> ("Loading.Enter the Load  (N)"=w2216:refnum<vi>)
            n1357 = Unbundle By Name(w2210) -> ("Loading.SSP 0.75"=w2226:refnum<vi>)
            n1358 = Unbundle By Name(w2210) -> ("Loading.SSP 0.3"=w2221:refnum<vi>)
            n1359 = property on="Property Node" class="Bool (strict)"(reference=w2221, "Value"=w2220) -> (reference out=w2223:refnum<vi>, error out=w2222:errorcluster)  [unwired: 1 in]
            n1360 = property on="Property Node" class="Bool (strict)"(reference=w2226, "Value"=w2220) -> (reference out=w2224:refnum<vi>, error out=w2225:errorcluster)  [unwired: 1 in]
            n1361 = property on="Property Node" class="DigNum (strict)"(reference=w2216, "Minimum"=2.0 ("Data Entry Limits:Minimum"), "Maximum"=200.0 ("Data Entry Limits:Maximum"), "Increment"=0.1 ("Data Entry Limits:Increment")) -> (reference out=w2214:refnum<vi>, error out=w2215:errorcluster)  [unwired: 1 in]
            n1362 = call "DATA ENCRYPT STRING FILE WRITE.vi"("error in (no error)"=w2218, "User Action"="User selected 0.5 SSP", "main ref"=w2210) -> ("error out"=w2217:errorcluster)  [unwired: 6 in, 1 out]
            n1363 = Close Reference(reference=w2223, error in (no error)=w2222) -> ()  [unwired: 1 out]
            n1364 = Close Reference(reference=w2224, error in (no error)=w2225) -> ()  [unwired: 1 out]
            n1365 = Close Reference(reference=w2214, error in (no error)=w2215) -> ()  [unwired: 1 out]
          }
        }
      }
      frame "SSP 0.75" {
        n1366 = Unbundle By Name(w2229) -> ("Loading.SSP 0.75"=w2232:refnum<vi>)
        n1367 = property on="Property Node" class="Bool (strict)"(reference=w2232, error in=w2231) -> (reference out=w2234:refnum<vi>, error out=w2233:errorcluster, "Value"=w2230:bool)
        n1368 = Close Reference(reference=w2234, error in (no error)=w2233) -> (error out=w2228:errorcluster)
        n1369 = case shown="True" w2230 {
          tunnel: w2229 -> [_ w2236]
          tunnel: w2228 -> [w2235 w2244]
          tunnel: [w2235 w2243] -> w2227
          frame False {
          }
          frame True {
            w2246 = FALSE ("Value")
            n1370 = Unbundle By Name(w2236) -> ("Loading.SSP 0.3"=w2247:refnum<vi>)
            n1371 = Unbundle By Name(w2236) -> ("Loading.SSP 0.5"=w2252:refnum<vi>)
            n1372 = Unbundle By Name(w2236) -> ("Loading.Enter the Load  (N)"=w2242:refnum<vi>)
            n1373 = property on="Property Node" class="Bool (strict)"(reference=w2247, "Value"=w2246) -> (reference out=w2249:refnum<vi>, error out=w2248:errorcluster)  [unwired: 1 in]
            n1374 = property on="Property Node" class="Bool (strict)"(reference=w2252, "Value"=w2246) -> (reference out=w2250:refnum<vi>, error out=w2251:errorcluster)  [unwired: 1 in]
            n1375 = property on="Property Node" class="DigNum (strict)"(reference=w2242, "Minimum"=200.0 ("Data Entry Limits:Minimum"), "Maximum"=500.0 ("Data Entry Limits:Maximum"), "Increment"=0.1 ("Data Entry Limits:Increment")) -> (reference out=w2240:refnum<vi>, error out=w2241:errorcluster)  [unwired: 1 in]
            n1376 = call "DATA ENCRYPT STRING FILE WRITE.vi"("error in (no error)"=w2244, "User Action"="User selected 0.75 SSP", "main ref"=w2236) -> ("error out"=w2243:errorcluster)  [unwired: 6 in, 1 out]
            n1377 = Close Reference(reference=w2249, error in (no error)=w2248) -> ()  [unwired: 1 out]
            n1378 = Close Reference(reference=w2250, error in (no error)=w2251) -> ()  [unwired: 1 out]
            n1379 = Close Reference(reference=w2240, error in (no error)=w2241) -> ()  [unwired: 1 out]
          }
        }
      }
      frame "LHBack" {
        # "Back to Configure"
        n1380 = Unbundle By Name(w2254) -> ("Main Home Screen.GUI"=w2263:refnum<vi>)
        n1381 = Unbundle By Name(w2254) -> ("Main Home Screen.MainPage"=w2259:refnum<vi>)
        n1382 = Unbundle By Name(w2254) -> ("Loading.LHBack"=w2257:refnum<vi>)
        n1383 = property on="Property Node" class="TabCtl (strict)"(reference=w2259, "Value"=T9."HOME") -> (reference out=w2261:refnum<vi>, error out=w2260:errorcluster)  [unwired: 1 in]
        n1384 = property on="Property Node" class="Bool (strict)"(reference=w2257, "Value"=FALSE) -> (reference out=w2255:refnum<vi>, error out=w2256:errorcluster)  [unwired: 1 in]
        n1385 = property on="Property Node" class="TabCtl (strict)"(reference=w2263, "Value"=T8."Setup") -> (reference out=w2265:refnum<vi>, error out=w2264:errorcluster)  [unwired: 1 in]
        n1386 = Close Reference(reference=w2261, error in (no error)=w2260) -> ()  [unwired: 1 out]
        n1387 = Close Reference(reference=w2255, error in (no error)=w2256) -> ()  [unwired: 1 out]
        n1388 = Close Reference(reference=w2265, error in (no error)=w2264) -> ()  [unwired: 1 out]
        n1389 = call "DATA ENCRYPT STRING FILE WRITE.vi"("error in (no error)"=w2266, "User Action"="User selected Back to Configure", "main ref"=w2254) -> ("error out"=w2267:errorcluster)  [unwired: 6 in, 1 out]
      }
      frame "MMBack" {
        # "Back to Configure"
        n1390 = Unbundle By Name(w2269) -> ("Motion Module.MMBack"=w2273:refnum<vi>)
        n1391 = Unbundle By Name(w2269) -> ("Main Home Screen.GUI"=w2279:refnum<vi>)
        n1392 = Unbundle By Name(w2269) -> ("Main Home Screen.MainPage"=w2275:refnum<vi>)
        n1393 = property on="Property Node" class="Bool (strict)"(reference=w2273, "Value"=FALSE) -> (reference out=w2271:refnum<vi>, error out=w2272:errorcluster)  [unwired: 1 in]
        n1394 = property on="Property Node" class="TabCtl (strict)"(reference=w2275, "Value"=T9."HOME") -> (reference out=w2277:refnum<vi>, error out=w2276:errorcluster)  [unwired: 1 in]
        n1395 = property on="Property Node" class="TabCtl (strict)"(reference=w2279, "Value"=T8."Load Head") -> (reference out=w2281:refnum<vi>, error out=w2280:errorcluster)  [unwired: 1 in]
        n1396 = Close Reference(reference=w2271, error in (no error)=w2272) -> ()  [unwired: 1 out]
        n1397 = Close Reference(reference=w2277, error in (no error)=w2276) -> ()  [unwired: 1 out]
        n1398 = Close Reference(reference=w2281, error in (no error)=w2280) -> ()  [unwired: 1 out]
        n1399 = call "DATA ENCRYPT STRING FILE WRITE.vi"("error in (no error)"=w2282, "User Action"="User selected Back to Load Selection", "main ref"=w2269) -> ("error out"=w2283:errorcluster)  [unwired: 6 in, 1 out]
      }
      frame "LHNext" {
        w2319 = FALSE ("Visible")
        n1400 = Unbundle By Name(w2285) -> ("Motion Module.HomeRot"=w2325:refnum<vi>)
        n1401 = Unbundle By Name(w2285) -> ("Motion Module.HomeScratch"=w2320:refnum<vi>)
        n1402 = Unbundle By Name(w2285) -> ("Motion Module.PlaceModule"=w2318:refnum<vi>)
        n1403 = Unbundle By Name(w2285) -> ("Motion Module.Motion Mode:"=w2311:refnum<vi>)
        n1404 = Unbundle By Name(w2285) -> ("Motion Module.Motion Direction:  3"=w2310:refnum<vi>)
        n1405 = Unbundle By Name(w2285) -> ("Motion Module.Wear Track Diameter (mm)"=w2304:refnum<vi>)
        n1406 = Unbundle By Name(w2285) -> ("Motion Module.Set WTD"=w2301:refnum<vi>)
        n1407 = Unbundle By Name(w2285) -> ("Motion Module.Rotary Module Selection"=w2295:refnum<vi>)
        n1408 = call "DATA ENCRYPT STRING FILE WRITE.vi"("error in (no error)"=w2334, "User Action"="User selected Select Module", "main ref"=w2285) -> ("error out"=w2298:errorcluster)  [unwired: 6 in, 1 out]
        n1409 = property on="Property Node" class="TabCtl (strict)"(reference=w2295, "Visible"=FALSE) -> (reference out=w2294:refnum<vi>, error out=w2296:errorcluster)  [unwired: 1 in]
        n1410 = property on="Property Node" class="Bool (strict)"(reference=w2325, error in=w2298, "Visible"=w2319) -> (reference out=w2323:refnum<vi>, error out=w2324:errorcluster)
        n1411 = property on="Property Node" class="Bool (strict)"(reference=w2320, error in=w2298, "Visible"=w2319) -> (reference out=w2322:refnum<vi>, error out=w2321:errorcluster)
        n1412 = property on="Property Node" class="Bool (strict)"(reference=w2318, error in=w2298, "Visible"=TRUE) -> (reference out=w2316:refnum<vi>, error out=w2317:errorcluster)
        n1413 = property on="Property Node" class="Ring (strict)"(reference=w2311, error in=w2298, "Visible"=FALSE) -> (reference out=w2313:refnum<vi>, error out=w2312:errorcluster)
        n1414 = property on="Property Node" class="Ring (strict)"(reference=w2310, error in=w2298, "Visible"=FALSE) -> (reference out=w2307:refnum<vi>, error out=w2309:errorcluster)
        n1415 = property on="Property Node" class="DigNum (strict)"(reference=w2304, "Visible"=FALSE) -> (reference out=w2303:refnum<vi>, error out=w2305:errorcluster)  [unwired: 1 in]
        n1416 = property on="Property Node" class="Bool (strict)"(reference=w2301, "Visible"=FALSE) -> (reference out=w2302:refnum<vi>, error out=w2300:errorcluster)  [unwired: 1 in]
        n1417 = Close Reference(reference=w2323, error in (no error)=w2324) -> ()  [unwired: 1 out]
        n1418 = Close Reference(reference=w2322, error in (no error)=w2321) -> ()  [unwired: 1 out]
        n1419 = Close Reference(reference=w2316, error in (no error)=w2317) -> ()  [unwired: 1 out]
        n1420 = Close Reference(reference=w2313, error in (no error)=w2312) -> ()  [unwired: 1 out]
        n1421 = Close Reference(reference=w2307, error in (no error)=w2309) -> ()  [unwired: 1 out]
        n1422 = Close Reference(reference=w2303, error in (no error)=w2305) -> ()  [unwired: 1 out]
        n1423 = Close Reference(reference=w2294, error in (no error)=w2296) -> ()  [unwired: 1 out]
        n1424 = Close Reference(reference=w2302, error in (no error)=w2300) -> ()  [unwired: 1 out]
        n1425 = Unbundle By Name(w2285) -> ("Motion Module.M3 Image"=w2293:refnum<vi>)
        n1426 = Unbundle By Name(w2285) -> ("Main Home Screen.GUI"=w2331:refnum<vi>)
        n1427 = Unbundle By Name(w2285) -> ("Main Home Screen.MainPage"=w2327:refnum<vi>)
        n1428 = Unbundle By Name(w2285) -> ("Loading.LHNext"=w2289:refnum<vi>)
        n1429 = property on="Property Node" class="TabCtl (strict)"(reference=w2293, "Value"=enum32{"Page 1", "Page 2"}."Page 2") -> (reference out=w2291:refnum<vi>, error out=w2292:errorcluster)  [unwired: 1 in]
        n1430 = property on="Property Node" class="TabCtl (strict)"(reference=w2327, "Value"=T9."HOME") -> (reference out=w2329:refnum<vi>, error out=w2328:errorcluster)  [unwired: 1 in]
        n1431 = property on="Property Node" class="TabCtl (strict)"(reference=w2331, "Value"=T8."Motion Module") -> (reference out=w2333:refnum<vi>, error out=w2332:errorcluster)  [unwired: 1 in]
        n1432 = property on="Property Node" class="Bool (strict)"(reference=w2289, "Value"=FALSE ("Visible")) -> (reference out=w2286:refnum<vi>, error out=w2288:errorcluster)  [unwired: 1 in]
        n1433 = Close Reference(reference=w2291, error in (no error)=w2292) -> ()  [unwired: 1 out]
        n1434 = Close Reference(reference=w2286, error in (no error)=w2288) -> ()  [unwired: 1 out]
        n1435 = Close Reference(reference=w2329, error in (no error)=w2328) -> ()  [unwired: 1 out]
        n1436 = Close Reference(reference=w2333, error in (no error)=w2332) -> ()  [unwired: 1 out]
      }
      frame "Rot Ver" {
        n1437 = call "Rotory Module Selection.vi"("error in (no error)"=w2338, "Data Cluster"=w2336) -> ("error out"=w2337:errorcluster)  [unwired: 9 in]
      }
      frame "Scratch" {
        n1438 = call "Scratch Module Selection.vi"("error in (no error)"=w2341, "Data Cluster"=w2339) -> ("error out"=w2340:errorcluster)  [unwired: 9 in]
      }
      frame "Traction" {
        n1439 = call "TractionModule Selection.vi"("error in (no error)"=w2344, "Data Cluster"=w2342) -> ("error out"=w2343:errorcluster)  [unwired: 9 in]
      }
      frame "Motion Mode:" {
        n1440 = Unbundle By Name(w2345) -> ("Motion Module.Motion Mode:"=w2347:refnum<vi>)
        n1441 = property on="Property Node" class="Ring (strict)"(reference=w2347) -> (reference out=w2349:refnum<vi>, error out=w2348:errorcluster, "Value"=w2346:u16)  [unwired: 1 in]
        n1442 = Close Reference(reference=w2349, error in (no error)=w2348) -> ()  [unwired: 1 out]
        n1443 = case shown="3" w2346 {
          tunnel: w2351 -> [w2368 w2385 w2402 w2419]
          tunnel: [w2367 w2384 w2401 w2418] -> w2350
          tunnel: w2345 -> [w2366 w2383 w2400 w2417]
          tunnel: w2345 -> [w2352 w2370 w2386 w2403]
          frame 0, Default {
            n1444 = Unbundle By Name(w2352) -> ("Motion Module.Rotary Module Selection"=w2362:refnum<vi>)
            n1445 = Unbundle By Name(w2352) -> ("Motion Module.Motion Direction:  3"=w2360:refnum<vi>)
            n1446 = Unbundle By Name(w2352) -> ("Main Screen.Angle (Deg)"=w2354:refnum<vi>)
            n1447 = property on="Property Node" class="TabCtl (strict)"(reference=w2362, "Value"=T11."Uniform Rotation") -> (reference out=w2364:refnum<vi>, error out=w2363:errorcluster)  [unwired: 1 in]
            n1448 = property on="Property Node" class="DigNum (strict)"(reference=w2354, "DisabledEnum"=T24."Disabled and Grayed Out" ("Disabled")) -> (reference out=w2356:refnum<vi>, error out=w2355:errorcluster)  [unwired: 1 in]
            n1449 = property on="Property Node" class="Ring (strict)"(reference=w2360, "Visible"=TRUE) -> (reference out=w2358:refnum<vi>, error out=w2359:errorcluster)  [unwired: 1 in]
            n1450 = Close Reference(reference=w2364, error in (no error)=w2363) -> ()  [unwired: 1 out]
            n1451 = Close Reference(reference=w2356, error in (no error)=w2355) -> ()  [unwired: 1 out]
            n1452 = Close Reference(reference=w2358, error in (no error)=w2359) -> ()  [unwired: 1 out]
            n1453 = call "DATA ENCRYPT STRING FILE WRITE.vi"("error in (no error)"=w2368, "User Action"="User Selected Uniform Rotation", "main ref"=w2366) -> ("error out"=w2367:errorcluster)  [unwired: 6 in, 1 out]
          }
          frame 1 {
            n1454 = Unbundle By Name(w2370) -> ("Motion Module.Rotary Module Selection"=w2379:refnum<vi>)
            n1455 = Unbundle By Name(w2370) -> ("Motion Module.Motion Direction:  3"=w2377:refnum<vi>)
            n1456 = Unbundle By Name(w2370) -> ("Main Screen.Angle (Deg)"=w2371:refnum<vi>)
            n1457 = property on="Property Node" class="TabCtl (strict)"(reference=w2379, "Value"=T11."Angular Oscillation") -> (reference out=w2381:refnum<vi>, error out=w2380:errorcluster)  [unwired: 1 in]
            n1458 = property on="Property Node" class="DigNum (strict)"(reference=w2371, "DisabledEnum"=T24."Enabled" ("Disabled")) -> (reference out=w2373:refnum<vi>, error out=w2372:errorcluster)  [unwired: 1 in]
            n1459 = property on="Property Node" class="Ring (strict)"(reference=w2377, "Visible"=FALSE) -> (reference out=w2375:refnum<vi>, error out=w2376:errorcluster)  [unwired: 1 in]
            n1460 = Close Reference(reference=w2381, error in (no error)=w2380) -> ()  [unwired: 1 out]
            n1461 = Close Reference(reference=w2375, error in (no error)=w2376) -> ()  [unwired: 1 out]
            n1462 = Close Reference(reference=w2373, error in (no error)=w2372) -> ()  [unwired: 1 out]
            n1463 = call "DATA ENCRYPT STRING FILE WRITE.vi"("error in (no error)"=w2385, "User Action"="User Selected Angular Oscillation", "main ref"=w2383) -> ("error out"=w2384:errorcluster)  [unwired: 6 in, 1 out]
          }
          frame 2 {
            n1464 = Unbundle By Name(w2386) -> ("Motion Module.Rotary Module Selection"=w2396:refnum<vi>)
            n1465 = Unbundle By Name(w2386) -> ("Motion Module.Motion Direction:  3"=w2394:refnum<vi>)
            n1466 = Unbundle By Name(w2386) -> ("Main Screen.Angle (Deg)"=w2388:refnum<vi>)
            n1467 = property on="Property Node" class="DigNum (strict)"(reference=w2388, "DisabledEnum"=T24."Disabled and Grayed Out" ("Disabled")) -> (reference out=w2390:refnum<vi>, error out=w2389:errorcluster)  [unwired: 1 in]
            n1468 = property on="Property Node" class="TabCtl (strict)"(reference=w2396, "Value"=T11."Speed Ramp") -> (reference out=w2398:refnum<vi>, error out=w2397:errorcluster)  [unwired: 1 in]
            n1469 = property on="Property Node" class="Ring (strict)"(reference=w2394, "Visible"=TRUE) -> (reference out=w2392:refnum<vi>, error out=w2393:errorcluster)  [unwired: 1 in]
            n1470 = Close Reference(reference=w2390, error in (no error)=w2389) -> ()  [unwired: 1 out]
            n1471 = Close Reference(reference=w2398, error in (no error)=w2397) -> ()  [unwired: 1 out]
            n1472 = Close Reference(reference=w2392, error in (no error)=w2393) -> ()  [unwired: 1 out]
            n1473 = call "DATA ENCRYPT STRING FILE WRITE.vi"("error in (no error)"=w2402, "User Action"="User Selected Ramp Mode", "main ref"=w2400) -> ("error out"=w2401:errorcluster)  [unwired: 6 in, 1 out]
          }
          frame 3 {
            n1474 = Unbundle By Name(w2403) -> ("Motion Module.Rotary Module Selection"=w2413:refnum<vi>)
            n1475 = Unbundle By Name(w2403) -> ("Motion Module.Motion Direction:  3"=w2411:refnum<vi>)
            n1476 = Unbundle By Name(w2403) -> ("Main Screen.Angle (Deg)"=w2405:refnum<vi>)
            n1477 = property on="Property Node" class="TabCtl (strict)"(reference=w2413, "Value"=T11."Speed Step") -> (reference out=w2415:refnum<vi>, error out=w2414:errorcluster)  [unwired: 1 in]
            n1478 = property on="Property Node" class="DigNum (strict)"(reference=w2405, "DisabledEnum"=T24."Disabled and Grayed Out" ("Disabled")) -> (reference out=w2407:refnum<vi>, error out=w2406:errorcluster)  [unwired: 1 in]
            n1479 = property on="Property Node" class="Ring (strict)"(reference=w2411, "Visible"=FALSE) -> (reference out=w2409:refnum<vi>, error out=w2410:errorcluster)  [unwired: 1 in]
            n1480 = Close Reference(reference=w2415, error in (no error)=w2414) -> ()  [unwired: 1 out]
            n1481 = Close Reference(reference=w2407, error in (no error)=w2406) -> ()  [unwired: 1 out]
            n1482 = Close Reference(reference=w2409, error in (no error)=w2410) -> ()  [unwired: 1 out]
            n1483 = call "DATA ENCRYPT STRING FILE WRITE.vi"("error in (no error)"=w2419, "User Action"="User Selected Step Mode", "main ref"=w2417) -> ("error out"=w2418:errorcluster)  [unwired: 6 in, 1 out]
          }
        }
      }
      frame "MMNext" {
        n1484 = Unbundle By Name(w2420) -> ("Motion Module.MMNext"=w2425:refnum<vi>)
        n1485 = Unbundle By Name(w2420) -> ("Motion Module.MMNext"=w2432:refnum<vi>)
        n1486 = Unbundle By Name(w2420) -> ("Main Home Screen.GUI"=w2434:refnum<vi>)
        n1487 = property on="Property Node" class="Bool (strict)"(reference=w2425, "Value"=FALSE ("Visible")) -> (reference out=w2422:refnum<vi>, error out=w2424:errorcluster)  [unwired: 1 in]
        n1488 = property on="Property Node" class="TabCtl (strict)"(reference=w2434, "Value"=T8."Environment") -> (reference out=w2436:refnum<vi>, error out=w2435:errorcluster)  [unwired: 1 in]
        n1489 = property on="Property Node" class="Bool (strict)"(reference=w2432, "Value"=FALSE) -> (reference out=w2430:refnum<vi>, error out=w2431:errorcluster)  [unwired: 1 in]
        n1490 = Close Reference(reference=w2422, error in (no error)=w2424) -> ()  [unwired: 1 out]
        n1491 = Close Reference(reference=w2430, error in (no error)=w2431) -> ()  [unwired: 1 out]
        n1492 = Close Reference(reference=w2436, error in (no error)=w2435) -> ()  [unwired: 1 out]
        n1493 = call "DATA ENCRYPT STRING FILE WRITE.vi"("error in (no error)"=w2427, "User Action"="User Selected SetUp Module", "main ref"=w2420) -> ("error out"=w2426:errorcluster)  [unwired: 6 in, 1 out]
        n1494 = call "Main Screen Tab Visible.vi"("error in (no error)"=w2426, "main ref"=w2420) -> ("error out"=w2421:errorcluster)  [unwired: 9 in]
      }
      frame "APBack" {
        n1495 = Unbundle By Name(w2437) -> ("Environmental control.APBack"=w2444:refnum<vi>)
        n1496 = Unbundle By Name(w2437) -> ("Main Home Screen.GUI"=w2446:refnum<vi>)
        n1497 = property on="Property Node" class="TabCtl (strict)"(reference=w2446, "Value"=T8."Motion Module") -> (reference out=w2448:refnum<vi>, error out=w2447:errorcluster)  [unwired: 1 in]
        n1498 = property on="Property Node" class="Bool (strict)"(reference=w2444, "Value"=FALSE) -> (reference out=w2442:refnum<vi>, error out=w2443:errorcluster)  [unwired: 1 in]
        n1499 = Close Reference(reference=w2442, error in (no error)=w2443) -> ()  [unwired: 1 out]
        n1500 = Close Reference(reference=w2448, error in (no error)=w2447) -> ()  [unwired: 1 out]
        n1501 = call "DATA ENCRYPT STRING FILE WRITE.vi"("error in (no error)"=w2439, "User Action"="User Selected Back to Module", "main ref"=w2437) -> ("error out"=w2438:errorcluster)  [unwired: 6 in, 1 out]
      }
      frame "SNext" {
        n1502 = Unbundle By Name(w2450) -> ("Environmental control.Acoustic Emission 3"=w2454:refnum<vi>)
        n1503 = property on="Property Node" class="Bool (strict)"(reference=w2454) -> (reference out=w2452:refnum<vi>, error out=w2453:errorcluster, "Value"=w2449:bool)  [unwired: 1 in]
        n1504 = Close Reference(reference=w2452, error in (no error)=w2453) -> ()  [unwired: 1 out]
        n1505 = case shown="True" w2449 {
          tunnel: w2456 -> [w2459 w2463]
          tunnel: [w2459 w2460] -> w2451
          tunnel: w2450 -> [_ w2461]
          frame False {
          }
          frame True {
            n1506 = call "Acq Gain Selection.vi"("error in (no error)"=w2463, "Data Cluster"=w2461) -> ("error out"=w2462:errorcluster)  [unwired: 9 in]
            n1507 = call <vilib>:"Clear Errors.vi"("error in (no error)"=w2462) -> ("error out"=w2460:errorcluster)  [unwired: 5 in, 1 out]
          }
        }
        n1508 = call "Init Before Main Screen.vi"("error in (no error)"=w2451, "Data Cluster"=w2450) -> ("error out"=w2455:errorcluster)  [unwired: 9 in]
        n1509 = call "DATA ENCRYPT STRING FILE WRITE.vi"("error in (no error)"=w2455, "User Action"="User Pressed Setup", "main ref"=w2450) -> ("error out"=w2457:errorcluster)  [unwired: 6 in, 1 out]
      }
      frame "Enable Platform" {
        n1510 = Unbundle By Name(w2466) -> ("Heave AND Surge.Sequence ID"=w2470:refnum<vi>)
        n1511 = Unbundle By Name(w2466) -> ("Heave AND Surge.Mode Command"=w2494:refnum<vi>)
        n1512 = Unbundle By Name(w2466) -> ("Heave AND Surge.Distance"=w2491:refnum<vi>)
        n1513 = Unbundle By Name(w2466) -> ("Heave AND Surge.SPEED"=w2488:refnum<vi>)
        n1514 = Unbundle By Name(w2466) -> ("Platform Settings.Enable Platform"=w2501:refnum<vi>)
        n1515 = property on="Property Node" class="DigNum (strict)"(reference=w2470, "Value"=u16 0) -> (reference out=w2469:refnum<vi>, error out=w2471:errorcluster)  [unwired: 1 in]
        n1516 = property on="Property Node" class="DigNum (strict)"(reference=w2491, error in=w2486, "Value"=sgl 0.0) -> (reference out=w2492:refnum<vi>, error out=w2490:errorcluster)
        n1517 = property on="Property Node" class="DigNum (strict)"(reference=w2488, error in=w2486, "Value"=sgl 0.0) -> (reference out=w2489:refnum<vi>, error out=w2487:errorcluster)
        n1518 = property on="Property Node" class="DigNum (strict)"(reference=w2494, error in=w2486, "Value"=u8 1) -> (reference out=w2493:refnum<vi>, error out=w2495:errorcluster)
        n1519 = property on="Property Node" class="Bool (strict)"(reference=w2501, "Value"=FALSE) -> (reference out=w2499:refnum<vi>, error out=w2500:errorcluster)  [unwired: 1 in]
        n1520 = Close Reference(reference=w2469, error in (no error)=w2471) -> (error out=w2468:errorcluster)
        n1521 = Close Reference(reference=w2492, error in (no error)=w2490) -> (error out=w2483:errorcluster)
        n1522 = Close Reference(reference=w2489, error in (no error)=w2487) -> (error out=w2482:errorcluster)
        n1523 = Close Reference(reference=w2493, error in (no error)=w2495) -> (error out=w2484:errorcluster)
        n1524 = Close Reference(reference=w2499, error in (no error)=w2500) -> ()  [unwired: 1 out]
        n1525 = Merge Errors(w2486, w2484, w2483, w2482, w2468) -> (w2485:errorcluster)
        n1526 = call "DATA ENCRYPT STRING FILE WRITE.vi"("error in (no error)"=w2485, "User Action"="User Pressed Enable Platform", "main ref"=w2466) -> ("error out"=w2465:errorcluster)  [unwired: 6 in, 1 out]
        n1527 = call "HEAVE WRITE FGV.vi"("Enum - Menu"=Heave_Write_enum."WRITE", "error in (no error)"=w2465, "main ref"=w2466) -> ("error out"=w2474:errorcluster)  [unwired: 8 in]
        n1528 = call "TRACTION HOME.vi"("error in (no error)"=w2465, "Data Cluster"=w2466) -> ("error out"=→"error out":errorcluster)  [unwired: 9 in]
        n1529 = Unbundle By Name(w2466) -> ("Heave AND Surge.Read Heave Temp"=w2478:refnum<vi>)
        n1530 = property on="Property Node" class="Bool (strict)"(reference=w2478, error in=w2474, "Value"=TRUE) -> (reference out=w2476:refnum<vi>, error out=w2477:errorcluster)
        n1531 = Close Reference(reference=w2476, error in (no error)=w2477) -> (error out=w2473:errorcluster)
        "HEAVE ENABLE" <- TRUE ("HEAVE ENABLE")
      }
      frame "Heave Up main" {
        n1532 = Unbundle By Name(w2502) -> ("Platform Settings.Heave Up main"=w2512:refnum<vi>)
        n1533 = call "Heave Up Main.vi"("error in (no error)"=w2504, "main ref"=w2502) -> ("error out"=w2503:errorcluster)  [unwired: 9 in]
        n1534 = property on="Property Node" class="Bool (strict)"(reference=w2512, "Value"=FALSE) -> (reference out=w2510:refnum<vi>, error out=w2511:errorcluster)  [unwired: 1 in]
        n1535 = Close Reference(reference=w2510, error in (no error)=w2511) -> ()  [unwired: 1 out]
        n1536 = call "DATA ENCRYPT STRING FILE WRITE.vi"("error in (no error)"=w2503, "User Action"="User Pressed Heave UP", "main ref"=w2502) -> ("error out"=w2507:errorcluster)  [unwired: 6 in, 1 out]
        n1537 = call "HEAVE WRITE FGV.vi"("Enum - Menu"=Heave_Write_enum."WRITE", "error in (no error)"=w2507, "main ref"=w2502) -> ("error out"=w2506:errorcluster)  [unwired: 8 in]
      }
      frame "Heave Up MM" {
        n1538 = Unbundle By Name(w2513) -> ("Motion Module.Heave Up MM"=w2523:refnum<vi>)
        n1539 = call "Heave Up Motion Module.vi"("error in (no error)"=w2515, "main ref"=w2513) -> ("error out"=w2514:errorcluster)  [unwired: 9 in]
        n1540 = property on="Property Node" class="Bool (strict)"(reference=w2523, "Value"=FALSE) -> (reference out=w2521:refnum<vi>, error out=w2522:errorcluster)  [unwired: 1 in]
        n1541 = Close Reference(reference=w2521, error in (no error)=w2522) -> ()  [unwired: 1 out]
        n1542 = call "DATA ENCRYPT STRING FILE WRITE.vi"("error in (no error)"=w2514, "User Action"="User Pressed Heave UP in Motion Module", "main ref"=w2513) -> ("error out"=w2518:errorcluster)  [unwired: 6 in, 1 out]
        n1543 = call "HEAVE WRITE FGV.vi"("Enum - Menu"=Heave_Write_enum."WRITE", "error in (no error)"=w2518, "main ref"=w2513) -> ("error out"=w2517:errorcluster)  [unwired: 8 in]
      }
      frame "Heave Down Main" {
        n1544 = call "Heave Down Main.vi"("error in (no error)"=w2526, "main ref"=w2524) -> ("error out"=w2525:errorcluster)  [unwired: 9 in]
        n1545 = Unbundle By Name(w2524) -> ("Platform Settings.Heave Down Main"=w2534:refnum<vi>)
        n1546 = property on="Property Node" class="Bool (strict)"(reference=w2534, "Value"=FALSE) -> (reference out=w2532:refnum<vi>, error out=w2533:errorcluster)  [unwired: 1 in]
        n1547 = Close Reference(reference=w2532, error in (no error)=w2533) -> ()  [unwired: 1 out]
        n1548 = call "DATA ENCRYPT STRING FILE WRITE.vi"("error in (no error)"=w2525, "User Action"="User Pressed Heave DOWN", "main ref"=w2524) -> ("error out"=w2529:errorcluster)  [unwired: 6 in, 1 out]
        n1549 = call "HEAVE WRITE FGV.vi"("Enum - Menu"=Heave_Write_enum."WRITE", "error in (no error)"=w2529, "main ref"=w2524) -> ("error out"=w2528:errorcluster)  [unwired: 8 in]
      }
      frame "Heave Down MM" {
        n1550 = call "Heave Down Motion Module.vi"("error in (no error)"=w2537, "main ref"=w2535) -> ("error out"=w2536:errorcluster)  [unwired: 9 in]
        n1551 = Unbundle By Name(w2535) -> ("Motion Module.Heave Down MM"=w2545:refnum<vi>)
        n1552 = property on="Property Node" class="Bool (strict)"(reference=w2545, "Value"=FALSE) -> (reference out=w2543:refnum<vi>, error out=w2544:errorcluster)  [unwired: 1 in]
        n1553 = Close Reference(reference=w2543, error in (no error)=w2544) -> ()  [unwired: 1 out]
        n1554 = call "DATA ENCRYPT STRING FILE WRITE.vi"("error in (no error)"=w2536, "User Action"="User Pressed Heave DOWN in Motion Module", "main ref"=w2535) -> ("error out"=w2540:errorcluster)  [unwired: 6 in, 1 out]
        n1555 = call "HEAVE WRITE FGV.vi"("Enum - Menu"=Heave_Write_enum."WRITE", "error in (no error)"=w2540, "main ref"=w2535) -> ("error out"=w2539:errorcluster)  [unwired: 8 in]
      }
      frame "Surge Backward Main" {
        n1556 = Unbundle By Name(w2546) -> ("Platform Settings.Surge Backward Main"=w2556:refnum<vi>)
        n1557 = call "Surge Backward Main.vi"("error in (no error)"=w2548, "main ref"=w2546) -> ("error out"=w2547:errorcluster)  [unwired: 9 in]
        n1558 = property on="Property Node" class="Bool (strict)"(reference=w2556, "Value"=FALSE) -> (reference out=w2554:refnum<vi>, error out=w2555:errorcluster)  [unwired: 1 in]
        n1559 = Close Reference(reference=w2554, error in (no error)=w2555) -> ()  [unwired: 1 out]
        n1560 = call "DATA ENCRYPT STRING FILE WRITE.vi"("error in (no error)"=w2547, "User Action"="User Pressed Surge Backward", "main ref"=w2546) -> ("error out"=w2551:errorcluster)  [unwired: 6 in, 1 out]
        n1561 = call "HEAVE WRITE FGV.vi"("Enum - Menu"=Heave_Write_enum."WRITE", "error in (no error)"=w2551, "main ref"=w2546) -> ("error out"=w2550:errorcluster)  [unwired: 8 in]
      }
      frame "Surge Backward MM" {
        n1562 = Unbundle By Name(w2557) -> ("Motion Module.Surge Backward MM"=w2567:refnum<vi>)
        n1563 = call "Surge Backward MM.vi"("error in (no error)"=w2559, "main ref"=w2557) -> ("error out"=w2558:errorcluster)  [unwired: 9 in]
        n1564 = property on="Property Node" class="Bool (strict)"(reference=w2567, "Value"=FALSE) -> (reference out=w2565:refnum<vi>, error out=w2566:errorcluster)  [unwired: 1 in]
        n1565 = Close Reference(reference=w2565, error in (no error)=w2566) -> ()  [unwired: 1 out]
        n1566 = call "DATA ENCRYPT STRING FILE WRITE.vi"("error in (no error)"=w2558, "User Action"="User Pressed Surge Backward in Motion Module", "main ref"=w2557) -> ("error out"=w2562:errorcluster)  [unwired: 6 in, 1 out]
        n1567 = call "HEAVE WRITE FGV.vi"("Enum - Menu"=Heave_Write_enum."WRITE", "error in (no error)"=w2562, "main ref"=w2557) -> ("error out"=w2561:errorcluster)  [unwired: 8 in]
      }
      frame "Surge Forward Main" {
        n1568 = Unbundle By Name(w2568) -> ("Platform Settings.Surge Forward Main"=w2578:refnum<vi>)
        n1569 = call "Surge Forward Main.vi"("error in (no error)"=w2570, "main ref"=w2568) -> ("error out"=w2569:errorcluster)  [unwired: 9 in]
        n1570 = property on="Property Node" class="Bool (strict)"(reference=w2578, "Value"=FALSE) -> (reference out=w2576:refnum<vi>, error out=w2577:errorcluster)  [unwired: 1 in]
        n1571 = Close Reference(reference=w2576, error in (no error)=w2577) -> ()  [unwired: 1 out]
        n1572 = call "DATA ENCRYPT STRING FILE WRITE.vi"("error in (no error)"=w2569, "User Action"="User Pressed Surge Forward", "main ref"=w2568) -> ("error out"=w2573:errorcluster)  [unwired: 6 in, 1 out]
        n1573 = call "HEAVE WRITE FGV.vi"("Enum - Menu"=Heave_Write_enum."WRITE", "error in (no error)"=w2573, "main ref"=w2568) -> ("error out"=w2572:errorcluster)  [unwired: 8 in]
      }
      frame "Surge Forward MM" {
        n1574 = Unbundle By Name(w2579) -> ("Motion Module.Surge Forward MM"=w2589:refnum<vi>)
        n1575 = call "Surge Forward MM.vi"("error in (no error)"=w2581, "main ref"=w2579) -> ("error out"=w2580:errorcluster)  [unwired: 9 in]
        n1576 = property on="Property Node" class="Bool (strict)"(reference=w2589, "Value"=FALSE) -> (reference out=w2587:refnum<vi>, error out=w2588:errorcluster)  [unwired: 1 in]
        n1577 = Close Reference(reference=w2587, error in (no error)=w2588) -> ()  [unwired: 1 out]
        n1578 = call "DATA ENCRYPT STRING FILE WRITE.vi"("error in (no error)"=w2580, "User Action"="User Pressed Surge Forward in Motion Module", "main ref"=w2579) -> ("error out"=w2584:errorcluster)  [unwired: 6 in, 1 out]
        n1579 = call "HEAVE WRITE FGV.vi"("Enum - Menu"=Heave_Write_enum."WRITE", "error in (no error)"=w2584, "main ref"=w2579) -> ("error out"=w2583:errorcluster)  [unwired: 8 in]
      }
      frame "Sway Left Main" {
        n1580 = call "Sway Left Main.vi"("error in (no error)"=w2593, "main ref"=w2591) -> ("error out"=w2592:errorcluster)  [unwired: 9 in]
        n1581 = Unbundle By Name(w2591) -> ("Platform Settings.Sway Left Main"=w2600:refnum<vi>)
        n1582 = property on="Property Node" class="Bool (strict)"(reference=w2600, "Value"=FALSE) -> (reference out=w2598:refnum<vi>, error out=w2599:errorcluster)  [unwired: 1 in]
        n1583 = Close Reference(reference=w2598, error in (no error)=w2599) -> ()  [unwired: 1 out]
        n1584 = call "DATA ENCRYPT STRING FILE WRITE.vi"("error in (no error)"=w2592, "User Action"="User Pressed Sway Left ", "main ref"=w2591) -> ("error out"=w2595:errorcluster)  [unwired: 6 in, 1 out]
        n1585 = call "SWAY WRITE FGV.vi"("Enum - Menu"=Sway_Write_enum."WRITE", "error in (no error)"=w2595, "main ref"=w2591) -> ("error out"=w2594:errorcluster)  [unwired: 8 in]
      }
      frame "Sway Left MM" {
        n1586 = call "Sway Left MM.vi"("error in (no error)"=w2604, "main ref"=w2602) -> ("error out"=w2603:errorcluster)  [unwired: 9 in]
        n1587 = Unbundle By Name(w2602) -> ("Motion Module.Sway Left MM"=w2611:refnum<vi>)
        n1588 = property on="Property Node" class="Bool (strict)"(reference=w2611, "Value"=FALSE) -> (reference out=w2609:refnum<vi>, error out=w2610:errorcluster)  [unwired: 1 in]
        n1589 = Close Reference(reference=w2609, error in (no error)=w2610) -> ()  [unwired: 1 out]
        n1590 = call "DATA ENCRYPT STRING FILE WRITE.vi"("error in (no error)"=w2603, "User Action"="User Pressed Sway Left in MM", "main ref"=w2602) -> ("error out"=w2606:errorcluster)  [unwired: 6 in, 1 out]
        n1591 = call "SWAY WRITE FGV.vi"("Enum - Menu"=Sway_Write_enum."WRITE", "error in (no error)"=w2606, "main ref"=w2602) -> ("error out"=w2605:errorcluster)  [unwired: 8 in]
      }
      frame "Sway Right MM" {
        n1592 = call "Sway Right MM.vi"("error in (no error)"=w2615, "main ref"=w2613) -> ("error out"=w2614:errorcluster)  [unwired: 9 in]
        n1593 = Unbundle By Name(w2613) -> ("Motion Module.Sway Right MM"=w2622:refnum<vi>)
        n1594 = property on="Property Node" class="Bool (strict)"(reference=w2622, "Value"=FALSE) -> (reference out=w2620:refnum<vi>, error out=w2621:errorcluster)  [unwired: 1 in]
        n1595 = Close Reference(reference=w2620, error in (no error)=w2621) -> ()  [unwired: 1 out]
        n1596 = call "DATA ENCRYPT STRING FILE WRITE.vi"("error in (no error)"=w2614, "User Action"="User Pressed Sway Right in MM", "main ref"=w2613) -> ("error out"=w2617:errorcluster)  [unwired: 6 in, 1 out]
        n1597 = call "SWAY WRITE FGV.vi"("Enum - Menu"=Sway_Write_enum."WRITE", "error in (no error)"=w2617, "main ref"=w2613) -> ("error out"=w2616:errorcluster)  [unwired: 8 in]
      }
      frame "Sway Right Main" {
        n1598 = call "Sway Right Main.vi"("error in (no error)"=w2626, "main ref"=w2624) -> ("error out"=w2625:errorcluster)  [unwired: 9 in]
        n1599 = Unbundle By Name(w2624) -> ("Platform Settings.Sway Right Main"=w2633:refnum<vi>)
        n1600 = property on="Property Node" class="Bool (strict)"(reference=w2633, "Value"=FALSE) -> (reference out=w2631:refnum<vi>, error out=w2632:errorcluster)  [unwired: 1 in]
        n1601 = Close Reference(reference=w2631, error in (no error)=w2632) -> ()  [unwired: 1 out]
        n1602 = call "DATA ENCRYPT STRING FILE WRITE.vi"("error in (no error)"=w2625, "User Action"="User Pressed Sway Right", "main ref"=w2624) -> ("error out"=w2628:errorcluster)  [unwired: 6 in, 1 out]
        n1603 = call "SWAY WRITE FGV.vi"("Enum - Menu"=Sway_Write_enum."WRITE", "error in (no error)"=w2628, "main ref"=w2624) -> ("error out"=w2627:errorcluster)  [unwired: 8 in]
      }
      frame "Manual Write Heave & Surge" {
        n1604 = Unbundle By Name(w2634) -> ("Heave AND Surge.Manual Write"=w2643:refnum<vi>)
        n1605 = property on="Property Node" class="Bool (strict)"(reference=w2643, "Value"=FALSE) -> (reference out=w2641:refnum<vi>, error out=w2642:errorcluster)  [unwired: 1 in]
        n1606 = Close Reference(reference=w2641, error in (no error)=w2642) -> ()  [unwired: 1 out]
        n1607 = call "DATA ENCRYPT STRING FILE WRITE.vi"("error in (no error)"=w2635, "User Action"="User Pressed Manual Write Heave and Surge", "main ref"=w2634) -> ("error out"=w2638:errorcluster)  [unwired: 6 in, 1 out]
        n1608 = call "HEAVE WRITE FGV.vi"("Enum - Menu"=Heave_Write_enum."WRITE", "error in (no error)"=w2638, "main ref"=w2634) -> ("error out"=w2637:errorcluster)  [unwired: 8 in]
      }
      frame "Manual Write SWAY" {
        n1609 = Unbundle By Name(w2645) -> ("SWAY.Manual Write SWAY"=w2653:refnum<vi>)
        n1610 = property on="Property Node" class="Bool (strict)"(reference=w2653, "Value"=FALSE) -> (reference out=w2651:refnum<vi>, error out=w2652:errorcluster)  [unwired: 1 in]
        n1611 = Close Reference(reference=w2651, error in (no error)=w2652) -> ()  [unwired: 1 out]
        n1612 = call "DATA ENCRYPT STRING FILE WRITE.vi"("error in (no error)"=w2646, "User Action"="User Pressed Manual Write Sway", "main ref"=w2645) -> ("error out"=w2648:errorcluster)  [unwired: 6 in, 1 out]
        n1613 = call "SWAY WRITE FGV.vi"("Enum - Menu"=Sway_Write_enum."WRITE", "error in (no error)"=w2648, "main ref"=w2645) -> ("error out"=w2647:errorcluster)  [unwired: 8 in]
      }
      frame "Manual Write TRACTION" {
        n1614 = Unbundle By Name(w2655) -> ("Traction.Manual Write TRACTION"=w2663:refnum<vi>)
        n1615 = property on="Property Node" class="Bool (strict)"(reference=w2663, "Value"=FALSE) -> (reference out=w2661:refnum<vi>, error out=w2662:errorcluster)  [unwired: 1 in]
        n1616 = Close Reference(reference=w2661, error in (no error)=w2662) -> ()  [unwired: 1 out]
        n1617 = call "DATA ENCRYPT STRING FILE WRITE.vi"("error in (no error)"=w2656, "User Action"="User Pressed Manual Write Traction", "main ref"=w2655) -> ("error out"=w2658:errorcluster)  [unwired: 6 in, 1 out]
        n1618 = call "TRACTION WRITE FGV.vi"("Enum - Menu"=Traction_Write_enum."WRITE", "error in (no error)"=w2658, "main ref"=w2655) -> ("error out"=w2657:errorcluster)  [unwired: 8 in]
      }
      frame "Manual Write ACQUOSTIC" {
        n1619 = local write "Manual Write Acquostic"(FALSE ("Manual Write Acquostic")) -> ()
        n1620 = call "DATA ENCRYPT STRING FILE WRITE.vi"("error in (no error)"=w2667, "User Action"="User Pressed Manual Write Acquostics", "main ref"=w2666) -> ("error out"=w2669:errorcluster)  [unwired: 6 in, 1 out]
        n1621 = call "Acq Write Loop.vi"("Enum - Menu"=Write_Main_Enum."WRITE", "error in (no error)"=w2669, "main ref"=w2666) -> ("error out"=w2668:errorcluster)  [unwired: 8 in]
      }
      frame "Load En" {
        # "zNL 2"
        n1622 = Unbundle By Name(w2672) -> ("Main Screen.Load En"=w2677:refnum<vi>)
        n1623 = property on="Property Node" class="Bool (strict)"(reference=w2677) -> (reference out=w2675:refnum<vi>, error out=w2676:errorcluster, "Value"=w2671:bool)  [unwired: 1 in]
        n1624 = Close Reference(reference=w2675, error in (no error)=w2676) -> ()  [unwired: 1 out]
        n1625 = case shown="True" w2671 {
          tunnel: [w2689 w2699] -> w2673
          tunnel: w2674 -> [w2691 w2698]
          tunnel: w2672 -> [w2679 w2693]
          tunnel: w2672 -> [w2687 _]
          tunnel: w2672 -> [w2686 _]
          frame False {
            n1626 = call "DATA ENCRYPT STRING FILE WRITE.vi"("error in (no error)"=w2691, "User Action"="User Pressed UnLoad on Main Screen", "main ref"=w2679) -> ("error out"=w2680:errorcluster)  [unwired: 6 in, 1 out]
            n1627 = call "Stall Data Flow.vim"("value in"=w2680, "milliseconds to wait"=u32 2000) -> ("value out"=w2685:errorcluster)  [unwired: 1 out]
            n1628 = Unbundle By Name(w2679) -> ("Main Screen.zNL 2"=w2683:refnum<vi>)
            n1629 = property on="Property Node" class="Bool (strict)"(reference=w2683, "DisabledEnum"=T24."Enabled" ("Disabled")) -> (reference out=w2681:refnum<vi>, error out=w2682:errorcluster)  [unwired: 1 in]
            n1630 = call "PID UNLOAD.vi"("error in (no error)"=w2685, "main ref"=w2686) -> ("error out"=w2688:errorcluster)  [unwired: 9 in]
            n1631 = Close Reference(reference=w2681, error in (no error)=w2682) -> ()  [unwired: 1 out]
            n1632 = call "HEAVE WRITE FGV.vi"("Enum - Menu"=Heave_Write_enum."WRITE", "error in (no error)"=w2688, "main ref"=w2687) -> ("error out"=w2689:errorcluster)  [unwired: 8 in]
          }
          frame True {
            n1633 = call "DATA ENCRYPT STRING FILE WRITE.vi"("error in (no error)"=w2698, "User Action"="User Pressed Load on Main Screen", "main ref"=w2693) -> ("error out"=w2699:errorcluster)  [unwired: 6 in, 1 out]
            n1634 = Unbundle By Name(w2693) -> ("Main Screen.zNL 2"=w2697:refnum<vi>)
            n1635 = property on="Property Node" class="Bool (strict)"(reference=w2697, "DisabledEnum"=T24."Disabled and Grayed Out" ("Disabled")) -> (reference out=w2695:refnum<vi>, error out=w2696:errorcluster)  [unwired: 1 in]
            n1636 = Close Reference(reference=w2695, error in (no error)=w2696) -> ()  [unwired: 1 out]
          }
        }
      }
      frame "apply load" {
        n1637 = Unbundle By Name(w2702) -> ("Main Screen.Load En"=w2707:refnum<vi>)
        n1638 = property on="Property Node" class="Bool (strict)"(reference=w2707) -> (reference out=w2705:refnum<vi>, error out=w2706:errorcluster, "Value"=w2701:bool)  [unwired: 1 in]
        n1639 = Close Reference(reference=w2705, error in (no error)=w2706) -> ()  [unwired: 1 out]
        n1640 = case shown="False" w2701 {
          tunnel: [w2714 w2721] -> w2703
          tunnel: w2704 -> [w2717 w2720]
          tunnel: w2702 -> [w2716 w2719]
          tunnel: w2702 -> [w2711 _]
          tunnel: w2702 -> [w2710 _]
          frame False {
            n1641 = call "DATA ENCRYPT STRING FILE WRITE.vi"("error in (no error)"=w2717, "User Action"="User Pressed UnLoad on Service Screen", "main ref"=w2716) -> ("error out"=w2713:errorcluster)  [unwired: 6 in, 1 out]
            n1642 = call "Stall Data Flow.vim"("value in"=w2713, "milliseconds to wait"=u32 2000) -> ("value out"=w2709:errorcluster)  [unwired: 1 out]
            n1643 = call "PID UNLOAD.vi"("error in (no error)"=w2709, "main ref"=w2710) -> ("error out"=w2712:errorcluster)  [unwired: 9 in]
            n1644 = call "HEAVE WRITE FGV.vi"("Enum - Menu"=Heave_Write_enum."WRITE", "error in (no error)"=w2712, "main ref"=w2711) -> ("error out"=w2714:errorcluster)  [unwired: 8 in]
          }
          frame True {
            n1645 = call "DATA ENCRYPT STRING FILE WRITE.vi"("error in (no error)"=w2720, "User Action"="User Pressed Load on Service Screen", "main ref"=w2719) -> ("error out"=w2721:errorcluster)  [unwired: 6 in, 1 out]
          }
        }
      }
      frame "BACK" {
        w2728 = FALSE ("Value")
        n1646 = Unbundle By Name(w2723) -> ("Main Screen.BACK"=w2748:refnum<vi>)
        n1647 = property on="Property Node" class="Bool (strict)"(reference=w2748, "Value"=FALSE) -> (reference out=w2746:refnum<vi>, error out=w2747:errorcluster)  [unwired: 1 in]
        n1648 = Close Reference(reference=w2746, error in (no error)=w2747) -> ()  [unwired: 1 out]
        n1649 = call "DATA ENCRYPT STRING FILE WRITE.vi"("error in (no error)"=w2745, "User Action"="User Pressed Back on Main Screen", "main ref"=w2723) -> ("error out"=w2743:errorcluster)  [unwired: 6 in, 1 out]
        n1650 = Unbundle By Name(w2723) -> ("Main Home Screen.MainPage"=w2735:refnum<vi>)
        n1651 = Unbundle By Name(w2723) -> ("Main Screen.Start Test"=w2731:refnum<vi>)
        n1652 = Unbundle By Name(w2723) -> ("Main Screen.STOP"=w2730:refnum<vi>)
        n1653 = Unbundle By Name(w2723) -> ("Main Home Screen.GUI"=w2739:refnum<vi>)
        n1654 = property on="Property Node" class="TabCtl (strict)"(reference=w2735, "Value"=T9."HOME") -> (reference out=w2737:refnum<vi>, error out=w2736:errorcluster)  [unwired: 1 in]
        n1655 = property on="Property Node" class="TabCtl (strict)"(reference=w2739, "Value"=T8."Setup") -> (reference out=w2741:refnum<vi>, error out=w2740:errorcluster)  [unwired: 1 in]
        n1656 = property on="Property Node" class="Bool (strict)"(reference=w2731, "Visible"=TRUE ("Value"), "Value"=FALSE) -> (reference out=w2726:refnum<vi>, error out=w2732:errorcluster)  [unwired: 1 in]
        n1657 = property on="Property Node" class="Bool (strict)"(reference=w2730, "Value"=w2728, "Visible"=w2728) -> (reference out=w2725:refnum<vi>, error out=w2729:errorcluster)  [unwired: 1 in]
        n1658 = Close Reference(reference=w2741, error in (no error)=w2740) -> ()  [unwired: 1 out]
        n1659 = Close Reference(reference=w2737, error in (no error)=w2736) -> ()  [unwired: 1 out]
        n1660 = Close Reference(reference=w2726, error in (no error)=w2732) -> ()  [unwired: 1 out]
        n1661 = Close Reference(reference=w2725, error in (no error)=w2729) -> ()  [unwired: 1 out]
        n1662 = call "Reinitial Parameter After Test.vi"("error in (no error)"=w2743, "main ref"=w2723) -> ("error out"=w2724:errorcluster)  [unwired: 9 in]
      }
      frame "Start Test" {
        n1663 = Unbundle By Name(w2749) -> ("Environmental control.Acoustic Emission 3"=w2755:refnum<vi>)
        n1664 = property on="Property Node" class="Bool (strict)"(reference=w2755) -> (reference out=w2753:refnum<vi>, error out=w2754:errorcluster, "Value"=w2752:bool)  [unwired: 1 in]
        n1665 = Close Reference(reference=w2753, error in (no error)=w2754) -> ()  [unwired: 1 out]
        n1666 = case shown="True" w2752 {
          tunnel: w2751 -> [w2757 w2761]
          tunnel: [w2757 w2758] -> w2750
          tunnel: w2749 -> [_ w2759]
          frame False {
          }
          frame True {
            n1667 = call "Acq start.vi"("error in (no error)"=w2761, "Data Cluster"=w2759) -> ("error out"=w2760:errorcluster)  [unwired: 9 in]
            n1668 = call <vilib>:"Clear Errors.vi"("error in (no error)"=w2760) -> ("error out"=w2758:errorcluster)  [unwired: 5 in, 1 out]
          }
        }
        n1669 = call "Test Start Sequence.vi"("error in (no error)"=w2750, "Data Cluster"=w2749) -> ("error out"=w2756:errorcluster)  [unwired: 9 in]
      }
      frame "STOP" {
        n1670 = call "Test Stop.vi"("error in (no error)"=w2783, "Data Cluster"=w2762) -> ("error out"=w2763:errorcluster)  [unwired: 9 in]
        n1671 = Unbundle By Name(w2762) -> ("Main Screen.Load En"=w2782:refnum<vi>)
        n1672 = Unbundle By Name(w2762) -> ("Main Screen.CZ FF"=w2777:refnum<vi>)
        n1673 = Unbundle By Name(w2762) -> ("Main Screen.zFF"=w2774:refnum<vi>)
        n1674 = property on="Property Node" class="Bool (strict)"(reference=w2782, "DisabledEnum"=T24."Disabled and Grayed Out" ("Disabled")) -> (reference out=w2770:refnum<vi>, error out=w2781:errorcluster)  [unwired: 1 in]
        n1675 = property on="Property Node" class="Bool (strict)"(reference=w2777, "DisabledEnum"=T24."Disabled and Grayed Out" ("Disabled"), "Value"=FALSE ("Visible")) -> (reference out=w2776:refnum<vi>, error out=w2778:errorcluster)  [unwired: 1 in]
        n1676 = property on="Property Node" class="Bool (strict)"(reference=w2774, "DisabledEnum"=T24."Disabled and Grayed Out" ("Disabled"), "Value"=FALSE ("Visible")) -> (reference out=w2775:refnum<vi>, error out=w2773:errorcluster)  [unwired: 1 in]
        n1677 = Close Reference(reference=w2770, error in (no error)=w2781) -> ()  [unwired: 1 out]
        n1678 = Close Reference(reference=w2776, error in (no error)=w2778) -> ()  [unwired: 1 out]
        n1679 = Close Reference(reference=w2775, error in (no error)=w2773) -> ()  [unwired: 1 out]
        n1680 = Unbundle By Name(w2762) -> ("Environmental control.Acoustic Emission 3"=w2768:refnum<vi>)
        n1681 = property on="Property Node" class="Bool (strict)"(reference=w2768) -> (reference out=w2766:refnum<vi>, error out=w2767:errorcluster, "Value"=w2765:bool)  [unwired: 1 in]
        n1682 = Close Reference(reference=w2766, error in (no error)=w2767) -> ()  [unwired: 1 out]
        n1683 = case shown="False" w2765 {
          tunnel: w2763 -> [w2784 w2788]
          tunnel: [w2784 w2785] -> w2764
          tunnel: w2762 -> [_ w2786]
          frame False {
          }
          frame True {
            n1684 = call "Acq stop.vi"("error in (no error)"=w2788, "Data Cluster"=w2786) -> ("error out"=w2787:errorcluster)  [unwired: 9 in]
            n1685 = call <vilib>:"Clear Errors.vi"("error in (no error)"=w2787) -> ("error out"=w2785:errorcluster)  [unwired: 5 in, 1 out]
          }
        }
      }
      frame "PlaceModule" {
        n1686 = call "Place Module.vi"("error in (no error)"=w2791, "main ref"=w2789) -> ("error out"=w2790:errorcluster)  [unwired: 9 in]
      }
      frame "Stage Homing" {
        n1687 = call "HOMINING.vi"("error in (no error)"=w2794, "main ref"=w2792) -> ("error out"=w2793:errorcluster)  [unwired: 9 in]
      }
      frame "Clear 3" {
        n1688 = Unbundle By Name(w2796) -> ("Loading.Stribeck Table  For loading"=w2806:refnum<vi>)
        n1689 = Unbundle By Name(w2796) -> ("Loading.Clear 3"=w2797:refnum<vi>)
        n1690 = property on="Property Node" class="Bool (strict)"(reference=w2797, "Value"=FALSE) -> (reference out=w2799:refnum<vi>, error out=w2798:errorcluster)  [unwired: 1 in]
        n1691 = call "DATA ENCRYPT STRING FILE WRITE.vi"("error in (no error)"=w2802, "User Action"="User Pressed Clear  on Step Load Sequence", "main ref"=w2796) -> ("error out"=w2801:errorcluster)  [unwired: 6 in, 1 out]
        n1692 = property on="Property Node" class="Tbl (strict)"(reference=w2806, "Value"=string[][] []) -> (reference out=w2804:refnum<vi>, error out=w2805:errorcluster)  [unwired: 1 in]
        n1693 = Close Reference(reference=w2799, error in (no error)=w2798) -> ()  [unwired: 1 out]
        n1694 = Close Reference(reference=w2804, error in (no error)=w2805) -> ()  [unwired: 1 out]
      }
      frame "Set WTD" {
        n1695 = Unbundle By Name(w2807) -> ("Motion Module.Set WTD"=w2810:refnum<vi>)
        n1696 = property on="Property Node" class="Bool (strict)"(reference=w2810, "Value"=FALSE) -> (reference out=w2812:refnum<vi>, error out=w2811:errorcluster)  [unwired: 1 in]
        n1697 = call "DATA ENCRYPT STRING FILE WRITE.vi"("error in (no error)"=w2814, "User Action"="User Pressed  on Set Wear Track", "main ref"=w2807) -> ("error out"=w2813:errorcluster)  [unwired: 6 in, 1 out]
        n1698 = call "Sway wear trac set.vi"("error in (no error)"=w2813, "main ref"=w2807) -> ("error out"=w2808:errorcluster)  [unwired: 9 in]
        n1699 = Close Reference(reference=w2812, error in (no error)=w2811) -> ()  [unwired: 1 out]
      }
      frame "Import 2" {
        n1700 = call "File Dialog"("start path"=path "C:/LAB-IQ 150/User Defined Protocol", "error in"=w2823) -> ("selected path"=w2817:path, "cancelled"=w2820:bool, "error out"=w2822:errorcluster)  [unwired: 10 in, 1 out]
        n1701 = call <vilib>:"Clear Errors.vi"("error in (no error)"=w2822) -> ("error out"=w2819:errorcluster)  [unwired: 5 in, 1 out]
        n1702 = case shown="False" w2820 {
          tunnel: w2819 -> [w2833 w2834]
          tunnel: [w2825 w2834] -> w2818
          tunnel: w2817 -> [w2832 _]
          tunnel: w2816 -> [w2827 _]
          frame False {
            n1703 = call-poly <vilib>:"Read Delimited Spreadsheet.vi"("file path (dialog if empty)"=w2832, "error in (no error)"=w2833, "delimiter (\\t)"=":" ("delimiter (\\t)")) -> ("all rows"=w2824:string[][], "error out"=w2826:errorcluster)  [unwired: 7 in, 4 out]
            n1704 = Unbundle By Name(w2827) -> ("Motion Module.StepTable For Speed"=w2830:refnum<vi>)
            n1705 = property on="Property Node" class="Tbl (strict)"(reference=w2830, error in=w2826, "Value"=w2824) -> (reference out=w2828:refnum<vi>, error out=w2829:errorcluster)
            n1706 = Close Reference(reference=w2828, error in (no error)=w2829) -> (error out=w2825:errorcluster)
          }
          frame True {
          }
        }
      }
      frame "Save 2" {
        n1707 = Unbundle By Name(w2838) -> ("Motion Module.StepTable For Speed"=w2853:refnum<vi>)
        n1708 = property on="Property Node" class="Tbl (strict)"(reference=w2853) -> (reference out=w2851:refnum<vi>, error out=w2852:errorcluster, "Value"=w2849:string[][])  [unwired: 1 in]
        n1709 = call "File Dialog2"("start path"=path "C:/LAB-IQ 150/User Defined Protocol", "error in"=w2843) -> ("selected path"=w2846:path, "error out"=w2845:errorcluster)  [unwired: 10 in, 2 out]
        n1710 = call <vilib>:"Clear Errors.vi"("error in (no error)"=w2845) -> ("error out"=w2844:errorcluster)  [unwired: 5 in, 1 out]
        n1711 = Close Reference(reference=w2851, error in (no error)=w2852) -> ()  [unwired: 1 out]
        n1712 = call-poly <vilib>:"Write Delimited Spreadsheet.vi"("file path (dialog if empty)"=w2846, "2D data"=w2849, "append to file? (new file:F)"=TRUE, "error in (no error)"=w2844, "delimiter (\\t)"=":" ("delimiter (\\t)")) -> ("error out"=w2842:errorcluster)  [unwired: 9 in, 1 out]
        n1713 = call <vilib>:"Clear Errors.vi"("error in (no error)"=w2842) -> ("error out"=w2837:errorcluster)  [unwired: 5 in, 1 out]
        n1714 = Unbundle By Name(w2838) -> ("Motion Module.Save 2"=w2839:refnum<vi>)
        n1715 = property on="Property Node" class="Bool (strict)"(reference=w2839, error in=w2837, "Value"=FALSE) -> (reference out=w2841:refnum<vi>, error out=w2840:errorcluster)
        n1716 = Close Reference(reference=w2841, error in (no error)=w2840) -> (error out=w2836:errorcluster)
      }
      frame "Calculate Rotary" {
        n1717 = call "STEP LOAD MM_SEC AND RPM CONVERSION.vi"("error in (no error)"=w2857, "Data Cluster"=w2855) -> ("error out"=w2856:errorcluster)  [unwired: 9 in]
        n1718 = local write "calculate rotary"(FALSE) -> ()
      }
      frame "Clear List" {
        n1719 = Unbundle By Name(w2859) -> ("Environmental control.Sensors Picked"=w2866:refnum<vi>)
        n1720 = Unbundle By Name(w2859) -> ("Environmental control.Clear List"=w2860:refnum<vi>)
        n1721 = property on="Property Node" class="Bool (strict)"(reference=w2860, "Value"=FALSE) -> (reference out=w2862:refnum<vi>, error out=w2861:errorcluster)  [unwired: 1 in]
        n1722 = property on="Property Node" class="Str"(reference=w2866, "Value"="") -> (reference out=w2864:refnum<vi>, error out=w2865:errorcluster)  [unwired: 1 in]
        n1723 = Close Reference(reference=w2862, error in (no error)=w2861) -> ()  [unwired: 1 out]
        n1724 = Close Reference(reference=w2864, error in (no error)=w2865) -> ()  [unwired: 1 out]
      }
      frame "ClrLog" {
        n1725 = Unbundle By Name(w2869) -> ("Main Screen.ClrLog"=w2870:refnum<vi>)
        n1726 = Unbundle By Name(w2869) -> ("Main Screen.Trip Log"=w2876:refnum<vi>)
        n1727 = property on="Property Node" class="Bool (strict)"(reference=w2870, "Value"=FALSE) -> (reference out=w2872:refnum<vi>, error out=w2871:errorcluster)  [unwired: 1 in]
        n1728 = property on="Property Node" class="Str"(reference=w2876, "Value"="") -> (reference out=w2874:refnum<vi>, error out=w2875:errorcluster)  [unwired: 1 in]
        n1729 = Close Reference(reference=w2872, error in (no error)=w2871) -> ()  [unwired: 1 out]
        n1730 = Close Reference(reference=w2874, error in (no error)=w2875) -> ()  [unwired: 1 out]
      }
      frame "Add to list" {
        n1731 = Unbundle By Name(w2878) -> ("Environmental control.Sensors Picked"=w2884:refnum<vi>)
        n1732 = property on="Property Node" class="Str"(reference=w2884, error in=w2879, "Value"="") -> (reference out=w2882:refnum<vi>, error out=w2883:errorcluster)
        n1733 = Close Reference(reference=w2882, error in (no error)=w2883) -> (error out=w2880:errorcluster)
        n1734 = call "Add  to List Loop.vi"("error in (no error)"=w2880, "Data Cluster"=w2878) -> ("error out"=w2886:errorcluster)  [unwired: 9 in]
        n1735 = Unbundle By Name(w2878) -> ("Environmental control.Add to list"=w2888:refnum<vi>)
        n1736 = property on="Property Node" class="Bool (strict)"(reference=w2888, error in=w2886, "Value"=FALSE) -> (reference out=w2890:refnum<vi>, error out=w2889:errorcluster)
        n1737 = Close Reference(reference=w2890, error in (no error)=w2889) -> (error out=w2885:errorcluster)
      }
      frame "Disable Axis Jog Soft Limits" {
        n1738 = call "DATA ENCRYPT STRING FILE WRITE.vi"("error in (no error)"=w2894, "User Action"="User Pressed Disable Axis Jog Soft Limits in Main Screen", "main ref"=w2892) -> ("error out"=w2893:errorcluster)  [unwired: 6 in, 1 out]
      }
      frame "Home Service" {
        n1739 = Unbundle By Name(w2896) -> ("Main Home Screen.MainPage"=w2902:refnum<vi>)
        n1740 = Unbundle By Name(w2896) -> ("Main Home Screen.GUI"=w2900:refnum<vi>)
        n1741 = local write "Home Service"(FALSE ("Home Service")) -> ()
        n1742 = property on="Property Node" class="TabCtl (strict)"(reference=w2902, "Value"=T9."HOME") -> (reference out=w2904:refnum<vi>, error out=w2903:errorcluster)  [unwired: 1 in]
        n1743 = property on="Property Node" class="TabCtl (strict)"(reference=w2900, "Value"=T8."Setup") -> (reference out=w2898:refnum<vi>, error out=w2899:errorcluster)  [unwired: 1 in]
        n1744 = Close Reference(reference=w2904, error in (no error)=w2903) -> ()  [unwired: 1 out]
        n1745 = Close Reference(reference=w2898, error in (no error)=w2899) -> ()  [unwired: 1 out]
        n1746 = call "DATA ENCRYPT STRING FILE WRITE.vi"("error in (no error)"=w2907, "User Action"="User Pressed Home Service from Service Screen", "main ref"=w2896) -> ("error out"=w2906:errorcluster)  [unwired: 6 in, 1 out]
      }
      frame "Analysis Home" {
        n1747 = Unbundle By Name(w2909) -> ("Main Screen.Main Screen Tab"=w2912:refnum<vi>)
        n1748 = Unbundle By Name(w2909) -> ("Main Home Screen.MainPage"=w2919:refnum<vi>)
        n1749 = Unbundle By Name(w2909) -> ("Main Home Screen.GUI"=w2917:refnum<vi>)
        n1750 = local write "Analysis Home new"(FALSE ("Analysis Home new")) -> ()
        n1751 = property on="Property Node" class="TabCtl (strict)"(reference=w2912, "Value"=T12."  Acquire  ") -> (reference out=w2910:refnum<vi>, error out=w2911:errorcluster)  [unwired: 1 in]
        n1752 = property on="Property Node" class="TabCtl (strict)"(reference=w2919, "Value"=T9."HOME") -> (reference out=w2921:refnum<vi>, error out=w2920:errorcluster)  [unwired: 1 in]
        n1753 = property on="Property Node" class="TabCtl (strict)"(reference=w2917, "Value"=T8."Setup") -> (reference out=w2915:refnum<vi>, error out=w2916:errorcluster)  [unwired: 1 in]
        n1754 = Close Reference(reference=w2910, error in (no error)=w2911) -> ()  [unwired: 1 out]
        n1755 = Close Reference(reference=w2921, error in (no error)=w2920) -> ()  [unwired: 1 out]
        n1756 = Close Reference(reference=w2915, error in (no error)=w2916) -> ()  [unwired: 1 out]
        n1757 = call "DATA ENCRYPT STRING FILE WRITE.vi"("error in (no error)"=w2924, "User Action"="User Pressed Home from AnalysisScreen", "main ref"=w2909) -> ("error out"=w2923:errorcluster)  [unwired: 6 in, 1 out]
      }
      frame "Post Analysis" {
        n1758 = Unbundle By Name(w2927) -> ("Main Screen.Main Screen Tab"=w2930:refnum<vi>)
        n1759 = Unbundle By Name(w2927) -> ("Main Home Screen.MainPage"=w2936:refnum<vi>)
        n1760 = Unbundle By Name(w2927) -> ("Main Home Screen.GUI"=w2934:refnum<vi>)
        n1761 = property on="Property Node" class="TabCtl (strict)"(reference=w2930, "Value"=T12."Compare Files Rot") -> (reference out=w2928:refnum<vi>, error out=w2929:errorcluster)  [unwired: 1 in]
        n1762 = property on="Property Node" class="TabCtl (strict)"(reference=w2936, "Value"=T9."HOME") -> (reference out=w2938:refnum<vi>, error out=w2937:errorcluster)  [unwired: 1 in]
        n1763 = property on="Property Node" class="TabCtl (strict)"(reference=w2934, "Value"=T8."Begin") -> (reference out=w2932:refnum<vi>, error out=w2933:errorcluster)  [unwired: 1 in]
        n1764 = local write "Post Analysis"(FALSE ("Post Analysis")) -> ()
        n1765 = Close Reference(reference=w2928, error in (no error)=w2929) -> ()  [unwired: 1 out]
        n1766 = Close Reference(reference=w2938, error in (no error)=w2937) -> ()  [unwired: 1 out]
        n1767 = Close Reference(reference=w2932, error in (no error)=w2933) -> ()  [unwired: 1 out]
        n1768 = call "DATA ENCRYPT STRING FILE WRITE.vi"("error in (no error)"=w2941, "User Action"="User Pressed Post Analysis ", "main ref"=w2927) -> ("error out"=w2940:errorcluster)  [unwired: 6 in, 1 out]
      }
      frame "Edit Gain Constants" {
        n1769 = Unbundle By Name(w2943) -> ("About Screen.Heave and Surge COM Port:"=w2973:refnum<vi>)
        n1770 = Unbundle By Name(w2943) -> ("About Screen.Edit Gain Constants"=w2953:refnum<vi>)
        n1771 = Unbundle By Name(w2943) -> ("About Screen.Sway COM Port:"=w2970:refnum<vi>)
        n1772 = Unbundle By Name(w2943) -> ("About Screen.Ramp Port:"=w2947:refnum<vi>)
        n1773 = Unbundle By Name(w2943) -> ("About Screen.Temp Modbus:"=w2967:refnum<vi>)
        n1774 = Unbundle By Name(w2943) -> ("About Screen.Humidity Port:"=w2966:refnum<vi>)
        n1775 = Unbundle By Name(w2943) -> ("About Screen.Password"=w2961:refnum<vi>)
        n1776 = Unbundle By Name(w2943) -> ("About Screen.ECR Port:"=w2946:refnum<vi>)
        n1777 = property on="Property Node" class="VISAName"(reference=w2947, "DisabledEnum"=T24."Enabled" ("Disabled")) -> (reference out=w2949:refnum<vi>, error out=w2948:errorcluster)  [unwired: 1 in]
        n1778 = property on="Property Node" class="Bool (strict)"(reference=w2953, "Value"=FALSE) -> (reference out=w2954:refnum<vi>, error out=w2952:errorcluster)  [unwired: 1 in]
        n1779 = property on="Property Node" class="VISAName"(reference=w2946, "DisabledEnum"=T24."Enabled" ("Disabled")) -> (reference out=w2942:refnum<vi>, error out=w2945:errorcluster)  [unwired: 1 in]
        n1780 = property on="Property Node" class="VISAName"(reference=w2973, "DisabledEnum"=T24."Enabled" ("Disabled")) -> (reference out=w2974:refnum<vi>, error out=w2972:errorcluster)  [unwired: 1 in]
        n1781 = property on="Property Node" class="VISAName"(reference=w2970, "DisabledEnum"=T24."Enabled" ("Disabled")) -> (reference out=w2971:refnum<vi>, error out=w2969:errorcluster)  [unwired: 1 in]
        n1782 = property on="Property Node" class="VISAName"(reference=w2967, "DisabledEnum"=T24."Enabled" ("Disabled")) -> (reference out=w2955:refnum<vi>, error out=w2968:errorcluster)  [unwired: 1 in]
        n1783 = property on="Property Node" class="VISAName"(reference=w2966, "DisabledEnum"=T24."Enabled" ("Disabled")) -> (reference out=w2964:refnum<vi>, error out=w2965:errorcluster)  [unwired: 1 in]
        n1784 = property on="Property Node" class="Str"(reference=w2961, "Visible"=FALSE) -> (reference out=w2963:refnum<vi>, error out=w2962:errorcluster)  [unwired: 1 in]
        n1785 = Close Reference(reference=w2949, error in (no error)=w2948) -> ()  [unwired: 1 out]
        n1786 = Close Reference(reference=w2963, error in (no error)=w2962) -> ()  [unwired: 1 out]
        n1787 = Close Reference(reference=w2942, error in (no error)=w2945) -> ()  [unwired: 1 out]
        n1788 = Close Reference(reference=w2954, error in (no error)=w2952) -> ()  [unwired: 1 out]
        n1789 = Close Reference(reference=w2974, error in (no error)=w2972) -> ()  [unwired: 1 out]
        n1790 = Close Reference(reference=w2971, error in (no error)=w2969) -> ()  [unwired: 1 out]
        n1791 = Close Reference(reference=w2955, error in (no error)=w2968) -> ()  [unwired: 1 out]
        n1792 = Close Reference(reference=w2964, error in (no error)=w2965) -> ()  [unwired: 1 out]
        n1793 = call "DATA ENCRYPT STRING FILE WRITE.vi"("error in (no error)"=w2977, "User Action"="User Pressed Home Service from Service Screen", "main ref"=w2943) -> ("error out"=w2976:errorcluster)  [unwired: 6 in, 1 out]
      }
      frame "Advanced Setting" {
        n1794 = Unbundle By Name(w2979) -> ("About Screen.Advanced Setting"=w2981:refnum<vi>)
        n1795 = property on="Property Node" class="Bool (strict)"(reference=w2981) -> (reference out=w2982:refnum<vi>, error out=w2980:errorcluster, "Value"=w2978:bool)  [unwired: 1 in]
        n1796 = Close Reference(reference=w2982, error in (no error)=w2980) -> ()  [unwired: 1 out]
        n1797 = case shown="True" w2978 {
          tunnel: w2979 -> [w2987 w3012]
          frame True {
            n1798 = Unbundle By Name(w2987) -> ("About Screen.Heave and Surge COM Port:"=w3009:refnum<vi>)
            n1799 = Unbundle By Name(w2987) -> ("About Screen.Edit Gain Constants"=w2989:refnum<vi>)
            n1800 = Unbundle By Name(w2987) -> ("About Screen.Sway COM Port:"=w3006:refnum<vi>)
            n1801 = Unbundle By Name(w2987) -> ("About Screen.Temp Modbus:"=w3003:refnum<vi>)
            n1802 = Unbundle By Name(w2987) -> ("About Screen.Humidity Port:"=w3002:refnum<vi>)
            n1803 = Unbundle By Name(w2987) -> ("About Screen.Password"=w2997:refnum<vi>)
            n1804 = property on="Property Node" class="Bool (strict)"(reference=w2989, "Value"=FALSE) -> (reference out=w2990:refnum<vi>, error out=w2988:errorcluster)  [unwired: 1 in]
            n1805 = property on="Property Node" class="VISAName"(reference=w3009, "DisabledEnum"=T24."Disabled and Grayed Out" ("Disabled")) -> (reference out=w3010:refnum<vi>, error out=w3008:errorcluster)  [unwired: 1 in]
            n1806 = property on="Property Node" class="VISAName"(reference=w3006, "DisabledEnum"=T24."Disabled and Grayed Out" ("Disabled")) -> (reference out=w3007:refnum<vi>, error out=w3005:errorcluster)  [unwired: 1 in]
            n1807 = property on="Property Node" class="VISAName"(reference=w3003, "DisabledEnum"=T24."Disabled and Grayed Out" ("Disabled")) -> (reference out=w2991:refnum<vi>, error out=w3004:errorcluster)  [unwired: 1 in]
            n1808 = property on="Property Node" class="VISAName"(reference=w3002, "DisabledEnum"=T24."Disabled and Grayed Out" ("Disabled")) -> (reference out=w3000:refnum<vi>, error out=w3001:errorcluster)  [unwired: 1 in]
            n1809 = property on="Property Node" class="Str"(reference=w2997, "Visible"=TRUE) -> (reference out=w2999:refnum<vi>, error out=w2998:errorcluster)  [unwired: 1 in]
            n1810 = Close Reference(reference=w2990, error in (no error)=w2988) -> ()  [unwired: 1 out]
            n1811 = Close Reference(reference=w3010, error in (no error)=w3008) -> ()  [unwired: 1 out]
            n1812 = Close Reference(reference=w3007, error in (no error)=w3005) -> ()  [unwired: 1 out]
            n1813 = Close Reference(reference=w2991, error in (no error)=w3004) -> ()  [unwired: 1 out]
            n1814 = Close Reference(reference=w3000, error in (no error)=w3001) -> ()  [unwired: 1 out]
            n1815 = Close Reference(reference=w2999, error in (no error)=w2998) -> ()  [unwired: 1 out]
          }
          frame False {
            n1816 = Unbundle By Name(w3012) -> ("About Screen.Heave and Surge COM Port:"=w3034:refnum<vi>)
            n1817 = Unbundle By Name(w3012) -> ("About Screen.Edit Gain Constants"=w3014:refnum<vi>)
            n1818 = Unbundle By Name(w3012) -> ("About Screen.Sway COM Port:"=w3031:refnum<vi>)
            n1819 = Unbundle By Name(w3012) -> ("About Screen.Temp Modbus:"=w3028:refnum<vi>)
            n1820 = Unbundle By Name(w3012) -> ("About Screen.Humidity Port:"=w3027:refnum<vi>)
            n1821 = Unbundle By Name(w3012) -> ("About Screen.Password"=w3022:refnum<vi>)
            n1822 = property on="Property Node" class="Bool (strict)"(reference=w3014, "Value"=FALSE) -> (reference out=w3015:refnum<vi>, error out=w3013:errorcluster)  [unwired: 1 in]
            n1823 = property on="Property Node" class="VISAName"(reference=w3034, "DisabledEnum"=T24."Disabled and Grayed Out" ("Disabled")) -> (reference out=w3035:refnum<vi>, error out=w3033:errorcluster)  [unwired: 1 in]
            n1824 = property on="Property Node" class="VISAName"(reference=w3031, "DisabledEnum"=T24."Disabled and Grayed Out" ("Disabled")) -> (reference out=w3032:refnum<vi>, error out=w3030:errorcluster)  [unwired: 1 in]
            n1825 = property on="Property Node" class="VISAName"(reference=w3028, "DisabledEnum"=T24."Disabled and Grayed Out" ("Disabled")) -> (reference out=w3016:refnum<vi>, error out=w3029:errorcluster)  [unwired: 1 in]
            n1826 = property on="Property Node" class="VISAName"(reference=w3027, "DisabledEnum"=T24."Disabled and Grayed Out" ("Disabled")) -> (reference out=w3025:refnum<vi>, error out=w3026:errorcluster)  [unwired: 1 in]
            n1827 = property on="Property Node" class="Str"(reference=w3022, "Visible"=FALSE) -> (reference out=w3024:refnum<vi>, error out=w3023:errorcluster)  [unwired: 1 in]
            n1828 = Close Reference(reference=w3015, error in (no error)=w3013) -> ()  [unwired: 1 out]
            n1829 = Close Reference(reference=w3035, error in (no error)=w3033) -> ()  [unwired: 1 out]
            n1830 = Close Reference(reference=w3032, error in (no error)=w3030) -> ()  [unwired: 1 out]
            n1831 = Close Reference(reference=w3016, error in (no error)=w3029) -> ()  [unwired: 1 out]
            n1832 = Close Reference(reference=w3025, error in (no error)=w3026) -> ()  [unwired: 1 out]
            n1833 = Close Reference(reference=w3024, error in (no error)=w3023) -> ()  [unwired: 1 out]
          }
        }
        n1834 = call "DATA ENCRYPT STRING FILE WRITE.vi"("error in (no error)"=w2985, "User Action"="User Pressed Advance Setting in Service Screen", "main ref"=w2979) -> ("error out"=w2984:errorcluster)  [unwired: 6 in, 1 out]
      }
      frame "Password" {
        n1835 = Unbundle By Name(w3036) -> ("About Screen.Password"=w3042:refnum<vi>)
        n1836 = property on="Property Node" class="Str"(reference=w3042) -> (reference out=w3043:refnum<vi>, error out=w3041:errorcluster, "Value"=w3040:string)  [unwired: 1 in]
        n1837 = call <vilib>:"Trim Whitespace.vi"("string"=w3040) -> ("trimmed string"=w3039:string)  [unwired: 1 in]
        n1838 = Close Reference(reference=w3043, error in (no error)=w3041) -> ()  [unwired: 1 out]
        n1839 = Equal?(x=w3039, y="UT150$") -> (x = y?=w3037:bool)
        n1840 = case shown="True" w3037 {
          tunnel: w3036 -> [_ w3046]
          frame False {
          }
          frame True {
            n1841 = Unbundle By Name(w3046) -> ("Main Screen.Main Screen Tab"=w3048:refnum<vi>)
            n1842 = Unbundle By Name(w3046) -> ("Main Home Screen.GUI"=w3052:refnum<vi>)
            n1843 = Unbundle By Name(w3046) -> ("About Screen.Password"=w3056:refnum<vi>)
            n1844 = property on="Property Node" class="TabCtl (strict)"(reference=w3052, "Value"=T8."Begin") -> (reference out=w3053:refnum<vi>, error out=w3051:errorcluster)  [unwired: 1 in]
            n1845 = property on="Property Node" class="TabCtl (strict)"(reference=w3048, "Value"=T12."Service") -> (reference out=w3047:refnum<vi>, error out=w3049:errorcluster)  [unwired: 1 in]
            n1846 = property on="Property Node" class="Str"(reference=w3056, "Value"="") -> (reference out=w3057:refnum<vi>, error out=w3055:errorcluster)  [unwired: 1 in]
            n1847 = Close Reference(reference=w3057, error in (no error)=w3055) -> ()  [unwired: 1 out]
            n1848 = Close Reference(reference=w3053, error in (no error)=w3051) -> ()  [unwired: 1 out]
            n1849 = Close Reference(reference=w3047, error in (no error)=w3049) -> ()  [unwired: 1 out]
          }
        }
      }
      frame "Service About" {
        n1850 = Unbundle By Name(w3059) -> ("Main Screen.Main Screen Tab"=w3062:refnum<vi>)
        n1851 = Unbundle By Name(w3059) -> ("Main Home Screen.GUI"=w3066:refnum<vi>)
        n1852 = local write "Service About"(FALSE ("Service About")) -> ()
        n1853 = property on="Property Node" class="TabCtl (strict)"(reference=w3066, "Value"=T8."Begin") -> (reference out=w3067:refnum<vi>, error out=w3065:errorcluster)  [unwired: 1 in]
        n1854 = property on="Property Node" class="TabCtl (strict)"(reference=w3062, "Value"=T12."About") -> (reference out=w3061:refnum<vi>, error out=w3063:errorcluster)  [unwired: 1 in]
        n1855 = Close Reference(reference=w3067, error in (no error)=w3065) -> ()  [unwired: 1 out]
        n1856 = Close Reference(reference=w3061, error in (no error)=w3063) -> ()  [unwired: 1 out]
      }
      frame "OPEN 1" {
        n1857 = Unbundle By Name(w3071) -> ("Analysis Screen.File 1 Discription"=w3080:refnum<vi>)
        n1858 = property on="Property Node" class="Str"(reference=w3080, error in=w3078, "Value"="") -> (reference out=w3081:refnum<vi>, error out=w3079:errorcluster)
        n1859 = Close Reference(reference=w3081, error in (no error)=w3079) -> (error out=w3077:errorcluster)
        n1860 = call <vilib>:"Application Directory.vi"() -> ("Application Directory"=w3085:path)
        n1861 = Unbundle By Name(w3071) -> ("Analysis Screen.OPEN 1"=w3073:refnum<vi>)
        n1862 = Build Path(base path=w3085, name or relative path="data") -> (appended path=w3083:path)
        n1863 = property on="Property Node" class="Bool (strict)"(reference=w3073, "Value"=FALSE) -> (reference out=w3074:refnum<vi>, error out=w3072:errorcluster)  [unwired: 1 in]
        n1864 = call "File Dialog3"("start path"=w3083, "error in"=w3077) -> ("selected path"=w3082:path, "cancelled"=w3069:bool, "error out"=w3086:errorcluster)  [unwired: 10 in, 1 out]
        n1865 = case shown="True" w3069 {
          tunnel: w3086 -> [w3100 _]
          tunnel: w3082 -> [w3096 _]
          tunnel: [w3088 _] -> w3075
          tunnel: w3071 -> [w3087 w3102]
          frame False {
            n1866 = Path To String(path=w3096) -> (string=w3095:string)
            n1867 = Unbundle By Name(w3087) -> ("Analysis Screen.File Name 1"=w3098:refnum<vi>)
            n1868 = call <vilib>:"Clear Errors.vi"("error in (no error)"=w3100) -> ("error out"=w3094:errorcluster)  [unwired: 5 in, 1 out]
            n1869 = property on="Property Node" class="Str"(reference=w3098, "Value"=w3095) -> (reference out=w3099:refnum<vi>, error out=w3097:errorcluster)  [unwired: 1 in]
            n1870 = call "INI FILE READ.vi"("error in (no error)"=w3094, "File Path"=w3095) -> ("error out"=w3090:errorcluster, "concatenated string"=w3089:string)  [unwired: 8 in]
            n1871 = Unbundle By Name(w3087) -> ("Analysis Screen.File 1 Discription"=w3092:refnum<vi>)
            n1872 = Close Reference(reference=w3099, error in (no error)=w3097) -> ()  [unwired: 1 out]
            n1873 = property on="Property Node" class="Str"(reference=w3092, error in=w3090, "Value"=w3089) -> (reference out=w3093:refnum<vi>, error out=w3091:errorcluster)
            n1874 = Close Reference(reference=w3093, error in (no error)=w3091) -> (error out=w3088:errorcluster)
          }
          frame True {
            n1875 = Unbundle By Name(w3102) -> ("Analysis Screen.File 1 Discription"=w3104:refnum<vi>)
            n1876 = Unbundle By Name(w3102) -> ("Analysis Screen.File Name 1"=w3108:refnum<vi>)
            n1877 = property on="Property Node" class="Str"(reference=w3104, "Value"="") -> (reference out=w3105:refnum<vi>, error out=w3103:errorcluster)  [unwired: 1 in]
            n1878 = property on="Property Node" class="Str"(reference=w3108, "Value"="") -> (reference out=w3109:refnum<vi>, error out=w3107:errorcluster)  [unwired: 1 in]
            n1879 = Close Reference(reference=w3105, error in (no error)=w3103) -> ()  [unwired: 1 out]
            n1880 = Close Reference(reference=w3109, error in (no error)=w3107) -> ()  [unwired: 1 out]
          }
        }
        n1881 = Close Reference(reference=w3074, error in (no error)=w3072) -> ()  [unwired: 1 out]
      }
      frame "OPEN 2" {
        n1882 = Unbundle By Name(w3112) -> ("Analysis Screen.File 2 Discription"=w3121:refnum<vi>)
        n1883 = property on="Property Node" class="Str"(reference=w3121, error in=w3119, "Value"="") -> (reference out=w3122:refnum<vi>, error out=w3120:errorcluster)
        n1884 = Close Reference(reference=w3122, error in (no error)=w3120) -> (error out=w3118:errorcluster)
        n1885 = call <vilib>:"Application Directory.vi"() -> ("Application Directory"=w3126:path)
        n1886 = Unbundle By Name(w3112) -> ("Analysis Screen.OPEN 2"=w3114:refnum<vi>)
        n1887 = Build Path(base path=w3126, name or relative path="data") -> (appended path=w3124:path)
        n1888 = property on="Property Node" class="Bool (strict)"(reference=w3114, "Value"=FALSE) -> (reference out=w3115:refnum<vi>, error out=w3113:errorcluster)  [unwired: 1 in]
        n1889 = call "File Dialog4"("start path"=w3124, "error in"=w3118) -> ("selected path"=w3123:path, "cancelled"=w3110:bool, "error out"=w3127:errorcluster)  [unwired: 10 in, 1 out]
        n1890 = case shown="True" w3110 {
          tunnel: w3127 -> [w3141 w3143]
          tunnel: w3123 -> [w3137 _]
          tunnel: [w3129 w3142] -> w3116
          tunnel: w3112 -> [w3128 w3145]
          frame False {
            n1891 = Path To String(path=w3137) -> (string=w3136:string)
            n1892 = Unbundle By Name(w3128) -> ("Analysis Screen.File Name 2"=w3139:refnum<vi>)
            n1893 = call <vilib>:"Clear Errors.vi"("error in (no error)"=w3141) -> ("error out"=w3135:errorcluster)  [unwired: 5 in, 1 out]
            n1894 = property on="Property Node" class="Str"(reference=w3139, "Value"=w3136) -> (reference out=w3140:refnum<vi>, error out=w3138:errorcluster)  [unwired: 1 in]
            n1895 = call "INI FILE READ.vi"("error in (no error)"=w3135, "File Path"=w3136) -> ("error out"=w3131:errorcluster, "concatenated string"=w3130:string)  [unwired: 8 in]
            n1896 = Unbundle By Name(w3128) -> ("Analysis Screen.File 2 Discription"=w3133:refnum<vi>)
            n1897 = Close Reference(reference=w3140, error in (no error)=w3138) -> ()  [unwired: 1 out]
            n1898 = property on="Property Node" class="Str"(reference=w3133, error in=w3131, "Value"=w3130) -> (reference out=w3134:refnum<vi>, error out=w3132:errorcluster)
            n1899 = Close Reference(reference=w3134, error in (no error)=w3132) -> (error out=w3129:errorcluster)
          }
          frame True {
            n1900 = Unbundle By Name(w3145) -> ("Analysis Screen.File Name 2"=w3151:refnum<vi>)
            n1901 = Unbundle By Name(w3145) -> ("Analysis Screen.File 2 Discription"=w3147:refnum<vi>)
            n1902 = property on="Property Node" class="Str"(reference=w3151, "Value"="") -> (reference out=w3152:refnum<vi>, error out=w3150:errorcluster)  [unwired: 1 in]
            n1903 = property on="Property Node" class="Str"(reference=w3147, "Value"="") -> (reference out=w3146:refnum<vi>, error out=w3148:errorcluster)  [unwired: 1 in]
            n1904 = call <vilib>:"Clear Errors.vi"("error in (no error)"=w3143) -> ("error out"=w3142:errorcluster)  [unwired: 5 in, 1 out]
            n1905 = Close Reference(reference=w3146, error in (no error)=w3148) -> ()  [unwired: 1 out]
            n1906 = Close Reference(reference=w3152, error in (no error)=w3150) -> ()  [unwired: 1 out]
          }
        }
        n1907 = Close Reference(reference=w3115, error in (no error)=w3113) -> ()  [unwired: 1 out]
      }
      frame "OPEN 3" {
        # "3416\n4017\n4554"
        n1908 = Unbundle By Name(w3155) -> ("Analysis Screen.File 3 Discription"=w3164:refnum<vi>)
        n1909 = property on="Property Node" class="Str"(reference=w3164, error in=w3162, "Value"="") -> (reference out=w3165:refnum<vi>, error out=w3163:errorcluster)
        n1910 = Close Reference(reference=w3165, error in (no error)=w3163) -> (error out=w3161:errorcluster)
        n1911 = call <vilib>:"Application Directory.vi"() -> ("Application Directory"=w3169:path)
        n1912 = Unbundle By Name(w3155) -> ("Analysis Screen.OPEN 3"=w3157:refnum<vi>)
        n1913 = Build Path(base path=w3169, name or relative path="data") -> (appended path=w3167:path)
        n1914 = property on="Property Node" class="Bool (strict)"(reference=w3157, "Value"=FALSE) -> (reference out=w3158:refnum<vi>, error out=w3156:errorcluster)  [unwired: 1 in]
        n1915 = call "File Dialog5"("start path"=w3167, "error in"=w3161) -> ("selected path"=w3166:path, "cancelled"=w3153:bool, "error out"=w3170:errorcluster)  [unwired: 10 in, 1 out]
        n1916 = case shown="True" w3153 {
          tunnel: w3170 -> [w3184 w3186]
          tunnel: w3166 -> [w3180 _]
          tunnel: [w3172 w3185] -> w3159
          tunnel: w3155 -> [w3171 w3188]
          frame False {
            n1917 = Path To String(path=w3180) -> (string=w3179:string)
            n1918 = Unbundle By Name(w3171) -> ("Analysis Screen.File Name 3"=w3182:refnum<vi>)
            n1919 = call <vilib>:"Clear Errors.vi"("error in (no error)"=w3184) -> ("error out"=w3178:errorcluster)  [unwired: 5 in, 1 out]
            n1920 = property on="Property Node" class="Str"(reference=w3182, "Value"=w3179) -> (reference out=w3183:refnum<vi>, error out=w3181:errorcluster)  [unwired: 1 in]
            n1921 = call "INI FILE READ.vi"("error in (no error)"=w3178, "File Path"=w3179) -> ("error out"=w3174:errorcluster, "concatenated string"=w3173:string)  [unwired: 8 in]
            n1922 = Unbundle By Name(w3171) -> ("Analysis Screen.File 3 Discription"=w3176:refnum<vi>)
            n1923 = Close Reference(reference=w3183, error in (no error)=w3181) -> ()  [unwired: 1 out]
            n1924 = property on="Property Node" class="Str"(reference=w3176, error in=w3174, "Value"=w3173) -> (reference out=w3177:refnum<vi>, error out=w3175:errorcluster)
            n1925 = Close Reference(reference=w3177, error in (no error)=w3175) -> (error out=w3172:errorcluster)
          }
          frame True {
            n1926 = Unbundle By Name(w3188) -> ("Analysis Screen.File Name 3"=w3194:refnum<vi>)
            n1927 = Unbundle By Name(w3188) -> ("Analysis Screen.File 3 Discription"=w3190:refnum<vi>)
            n1928 = property on="Property Node" class="Str"(reference=w3194, "Value"="") -> (reference out=w3195:refnum<vi>, error out=w3193:errorcluster)  [unwired: 1 in]
            n1929 = property on="Property Node" class="Str"(reference=w3190, "Value"="") -> (reference out=w3189:refnum<vi>, error out=w3191:errorcluster)  [unwired: 1 in]
            n1930 = Close Reference(reference=w3189, error in (no error)=w3191) -> ()  [unwired: 1 out]
            n1931 = Close Reference(reference=w3195, error in (no error)=w3193) -> ()  [unwired: 1 out]
            n1932 = call <vilib>:"Clear Errors.vi"("error in (no error)"=w3186) -> ("error out"=w3185:errorcluster)  [unwired: 5 in, 1 out]
          }
        }
        n1933 = Close Reference(reference=w3158, error in (no error)=w3156) -> ()  [unwired: 1 out]
      }
      frame "OPEN 4" {
        n1934 = Unbundle By Name(w3198) -> ("Analysis Screen.File 4 Discription"=w3207:refnum<vi>)
        n1935 = property on="Property Node" class="Str"(reference=w3207, error in=w3205, "Value"="") -> (reference out=w3208:refnum<vi>, error out=w3206:errorcluster)
        n1936 = Close Reference(reference=w3208, error in (no error)=w3206) -> (error out=w3204:errorcluster)
        n1937 = call <vilib>:"Application Directory.vi"() -> ("Application Directory"=w3212:path)
        n1938 = Unbundle By Name(w3198) -> ("Analysis Screen.OPEN 4"=w3200:refnum<vi>)
        n1939 = Build Path(base path=w3212, name or relative path="data") -> (appended path=w3210:path)
        n1940 = property on="Property Node" class="Bool (strict)"(reference=w3200, "Value"=FALSE) -> (reference out=w3201:refnum<vi>, error out=w3199:errorcluster)  [unwired: 1 in]
        n1941 = call "File Dialog6"("start path"=w3210, "error in"=w3204) -> ("selected path"=w3209:path, "cancelled"=w3196:bool, "error out"=w3213:errorcluster)  [unwired: 10 in, 1 out]
        n1942 = case shown="True" w3196 {
          tunnel: w3213 -> [w3227 w3229]
          tunnel: w3209 -> [w3223 _]
          tunnel: [w3215 w3228] -> w3202
          tunnel: w3198 -> [w3214 w3231]
          frame False {
            n1943 = Path To String(path=w3223) -> (string=w3222:string)
            n1944 = Unbundle By Name(w3214) -> ("Analysis Screen.File Name 4"=w3225:refnum<vi>)
            n1945 = call <vilib>:"Clear Errors.vi"("error in (no error)"=w3227) -> ("error out"=w3221:errorcluster)  [unwired: 5 in, 1 out]
            n1946 = property on="Property Node" class="Str"(reference=w3225, "Value"=w3222) -> (reference out=w3226:refnum<vi>, error out=w3224:errorcluster)  [unwired: 1 in]
            n1947 = call "INI FILE READ.vi"("error in (no error)"=w3221, "File Path"=w3222) -> ("error out"=w3217:errorcluster, "concatenated string"=w3216:string)  [unwired: 8 in]
            n1948 = Unbundle By Name(w3214) -> ("Analysis Screen.File 4 Discription"=w3219:refnum<vi>)
            n1949 = Close Reference(reference=w3226, error in (no error)=w3224) -> ()  [unwired: 1 out]
            n1950 = property on="Property Node" class="Str"(reference=w3219, error in=w3217, "Value"=w3216) -> (reference out=w3220:refnum<vi>, error out=w3218:errorcluster)
            n1951 = Close Reference(reference=w3220, error in (no error)=w3218) -> (error out=w3215:errorcluster)
          }
          frame True {
            n1952 = Unbundle By Name(w3231) -> ("Analysis Screen.File Name 4"=w3237:refnum<vi>)
            n1953 = Unbundle By Name(w3231) -> ("Analysis Screen.File 4 Discription"=w3233:refnum<vi>)
            n1954 = property on="Property Node" class="Str"(reference=w3237, "Value"="") -> (reference out=w3238:refnum<vi>, error out=w3236:errorcluster)  [unwired: 1 in]
            n1955 = property on="Property Node" class="Str"(reference=w3233, "Value"="") -> (reference out=w3232:refnum<vi>, error out=w3234:errorcluster)  [unwired: 1 in]
            n1956 = Close Reference(reference=w3232, error in (no error)=w3234) -> ()  [unwired: 1 out]
            n1957 = Close Reference(reference=w3238, error in (no error)=w3236) -> ()  [unwired: 1 out]
            n1958 = call <vilib>:"Clear Errors.vi"("error in (no error)"=w3229) -> ("error out"=w3228:errorcluster)  [unwired: 5 in, 1 out]
          }
        }
        n1959 = Close Reference(reference=w3201, error in (no error)=w3199) -> ()  [unwired: 1 out]
      }
      frame "Refresh 2" {
        n1960 = call "Data Log Refresh.vi"("error in (no error)"=w3241, "Data Cluster"=w3240) -> ("error out"=w3242:errorcluster)  [unwired: 9 in]
        n1961 = local write "Refresh 2"(FALSE ("Refresh 2")) -> ()
      }
      frame "Scratch Mode" {
        n1962 = Unbundle By Name(w3243) -> ("Motion Module.Scratch Mode"=w3246:refnum<vi>)
        n1963 = property on="Property Node" class="Ring (strict)"(reference=w3246) -> (reference out=w3247:refnum<vi>, error out=w3245:errorcluster, "Value"=w3244:u16)  [unwired: 1 in]
        n1964 = Close Reference(reference=w3247, error in (no error)=w3245) -> ()  [unwired: 1 out]
        n1965 = case shown="2" w3244 {
          tunnel: w3243 -> [w3250 w3254]
          frame 0, Default {
            n1966 = Unbundle By Name(w3250) -> ("Motion Module.No of Scratch"=w3252:refnum<vi>)
            n1967 = property on="Property Node" class="DigNum (strict)"(reference=w3252, "Visible"=FALSE) -> (reference out=w3253:refnum<vi>, error out=w3251:errorcluster)  [unwired: 1 in]
            n1968 = Close Reference(reference=w3253, error in (no error)=w3251) -> ()  [unwired: 1 out]
          }
          frame 2 {
            n1969 = Unbundle By Name(w3254) -> ("Motion Module.No of Scratch"=w3257:refnum<vi>)
            n1970 = property on="Property Node" class="DigNum (strict)"(reference=w3257, "Visible"=TRUE) -> (reference out=w3258:refnum<vi>, error out=w3256:errorcluster)  [unwired: 1 in]
            n1971 = Close Reference(reference=w3258, error in (no error)=w3256) -> ()  [unwired: 1 out]
          }
        }
      }
      frame "Export" {
        n1972 = call "Export file.vi"("error in (no error)"=w3267, "Data Cluster"=w3260) -> ("error out"=w3262:errorcluster)  [unwired: 9 in]
        n1973 = call "DATA ENCRYPT STRING FILE WRITE.vi"("error in (no error)"=w3262, "User Action"="User Pressed  Export ", "main ref"=w3260) -> ("error out"=w3261:errorcluster)  [unwired: 6 in, 1 out]
        n1974 = Unbundle By Name(w3260) -> ("Analysis Screen.Export"=w3265:refnum<vi>)
        n1975 = property on="Property Node" class="Bool (strict)"(reference=w3265, "Value"=FALSE) -> (reference out=w3266:refnum<vi>, error out=w3264:errorcluster)  [unwired: 1 in]
        n1976 = Close Reference(reference=w3266, error in (no error)=w3264) -> ()  [unwired: 1 out]
      }
      frame "Traction Receipe Update Details" {
        n1977 = call "Traction Receipe Main.vi"("error in (no error)"=w3273, "main ref"=w3270) -> ("error out"=w3272:errorcluster)  [unwired: 9 in]
        n1978 = local write "Traction Receipe Update Details"(FALSE ("Traction Step Update Details")) -> ()
        n1979 = call "DATA ENCRYPT STRING FILE WRITE.vi"("error in (no error)"=w3272, "User Action"="User Pressed  Traction Update Details ", "main ref"=w3270) -> ("error out"=w3271:errorcluster)  [unwired: 6 in, 1 out]
      }
      frame "Acoustic Emission 3" {
        n1980 = Unbundle By Name(w3275) -> ("Environmental control.Acoustic Emission 3"=w3278:refnum<vi>)
        n1981 = property on="Property Node" class="Bool (strict)"(reference=w3278) -> (reference out=w3276:refnum<vi>, error out=w3277:errorcluster, "Value"=w3274:bool)  [unwired: 1 in]
        n1982 = Close Reference(reference=w3276, error in (no error)=w3277) -> ()  [unwired: 1 out]
        n1983 = case shown="True" w3274 {
          tunnel: w3275 -> [w3282 w3287]
          frame True {
            n1984 = Unbundle By Name(w3282) -> ("Acquostic.Gains"=w3284:refnum<vi>)
            n1985 = property class="RadioBtnsControl (strict)"(reference=w3284, "Visible"=TRUE) -> (reference out=w3286:refnum<vi>, error out=w3285:errorcluster)  [unwired: 1 in]
            n1986 = Close Reference(reference=w3286, error in (no error)=w3285) -> ()  [unwired: 1 out]
          }
          frame False {
            n1987 = Unbundle By Name(w3287) -> ("Acquostic.Gains"=w3289:refnum<vi>)
            n1988 = property class="RadioBtnsControl (strict)"(reference=w3289, "Visible"=FALSE) -> (reference out=w3291:refnum<vi>, error out=w3290:errorcluster)  [unwired: 1 in]
            n1989 = Close Reference(reference=w3291, error in (no error)=w3290) -> ()  [unwired: 1 out]
          }
        }
        n1990 = call "DATA ENCRYPT STRING FILE WRITE.vi"("error in (no error)"=w3281, "User Action"="User Pressed  on  Acuostic in Environmental Screen", "main ref"=w3275) -> ("error out"=w3280:errorcluster)  [unwired: 6 in, 1 out]
      }
      frame "Report" {
        n1991 = call "REPORT GENERATION FOR PYTHON.vi"("error in (no error)"=w3297, "main ref"=w3294) -> ("error out"=w3296:errorcluster)  [unwired: 9 in]
        n1992 = local write "Report"(FALSE ("Report")) -> ()
        n1993 = call "DATA ENCRYPT STRING FILE WRITE.vi"("error in (no error)"=w3296, "User Action"="User Pressed Report ", "main ref"=w3294) -> ("error out"=w3295:errorcluster)  [unwired: 6 in, 1 out]
      }
      frame "Error" {
        # "#CodeRecommended - If you ever change the name of this \"Error\" message, you'll need to update the name in the Check Loop Error.vi as well."
        # "#CodeRecommended - Consider creating a system for logging errors in some way. These errors are for notification purposes only. Handling of specific errors should be performed in the message frames that generated the error."
        # "Error - Display an error dialog. This message is sent by the \"Error Handler\" VIs at the end of other loops in this application."
        n1994 = Variant To Data(error in=w3304, type=errorcluster {"status"=FALSE, "code"=0, "source"=""} ("error constant"), Variant=w3302) -> (data=w3300:errorcluster, error out=w3299:errorcluster)
        n1995 = call <vilib>:"Simple Error Handler.vi"("error in (no error)"=w3300) -> ()  [unwired: 4 in, 5 out]
        n1996 = Merge Errors(w3299) -> (w3298:errorcluster)
      }
      frame "Confirm Quit" {
        # "#CodeNeeded - If you want to provide an \"Are you sure\" dialog (or some other notification) before the application exits, place that code here. This message is typically sent from a Panel Close? event."
        # "Confirm Quit - Message that can confirm whether or not the user wants to exit the application."
        n1997 = call-poly "Enqueue Message.vi"("Priority Message? (F)"=TRUE, "error in (no error)"=w3311, "Message"="Exit", "Message Queue"=w3308) -> ("error out"=w3309:errorcluster)  [unwired: 6 in, 1 out]
        n1998 = Merge Errors(w3309) -> (w3310:errorcluster)
      }
      frame "Exit" {
        # "Stop the VI"
        # "Release the message queue reference"
        # "#CodeNeeded - Add any required cleanup code here. Note that if 'Exit' was called as a result of an error, an error dialog will be displayed. Add any custom error handling for an 'Exit' condition here as well."
        # "Exit - Exit the application."
        n1999 = call "Fire User Event - Stop.vi"("User Event - Stop"=w3314) -> ("error out"=w3313:errorcluster)  [unwired: 10 in]
        n2000 = Release Queue(queue=w3319, error in (no error)=w3312) -> (error out=w3316:errorcluster)  [unwired: 1 in, 2 out]
        n2001 = Merge Errors(w3313, w3316) -> (w3315:errorcluster)
      }
      frame Default {
        # "'Default' case only runs if there is a message that isn't defined in any of the other cases.  Output a programming error."
        n2002 = xnode ("Error Ring")("parameter 0"=w3320) -> ("error out"=w3321:errorcluster)
      }
    }
    n2003 = call "LAB-IQ Error Handler - Message Handling Loop.vi"("error in (no error)"=w1916, "Message Queue"=w1918) -> ("dup error in"=w1917:errorcluster)  [unwired: 8 in, 1 out]
  }
  n2004 = timed-loop "Timed Loop" {
    shift-right: [w3340] -> _
    shift-left: w9 -> [w3341]
    tunnel: [w3334] -> w52
    tunnel: w51 -> [w3332]
    tunnel: w6 -> [w3331]
    tunnel: w10 -> [w3330]
    timing: w28 -> [_]
    timing-out: [_] -> w27
    stop <- w3339 stop-if-true
    # "Load  Handling Loop"
    n2005 = node-c288() -> ()  [unwired: 1 in, 1 out]
    n2006 = call "Dequeue Message.vi"("error in (no error)"=w3331, "Message Queue"=w3332) -> ("error out"=w3338:errorcluster, "Message Data"=w3336:variant, "Message"=w3337:string, "dup Message Queue"=w3335:refnum<queue>)  [unwired: 6 in]
    n2007 = case "Message Cases" shown="\"Load Main\"" w3337 {
      selector: w3337 -> [_ _ _ _ _ w3397]
      tunnel: w3335 -> [w3344 w3357 _ w3386 w3396 _]
      tunnel: w3338 -> [w3347 w3355 w3373 w3388 w3390 _]
      tunnel: [w3348 w3358 w3367 w3374 w3392 w3398] -> w3333
      tunnel: w3341 -> [w3346 w3350 w3372 w3383 w3395 w3399]
      tunnel: [w3346 w3350 w3372 w3383 w3395 w3399] -> w3340
      tunnel: [_ _ _ _ TRUE _] -> w3339
      tunnel: w3336 -> [_ _ w3371 _ _ _]
      tunnel: w3330 -> [_ _ _ _ w3389 _]
      frame "init" {
        # "Bundle control references and a sample string value."
        # "Initialize - All initialization work should take place in this message, since other loops can potentially enqueue messages that execute immediately after this one."
        n2008 = call-poly "Enqueue Message.vi"("error in (no error)"=w3347, "Message"="Load Main", "Message Queue"=w3344) -> ("error out"=w3348:errorcluster)  [unwired: 7 in, 1 out]
      }
      frame "Load Main" {
        n2009 = call "LOAD CELL READ.vi"("error in (no error)"=w3355, "main ref"=w3350) -> ("error out"=w3351:errorcluster)  [unwired: 9 in]
        n2010 = call <vilib>:"Clear Errors.vi"("error in (no error)"=w3351) -> ("error out"=w3349:errorcluster)  [unwired: 5 in, 1 out]
        n2011 = Unbundle By Name(w3350) -> ("Main Home Screen.EXIT"=w3356:refnum<vi>)
        n2012 = property on="Property Node" class="Bool (strict)"(reference=w3356) -> (reference out=w3353:refnum<vi>, error out=w3354:errorcluster, "Value"=w3352:bool)  [unwired: 1 in]
        n2013 = Close Reference(reference=w3353, error in (no error)=w3354) -> ()  [unwired: 1 out]
        n2014 = case shown="False" w3352 {
          tunnel: [w3361 w3365] -> w3358
          tunnel: w3357 -> [w3360 w3364]
          tunnel: w3349 -> [w3359 w3363]
          frame True {
            n2015 = call-poly "Enqueue Message.vi"("error in (no error)"=w3359, "Message"="Confirm Quit", "Message Queue"=w3360) -> ("error out"=w3361:errorcluster)  [unwired: 7 in, 1 out]
          }
          frame False {
            n2016 = call-poly "Enqueue Message.vi"("error in (no error)"=w3363, "Message"="Load Main", "Message Queue"=w3364) -> ("error out"=w3365:errorcluster)  [unwired: 7 in, 1 out]
          }
        }
      }
      frame "Error" {
        # "#CodeRecommended - If you ever change the name of this \"Error\" message, you'll need to update the name in the Check Loop Error.vi as well."
        # "#CodeRecommended - Consider creating a system for logging errors in some way. These errors are for notification purposes only. Handling of specific errors should be performed in the message frames that generated the error."
        # "Error - Display an error dialog. This message is sent by the \"Error Handler\" VIs at the end of other loops in this application."
        n2017 = Variant To Data(error in=w3373, type=errorcluster {"status"=FALSE, "code"=0, "source"=""} ("error constant"), Variant=w3371) -> (data=w3369:errorcluster, error out=w3368:errorcluster)
        n2018 = call <vilib>:"Simple Error Handler.vi"("error in (no error)"=w3369) -> ()  [unwired: 4 in, 5 out]
        n2019 = Merge Errors(w3368) -> (w3367:errorcluster)
      }
      frame "Confirm Quit" {
        # "#CodeNeeded - If you want to provide an \"Are you sure\" dialog (or some other notification) before the application exits, place that code here. This message is typically sent from a Panel Close? event."
        # "Confirm Quit - Message that can confirm whether or not the user wants to exit the application."
        n2020 = call-poly "Enqueue Message.vi"("Priority Message? (F)"=TRUE, "error in (no error)"=w3388, "Message"="Exit", "Message Queue"=w3386) -> ("error out"=w3387:errorcluster)  [unwired: 6 in, 1 out]
        n2021 = Merge Errors(w3387) -> (w3379:errorcluster)
        n2022 = call <vilib>:"Clear Errors.vi"("error in (no error)"=w3379) -> ("error out"=w3375:errorcluster)  [unwired: 5 in, 1 out]
        n2023 = call "LOAD CELL FGV MAIN.vi"("Enum"=T25."UNINITIAL", "error in (no error)"=w3375, "main ref"=w3383) -> ("error IO"=w3382:errorcluster)  [unwired: 8 in]
        n2024 = call "Stall Data Flow.vim"("value in"=w3382, "milliseconds to wait"=u32 1000) -> ("value out"=w3377:errorcluster)  [unwired: 1 out]
        n2025 = call "LOAD CELL FGV MAIN.vi"("Enum"=T25."DELETEHANDLE", "error in (no error)"=w3377, "main ref"=w3383) -> ("error IO"=w3378:errorcluster)  [unwired: 8 in]
        n2026 = call <vilib>:"Clear Errors.vi"("error in (no error)"=w3378) -> ("error out"=w3374:errorcluster)  [unwired: 5 in, 1 out]
      }
      frame "Exit" {
        # "Stop the VI"
        # "Release the message queue reference"
        # "#CodeNeeded - Add any required cleanup code here. Note that if 'Exit' was called as a result of an error, an error dialog will be displayed. Add any custom error handling for an 'Exit' condition here as well."
        # "Exit - Exit the application."
        n2027 = call "Fire User Event - Stop.vi"("User Event - Stop"=w3389) -> ("error out"=w3391:errorcluster)  [unwired: 10 in]
        n2028 = Release Queue(queue=w3396, error in (no error)=w3390) -> (error out=w3393:errorcluster)  [unwired: 1 in, 2 out]
        n2029 = Merge Errors(w3391, w3393) -> (w3392:errorcluster)
      }
      frame Default {
        # "'Default' case only runs if there is a message that isn't defined in any of the other cases.  Output a programming error."
        n2030 = xnode ("Error Ring")("parameter 0"=w3397) -> ("error out"=w3398:errorcluster)
      }
    }
    n2031 = call "LAB-IQ Error Handler - Message Handling Loop.vi"("error in (no error)"=w3333, "Message Queue"=w3335) -> ("dup error in"=w3334:errorcluster)  [unwired: 8 in, 1 out]
    n2032 = node-c288() -> ()  [unwired: 1 in, 1 out]
  }
  n2033 = timed-loop "Timed Loop" {
    shift-right: [w3408] -> _
    shift-left: w9 -> [w3427]
    tunnel: [w3421] -> w49
    tunnel: w50 -> [w3419]
    tunnel: w6 -> [w3418]
    tunnel: w10 -> [w3417]
    timing: w30 -> [_]
    timing-out: [_] -> w29
    stop <- w3426 stop-if-true
    # "Sway Motor  Handling Loop"
    n2034 = node-c288() -> ()  [unwired: 1 in, 1 out]
    n2035 = call "Dequeue Message.vi"("error in (no error)"=w3418, "Message Queue"=w3419) -> ("error out"=w3425:errorcluster, "Message Data"=w3423:variant, "Message"=w3424:string, "dup Message Queue"=w3422:refnum<queue>)  [unwired: 6 in]
    n2036 = case "Message Cases" shown="\"init\"" w3424 {
      selector: w3424 -> [_ _ _ _ _ w3515]
      tunnel: w3422 -> [w3443 w3472 _ w3502 w3514 _]
      tunnel: w3425 -> [w3445 w3455 w3499 w3506 w3508 _]
      tunnel: [w3446 w3473 w3493 w3504 w3510 w3516] -> w3420
      tunnel: w3427 -> [w3433 w3450 w3498 w3505 w3513 w3517]
      tunnel: [w3433 w3450 w3498 w3505 w3513 w3517] -> w3408
      tunnel: [_ _ _ _ TRUE _] -> w3426
      tunnel: w3423 -> [_ _ w3497 _ _ _]
      tunnel: w3417 -> [_ _ _ _ w3507 _]
      frame "init" {
        # "Initialize - All initialization work should take place in this message, since other loops can potentially enqueue messages that execute immediately after this one."
        n2037 = call "SWAY WRITE FGV.vi"("Enum - Menu"=Sway_Write_enum."INIT", "error in (no error)"=w3445, "main ref"=w3433) -> ("error out"=w3442:errorcluster)  [unwired: 8 in]
        n2038 = call <vilib>:"Clear Errors.vi"("error in (no error)"=w3442) -> ("error out"=w3436:errorcluster)  [unwired: 5 in, 1 out]
        n2039 = call "Stall Data Flow.vim"("value in"=w3436, "milliseconds to wait"=u32 1000) -> ("value out"=w3440:errorcluster)  [unwired: 1 out]
        n2040 = call "Sway Init.vi"("error in (no error)"=w3440, "main ref"=w3433) -> ("error out"=w3437:errorcluster)  [unwired: 9 in]
        n2041 = call <vilib>:"Clear Errors.vi"("error in (no error)"=w3437) -> ("error out"=w3435:errorcluster)  [unwired: 5 in, 1 out]
        n2042 = call "SWAY READ FGV.vi"("Enum - Menu"=Sway_Right_enum."INIT", "error in (no error)"=w3435, "main ref"=w3433) -> ("error out"=w3434:errorcluster)  [unwired: 7 in, 1 out]
        n2043 = call <vilib>:"Clear Errors.vi"("error in (no error)"=w3434) -> ("error out"=w3438:errorcluster)  [unwired: 5 in, 1 out]
        n2044 = call-poly "Enqueue Message.vi"("error in (no error)"=w3438, "Message"="Sway Main", "Message Queue"=w3443) -> ("error out"=w3446:errorcluster)  [unwired: 7 in, 1 out]
      }
      frame "Sway Main" {
        n2045 = Unbundle By Name(w3450) -> ("Heave AND Surge.Homed"=w3458:refnum<vi>)
        n2046 = Unbundle By Name(w3450) -> ("SWAY.Read SWAY Temp"=w3467:refnum<vi>)
        n2047 = local read "HEAVE ENABLE"() -> (w3462:bool)
        n2048 = property on="Property Node" class="DigNum (strict)"(reference=w3458) -> (reference out=w3460:refnum<vi>, error out=w3459:errorcluster, "Value"=w3449:u8)  [unwired: 1 in]
        n2049 = property on="Property Node" class="Bool (strict)"(reference=w3467) -> (reference out=w3465:refnum<vi>, error out=w3466:errorcluster, "Value"=w3464:bool)  [unwired: 1 in]
        n2050 = Equal?(x=w3462, y=TRUE) -> (x = y?=w3457:bool)
        n2051 = Close Reference(reference=w3460, error in (no error)=w3459) -> ()  [unwired: 1 out]
        n2052 = Equal?(x=w3449, y=u8 1 ("Value")) -> (x = y?=w3447:bool)
        n2053 = Close Reference(reference=w3465, error in (no error)=w3466) -> ()  [unwired: 1 out]
        n2054 = And(x=w3457, y=w3447) -> (x .and. y?=w3456:bool)
        n2055 = case shown="True" w3464 {
          tunnel: w3455 -> [w3480 w3484]
          tunnel: [w3480 w3483] -> w3452
          tunnel: w3450 -> [_ w3482]
          frame False {
          }
          frame True {
            n2056 = call "SWAY READ FGV.vi"("Enum - Menu"=Sway_Right_enum."READ", "error in (no error)"=w3484, "main ref"=w3482) -> ("error out"=w3483:errorcluster)  [unwired: 7 in, 1 out]
          }
        }
        n2057 = case shown="True" w3456 {
          tunnel: w3450 -> [_ w3479]
          tunnel: w3455 -> [w3474 w3478]
          tunnel: [w3474 w3475] -> w3453
          frame False {
          }
          frame True {
            n2058 = call "SWAY HOME.vi"("error in (no error)"=w3478, "Data Cluster"=w3479) -> ("error out"=w3476:errorcluster)  [unwired: 9 in]
            n2059 = local write "HEAVE ENABLE"(FALSE ("HEAVE ENABLE")) -> ()
            n2060 = call <vilib>:"Clear Errors.vi"("error in (no error)"=w3476) -> ("error out"=w3475:errorcluster)  [unwired: 5 in, 1 out]
          }
        }
        n2061 = call "Sway Reinitize.vi"("error in (no error)"=w3452, "Data Cluster"=w3450) -> ("error out"=w3451:errorcluster)  [unwired: 9 in]
        n2062 = Unbundle By Name(w3450) -> ("Main Home Screen.EXIT"=w3471:refnum<vi>)
        n2063 = property on="Property Node" class="Bool (strict)"(reference=w3471) -> (reference out=w3469:refnum<vi>, error out=w3470:errorcluster, "Value"=w3468:bool)  [unwired: 1 in]
        n2064 = call <vilib>:"Clear Errors.vi"("error in (no error)"=w3451) -> ("error out"=w3463:errorcluster)  [unwired: 5 in, 1 out]
        n2065 = Merge Errors(w3463, w3453) -> (w3454:errorcluster)
        n2066 = Close Reference(reference=w3469, error in (no error)=w3470) -> ()  [unwired: 1 out]
        n2067 = case shown="False" w3468 {
          tunnel: [w3487 w3491] -> w3473
          tunnel: w3472 -> [w3486 w3490]
          tunnel: w3454 -> [w3485 w3489]
          frame True {
            n2068 = call-poly "Enqueue Message.vi"("error in (no error)"=w3485, "Message"="Confirm Quit", "Message Queue"=w3486) -> ("error out"=w3487:errorcluster)  [unwired: 7 in, 1 out]
          }
          frame False {
            n2069 = call-poly "Enqueue Message.vi"("error in (no error)"=w3489, "Message"="Sway Main", "Message Queue"=w3490) -> ("error out"=w3491:errorcluster)  [unwired: 7 in, 1 out]
          }
        }
      }
      frame "Error" {
        # "#CodeRecommended - If you ever change the name of this \"Error\" message, you'll need to update the name in the Check Loop Error.vi as well."
        # "#CodeRecommended - Consider creating a system for logging errors in some way. These errors are for notification purposes only. Handling of specific errors should be performed in the message frames that generated the error."
        # "Error - Display an error dialog. This message is sent by the \"Error Handler\" VIs at the end of other loops in this application."
        n2070 = Variant To Data(error in=w3499, type=errorcluster {"status"=FALSE, "code"=0, "source"=""} ("error constant"), Variant=w3497) -> (data=w3495:errorcluster, error out=w3494:errorcluster)
        n2071 = call <vilib>:"Simple Error Handler.vi"("error in (no error)"=w3495) -> ()  [unwired: 4 in, 5 out]
        n2072 = Merge Errors(w3494) -> (w3493:errorcluster)
      }
      frame "Confirm Quit" {
        # "#CodeNeeded - If you want to provide an \"Are you sure\" dialog (or some other notification) before the application exits, place that code here. This message is typically sent from a Panel Close? event."
        # "Confirm Quit - Message that can confirm whether or not the user wants to exit the application."
        n2073 = call-poly "Enqueue Message.vi"("Priority Message? (F)"=TRUE, "error in (no error)"=w3506, "Message"="Exit", "Message Queue"=w3502) -> ("error out"=w3503:errorcluster)  [unwired: 6 in, 1 out]
        n2074 = Merge Errors(w3503) -> (w3504:errorcluster)
      }
      frame "Exit" {
        # "Stop the VI"
        # "Release the message queue reference"
        # "#CodeNeeded - Add any required cleanup code here. Note that if 'Exit' was called as a result of an error, an error dialog will be displayed. Add any custom error handling for an 'Exit' condition here as well."
        # "Exit - Exit the application."
        n2075 = call "Fire User Event - Stop.vi"("User Event - Stop"=w3507) -> ("error out"=w3509:errorcluster)  [unwired: 10 in]
        n2076 = Release Queue(queue=w3514, error in (no error)=w3508) -> (error out=w3511:errorcluster)  [unwired: 1 in, 2 out]
        n2077 = Merge Errors(w3509, w3511) -> (w3510:errorcluster)
      }
      frame Default {
        # "'Default' case only runs if there is a message that isn't defined in any of the other cases.  Output a programming error."
        n2078 = xnode ("Error Ring")("parameter 0"=w3515) -> ("error out"=w3516:errorcluster)
      }
    }
    n2079 = Unbundle By Name(w3408) -> ("Environmental control.Acoustic Emission 3"=w3416:refnum<vi>)
    n2080 = call "LAB-IQ Error Handler - Message Handling Loop.vi"("error in (no error)"=w3420, "Message Queue"=w3422) -> ("dup error in"=w3421:errorcluster)  [unwired: 8 in, 1 out]
    n2081 = property on="Property Node" class="Bool (strict)"(reference=w3416) -> (reference out=w3414:refnum<vi>, error out=w3415:errorcluster, "Value"=w3413:bool)  [unwired: 1 in]
    n2082 = Close Reference(reference=w3414, error in (no error)=w3415) -> ()  [unwired: 1 out]
    n2083 = Equal?(x=w3413, y=TRUE) -> (x = y?=w3411:bool)
    n2084 = Select(t=i64 100 ("Period"), s=w3411, f=i64 10) -> (s? t:f=w3407:i64)
    n2085 = node-c288(w3407) -> ()  [unwired: 1 in, 1 out]
  }
  n2086 = timed-loop {
    shift-right: [w3535] -> _
    shift-left: w9 -> [w3536]
    tunnel: [w3529] -> w23
    tunnel: w46 -> [w3527]
    tunnel: w6 -> [w3526]
    tunnel: w10 -> [w3525]
    timing: w2 -> [_]
    timing-out: [_] -> w1
    stop <- w3534 stop-if-true
    # "Ramp Motor  Handling Loop"
    n2087 = node-c288() -> ()  [unwired: 1 in, 1 out]
    n2088 = call "Dequeue Message.vi"("error in (no error)"=w3526, "Message Queue"=w3527) -> ("error out"=w3533:errorcluster, "Message Data"=w3531:variant, "Message"=w3532:string, "dup Message Queue"=w3530:refnum<queue>)  [unwired: 6 in]
    n2089 = case "Message Cases" shown="\"init\"" w3532 {
      selector: w3532 -> [_ _ _ _ _ w3606]
      tunnel: w3530 -> [w3550 w3566 _ w3593 w3605 _]
      tunnel: w3533 -> [w3552 w3564 w3590 w3597 w3599 _]
      tunnel: [w3553 w3567 w3584 w3595 w3601 w3607] -> w3528
      tunnel: w3536 -> [w3541 w3555 w3589 w3596 w3604 w3608]
      tunnel: [w3541 w3555 w3589 w3596 w3604 w3608] -> w3535
      tunnel: [_ _ _ _ TRUE _] -> w3534
      tunnel: w3531 -> [_ _ w3588 _ _ _]
      tunnel: w3525 -> [_ _ _ _ w3598 _]
      frame "init" {
        # "Initialize - All initialization work should take place in this message, since other loops can potentially enqueue messages that execute immediately after this one."
        n2090 = call "TRACTION WRITE FGV.vi"("Enum - Menu"=Traction_Write_enum."INIT", "error in (no error)"=w3552, "main ref"=w3541) -> ("error out"=w3549:errorcluster)  [unwired: 8 in]
        n2091 = call <vilib>:"Clear Errors.vi"("error in (no error)"=w3549) -> ("error out"=w3547:errorcluster)  [unwired: 5 in, 1 out]
        n2092 = call "Stall Data Flow.vim"("value in"=w3547, "milliseconds to wait"=u32 1000) -> ("value out"=w3546:errorcluster)  [unwired: 1 out]
        n2093 = call "Traction  Init.vi"("error in (no error)"=w3546, "main ref"=w3541) -> ("error out"=w3544:errorcluster)  [unwired: 9 in]
        n2094 = call <vilib>:"Clear Errors.vi"("error in (no error)"=w3544) -> ("error out"=w3543:errorcluster)  [unwired: 5 in, 1 out]
        n2095 = call "TRACTION READ FGV.vi"("Enum - Menu"=Traction_Read_enum."INIT", "error in (no error)"=w3543, "main ref"=w3541) -> ("error out"=w3542:errorcluster)  [unwired: 6 in, 2 out]
        n2096 = call <vilib>:"Clear Errors.vi"("error in (no error)"=w3542) -> ("error out"=w3540:errorcluster)  [unwired: 5 in, 1 out]
        n2097 = call-poly "Enqueue Message.vi"("error in (no error)"=w3540, "Message"="Ramp Main", "Message Queue"=w3550) -> ("error out"=w3553:errorcluster)  [unwired: 7 in, 1 out]
      }
      frame "Ramp Main" {
        n2098 = Unbundle By Name(w3555) -> ("Traction.Read TRACTION Temp"=w3560:refnum<vi>)
        n2099 = property on="Property Node" class="Bool (strict)"(reference=w3560) -> (reference out=w3558:refnum<vi>, error out=w3559:errorcluster, "Value"=w3556:bool)  [unwired: 1 in]
        n2100 = Close Reference(reference=w3558, error in (no error)=w3559) -> ()  [unwired: 1 out]
        n2101 = case shown="True" w3556 {
          tunnel: w3564 -> [w3568 w3575]
          tunnel: [w3568 w3572] -> w3557
          tunnel: w3555 -> [_ w3573]
          tunnel: w3555 -> [_ w3571]
          frame False {
          }
          frame True {
            n2102 = call "TRACTION READ FGV.vi"("Enum - Menu"=Traction_Read_enum."READ", "error in (no error)"=w3575, "main ref"=w3573) -> ("error out"=w3574:errorcluster, "ERROR TEMP"=w3570:bool)  [unwired: 6 in, 1 out]
            n2103 = call "Traction Reinitize.vi"("error in (no error)"=w3574, "Checkbox"=w3570, "Data Cluster"=w3571) -> ("error out"=w3572:errorcluster)  [unwired: 8 in]
          }
        }
        n2104 = Unbundle By Name(w3555) -> ("Main Home Screen.EXIT"=w3565:refnum<vi>)
        n2105 = call <vilib>:"Clear Errors.vi"("error in (no error)"=w3557) -> ("error out"=w3554:errorcluster)  [unwired: 5 in, 1 out]
        n2106 = property on="Property Node" class="Bool (strict)"(reference=w3565) -> (reference out=w3562:refnum<vi>, error out=w3563:errorcluster, "Value"=w3561:bool)  [unwired: 1 in]
        n2107 = case shown="False" w3561 {
          tunnel: [w3578 w3582] -> w3567
          tunnel: w3566 -> [w3577 w3581]
          tunnel: w3554 -> [w3576 w3580]
          frame True {
            n2108 = call-poly "Enqueue Message.vi"("error in (no error)"=w3576, "Message"="Confirm Quit", "Message Queue"=w3577) -> ("error out"=w3578:errorcluster)  [unwired: 7 in, 1 out]
          }
          frame False {
            n2109 = call-poly "Enqueue Message.vi"("error in (no error)"=w3580, "Message"="Ramp Main", "Message Queue"=w3581) -> ("error out"=w3582:errorcluster)  [unwired: 7 in, 1 out]
          }
        }
        n2110 = Close Reference(reference=w3562, error in (no error)=w3563) -> ()  [unwired: 1 out]
      }
      frame "Error" {
        # "#CodeRecommended - If you ever change the name of this \"Error\" message, you'll need to update the name in the Check Loop Error.vi as well."
        # "#CodeRecommended - Consider creating a system for logging errors in some way. These errors are for notification purposes only. Handling of specific errors should be performed in the message frames that generated the error."
        # "Error - Display an error dialog. This message is sent by the \"Error Handler\" VIs at the end of other loops in this application."
        n2111 = Variant To Data(error in=w3590, type=errorcluster {"status"=FALSE, "code"=0, "source"=""} ("error constant"), Variant=w3588) -> (data=w3586:errorcluster, error out=w3585:errorcluster)
        n2112 = call <vilib>:"Simple Error Handler.vi"("error in (no error)"=w3586) -> ()  [unwired: 4 in, 5 out]
        n2113 = Merge Errors(w3585) -> (w3584:errorcluster)
      }
      frame "Confirm Quit" {
        # "#CodeNeeded - If you want to provide an \"Are you sure\" dialog (or some other notification) before the application exits, place that code here. This message is typically sent from a Panel Close? event."
        # "Confirm Quit - Message that can confirm whether or not the user wants to exit the application."
        n2114 = call-poly "Enqueue Message.vi"("Priority Message? (F)"=TRUE, "error in (no error)"=w3597, "Message"="Exit", "Message Queue"=w3593) -> ("error out"=w3594:errorcluster)  [unwired: 6 in, 1 out]
        n2115 = Merge Errors(w3594) -> (w3595:errorcluster)
      }
      frame "Exit" {
        # "Stop the VI"
        # "Release the message queue reference"
        # "#CodeNeeded - Add any required cleanup code here. Note that if 'Exit' was called as a result of an error, an error dialog will be displayed. Add any custom error handling for an 'Exit' condition here as well."
        # "Exit - Exit the application."
        n2116 = call "Fire User Event - Stop.vi"("User Event - Stop"=w3598) -> ("error out"=w3600:errorcluster)  [unwired: 10 in]
        n2117 = Release Queue(queue=w3605, error in (no error)=w3599) -> (error out=w3602:errorcluster)  [unwired: 1 in, 2 out]
        n2118 = Merge Errors(w3600, w3602) -> (w3601:errorcluster)
      }
      frame Default {
        # "'Default' case only runs if there is a message that isn't defined in any of the other cases.  Output a programming error."
        n2119 = xnode ("Error Ring")("parameter 0"=w3606) -> ("error out"=w3607:errorcluster)
      }
    }
    n2120 = call "LAB-IQ Error Handler - Message Handling Loop.vi"("error in (no error)"=w3528, "Message Queue"=w3530) -> ("dup error in"=w3529:errorcluster)  [unwired: 8 in, 1 out]
    n2121 = node-c288() -> ()  [unwired: 1 in, 1 out]
  }
  n2122 = while {
    shift-right: [w3626] -> _
    shift-left: w9 -> [w3627]
    tunnel: [w3620] -> w15
    tunnel: w43 -> [w3618]
    tunnel: w6 -> [w3617]
    tunnel: w10 -> [w3616]
    stop <- w3625 stop-if-true
    # "Program  Handling Loop"
    n2123 = call "Dequeue Message.vi"("error in (no error)"=w3617, "Message Queue"=w3618) -> ("error out"=w3624:errorcluster, "Message Data"=w3622:variant, "Message"=w3623:string, "dup Message Queue"=w3621:refnum<queue>)  [unwired: 6 in]
    n2124 = case "Message Cases" shown="\"Program Main\"" w3623 {
      selector: w3623 -> [_ _ _ _ _ w3672]
      tunnel: w3621 -> [w3628 w3640 _ w3659 w3671 _]
      tunnel: w3624 -> [w3631 w3634 w3656 w3663 w3665 _]
      tunnel: [w3632 w3641 w3650 w3661 w3667 w3673] -> w3619
      tunnel: w3627 -> [w3630 w3633 w3655 w3662 w3670 w3674]
      tunnel: [w3630 w3633 w3655 w3662 w3670 w3674] -> w3626
      tunnel: [_ _ _ _ TRUE _] -> w3625
      tunnel: w3622 -> [_ _ w3654 _ _ _]
      tunnel: w3616 -> [_ _ _ _ w3664 _]
      frame "init" {
        # "Initialize - All initialization work should take place in this message, since other loops can potentially enqueue messages that execute immediately after this one."
        n2125 = call-poly "Enqueue Message.vi"("error in (no error)"=w3631, "Message"="Program Main", "Message Queue"=w3628) -> ("error out"=w3632:errorcluster)  [unwired: 7 in, 1 out]
      }
      frame "Program Main" {
        n2126 = call "Main Program Loop Vi.vi"("error in (no error)"=w3634, "Data Cluster"=w3633) -> ("error out"=w3635:errorcluster)  [unwired: 9 in]
        n2127 = Unbundle By Name(w3633) -> ("Main Home Screen.EXIT"=w3639:refnum<vi>)
        n2128 = property on="Property Node" class="Bool (strict)"(reference=w3639) -> (reference out=w3637:refnum<vi>, error out=w3638:errorcluster, "Value"=w3636:bool)  [unwired: 1 in]
        n2129 = case shown="False" w3636 {
          tunnel: [w3644 w3648] -> w3641
          tunnel: w3640 -> [w3643 w3647]
          tunnel: w3635 -> [w3642 w3646]
          frame True {
            n2130 = call-poly "Enqueue Message.vi"("error in (no error)"=w3642, "Message"="Confirm Quit", "Message Queue"=w3643) -> ("error out"=w3644:errorcluster)  [unwired: 7 in, 1 out]
          }
          frame False {
            n2131 = call-poly "Enqueue Message.vi"("error in (no error)"=w3646, "Message"="Program Main", "Message Queue"=w3647) -> ("error out"=w3648:errorcluster)  [unwired: 7 in, 1 out]
          }
        }
        n2132 = Close Reference(reference=w3637, error in (no error)=w3638) -> ()  [unwired: 1 out]
      }
      frame "Error" {
        # "#CodeRecommended - If you ever change the name of this \"Error\" message, you'll need to update the name in the Check Loop Error.vi as well."
        # "#CodeRecommended - Consider creating a system for logging errors in some way. These errors are for notification purposes only. Handling of specific errors should be performed in the message frames that generated the error."
        # "Error - Display an error dialog. This message is sent by the \"Error Handler\" VIs at the end of other loops in this application."
        n2133 = Variant To Data(error in=w3656, type=errorcluster {"status"=FALSE, "code"=0, "source"=""} ("error constant"), Variant=w3654) -> (data=w3652:errorcluster, error out=w3651:errorcluster)
        n2134 = call <vilib>:"Simple Error Handler.vi"("error in (no error)"=w3652) -> ()  [unwired: 4 in, 5 out]
        n2135 = Merge Errors(w3651) -> (w3650:errorcluster)
      }
      frame "Confirm Quit" {
        # "#CodeNeeded - If you want to provide an \"Are you sure\" dialog (or some other notification) before the application exits, place that code here. This message is typically sent from a Panel Close? event."
        # "Confirm Quit - Message that can confirm whether or not the user wants to exit the application."
        n2136 = call-poly "Enqueue Message.vi"("Priority Message? (F)"=TRUE, "error in (no error)"=w3663, "Message"="Exit", "Message Queue"=w3659) -> ("error out"=w3660:errorcluster)  [unwired: 6 in, 1 out]
        n2137 = Merge Errors(w3660) -> (w3661:errorcluster)
      }
      frame "Exit" {
        # "Stop the VI"
        # "Release the message queue reference"
        # "#CodeNeeded - Add any required cleanup code here. Note that if 'Exit' was called as a result of an error, an error dialog will be displayed. Add any custom error handling for an 'Exit' condition here as well."
        # "Exit - Exit the application."
        n2138 = call "Fire User Event - Stop.vi"("User Event - Stop"=w3664) -> ("error out"=w3666:errorcluster)  [unwired: 10 in]
        n2139 = Release Queue(queue=w3671, error in (no error)=w3665) -> (error out=w3668:errorcluster)  [unwired: 1 in, 2 out]
        n2140 = Merge Errors(w3666, w3668) -> (w3667:errorcluster)
      }
      frame Default {
        # "'Default' case only runs if there is a message that isn't defined in any of the other cases.  Output a programming error."
        n2141 = xnode ("Error Ring")("parameter 0"=w3672) -> ("error out"=w3673:errorcluster)
      }
    }
    n2142 = call "LAB-IQ Error Handler - Message Handling Loop.vi"("error in (no error)"=w3619, "Message Queue"=w3621) -> ("dup error in"=w3620:errorcluster)  [unwired: 8 in, 1 out]
  }
  n2143 = while "Timed Loop" {
    shift-right: [w3688] -> _
    shift-left: w9 -> [w3702]
    tunnel: [w3696] -> w14
    tunnel: w42 -> [w3694]
    tunnel: w6 -> [w3693]
    tunnel: w10 -> [w3692]
    stop <- w3701 stop-if-true
    # "Monitor  Handling Loop"
    n2144 = call "Dequeue Message.vi"("error in (no error)"=w3693, "Message Queue"=w3694) -> ("error out"=w3700:errorcluster, "Message Data"=w3698:variant, "Message"=w3699:string, "dup Message Queue"=w3697:refnum<queue>)  [unwired: 6 in]
    n2145 = case "Message Cases" shown="\"Monitor Main\"" w3699 {
      selector: w3699 -> [_ _ _ _ _ w3750]
      tunnel: w3697 -> [w3703 w3718 _ w3737 w3749 _]
      tunnel: w3700 -> [w3706 w3708 w3734 w3741 w3743 _]
      tunnel: [w3707 w3719 w3728 w3739 w3745 w3751] -> w3695
      tunnel: w3702 -> [w3705 w3709 w3733 w3740 w3748 w3752]
      tunnel: [w3705 w3709 w3733 w3740 w3748 w3752] -> w3688
      tunnel: [_ _ _ _ TRUE _] -> w3701
      tunnel: w3698 -> [_ _ w3732 _ _ _]
      tunnel: w3692 -> [_ _ _ _ w3742 _]
      frame "init" {
        # "Initialize - All initialization work should take place in this message, since other loops can potentially enqueue messages that execute immediately after this one."
        n2146 = call-poly "Enqueue Message.vi"("error in (no error)"=w3706, "Message"="Monitor Main", "Message Queue"=w3703) -> ("error out"=w3707:errorcluster)  [unwired: 7 in, 1 out]
      }
      frame "Monitor Main" {
        n2147 = call "Main Monitor Loop.vi"("error in (no error)"=w3708, "main ref"=w3709) -> ("error out"=w3713:errorcluster)  [unwired: 9 in]
        n2148 = call "LOAD SELECTION MAIN CODE.vi"("error in (no error)"=w3708, "main ref"=w3709) -> ("error out"=w3711:errorcluster)  [unwired: 9 in]
        n2149 = call "Trip Log and Trip Monitor.vi"("error in (no error)"=w3708, "main ref"=w3709) -> ("error out"=w3710:errorcluster)  [unwired: 9 in]
        n2150 = Merge Errors(w3713, w3711, w3710) -> (w3712:errorcluster)
        n2151 = Unbundle By Name(w3709) -> ("Main Home Screen.EXIT"=w3717:refnum<vi>)
        n2152 = property on="Property Node" class="Bool (strict)"(reference=w3717) -> (reference out=w3715:refnum<vi>, error out=w3716:errorcluster, "Value"=w3714:bool)  [unwired: 1 in]
        n2153 = case shown="False" w3714 {
          tunnel: [w3722 w3726] -> w3719
          tunnel: w3718 -> [w3721 w3725]
          tunnel: w3712 -> [w3720 w3724]
          frame True {
            n2154 = call-poly "Enqueue Message.vi"("error in (no error)"=w3720, "Message"="Confirm Quit", "Message Queue"=w3721) -> ("error out"=w3722:errorcluster)  [unwired: 7 in, 1 out]
          }
          frame False {
            n2155 = call-poly "Enqueue Message.vi"("error in (no error)"=w3724, "Message"="Monitor Main", "Message Queue"=w3725) -> ("error out"=w3726:errorcluster)  [unwired: 7 in, 1 out]
          }
        }
        n2156 = Close Reference(reference=w3715, error in (no error)=w3716) -> ()  [unwired: 1 out]
      }
      frame "Error" {
        # "#CodeRecommended - If you ever change the name of this \"Error\" message, you'll need to update the name in the Check Loop Error.vi as well."
        # "#CodeRecommended - Consider creating a system for logging errors in some way. These errors are for notification purposes only. Handling of specific errors should be performed in the message frames that generated the error."
        # "Error - Display an error dialog. This message is sent by the \"Error Handler\" VIs at the end of other loops in this application."
        n2157 = Variant To Data(error in=w3734, type=errorcluster {"status"=FALSE, "code"=0, "source"=""} ("error constant"), Variant=w3732) -> (data=w3730:errorcluster, error out=w3729:errorcluster)
        n2158 = call <vilib>:"Simple Error Handler.vi"("error in (no error)"=w3730) -> ()  [unwired: 4 in, 5 out]
        n2159 = Merge Errors(w3729) -> (w3728:errorcluster)
      }
      frame "Confirm Quit" {
        # "#CodeNeeded - If you want to provide an \"Are you sure\" dialog (or some other notification) before the application exits, place that code here. This message is typically sent from a Panel Close? event."
        # "Confirm Quit - Message that can confirm whether or not the user wants to exit the application."
        n2160 = call-poly "Enqueue Message.vi"("Priority Message? (F)"=TRUE, "error in (no error)"=w3741, "Message"="Exit", "Message Queue"=w3737) -> ("error out"=w3738:errorcluster)  [unwired: 6 in, 1 out]
        n2161 = Merge Errors(w3738) -> (w3739:errorcluster)
      }
      frame "Exit" {
        # "Stop the VI"
        # "Release the message queue reference"
        # "#CodeNeeded - Add any required cleanup code here. Note that if 'Exit' was called as a result of an error, an error dialog will be displayed. Add any custom error handling for an 'Exit' condition here as well."
        # "Exit - Exit the application."
        n2162 = call "Fire User Event - Stop.vi"("User Event - Stop"=w3742) -> ("error out"=w3744:errorcluster)  [unwired: 10 in]
        n2163 = Release Queue(queue=w3749, error in (no error)=w3743) -> (error out=w3746:errorcluster)  [unwired: 1 in, 2 out]
        n2164 = Merge Errors(w3744, w3746) -> (w3745:errorcluster)
      }
      frame Default {
        # "'Default' case only runs if there is a message that isn't defined in any of the other cases.  Output a programming error."
        n2165 = xnode ("Error Ring")("parameter 0"=w3750) -> ("error out"=w3751:errorcluster)
      }
    }
    n2166 = Unbundle By Name(w3688) -> ("Environmental control.Acoustic Emission 3"=w3691:refnum<vi>)
    n2167 = property on="Property Node" class="Bool (strict)"(reference=w3691) -> (reference out=w3689:refnum<vi>, error out=w3690:errorcluster, "Value"=w3687:bool)  [unwired: 1 in]
    n2168 = call "LAB-IQ Error Handler - Message Handling Loop.vi"("error in (no error)"=w3695, "Message Queue"=w3697) -> ("dup error in"=w3696:errorcluster)  [unwired: 8 in, 1 out]
    n2169 = Close Reference(reference=w3689, error in (no error)=w3690) -> ()  [unwired: 1 out]
    n2170 = Equal?(x=w3687, y=TRUE) -> (x = y?=w3685:bool)
    n2171 = Select(t=i64 30 ("Period"), s=w3685, f=i64 100) -> (s? t:f=w3682:i64)
    n2172 = Wait (ms)(milliseconds to wait=w3682) -> ()  [unwired: 1 out]
  }
  n2173 = Unregister For Events(event registration refnum=w75, error in=w73) -> (error out=w76:errorcluster)
  n2174 = node-c288(w27) -> ()  [unwired: 1 out]
  n2175 = node-c288(w19) -> ()  [unwired: 1 out]
  n2176 = node-c288(w1) -> ()  [unwired: 1 out]
  n2177 = node-c288(w25) -> ()  [unwired: 1 out]
  n2178 = node-c288(w3) -> ()  [unwired: 1 out]
  n2179 = node-c288(w29) -> ()  [unwired: 1 out]
  n2180 = Merge Errors(w76, w79, w52, w49, w47, w32, w23, w17, w16, w15, w14, w12, w13, w5) -> (w77:errorcluster)
  n2181 = call "Destroy User Event - Stop.vi"("error in (no error)"=w77, "User Event - Stop"=w10) -> ("error out"=w74:errorcluster)  [unwired: 9 in]
  n2182 = disable-structure "Conditional Disable Structure" shown="RUN_TIME_ENGINE==True" {
    disable-tunnel: w74 -> [_ _]
    frame condition #0 (active) {
    }
    frame condition #1 {
      # "Call Quit LabVIEW if running as a built application."
      n2183 = Quit LabVIEW() -> ()  [unwired: 1 in]
    }
  }
